vi "UNITEST MAIN v2.0.vi"() -> ()   [LabVIEW 2025]
uses:
  support/Message Queue/LAB-IQ Message Queue.lvlib
  support/Message Queue/Enqueue Message (Single).vi
  support/User Event - Stop/LAB-IQ User Event - Stop.lvlib
  <vilib>/Utility/error.llb/Error Cluster From Error Code.vi
  <vilib>/ErrorRing/Error Ring.xnode
  controls/LAB-IQ UI Data.ctl
  02c5850b-52e8-4ed5-91f8-6f0ad62f4994.vi
  HEAVE vi's/Heave Write enum.ctl
  d081153b-36ca-4bc4-8478-749476f82ba4.vi
  1223eb78-e4c4-4b69-bf80-185c82055158.vi
  e5651a45-6a49-4a3f-b503-ff1eaf449b4a.vi
  SWAY vi's/Sway Write enum.ctl
  1202965f-721d-4349-8d61-5de826f379ef.vi
  <vilib>/platform/TimedLoop/XDataNode/XDataNode.xnode
  <vilib>/Platform/TimedLoop/XDataNode/nitl_modes.ctl
  <vilib>/Platform/TimedLoop/XDataNode/XDNodeRunTimeDep.lvlib
  <vilib>/Platform/TimedLoop/XDataNode/wakeup.ctl
  <vilib>/Platform/TimedLoop/XDataNode/timing_clust.ctl
  HEAVE vi's/Heave Right enum.ctl
  SWAY vi's/Sway Right enum.ctl
  Traction Loop/Traction Write enum.ctl
  48f5795f-33f4-4366-aaa7-704d1097ecc1.vi
  Traction Loop/Traction Read enum.ctl
  0f9b3d6c-7caf-4790-9f98-5fac89a3677b.vi
  Acquostics Loops/Write Main Enum.ctl
  Acquostics Loops/Read Main Enum.ctl
  <vilib>/Utility/file.llb/Read Delimited Spreadsheet (string).vi
  <vilib>/Utility/file.llb/Write Delimited Spreadsheet (string).vi
  v05/LOAD CELL CODE/New Logic/Load cell Enum.ctl
  Traction Loop/Traction Receipe Enum.ctl
panel:
  in  "Ramp":bool
  out "Load Cell Communication Slide":u8(slide)=1 min=1 max=10 step=1 scale=0.0..10.0
  in  "Uplink Traction":refnum<vi>
  in  "Traction":bool
  in  "Scratch":bool
  in  "LRM CAM":bool
  in  "Sway LRM":bool
  in  "Rotary Horizontal":bool
  in  "Rotary Vertical":bool
  out "Acoustic Graphs":cluster{"number: 0 to 1":dbl, dbl, dbl}(graph)
  out "SET entrainment Velocity":dbl
  out "Test Array Size":i32
  in  "SRR INDEX [ STRIBECK]":i32
  out "Stribeck Size":i32
  out "SET SRR":dbl
  out "Enum - READ":T1
  out "ELAPSED TIMER":dbl
  out "BALL SET RPM":dbl
  out "DISC SET RPM":dbl
  out "SET LOAD":dbl
  in  "TEMPERATURE READ":dbl=40.0
  out "SET TEMPERATURE":dbl
  out "Traction Size":i32
  out "DISC SPEED (rpm)":dbl=100.0 min=0.1 max=3000.0 step=0.1 format="%.1f"
  out "BALL SPEED (rpm)":dbl=100.0 min=0.1 max=3000.0 step=0.1 format="%.1f"
  in  "BALL WEAR TRACK":dbl=7.9
  in  "DISC WEARTRACK":dbl=24.0
  in  "SRR INDEX [ TRACTION]":i32
  in  "Start Index Type":i32
  in  "Enum - Menu":T1
  out "Ball (mm/sec)":dbl
  out "Disc (mm/sec)":dbl
  in  "Traction Receipe Update Details":bool
  in  "HomeTraction":bool
  in  "Demo Mode Display":enum32{"Page 1", "Page 2"}(tab)
  in  "Traction Message":string="Recommended motion directions \nfor traction module.\n\nBall:  Counterclockwise\nDisc: Clockwise"
  in  "Traction Step Update Details":bool
  in  "Main Tab sequence for selection":T2(tab)
  out "ExceedDiscSpeed  Cinstant Speed":string
  out "ExceedBallSpeed Constant":string
  in  "TEST SELECTION (MTM) 2":enum32{"Ball Speed", "Disc Speed"}(radio)
  in  "SPEED SELECTION : MTM 2":enum32{"Speed in Rpm", "Speed in m/sec"}(radio)=enum."Speed in m/sec"
  in  "MTM Test Selection 2":enum32{"Time", "Cycle"}(radio)
  in  "Enter the Speed (m/sec):":dbl=0.5 min=3e-06 max=2500.0 step=0.001 format="%.6f"
  in  "Enter the Speed (m/sec):":dbl=0.5 min=3e-06 max=3000.0 step=0.001 format="%.6f"
  in  "Enter the Speed (RPM):":dbl=100.0 min=0.1 max=3000.0 step=0.1 format="%.1f"
  out "Lower Spped":string
  out "Upper":string
  in  "Enter the Speed (RPM):":dbl=1.0 min=0.1 max=2500.0 step=0.1 format="%.1f"
  out "ExceedBallSpeed step":string
  out "ExceedDiscSpeed":string
  out "Disc Speed Indicator":bool
  out "ExceedBallSpeed":string
  out "BallSpeed Exceed Indication":bool
  in  "Apply":bool
  in  "SPEED SELECTION : MTM":enum32{"Speed in Rpm", "Speed in m/sec"}(radio)=enum."Speed in m/sec"
  in  "TEST SELECTION (MTM)":enum32{"Ball Speed", "Disc Speed"}(radio)
  in  "MTM Test Selection":enum32{"Time", "Cycle"}(radio)
  in  "File Path Tab":enum32{"Page 1", "Page 2"}(tab)
  in  "File Path String":string="File Path Location : C:-->LAB-IQ 150 --> User Defined\n                                       Protocol-->File.txt"
  in  "Save":bool
  in  "Import":bool
  in  "File Path :":path
  in  "Step Sequence Indication Tab":enum32{"Page 1", "Page 2"}(tab)
  in  "Step Sequence Indication":string="Minimum 2 Steps required to perform the Speed Sequence"
  in  "Calculate Step":bool
  in  "StepTable":string[][](table)
  in  "Ramp Tab":enum32{"Page 1"}(tab)
  out "e.v/ssr":enum32{"E.V", "SSR"}(tab)
  in  "Enter Fixed SRR":dbl=1.0 min=-1.0 max=1.0 step=0.001 format="%.3f"
  in  "Enter the Final E.Velocity (m/s)":dbl=1.0 min=0.001 max=10.0 step=0.001 format="%.3f"
  in  "Enter initial E.Velocity (m/s)":dbl=2.0 min=0.001 max=10.0 step=0.001 format="%.3f"
  in  "Enter Fixed E.Velocity":dbl=1.0 min=0.001 max=2.0 step=0.001 format="%.3f"
  in  "Enter Final SRR":dbl=1.0 min=-1.0 max=1.0 step=0.001 format="%.2f"
  in  "Enter initial SRR":dbl=1.0 min=-1.0 max=1.0 step=0.001 format="%.2f"
  in  "Ball WTD":dbl=17.32 min=17.32 max=17.32 step=0.001 format="%.2f"
  in  "E.Velocity":bool caption="SRR"
  in  "Enter the Final Velocity (m/s)":dbl=1.0 min=0.001 max=2.0 step=0.001 format="%.3f"
  in  "Enter initial Velocity (m/s)":dbl=2.0 min=0.001 max=2.0 step=0.001 format="%.3f"
  out "Ramp Up   Disc":bool caption="Ramp Down"
  out "Initial DiscSpeed (RPM)":dbl=100.0 min=0.1 max=3000.0 step=0.1 format="%.1f"
  out "Final Speed (RPM)":dbl=1.0 min=0.1 max=3000.0 step=0.1 format="%.1f"
  out "Final Speed (RPM)":dbl=1.0 min=0.1 max=3000.0 step=0.1 format="%.1f"
  out "Initial Speed (RPM)":dbl=100.0 min=0.1 max=3000.0 step=0.1 format="%.1f"
  in  "Enter the Final Velocity (m/s)":dbl=1.0 min=0.001 max=2.0 step=0.001 format="%.3f"
  in  "Enter initial Velocity (m/s)":dbl=2.0 min=0.001 max=2.0 step=0.001 format="%.3f"
  out "Ramp Up":bool caption="Ramp Down"
  in  "Disc Motion Direction:":u16(ring) items=["Clockwise", "Counter Clockwise"]
  in  "Ball Motion Direction :":u16(ring) items=["Clockwise", "Counter Clockwise"]
  in  "Motion Mode:":u16(ring) items=["Uniform Rotation", "Speed Step", "Speed Ramp", "Speed Recipe"]
  in  "Wear Track Diameter (mm) 3":dbl=16.0 caption="Wear Track Diameter (mm):" min=1.0 max=20.0 step=0.01 format="%.2f"
  in  "Set WTD 2":bool
  in  "SRR Sweep Range (%)":string caption="Speed (mm/s)"
  out "Traction Receipe":i32(listbox)=-1
  in  "Total Execution Time":dbl
  in  "Total Steps":dbl
  in  "Duration / Step (s)":dbl=6.0
  in  "STRIBECK Fixed SRR List (%)":string="5,10,20,40,60,80,100"
  in  "Duration / Step (s)":dbl=6.0
  in  "SRR Sweep Range (%)":string
  in  "Speed (mm/s)":dbl=1000.0
  in  "Temperature Stages (°C)":string="40,100,140"
  in  "Load (N)":string="25"
  in  "Lubricant Name":string
  in  "Profile File Name":string
  out "error out":errorcluster
  in  "DEPTH TRIP   ENABLE":bool
  in  "DEPTH TRIP VALUE":dbl
  in  "LOAD TRIP  ENABLE":bool
  in  "LOAD TRIP VALUE":dbl
  in  "CYCLIC COF TRIP  ENABLE":bool
  in  "CYCLIC FF TRIP  ENABLE":bool
  in  "FF TRIP  ENABLE":bool
  in  "COF TRIP  ENABLE":bool
  in  "CYCLIC CoF TRIP VALUE":dbl
  in  "CYCLIC FF TRIP VALUE":dbl
  in  "FF TRIP VALUE":dbl
  in  "COF TRIP VALUE":dbl
  in  "Checkbox 2":bool
  in  "Checkbox":bool=TRUE
  out "Scratch Start Recording":bool
  in  "SwaySpeed Set":bool
  in  "Update":bool
  in  "Analysis Home":bool
  in  "Installation/Replacement completed":bool
  in  "Loahead":bool
  out "Test Trip":bool
  out "Hymidity":bool
  in  "Humidity Disable trip":bool=TRUE
  in  "CoF Trip  2":dbl=540.0 min=100.0 max=540.0 step=1.0
  in  "File Path :  2":path
  out "Wear Track Diameter":dbl
  in  "Stribeck table":bool
  in  "seq":bool=TRUE
  out "Drive Error":string
  out "Scratch Start Test":bool
  in  "HomeScratch":bool
  in  "TEST SELECTION":enum32{"Time", "Cycle"}(radio)
  out "Spare 15":u8
  out "Spare 14":u8
  out "Spare 13":u8
  out "Spare 12":u8
  out "Spare 11":u8
  out "Spare 10":u8
  out "Spare 9":u8
  out "Spare 8":u8
  out "Start Test Temp":bool
  in  "AppLoadSeq scratch":bool
  in  "PID Delay (sec)":dbl=1.0 format="%#_6p"
  out "Spare 15":u8
  out "Spare 14":u8
  out "Spare 13":u8
  out "Spare 12":u8
  out "Spare 11":u8
  out "Spare 10":u8
  out "Spare 9":u8
  out "Spare 8":u8
  out "Load Cell Temp":bool
  in  "Stop Scratch":bool
  in  "Enter Fixed SRR 2":dbl min=0.0 max=0.0 format="%.3f"
  in  "E.Velocity 2":bool=TRUE caption="SRR"
  in  "Tab Control 3":T3(tab)
  in  "PID":T4={"min_deadband_floor"=50000000.0, "min_finetune_floor"=10.0, "dynamic_spindle_noise_scalar"=100.0, "filter_alpha"=0.05, "Vertical load (N)"=0.0, "Pulse delta"=0.0, "Fine Tune Zone"=10.0, "Max_pos_limit"=50000000.0, "Min_pos_limit"=0.0, "i_limit"=10.0, "Max Step Linit"=10.0, "Init Step"=10.0, "pct_scale"=100.0, "Deadband"=0.1, "Kd"=0.0, "Ki"=0.0, "Kp"=1.0, "Current Position"=0.0, "Set Load"=0.0, "Current Load"=0.0, "gFF Rot 7"={0.0, 0.0, 0.0}, "Bypass Load"=FALSE, "Enter ByPass Load"=0.0, "apply load"=FALSE} {"Vertical load (N)" format="%#.3f"}
  in  "Load Cell Link":T5={"model"="", "SN"=0, "Sensor IP"="192.168.1.100", "Port"=8080, "Acq Delay (ms)"=10.0, "Burst Delay (ms)"=10.0, "Save Dwell"=0.015, "FORCE (N)"=[], "TORQUE (N-m)"=[], "ft_data"=[1.0, 1.0, 1.0, 1.0, 1.0, 1.0], "running_flag"=FALSE, "ClearAll"=FALSE, "ZeroAll"=FALSE} {"Save Dwell" min=0.0 max=5.0 step=0.001 format="%.3f"}
  out "Downlink traction":T6 {"TRACTION POSE 1" format="%#.6f"; "TRACTION POSE 2" format="%#.6f"; "Missed Packets" format="%#.6f"}
  in  "Uplink Traction 2":T7={"Sequence ID"=0, "Mode Command"=2, "Distance"=10000.0, "SPEED"=10000.0, "Reserved "=0.0, "SPARE 1"=0, "SPARE 2"=0, "SPARE  3"=0, "SPARE  4"=0, "SPARE  5"=0, "SPARE 6"=0, "SPARE 7"=0, "SPARE 8"=0, "SPARE 9"=0, "SPARE 10"=0, "SPARE 11"=0, "SPARE 12"=0, "SPARE 13"=0, "SPARE 14"=0, "SPARE 15"=0, "SPARE 16"=0, "SPARE 17"=0}
  out "DOWNLINK SWAY":T8 {"SWAY POSE" format="%#.6f"; "Rotary POSE" format="%#.6f"; "Missed Packets" format="%#.6f"}
  in  "UPLINK SWAY":T9={"Sequence ID"=0, "Mode Command"=2, "Distance"=10000.0, "SPEED"=10000.0, "Reserved"=0.0, "SPARE1"=0, "SPARE 2"=0, "SPARE  3"=0, "SPARE  4"=0, "SPARE  5"=0, "SPARE 6"=0, "SPARE 7"=0, "SPARE 8"=0, "SPARE 9"=0, "SPARE 10"=0, "SPARE 11"=0, "SPARE 12"=0, "SPARE 13"=0, "SPARE 14"=0, "SPARE 15"=0, "SPARE 16"=0, "SPARE 17"=0}
  out "DOWNLINK HEAVE":T10 {"HEAVE POSE" format="%#.6f"; "SURGE POSE" format="%#.6f"; "Missed Packets" format="%#.6f"}
  in  "UPLINK HEAVE":T11={"Sequence ID"=0, "Mode Command"=2, "Distance"=10000.0, "SPEED"=10000.0, "Reserved"=0.0, "SPARE 1"=0, "SPARE 2"=0, "SPARE 3"=0, "SPARE 4"=0, "SPARE 5"=0, "SPARE 6"=0, "SPARE 7"=0, "SPARE 8"=0, "SPARE 9"=0, "SPARE 10"=0, "SPARE 11"=0, "SPARE 12"=0, "SPARE 13"=0, "SPARE 14"=0, "SPARE 15"=0, "SPARE 16"=0, "SPARE 17"=0}
  out "error out 2":errorcluster
  in  "error in (no error)":errorcluster
  out "Downlink Packet":T12
  in  "Uplink Packet":T13
  in  "Manual Write TRACTION":bool
  out "TRACTION WRITE":string
  out "Read TRACTION Temp":bool
  out "error out Read TRACTION":errorcluster
  out "error out Write  TRACTION":errorcluster
  out "TRACTION READ":string
  in  "Manual Write SWAY":bool
  out "SWAY WRITE":string
  out "Read SWAY Temp":bool
  out "error out Read SWAY":errorcluster
  out "error out Write  SWAY":errorcluster
  out "SWAY READ":string
  out "HEAVE ENABLE":bool
  in  "Manual Write Heave & Surge":bool
  out "Heave and Surge Write":string
  out "Read Heave Temp":bool
  out "error out Read":errorcluster
  out "error out Write":errorcluster
  out "Heave and Surge Read":string
  out "DAQ Status":u32
  out "Isolated Gain":u32
  out "Current Filter Id":u32
  out "rx command count":u32
  out "Last Config Rejected":u32
  out "data out":string
  in  "Manual Write Acquostic":bool
  in  "Sway Loop Delay":dbl
  in  "Sway PID Speed":dbl=1.0 format="%.4f"
  in  "Sway Jog Speed":dbl=1.0 format="%.4f"
  in  "Heave Loop Delay":dbl
  in  "Heave PID Speed":dbl=15.0
  in  "Surge Jog Speed":dbl=1.0 format="%.4f"
  in  "Heave Jog Speed":dbl=15.0
  in  "Sway PPR":dbl=6400.0
  in  "Surge PPR":dbl=6400.0
  in  "Heave PPR":dbl=6400.0
  in  "Sway Pitch":dbl=2.0
  in  "Surge Pitch":dbl=3.0
  in  "Heave Pitch":dbl=4.0
  out "Sway Pulses/mm":dbl=320.0
  out "Surge Pulses/mm":dbl=1600.0
  out "Heave Pulses/mm":dbl=1600.0
  out "Zmm":dbl=1600.0
  in  "Heave distance":dbl=340.0
  in  "RotHomeSurgeOffsetCounts":dbl=311465.0
  in  "RotHomeSwayOffsetCounts":dbl=14656.0
  in  "TracHomeSwayOffsetCounts 20MM":dbl=1432.0
  in  "TracHomeSurgeOffsetCounts 20MM":dbl=505100.0
  in  "LRMHomeSwayOffsetCounts":dbl=26880.0
  in  "LRMHomeSurgeOffsetCounts":dbl=307197.0
  in  "Heave Counts:":dbl=100.0 min=0.0 max=100000000.0 step=1.0
  in  "Distance (mm):":dbl=100.0 min=0.0 max=1500.0 step=0.001 format="%.5f"
  in  "Distance (mm): 2":dbl=100.0 caption="Distance (mm):" min=0.0 max=1500.0 step=0.0001 format="%.3f"
  in  "Surge Counts:":dbl=100.0 min=0.0 max=100000000.0 step=1.0 format="%.1f"
  in  "Distance (mm): 3":dbl=100.0 caption="Distance (mm):" min=0.0 max=1500.0 step=0.001 format="%.5f"
  in  "Sway Counts:":dbl=100.0 min=0.0 max=100000000.0 step=1.0 format="%.2f"
  in  "Enter Distance":bool caption="Enter Counts"
  in  "SAVE  2":bool
  in  "DataSavingLoopDelay(ms)":dbl=15.0
  in  "Surge distance (mm)":dbl=370.0
  in  "Sway distance (mm)":dbl=245.0
  in  "Filter%":dbl=80.0 min=50.0 max=100.0 step=0.1 format="%.1f"
  in  "Apply Filter (Load)":bool=TRUE
  in  "Filter% 2":dbl=50.0 min=50.0 max=100.0 step=0.1 format="%.1f"
  in  "Apply Filter (FF)":bool
  in  "Acoustic Emission:":dbl=1.0 min=0.0001 max=200.0 step=0.0001 format="%.4f"
  in  "TracHomeSwayOffsetCounts 10MM":dbl=1432.0
  in  "TracHomeSurgeOffsetCounts 10MM":dbl=505100.0
  in  "Filter ON/OFF":bool=TRUE
  in  "Re-initilaize":bool
  in  "SAMPLES":dbl=100.0
  in  "JOG TRIP LOAD VALUE (N)":dbl
  in  "GUI":T14(tab)
  in  "Platform Settings":bool caption="Password"
  in  "Configure":bool caption="Password"
  in  "Home":bool caption="Password"
  in  "EXIT":bool
  in  "Analysis":bool caption="Password"
  in  "service 2":bool caption="Password"
  in  "MainPage":T15(tab)=enum."HOME"
  in  "Select Load Head":bool
  in  "Notes :":string
  in  "FILE":string
  in  "Sample ID :":string
  in  "Operator ID :":string
  in  "Operator Name :":string
  in  "Auto":bool caption="Power Status"
  in  "Disable Axis Jog Soft Limits m":bool
  out "Sway and Surge COM Status":bool=TRUE caption="Load COM Status"
  out "Heave COM Status":bool=TRUE caption="Load COM Status"
  in  "Enable Platform":bool
  in  "Surge Forward Main":bool
  in  "Surge Backward Main":bool
  in  "Sway Right Main":bool
  in  "Sway Left Main":bool
  in  "Heave Down Main":bool
  in  "Heave Up main":bool
  in  "mm":dbl=0.001 caption="Jog" min=0.001 max=100.0 step=0.01 format="%#.3f"
  in  "Surface Analysis":bool
  in  "Imaging":bool
  in  "Image Analysis":bool
  in  "Post Analysis":bool
  in  "SSP 0.75":bool
  in  "SSP 0.5":bool
  in  "SSP 0.3":bool
  in  "Warning":enum32{"Page 2"}(tab)
  in  "gui GIF":enum32{"Check", "Deca", "kilo", "Micro"}(tab)
  out "Communication is established":bool=TRUE caption="Load COM Status"
  in  "Reference Sample":u16(ring) items=["None", "Brass", "Aluminium", "Mild Steel"]
  in  "com 3":bool
  out "com":bool
  out "DecaForce COM Status":bool caption="Load COM Status"
  in  "Loading Mode":u16(ring) items=["Constant", "Ramp", "Steps", "Indentation"]
  in  "Enter the CoF Trip":dbl=1.0
  in  "Enter the Friction Force Trip":dbl=520.0 min=500.0 max=500.0 step=1.0 format="%#.1f"
  in  "Enter the Normal load Trip":dbl=520.0 min=500.0 max=500.0 step=0.001 format="%.3f"
  in  "KiloForce":bool
  in  "DecaForce":bool
  in  "MicroForce":bool
  in  "LHBack":bool
  in  "LHNext":bool
  in  "Load Selection":T16(tab)
  in  "Enter the Load  (N)":dbl=2.0 caption="Enter the Load (N)" min=2.0 max=200.0 step=0.1 format="%#.4f"
  in  "Enter the Final Load (N)":dbl=1.0 min=0.0 max=500.0 step=1.0 format="%#.0f"
  in  "Enter the Loading Rate (N/min)":dbl=60.0 min=1.0 max=200.0 step=0.1 format="%.2f"
  out "Warning 2":bool
  in  "Stribeck Table  For loading":string[][](table)
  in  "Clear 3":bool
  out "Message":string="Load Entered is out of range!!!"
  in  "Save 3":bool
  in  "Import 3":bool
  in  "Indentation":string[][](table)=[["Detection", "5", "2"], ["Unload", "0", "5"], ["Load", "10", "2"], ["Unload", "0", "5"], ["Detection", "5", "2"], ["Unload", "0", "5"]]
  in  "Multipoint":bool caption="Singlepoint"
  in  "AppLoad 4":bool
  in  "zNL":bool
  out "NL disp":dbl caption="Normal Load ( N )" min=-2000.0 max=2000.0 step=0.0001 format="%.1f"
  in  "Traction":bool
  in  "Surge Forward MM":bool
  in  "Surge Backward MM":bool
  in  "M3 Image":enum32{"Page 1", "Page 2"}(tab)
  in  "String 39":string="Jog heave to bring the upper sample closer to the lower sample within 1mm."
  in  "Sway Left MM":bool
  in  "Sway Right MM":bool
  in  "Disable Axis Jog Soft Limits":bool
  in  "mm":dbl=0.001 caption="Jog" min=0.001 max=5.0 step=0.0001 format="%#.3f"
  in  "Heave Down MM":bool
  in  "Heave Up MM":bool
  in  "Wear Track Diameter (mm)":dbl=30.0 caption="Wear Track Diameter (mm):" min=1.0 max=30.0 step=1.0 format="%.2f"
  in  "Set WTD":bool
  in  "HomeScratch":bool
  in  "HomeRot":bool
  in  "PlaceModule":bool
  in  "Motion Mode:":u16(ring) items=["Uniform Rotation", "Angular Oscillation", "Stribeck ", "Steps"]
  in  "LR Sway":bool
  in  "Rot Hor":bool
  in  "Rot Ver":bool
  in  "Scratch":bool
  in  "LR Cam":bool
  in  "MMBack":bool
  in  "MMNext":bool
  in  "Rotary Module Selection":T17(tab)
  in  "SPEED SELECTION :":enum32{"Speed in RPM", "Speed in m/sec"}(radio)=enum."Speed in m/sec"
  in  "Enter the Speed(mm/sec)":dbl=0.1 min=0.0001 max=1000.0 step=0.1 format="%#.4f"
  in  "Enter the Speed (RPM)":dbl=45.0 min=1.0 max=3000.0 step=1.0
  in  "Enter the Frequency (Hz)":dbl=1.0 min=0.1 max=10.0 step=0.1 format="%.1f"
  in  "Enter the Angle (Deg)":dbl=45.0 min=5.0 max=300.0 step=1.0
  in  "Angular Oscillation Set":bool
  in  "Rotary Tab":enum32{"Page 1", "Page 2"}(tab)
  out "e.v/ssr 2":enum32{"E.V", "SSR"}(tab)
  in  "Enter the Final E.Velocity (m/s) 2":dbl=1.0 min=0.001 max=4.0 step=0.001 format="%.3f"
  in  "Enter initial E.Velocity (m/s) 2":dbl=2.0 min=0.001 max=4.0 step=0.001 format="%.3f"
  in  "Enter Fixed E.Velocity 2":dbl=1.0 min=0.001 max=2.0 step=0.001 format="%.3f"
  in  "Enter Final SRR 2":dbl=1.0 min=0.001 max=1.0 step=0.001 format="%.2f"
  in  "Enter initial SRR 2":dbl=1.0 min=0.001 max=1.0 step=0.001 format="%.2f"
  out "Final Speed (RPM) 3":dbl=1.0 min=0.1 max=3000.0 step=0.1 format="%.1f"
  out "Initial Speed (RPM) 2":dbl=100.0 min=0.1 max=3000.0 step=0.1 format="%.1f"
  in  "Enter the Final Velocity (m/s) 3":dbl=1.0 min=0.001 max=2.0 step=0.001 format="%.3f"
  in  "Enter initial Velocity (m/s)  3":dbl=2.0 min=0.001 max=2.0 step=0.001 format="%.3f"
  out "Ramp Up 2":bool caption="Ramp Down"
  in  "Import 2":bool
  in  "Save 2":bool
  in  "SPEED SELECTION : rotary":enum32{"Speed in Rpm", "Speed in m/sec"}(radio)=enum."Speed in m/sec"
  in  "calculate rotary":bool
  in  "String 45":string="File Path Location : C:-->LAB-IQ 150 --> User Defined\n                                       Protocol-->File.txt"
  in  "Step Speed":enum32{"Step Speed", "Step (load-Speed)"}(tab)
  in  "StepTable For Speed":string[][](table)
  in  "StepTable For Load-Speed":string[][](table)=[["", "", ""], ["", "", ""], ["", "", ""], ["", "", ""]]
  in  "StepTable For Speed 3":string[][](table)=[["", "", ""], ["", "", ""], ["", "", ""], ["", "", ""]]
  in  "Motion Direction:  3":u16(ring)=1 items=["Clockwise", "Counter Clockwise"]
  in  "Enter Scratch length (mm):":dbl=1.0 min=1.0 max=50.0 step=0.0001 format="%.4f"
  in  "Enter Scratch Speed (mm/s):":dbl=1.0 min=0.003 max=10.0 step=0.0031 format="%.5f"
  in  "Scartch Offset":dbl=1.0 caption="Scratch Offset: (mm)" min=0.1 max=5.0 step=0.1 format="%.1f"
  in  "Motion type:":u16(ring) items=["Unidirection", "Bidirection"]
  in  "Scratch Mode":u16(ring) items=["Scratch", "Pre-Post Scan", "Multi Scratch"]
  in  "Rotary Speed Exced":string="Motor Speed Out of Range"
  in  "No of Scratch":dbl=1.0 min=1.0 max=50.0 step=0.0001
  out "Humidity  Status  3":bool caption="Communication Status"
  out "Low Temp  Status  2":bool=TRUE caption="Communication Status"
  out "TK4 status 2":bool=TRUE caption="Communication Status"
  in  "Acuostic M":string="Before selecting Acoustic make sure the sensor output pin is connected to A4."
  in  "Stage Temperature":dbl[](array[numeric])=[150.0, 230.0, 300.0, 350.0, 400.0, 450.0, 500.0]
  in  "Sample Temperature":dbl[](array[numeric])=[100.0, 150.0, 200.0, 250.0, 300.0, 350.0, 400.0]
  in  "Humidity (Amb)":bool
  in  "Clear List":bool
  out "Sensors Picked":string
  in  "Add to list":bool
  in  "Wear":bool
  in  "Vibration":bool
  in  "Humidity (Chamber)":bool
  in  "Temperature (Chamber)":bool
  in  "ECR":bool
  in  "Temperature (Amb)":bool
  in  "Microphone":bool
  in  "Acoustic Emission 3":bool
  in  "SNext":bool
  in  "APBack":bool
  in  "Enter the Temperature (°C):":dbl
  in  "Enter the Stage \nTemperature (°C):":dbl=20.0 min=20.0 max=150.0 step=1.0 format="%#.0f"
  in  "Enter the Humidity (%Rh):":dbl=30.0 min=30.0 max=85.0 step=1.0
  in  "Low Temp":bool
  in  "High Temp":bool
  in  "Humidity":bool
  in  "Gains":enum32{"20dB", "40dB", "60dB"}(radio)=enum."60dB"
  in  "Main Screen Tab":T18(tab)
  out "NL Trip 2":dbl=600.0
  out "Load Reset Graph":bool
  out "NL Display 4":dbl caption="Normal Load ( N )" min=-2000.0 max=2000.0 step=0.0001 format="%.1f"
  out "Load Disable Trip":bool=TRUE
  out "Main Chart 3":cluster{dbl, "NL disp":dbl, dbl}(graph)
  in  "Aqucostic Reset Graph":bool
  in  "Depth Reset Graph":bool
  out "Weart Deapth":bool
  in  "Depth Trip 2":bool=TRUE
  out "Depth Trip":dbl=600.0
  in  "ClrLog":bool
  out "Trip Log":string
  in  "Start Test":bool
  out "Test status":bool caption="Test Status"
  out "AR Led":bool caption="AR"
  out "Data":bool=TRUE
  out "Health":bool=TRUE
  out "Sway COM Status":bool=TRUE caption="Load COM Status"
  out "Heave COM Status":bool=TRUE caption="Load COM Status"
  in  "BACK":bool
  out "Ambient \nTemperature":dbl min=0.0 max=5000.0 step=0.1 format="%.1f"
  out "Ambient\n Humidity":dbl min=0.0 max=5000.0 step=0.1 format="%.2f"
  out "NL disp 2":dbl caption="Normal Load ( N )" min=-2000.0 max=2000.0 step=0.0001 format="%.1f"
  out "Set Humidity":dbl caption="Set Humidity  (% Rh)" min=-2000.0 max=2000.0 step=1.0 format="%.1f"
  out "humidity disp":dbl caption="Humidity (% Rh)" min=-2000.0 max=2000.0 step=1.0 format="%.1f"
  in  "Humidity On":bool
  in  "zNL 2":bool
  in  "Load En":bool
  out "Freq (Hz)":dbl min=0.0 max=5000.0 step=0.1 format="%.4f"
  out "HumCOMStatus":bool caption="Communication Status"
  out "Load Communication":bool
  in  "Temp Tabs":enum32{"Low Temp", "High Temp"}(tab)=enum."High Temp"
  out "Controller  Status":bool
  out "ChamberTemp":dbl format="%#.1f"
  in  "SetTmp":dbl=-190.0 caption="Set Temperature (Deg C)" min=-190.0 max=100.0 step=1.0 format="%.1f"
  in  "Cooling":bool
  in  "Heater":bool
  out "TK4 status":bool caption="Controller  Status"
  out "ChamberTemp":dbl format="%#.1f"
  in  "SetTmp":dbl caption="Set Temperature (Deg C)" min=0.0 max=1000.0 step=1.0 format="%.1f"
  in  "Set Load (N)":dbl=100.0 min=0.01 max=1500.0 step=0.01 format="%.1f"
  in  "Time Tab":enum32{"cycles", "duration"}(tab)=enum."duration"
  out "Test Duration 4":dbl=600.0 caption="Test Duration\n(HH:MM:SS)" min=0.0083 max=180000.0 step=0.0001 format="%<%H:%M:%S>t"
  out "TEST CYCLE":dbl min=0.0 max=5000.0 step=0.01 format="%.2f"
  in  "TOTAL CYCLES":dbl min=0.0 max=5000.0 step=0.1 format="%.4f"
  out "Time ( HH:MM:SS ) 2":dbl min=0.0 max=144000.0 step=1.0 format="%<%H:%M:%S>t"
  in  "Test Duration":dbl=600.0 caption="Test Duration\n(HH:MM:SS)" min=0.0083 max=180000.0 step=0.0001 format="%<%H:%M:%S>t"
  in  "Main Speed Tab":enum32{"ROTARY", "TRACTION"}(tab)
  in  "SPEED TAB":enum32{"RPM", "m/sec"}(tab)
  out "Speed (RPM)":dbl min=0.0 max=5000.0 step=0.1 format="%.1f"
  out "Set Speed":dbl caption="Set Speed (RPM)" min=0.0 max=1500.0 step=0.1 format="%.1f"
  out "Speed (m/sec)":dbl min=0.0 max=5000.0 step=0.001 format="%.4f"
  out "Set Speed (m/sec)":dbl min=0.0 max=1500.0 step=0.001 format="%.4f"
  in  "MTM MOTOR DISPLAY":enum32{"MTM RPM", "MTM m/sec"}(tab)
  out "Disc Speed (RPM)":dbl min=0.0 max=1500.0 step=0.1 format="%.1f"
  out "Ball Speed (RPM)":dbl min=0.0 max=1500.0 step=0.1 format="%.1f"
  out "Disc Speed (m/sec)":dbl min=0.0 max=1500.0 step=0.1 format="%.1f"
  out "Ball Speed (m/sec)":dbl min=0.0 max=1500.0 step=0.1 format="%.1f"
  in  "Angle and Frequency":enum32{"angular", "lrm"}(tab)
  out "Angle (Deg)":dbl min=0.0 max=5000.0 step=0.01 format="%.2f"
  out "Stroke (mm)":dbl min=0.0 max=5000.0 step=0.01 format="%.2f"
  in  "STOP":bool
  out "Multi Scratch Pass":dbl min=0.0 max=5000.0 step=0.1
  in  "FF Tab":T19(tab)
  in  "COF Reset Graph":bool
  in  "COF Disable Trip":bool=TRUE
  out "COF TRIP":dbl=600.0
  out "Coefficient of Friction":dbl(graph)=0.13298760003255525
  in  "zFF":bool
  out "Friction Force (N)":dbl min=-2000.0 max=2000.0 step=0.0001 format="%.3f"
  in  "FF Reset Graph":bool
  in  "FF Disable Trip":bool=TRUE
  out "FF TRIP":dbl=600.0
  out "Friction Force (N) Graph":dbl(graph)=0.13298760003255525
  in  "CZ FF":bool
  out "Cyclic Friction Force (N)":dbl min=-2000.0 max=2000.0 step=0.0001 format="%.3f"
  out "Cyclic FF TRIP":dbl=600.0
  in  "Cyclic FF Disable Trip":bool=TRUE
  in  "Cyclic FF Reset Graph":bool
  out "Cyclic Friction Force (N) Graph":dbl(graph)=0.13298760003255525
  out "cyclic COF TRIP":dbl=600.0
  in  "cyclic COF Disable Trip":bool=TRUE
  in  "cyclic COF Reset Graph":bool
  out "Cyclic Coefficient of Friction":dbl(graph)=0.13298760003255525
  out "WearGp":dbl(graph)=0.13298760003255525
  out "Depth (µm)":dbl min=-200.0 max=200.0 step=0.1 format="%.1f"
  in  "Depthz":bool
  out "Weart":bool
  out "Acoustic Emission (mV)":dbl min=0.0 max=5000.0 step=0.1
  out "gACQUOS":dbl(graph)=0.13298760003255525
  in  "X-AXIS":u16(ring) items=["None", "Time ( Sec )", "Normal Load ( N )", "Frictional Force ( N )", "Coefficient of Friction", "Depth ( Microns )", "Speed ( RPM )", "Frequency ( Hz )", "Angle ( Degree )", "Cyclic Friction Force ( N )", "Cyclic Co efficient Friction ", "Stage temperature ( Degree celcius )", "Sample temperature ( Degree celcius )", "Stroke Length ( mm )", "Scratch Speed ( mm/sec )", "Amb Humidity ( % Rh ) ", "Amb Temperature (Deg C)", "Acoustic (mV)", "Mx (Nm)", "My (Nm)", "Mz (Nm)", "Humidity ( % Rh )", "Sliding Distance (mm)", "Wear Track Diameter (mm)", "Fx(N)", "Fy(N)", "MTM BallSpeed (RPM)", "MTM DiscSpeed (RPM)", "Entrainment Speed", "Slide Role", "Slip(%)", "Rotary Speed (m/sec)", "MTM Ball Speed (m/sec)", "MTM Disc Speed (m/sec)", "ECR (ohms)"]
  in  "Y-AXIS":u16(ring) items=["None", "Time ( Sec )", "Normal Load ( N )", "Frictional Force ( N )", "Coefficient of Friction", "Depth ( Microns )", "Speed ( RPM )", "Frequency ( Hz )", "Angle ( Degree )", "Cyclic Friction Force ( N )", "Cyclic Co efficient Friction ", "Stage temperature ( Degree celcius )", "Sample temperature ( Degree celcius )", "Stroke Length ( mm )", "Scratch Speed ( mm/sec )", "Amb Humidity ( % Rh ) ", "Amb Temperature (Deg C)", "Acoustic (mV)", "Mx (Nm)", "My (Nm)", "Mz (Nm)", "Humidity ( % Rh )", "Sliding Distance (mm)", "Wear Track Diameter (mm)", "Fx(N)", "Fy(N)", "MTM BallSpeed (RPM)", "MTM DiscSpeed (RPM)", "Entrainment Speed", "Slide Role", "Slip(%)", "Rotary Speed (m/sec)", "MTM Ball Speed (m/sec)", "MTM Disc Speed (m/sec)", "ECR (ohms)"]
  out "XY Graph":cluster{"Array 2":dbl[], "Array 2":dbl[]}[](graph) caption="XY Graph 20"
  out "VARIANCE":dbl=-0.0 format="%0.2f"
  out "SD":dbl=-0.0 format="%.3f"
  out "MEAN":dbl format="%.3f"
  out "VARIANCE":dbl=-0.0 format="%0.2f"
  out "SD":dbl=-0.0 format="%.3f"
  out "MEAN":dbl format="%.3f"
  out "VARIANCE":dbl=-0.0 format="%0.2f"
  out "SD":dbl=-0.0 format="%.3f"
  out "MEAN":dbl format="%.3f"
  out "VARIANCE":dbl=-0.0 format="%0.2f"
  out "SD":dbl=-0.0 format="%.3f"
  out "MEAN":dbl format="%.3f"
  in  "Analysis Home new":bool
  out "File 2 Discription":string="\r"
  out "File 1 Discription":string="\r"
  in  "OPEN 1":bool
  in  "OPEN 2":bool
  out "File Name 1":string
  out "File Name 2":string
  in  "Refresh 2":bool
  in  "OPEN 3":bool
  out "File Name 3":string
  out "File Name 4":string
  in  "OPEN 4":bool
  out "File 4 Discription":string="\r"
  out "File 3 Discription":string="\r"
  in  "File Format":u16(ring) items=["csv", "txt", "duf"]
  in  "Export":bool
  in  "Report":bool
  in  "Password":string
  in  "Home Service":bool
  in  "Advanced Setting":bool
  in  "About Tab":enum32{"Primary"}(tab)
  in  "ECR Port:":refnum<visa-resource-name>="COM10"
  in  "Ramp Port:":refnum<visa-resource-name>="COM10"
  in  "Temp Modbus:":refnum<visa-resource-name>="COM14"
  in  "Humidity Port:":refnum<visa-resource-name>="COM10"
  in  "Edit Gain Constants":bool
  in  "Save Gain Constants":bool
  in  "Service About":bool
  # "1. Test Identification & Global Setup"
  # "2. Step Configurations & Timing"
  # "Step 1 Configuration: TRACTION Step"
  # "%"
  # "NOTE: This operation needs to be done only when the machine is ON."
  # "Steps 2+ Configuration: STRIBECK Steps"
  # "Upper Drive (Ball)"
  # "Lower Drive (Disc)"
  # "Variable"
  # "Configuration"
  # "Limits for Heave Surge and Sway"
  # "Modules Offset Parameters"
  # "Counts-Distance Calculator"
  # "File Name :"
  # "Ensure the traction module is aligned\n horizontally with the stage before ENABLE."
  # "JOG MODE"
  # "Module Selection"
  # "Positioning Control"
  # "Connect the controller\ncable to M2"
  # "Environment"
  # "Sensors"
  # "Data Points"
  # "Data Points"
  # "Data Points"
  # "LAB-IQ 150 / UNITEST / WO2476 / UT150  v06 / AUGUST 2026"
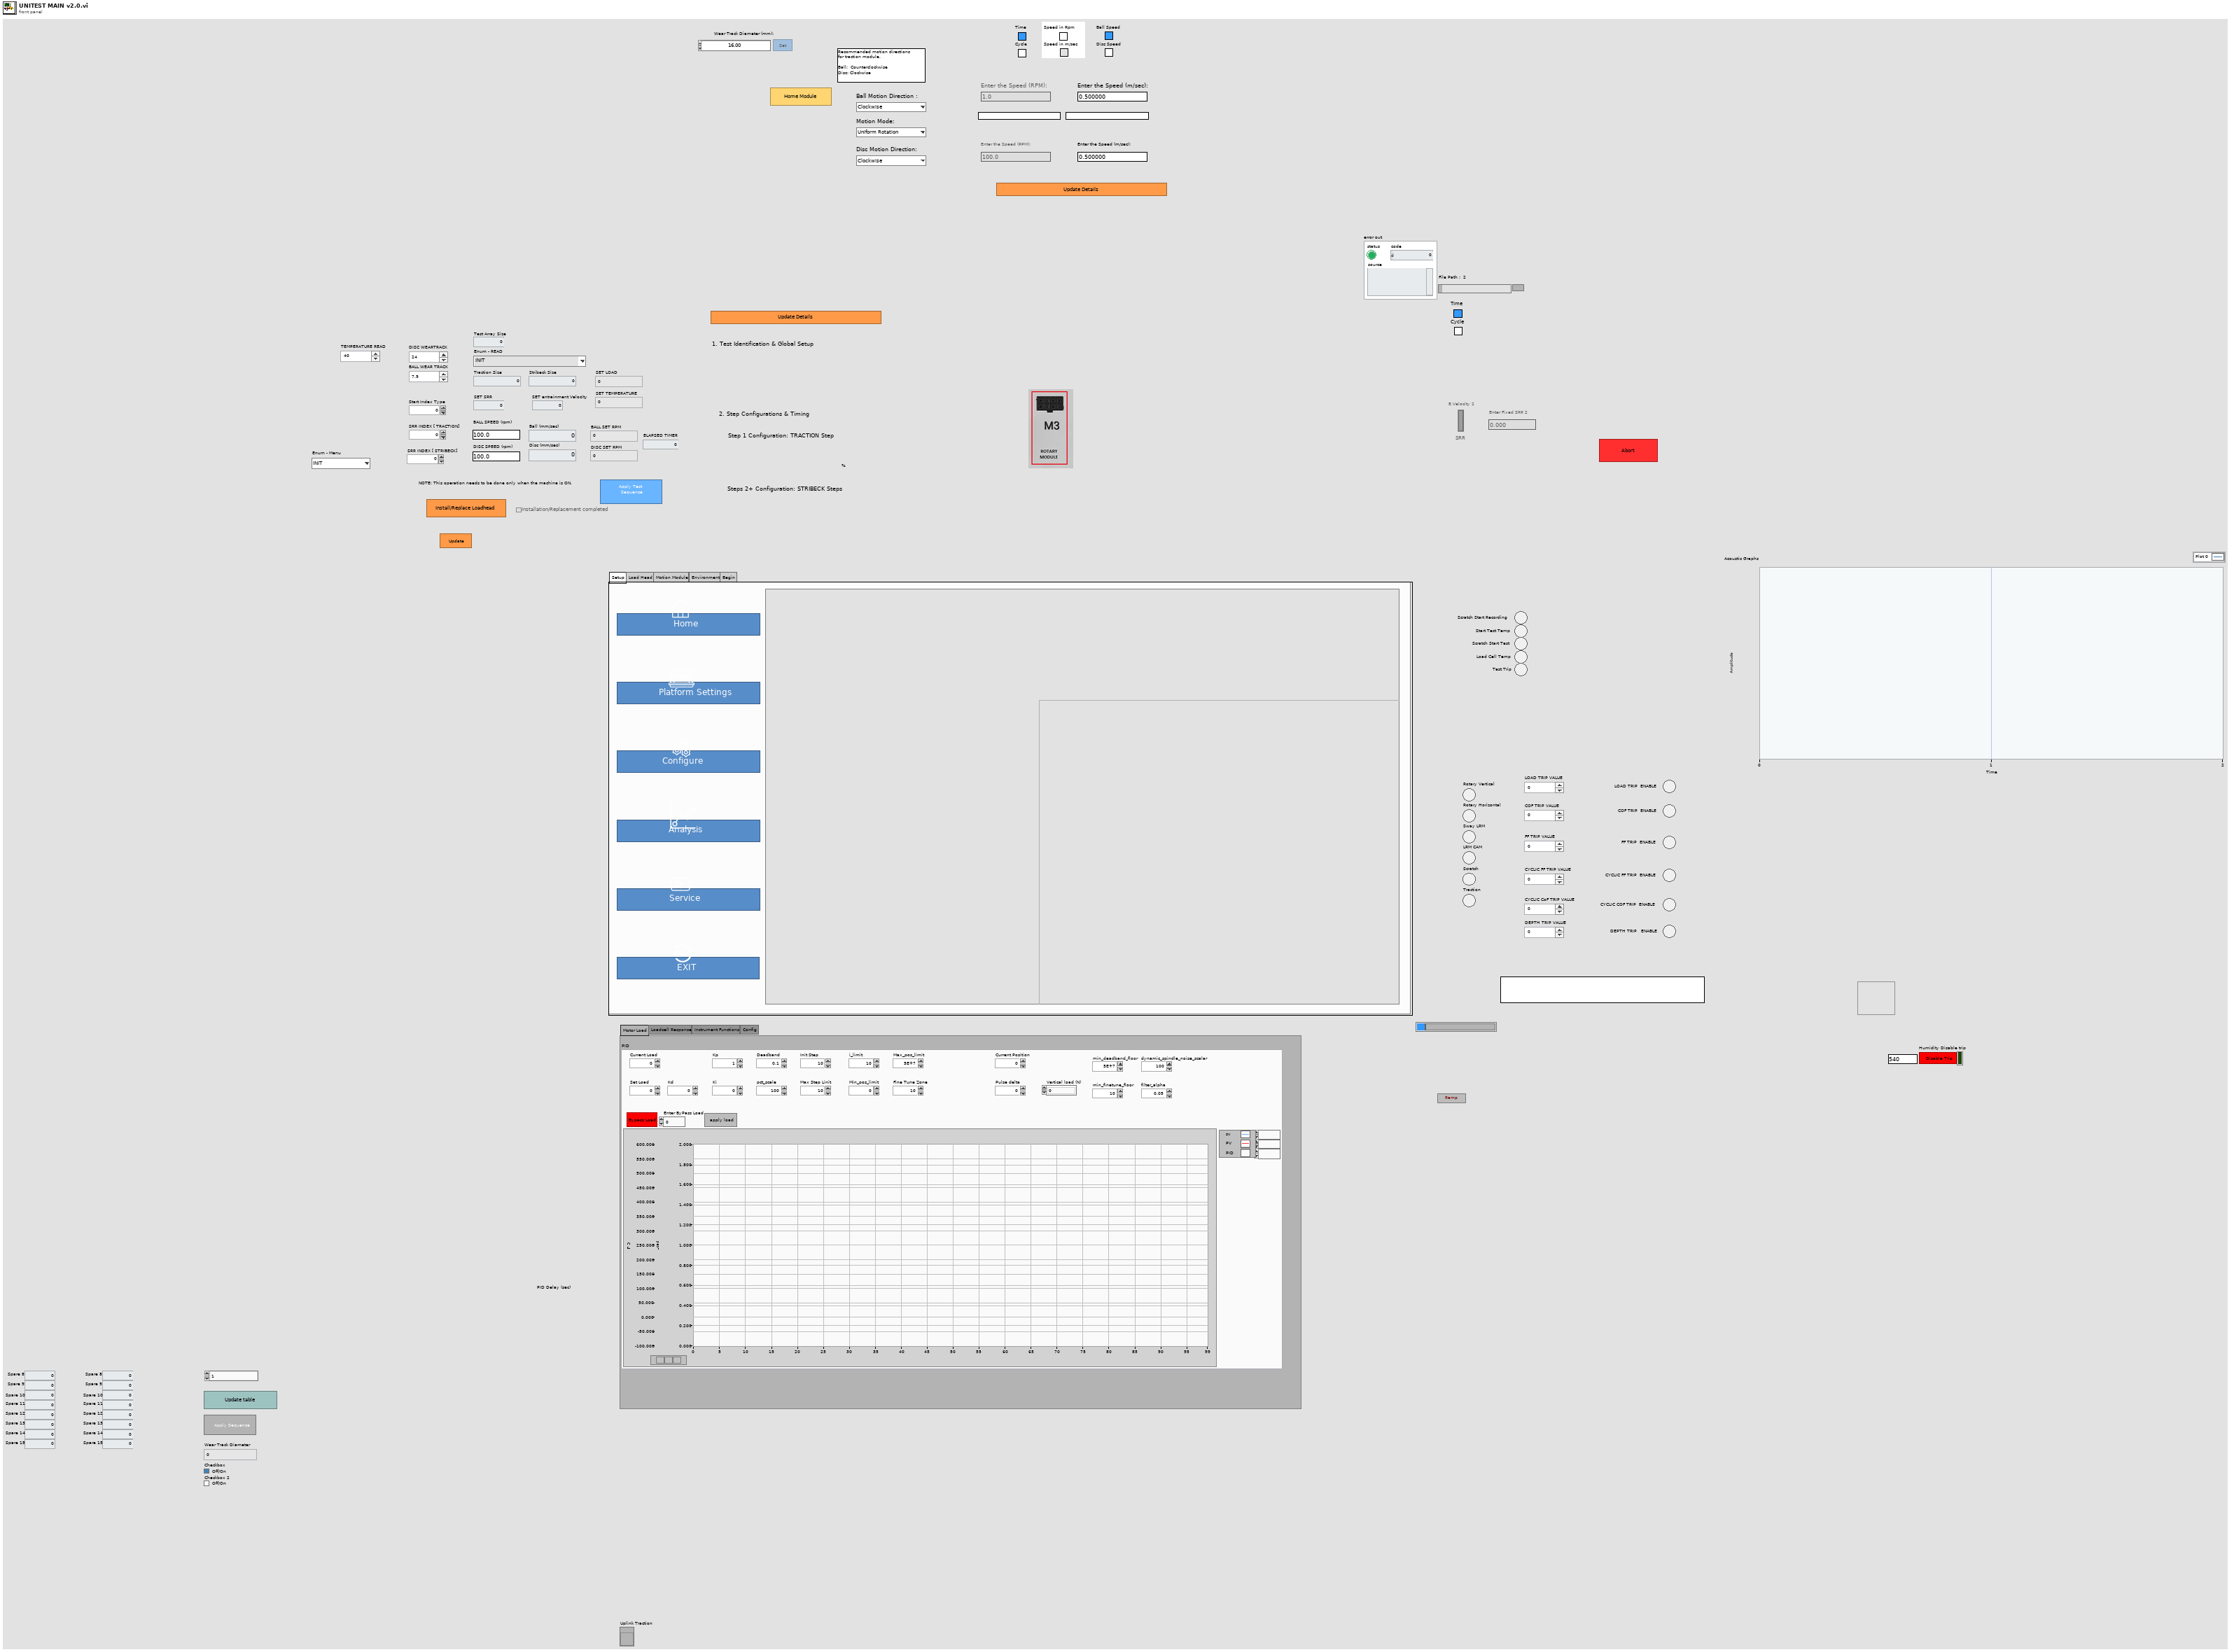
[diagram p1: front panel]
types:
  T1 = typedef "Traction Receipe Enum.ctl" = enum16{"INIT", "START", "TRACTION", "STRIBECK", "MAIN INDEX INCREMENT", "TEMPERATURE SET", "TEMPERATURE REACH", "CHURNING START", "CHURNING STOP", "LOAD", "LOAD REACHED", "SRR SET", "SRR WAIT", "SRR INCREMENT", "SPEED SET", "SPEED WAIT", "SPEED INCREMENT", "UNLOAD", "CLOSE"}
  T2 = enum32{"Uniform Rotary", "Speed Sequence", "SpeedRamp"}
  T3 = enum32{"Motor Load", "Loadcell Response", "Motor", "Depth_graph", "UIO Communicator", "Add to list parametrs", "Instrument Functions", "Config"}
  T4 = cluster{"min_deadband_floor":dbl, "min_finetune_floor":dbl, "dynamic_spindle_noise_scalar":dbl, "filter_alpha":dbl, "Vertical load (N)":dbl, "Pulse delta":dbl, "Fine Tune Zone":dbl, "Max_pos_limit":dbl, "Min_pos_limit":dbl, "i_limit":dbl, "Max Step Linit":dbl, "Init Step":dbl, "pct_scale":dbl, "Deadband":dbl, "Kd":dbl, "Ki":dbl, "Kp":dbl, "Current Position":dbl, "Set Load":dbl, "Current Load":dbl, "gFF Rot 7":cluster{dbl, dbl, dbl}, "Bypass Load":bool, "Enter ByPass Load":dbl, "apply load":bool}
  T5 = cluster{"model":string, "SN":i32, "Sensor IP":string, "Port":i32, "Acq Delay (ms)":dbl, "Burst Delay (ms)":dbl, "Save Dwell":dbl, "FORCE (N)":dbl[][], "TORQUE (N-m)":dbl[][], "ft_data":dbl[], "running_flag":bool, "ClearAll":bool, "ZeroAll":bool}
  T6 = cluster{"Ack ID":u16, "State":u8, "Homed":u8, "TRACTION POSE 1":sgl, "TRACTION POSE 2":sgl, "faultCode ":u16, "fwMajor ":u8, "fwMinor":u8, "Node Id":u8, "Spare 1":u8, "Spare 2":u8, "Spare 3":u8, "Spare 4":u8, "Spare 5":u8, "Spare 6":u8, "Spare 7":u8, "System UPTIME":sgl, "Missed Packets":sgl, "faultCode Traction 1":u16, "faultCode Traction 2":u16}
  T7 = cluster{"Sequence ID":u16, "Mode Command":u8, "Distance":sgl, "SPEED":sgl, "Reserved ":sgl, "SPARE 1":u8, "SPARE 2":u8, "SPARE  3":u8, "SPARE  4":u8, "SPARE  5":u8, "SPARE 6":u8, "SPARE 7":u8, "SPARE 8":u8, "SPARE 9":u8, "SPARE 10":u8, "SPARE 11":u8, "SPARE 12":u8, "SPARE 13":u8, "SPARE 14":u8, "SPARE 15":u8, "SPARE 16":u8, "SPARE 17":u8}
  T8 = cluster{"Ack ID ":u16, "State":u8, "Homed":u8, "SWAY POSE ":sgl, "Rotary POSE ":sgl, "faultCode":u16, "fwMajor":u8, "fwMinor":u8, "Node Id":u8, "Spare 1":u8, "Spare 2":u8, "Spare 3":u8, "Spare 4":u8, "Spare 5":u8, "Spare 6":u8, "Spare 7":u8, "System UPTIME ":sgl, "Missed Packets ":sgl, "faultCode Sway":u16, "faultCode Rotary":u16}
  T9 = cluster{"Sequence ID":u16, "Mode Command":u8, "Distance":sgl, "SPEED":sgl, "Reserved":sgl, "SPARE1":u8, "SPARE 2":u8, "SPARE  3":u8, "SPARE  4":u8, "SPARE  5":u8, "SPARE 6":u8, "SPARE 7":u8, "SPARE 8":u8, "SPARE 9":u8, "SPARE 10":u8, "SPARE 11":u8, "SPARE 12":u8, "SPARE 13":u8, "SPARE 14":u8, "SPARE 15":u8, "SPARE 16":u8, "SPARE 17":u8}
  T10 = cluster{"Ack ID":u16, "State":u8, "Homed":u8, "HEAVE POSE":sgl, "SURGE POSE":sgl, "faultCode":u16, "fwMajor":u8, "fwMinor":u8, "Node Id":u8, "Temp":u8, "Humidity":u8, "Spare 1":u8, "Spare 2":u8, "Spare 3":u8, "Spare 4":u8, "Spare 5":u8, "System UPTIME":sgl, "Missed Packets":sgl, "faultCode Heave":u16, "faultCode Surge Left":u16, "faultCode Surge Right":u16}
  T11 = cluster{"Sequence ID":u16, "Mode Command":u8, "Distance":sgl, "SPEED":sgl, "Reserved":sgl, "SPARE 1":u8, "SPARE 2":u8, "SPARE 3":u8, "SPARE 4":u8, "SPARE 5":u8, "SPARE 6":u8, "SPARE 7":u8, "SPARE 8":u8, "SPARE 9":u8, "SPARE 10":u8, "SPARE 11":u8, "SPARE 12":u8, "SPARE 13":u8, "SPARE 14":u8, "SPARE 15":u8, "SPARE 16":u8, "SPARE 17":u8}
  T12 = cluster{"Sequence ID":u32, "Timestamp":u32, "System Status":u32, "Peak Amplitude":sgl, "Amplitude dB_AE":sgl, "AE Ring-Down Counts":u32, "Signal Energy":sgl, "Spare 1":u32}
  T13 = cluster{"Sequence ID":u32, "Target Gain":u32, "Target Filter":u32, "Spare 1":u32, "Spare 2":u32, "Spare 3":u32, "Spare 4":u32, "Spare 5":u32}
  T14 = enum32{"Setup", "Load Head", "Motion Module", "Environment", "Begin"}
  T15 = enum32{"Details", "PlatformSetting", "Analysis", "HOME"}
  T16 = enum32{"Constant", "Ramp", "Step", "Indentation"}
  T17 = enum32{"Uniform Rotation", "Angular Oscillation", "Speed Ramp", "Speed Step"}
  T18 = enum32{"  Acquire  ", "Compare Files Rot", "About", "Service"}
  T19 = enum32{"Coefficient of Friction ", "Friction Force (N)", "Cyclic Friction Force (N)", "Cyclic Coefficient of Friction "}
  T20 = typedef "LAB-IQ UI Data.ctl" = cluster{"Main Home Screen":cluster{"GUI":refnum<vi>, "Platform Settings":refnum<vi>, "Configure":refnum<vi>, "Home":refnum<vi>, "EXIT":refnum<vi>, "service 2":refnum<vi>, "MainPage":refnum<vi>, "Analysis":refnum<vi>}, "Platform Settings":cluster{"mm/s  Surge":refnum<vi>, "Drive Error":refnum<vi>, "Disable Axis Jog Soft Limits":refnum<vi>, "mm/s  Sway":refnum<vi>, "Sway and Surge COM Status":refnum<vi>, "Heave COM Status":refnum<vi>, "Enable Platform":refnum<vi>, "Surge Forward Main":refnum<vi>, "Sway Right Main":refnum<vi>, "Sway Left Main":refnum<vi>, "Heave Down Main":refnum<vi>, "Heave Up main":refnum<vi>, "mm/s Heave":refnum<vi>, "mm/sec":refnum<vi>, "mm":refnum<vi>, "Surge Backward Main":refnum<vi>}, "Analysis Screen":cluster{"Analysis Home":refnum<vi>, "Surface Analysis":refnum<vi>, "Imaging":refnum<vi>, "Image Analysis":refnum<vi>, "Post Analysis":refnum<vi>}, "Config Screen":cluster{"Select Load Head":refnum<vi>, "Notes :":refnum<vi>, "FILE":refnum<vi>, "Sample ID :":refnum<vi>, "Operator ID :":refnum<vi>, "Operator Name :":refnum<vi>, "Auto":refnum<vi>}, "Motion Module":cluster{"zNL":refnum<vi>, "NL disp":refnum<vi>, "Rotary Tab":refnum<vi>, "Motion Direction:  3":refnum<vi>, "E.Velocity 2":refnum<vi>, "e.v/ssr 2":refnum<vi>, "Enter Fixed E.Velocity 2":refnum<vi>, "Enter Final SRR 2":refnum<vi>, "Enter initial SRR 2":refnum<vi>, "Enter Fixed SRR 2":refnum<vi>, "Enter the Final E.Velocity (m/s) 2":refnum<vi>, "Enter initial E.Velocity (m/s) 2":refnum<vi>, "Final Speed (RPM) 3":refnum<vi>, "Initial Speed (RPM) 2":refnum<vi>, "Enter the Final Velocity (m/s) 3":refnum<vi>, "Enter initial Velocity (m/s)  3":refnum<vi>, "Ramp Up 2":refnum<vi>, "TEST SELECTION":refnum<vi>, "SPEED SELECTION : ":refnum<vi>, "Angular Oscillation Set":refnum<vi>, "Traction":refnum<vi>, "Step Speed":refnum<vi>, "StepTable For Load-Speed":refnum<vi>, "StepTable For Speed":refnum<vi>, "Surge Forward MM":refnum<vi>, "Surge Backward MM":refnum<vi>, "M3 Image":refnum<vi>, "String 39":refnum<vi>, "Sway Left MM":refnum<vi>, "Sway Right MM":refnum<vi>, "Disable Axis Jog Soft Limits":refnum<vi>, "mm":refnum<vi>, "Heave Down MM":refnum<vi>, "Heave Up MM":refnum<vi>, "Wear Track Diameter (mm)":refnum<vi>, "Set WTD":refnum<vi>, "HomeScratch":refnum<vi>, "HomeRot":refnum<vi>, "PlaceModule":refnum<vi>, "Enter the Angle (Deg)":refnum<vi>, "Enter the Frequency (Hz)":refnum<vi>, "Motion Mode:":refnum<vi>, "LR Sway":refnum<vi>, "Rot Hor":refnum<vi>, "Scratch":refnum<vi>, "LR Cam":refnum<vi>, "MMBack":refnum<vi>, "MMNext":refnum<vi>, "Rot Ver":refnum<vi>, "Rotary Module Selection":refnum<vi>, "calculate rotary":refnum<vi>, "SPEED SELECTION : rotary":refnum<vi>, "Import 2":refnum<vi>, "Save 2":refnum<vi>, "File Path :  2":refnum<vi>, "String 45":refnum<vi>, "StepTable For Speed 3":refnum<vi>, "Enter the Speed(mm/sec)":refnum<vi>, "Enter the Speed(RPM)":refnum<vi>, "Enter Scratch Speed (mm/s):":refnum<vi>, "SwaySpeed Set":refnum<vi>, "Scartch Offset":refnum<vi>, "Motion type:":refnum<vi>, "HomeScratch 2":refnum<vi>, "Enter Scratch length (mm):":refnum<vi>, "Wear Track Diameter":refnum<vi>, "Rotary Speed Exced":refnum<vi>, "Scratch Mode":refnum<vi>, "No of Scratch":refnum<vi>}, "Environmental control":cluster{"Humidity  Status  3":refnum<vi>, "Low Temp  Status  2":refnum<vi>, "TK4 status 2":refnum<vi>, "Stage Temperature":refnum<vi>, "Sample Temperature":refnum<vi>, "Humidity (Amb)":refnum<vi>, "Clear List":refnum<vi>, "Add to list":refnum<vi>, "Wear":refnum<vi>, "Vibration":refnum<vi>, "Humidity (Chamber)":refnum<vi>, "Temperature (Chamber)":refnum<vi>, "ECR ":refnum<vi>, "Temperature (Amb)":refnum<vi>, "Microphone":refnum<vi>, "Acoustic Emission 3":refnum<vi>, "SNext":refnum<vi>, "APBack":refnum<vi>, "Enter the Temperature (°C):":refnum<vi>, "Enter the Stage \nTemperature (°C):":refnum<vi>, "Enter the Humidity (%Rh):":refnum<vi>, "Low Temp":refnum<vi>, "High Temp":refnum<vi>, "Humidity":refnum<vi>, "Sensors Picked":refnum<vi>}, "About Screen":cluster{"Password":refnum<vi>, "Home Service":refnum<vi>, "Advanced Setting":refnum<vi>, "About Tab":refnum<vi>, "ECR Port:":refnum<vi>, "Ramp Port:":refnum<vi>, "Installation/Replacement completed":refnum<vi>, "Loahead":refnum<vi>, "Heave and Surge COM Port:":refnum<vi>, "Sway COM Port:":refnum<vi>, "Temp Modbus:":refnum<vi>, "Humidity Port:":refnum<vi>, "Edit Gain Constants":refnum<vi>, "Save Gain Constants":refnum<vi>}, "Main Screen":cluster{"Main Screen Tab":refnum<vi>, "Angle and Frequency":refnum<vi>, "Stroke (mm)":refnum<vi>, "Angle (Deg)":refnum<vi>, "Main Speed Tab":refnum<vi>, "MTM MOTOR DISPLAY":refnum<vi>, "Disc Speed (m/sec)":refnum<vi>, "Ball Speed (m/sec)":refnum<vi>, "Disc Speed (RPM)":refnum<vi>, "Ball Speed (RPM)":refnum<vi>, "SPEED TAB":refnum<vi>, "Speed (m/sec)":refnum<vi>, "Set Speed (m/sec)":refnum<vi>, "Speed (RPM)":refnum<vi>, "Set Speed":refnum<vi>, "Time Tab":refnum<vi>, "Time ( HH:MM:SS ) 2":refnum<vi>, "Test Duration":refnum<vi>, "Test Duration 4":refnum<vi>, "TEST CYCLE":refnum<vi>, "TOTAL CYCLES":refnum<vi>, "Set Load (N)":refnum<vi>, "Temp Tabs":refnum<vi>, "Heater":refnum<vi>, "TK4 status":refnum<vi>, "ChamberTemp":refnum<vi>, "SetTmp":refnum<vi>, "Controller  Status":refnum<vi>, "ChamberTemp 2":refnum<vi>, "SetTmp 2":refnum<vi>, "Controller  Status 2":refnum<vi>, "ChamberTemp 3":refnum<vi>, "SetTmp 3":refnum<vi>, "Cooling":refnum<vi>, "Load Communication":refnum<vi>, "Ambient \nTemperature":refnum<vi>, "HumCOMStatus":refnum<vi>, "Ambient\n Humidity":refnum<vi>, "Freq (Hz)":refnum<vi>, "Load En":refnum<vi>, "NLt":refnum<vi>, "zNL 2":refnum<vi>, "Humidity On":refnum<vi>, "humidity disp":refnum<vi>, "Set Humidity":refnum<vi>, "NL disp 2":refnum<vi>, "Humidity On 2":refnum<vi>, "humidity disp 2":refnum<vi>, "Set Humidity 2":refnum<vi>, "NL disp 3":refnum<vi>, "AppLoadSeq scratch":refnum<vi>, "Stop Scratch":refnum<vi>, "ClrLog":refnum<vi>, "Trip Log":refnum<vi>, "STOP":refnum<vi>, "Start Test":refnum<vi>, "Test status":refnum<vi>, "AR Led":refnum<vi>, "Data":refnum<vi>, "Health":refnum<vi>, "Sway COM Status":refnum<vi>, "Heave COM Status":refnum<vi>, "Grp Tab":refnum<vi>, "Sub Graph":refnum<vi>, "SD (mm)":refnum<vi>, "Siliding distance Reset Graph":refnum<vi>, "SDGp":refnum<vi>, "Humidity Reset Graph":refnum<vi>, "HumrGp":refnum<vi>, "Acoustic Emission (mV)":refnum<vi>, "Aqucostic Reset Graph":refnum<vi>, "gACQUOS":refnum<vi>, "ECR RESET":refnum<vi>, "ECR":refnum<vi>, "Temperature Reset":refnum<vi>, "Acoustic Emission (mV) 2":refnum<vi>, "Aqucostic Reset Graph 2":refnum<vi>, "gACQUOS 2":refnum<vi>, "ECR RESET 2":refnum<vi>, "ECR 2":refnum<vi>, "Temperature Reset 2":refnum<vi>, "Temperature (deg c)":refnum<vi>, "Speed Reset Graph":refnum<vi>, "Speed Tab":refnum<vi>, "MTM DISC  SPEED":refnum<vi>, "MTM BALL SPEED":refnum<vi>, "speed mm/sec":refnum<vi>, "Hymidity":refnum<vi>, "Humidity Disable trip":refnum<vi>, "CoF Trip  2":refnum<vi>, "Depth Trip":refnum<vi>, "Weart Deapth":refnum<vi>, "Depth Reset Graph":refnum<vi>, "Weart":refnum<vi>, "Depthz":refnum<vi>, "Depth (µm)":refnum<vi>, "WearGp":refnum<vi>, "NL Trip 2":refnum<vi>, "Load pid":refnum<vi>, "Load Disable Trip":refnum<vi>, "Load Reset Graph":refnum<vi>, "NL Display 4":refnum<vi>, "Main Chart 3":refnum<vi>, "BACK":refnum<vi>, "Depth Trip 2":refnum<vi>, "COF TRIP ":refnum<vi>, "Friction Force (N)":refnum<vi>, "FF Reset Graph":refnum<vi>, "FF Disable Trip":refnum<vi>, "FF TRIP":refnum<vi>, "COF Disable Trip":refnum<vi>, "COF Reset Graph":refnum<vi>, "Start Test Temp":refnum<vi>, "zFF":refnum<vi>, "Friction Force (N) Graph":refnum<vi>, "Coefficient of Friction":refnum<vi>, "Scratch Start Test":refnum<vi>, "FF Tab":refnum<vi>, "Cyclic Friction Force (N)":refnum<vi>, "CZ FF":refnum<vi>, "Cyclic Friction Force (N) Graph":refnum<vi>, "Cyclic Coefficient of Friction":refnum<vi>, "Cyclic FF TRIP":refnum<vi>, "Cyclic FF Disable Trip":refnum<vi>, "cyclic COF Disable Trip":refnum<vi>, "cyclic COF TRIP":refnum<vi>, "cyclic COF Reset Graph":refnum<vi>, "Cyclic FF Reset Graph":refnum<vi>, "Test Trip":refnum<vi>, "Multi Scratch Pass":refnum<vi>, "Scratch Start Recording":refnum<vi>}, "Loading":cluster{"Indentation":refnum<vi>, "Reference Sample":refnum<vi>, "Load Cell Communication Slide":refnum<vi>, "com 3":refnum<vi>, "com":refnum<vi>, "DecaForce COM Status":refnum<vi>, "Update":refnum<vi>, "Clear 3":refnum<vi>, "seq":refnum<vi>, "Stribeck table":refnum<vi>, "Stribeck Table  For loading":refnum<vi>, "Loading Mode":refnum<vi>, "Enter the Final Load (N)":refnum<vi>, "Enter the CoF Trip":refnum<vi>, "Enter the Friction Force Trip":refnum<vi>, "Enter the Normal load Trip":refnum<vi>, "Enter the Load  (N)":refnum<vi>, "KiloForce":refnum<vi>, "DecaForce ":refnum<vi>, "MicroForce":refnum<vi>, "LHBack":refnum<vi>, "LHNext":refnum<vi>, "Enter the Loading Rate (N/min)":refnum<vi>, "Message":refnum<vi>, "Warning 2":refnum<vi>, "SSP 0.75":refnum<vi>, "SSP 0.5":refnum<vi>, "SSP 0.3":refnum<vi>, "Warning":refnum<vi>, "gui GIF":refnum<vi>, "Communication is established":refnum<vi>, "AppLoad 4":refnum<vi>, "Multipoint":refnum<vi>, "Load Selection":refnum<vi>}, "PID":cluster{"Ramp":refnum<vi>, "Vertical load (N)":refnum<vi>, "apply load":refnum<vi>, "apply load 2":refnum<vi>, "Enter ByPass Load":refnum<vi>, "Bypass Load":refnum<vi>, "gFF Rot":refnum<vi>}, "Config Parameters":cluster{"Tab Control 3":refnum<vi>, "Tab Control 19":refnum<vi>, "SAMPLES":refnum<vi>, "Re-initilaize":refnum<vi>, "Filter ON/OFF":refnum<vi>, "TracHomeSurgeOffsetCounts 10MM":refnum<vi>, "TracHomeSwayOffsetCounts 10MM":refnum<vi>, "Acoustic Emission:":refnum<vi>, "Apply Filter (FF)":refnum<vi>, "Filter% 2":refnum<vi>, "Apply Filter (Load)":refnum<vi>, "Filter% ":refnum<vi>, "Sway distance (mm)":refnum<vi>, "Surge distance (mm)":refnum<vi>, "DataSavingLoopDelay(ms)":refnum<vi>, "SAVE 2":refnum<vi>, "Enter Distance":refnum<vi>, "Sway Counts:":refnum<vi>, "Distance (mm): 3":refnum<vi>, "Surge Counts:":refnum<vi>, "Distance (mm): 2":refnum<vi>, "Distance (mm):":refnum<vi>, "Heave Counts:":refnum<vi>, "LRMHomeSurgeOffsetCounts":refnum<vi>, "LRMHomeSwayOffsetCounts":refnum<vi>, "TracHomeSurgeOffsetCounts 20MM":refnum<vi>, "TracHomeSwayOffsetCounts 20MM":refnum<vi>, "RotHomeSwayOffsetCounts":refnum<vi>, "RotHomeSurgeOffsetCounts":refnum<vi>, "Heave distance":refnum<vi>, "Zmm":refnum<vi>, "Heave Pulses/mm":refnum<vi>, "Surge Pulses/mm":refnum<vi>, "Sway Pulses/mm":refnum<vi>, "Heave Pitch":refnum<vi>, "Surge Pitch":refnum<vi>, "Sway Pitch":refnum<vi>, "Heave PPR":refnum<vi>, "Surge PPR":refnum<vi>, "Sway PPR":refnum<vi>, "Tab Control 5":refnum<vi>, "Tab Control 14":refnum<vi>, "Tab Control 26":refnum<vi>, "AE":refnum<vi>, "Heave Loop Delay":refnum<vi>, "Heave PID Speed":refnum<vi>, "Surge Jog Speed":refnum<vi>, "Heave Jog Speed":refnum<vi>, "Sway Loop Delay":refnum<vi>, "Sway PID Speed":refnum<vi>, "Sway Jog Speed":refnum<vi>, "DEPTH TRIP VALUE":refnum<vi>, "LOAD TRIP VALUE":refnum<vi>, "DEPTH TRIP   ENABLE":refnum<vi>, "LOAD TRIP  ENABLE":refnum<vi>, "CYCLIC FF TRIP VALUE":refnum<vi>, "FF TRIP VALUE":refnum<vi>, "CYCLIC CoF TRIP VALUE":refnum<vi>, "COF TRIP VALUE":refnum<vi>, "CYCLIC COF TRIP  ENABLE":refnum<vi>, "CYCLIC FF TRIP  ENABLE":refnum<vi>, "FF TRIP  ENABLE":refnum<vi>, "COF TRIP  ENABLE":refnum<vi>, "JOG TRIP LOAD VALUE (N)":refnum<vi>, "Rotary Vertical":refnum<vi>, "Traction":refnum<vi>, "Scratch":refnum<vi>, "LRM CAM":refnum<vi>, "Sway LRM":refnum<vi>, "Rotary Horizontal":refnum<vi>}, "Loading Com Port":cluster{"ClearAll":refnum<vi>, "Mz(Nm)":refnum<vi>, "My(Nm)":refnum<vi>, "Mx(Nm)":refnum<vi>, "Save Dwell":refnum<vi>, "Acq Delay (ms)":refnum<vi>, "Burst Delay (ms)":refnum<vi>, "model":refnum<vi>, "SN":refnum<vi>, "FFx(N)":refnum<vi>, "Sensor IP":refnum<vi>, "Port":refnum<vi>, "FFy(N)":refnum<vi>, "Load(N)":refnum<vi>, "delete Handle":refnum<vi>, "Create Handle":refnum<vi>, "ft_data":refnum<vi>, "ft_range":refnum<vi>, "ft_data 2":refnum<vi>, "stop 6":refnum<vi>, "running_flag":refnum<vi>, "ft_udp_handle":refnum<vi>, "get-data-return":refnum<vi>, "get-range-return":refnum<vi>, "zero-return":refnum<vi>, "filter-return":refnum<vi>, "initial-return":refnum<vi>, "deleteHandle-result":refnum<vi>, "Load Cell Temp":refnum<vi>, "Load Cell":refnum<vi>, "ZeroAll":refnum<vi>, "FORCE (N)":refnum<vi>, "TORQUE (N-m)":refnum<vi>, "Load Cell Link":refnum<vi>}, "Heave AND Surge":cluster{"SURGE POSE":refnum<vi>, "error out Read":refnum<vi>, "HEAVE POSE":refnum<vi>, "State":refnum<vi>, "Homed":refnum<vi>, "Sequence ID":refnum<vi>, "error out Write":refnum<vi>, "faultCode":refnum<vi>, "Ack ID":refnum<vi>, "SPEED":refnum<vi>, "Distance":refnum<vi>, "Mode Command":refnum<vi>, "Heave and Surge Read":refnum<vi>, "Read Heave Temp":refnum<vi>, "Spare 15":refnum<vi>, "Spare 14":refnum<vi>, "Spare 13":refnum<vi>, "Spare 12":refnum<vi>, "Spare 11":refnum<vi>, "Spare 10":refnum<vi>, "Spare 9":refnum<vi>, "Spare 8":refnum<vi>, "Spare 7":refnum<vi>, "Spare 4":refnum<vi>, "Spare 3":refnum<vi>, "Spare 2":refnum<vi>, "Humidity":refnum<vi>, "Temp":refnum<vi>, "Node Id":refnum<vi>, "Spare 1":refnum<vi>, "SPARE 4":refnum<vi>, "SPARE 3":refnum<vi>, "SPARE 2":refnum<vi>, "SPARE 1":refnum<vi>, "fwMajor":refnum<vi>, "fwMinor":refnum<vi>, "Manual Write":refnum<vi>, "Heave and Surge Write":refnum<vi>, "SPARE 5":refnum<vi>, "Reserved ":refnum<vi>, "SPARE 8":refnum<vi>, "SPARE 6":refnum<vi>, "SPARE 7":refnum<vi>, "SPARE 17":refnum<vi>, "SPARE 16":refnum<vi>, "SPARE 15":refnum<vi>, "SPARE 14":refnum<vi>, "SPARE 13":refnum<vi>, "SPARE 12":refnum<vi>, "SPARE 11":refnum<vi>, "SPARE 10":refnum<vi>, "SPARE 9":refnum<vi>, "System UPTIME":refnum<vi>, "Missed Packets":refnum<vi>, "faultCode Surge Right":refnum<vi>, "faultCode Surge Left":refnum<vi>, "faultCode Heave":refnum<vi>, "UPLINK HEAVE":refnum<vi>, "DOWNLINK HEAVE":refnum<vi>}, "New PID LOGIC":cluster{"Fine Tune Zone":refnum<vi>, "PID SDelay":refnum<vi>, "Max_pos_limit":refnum<vi>, "Min_pos_limit":refnum<vi>, "i_limit":refnum<vi>, "pct_scale":refnum<vi>, "Deadband":refnum<vi>, "Kd":refnum<vi>, "Ki":refnum<vi>, "Kp":refnum<vi>, "Current Position":refnum<vi>, "Set Load":refnum<vi>, "Current Load":refnum<vi>, "Pulse delta":refnum<vi>, "Init Step":refnum<vi>, "Max Step Linit":refnum<vi>, "min_deadband_floor":refnum<vi>, "dynamic_spindle_noise_scalar":refnum<vi>, "min_finetune_floor":refnum<vi>, "filter_alpha":refnum<vi>, "PID":refnum<vi>}, "SWAY ":cluster{"fwMajor":refnum<vi>, "Homed":refnum<vi>, "Rotary POSE":refnum<vi>, "State":refnum<vi>, "SWAY POSE":refnum<vi>, "Ack ID":refnum<vi>, "faultCode":refnum<vi>, "Node Id":refnum<vi>, "fwMinor":refnum<vi>, "Spare 6":refnum<vi>, "Spare 5":refnum<vi>, "Spare 4":refnum<vi>, "Spare 3":refnum<vi>, "Spare 2":refnum<vi>, "Spare 1":refnum<vi>, "Spare 7":refnum<vi>, "SPARE  5":refnum<vi>, "error out Write  SWAY ":refnum<vi>, "error out Read SWAY ":refnum<vi>, "Manual Write SWAY ":refnum<vi>, "SWAY WRITE":refnum<vi>, "SPARE  4":refnum<vi>, "SPARE  3":refnum<vi>, "SPARE 2":refnum<vi>, "SPARE 1":refnum<vi>, "Spare 15":refnum<vi>, "Spare 14":refnum<vi>, "Spare 13":refnum<vi>, "Spare 12":refnum<vi>, "Spare 11":refnum<vi>, "Spare 9":refnum<vi>, "Spare 8":refnum<vi>, "SPEED":refnum<vi>, "Distance":refnum<vi>, "Mode Command":refnum<vi>, "Sequence ID":refnum<vi>, "SWAY READ":refnum<vi>, "Spare 10":refnum<vi>, "Read SWAY Temp":refnum<vi>, "faultCode Sway ":refnum<vi>, "Missed Packets":refnum<vi>, "System UPTIME sway":refnum<vi>, "SPARE 6":refnum<vi>, "SPARE 7":refnum<vi>, "SPARE 9":refnum<vi>, "SPARE 11":refnum<vi>, "SPARE 10":refnum<vi>, "SPARE 8":refnum<vi>, "SPARE 13":refnum<vi>, "SPARE 12":refnum<vi>, "SPARE 17":refnum<vi>, "SPARE 16":refnum<vi>, "SPARE 15":refnum<vi>, "SPARE 14":refnum<vi>, "Reserved":refnum<vi>, "faultCode Rotary":refnum<vi>, "UPLINK SWAY":refnum<vi>, "DOWNLINK SWAY":refnum<vi>}, "Analysis Screen":cluster{"Analysis Home":refnum<vi>, "Refresh 2":refnum<vi>, "MEAN 4":refnum<vi>, "SD 4":refnum<vi>, "VARIANCE 4":refnum<vi>, "MEAN  3":refnum<vi>, "SD  3":refnum<vi>, "VARIANCE  3":refnum<vi>, "MEAN 2":refnum<vi>, "SD  2":refnum<vi>, "VARIANCE 2":refnum<vi>, "MEAN":refnum<vi>, "SD":refnum<vi>, "VARIANCE":refnum<vi>, "File 4 Discription":refnum<vi>, "OPEN 4":refnum<vi>, "File Name 4":refnum<vi>, "OPEN 3":refnum<vi>, "File 3 Discription":refnum<vi>, "File Name 3":refnum<vi>, "Y-AXIS":refnum<vi>, "X-AXIS":refnum<vi>, "XY Graph":refnum<vi>, "File Name 2":refnum<vi>, "File Name 1":refnum<vi>, "OPEN 2":refnum<vi>, "OPEN 1":refnum<vi>, "File 1 Discription ":refnum<vi>, "File 2 Discription":refnum<vi>, "Export":refnum<vi>, "File Format":refnum<vi>}, "Traction":cluster{"faultCode Traction 2":refnum<vi>, "faultCode Traction 1":refnum<vi>, "Missed Packets":refnum<vi>, "System UPTIME Traction":refnum<vi>, "SPARE 17":refnum<vi>, "SPARE 16":refnum<vi>, "SPARE 15":refnum<vi>, "SPARE 14":refnum<vi>, "SPARE 13":refnum<vi>, "SPARE 12":refnum<vi>, "SPARE 11":refnum<vi>, "SPARE 10":refnum<vi>, "SPARE 9":refnum<vi>, "SPARE 8":refnum<vi>, "SPARE 7":refnum<vi>, "SPARE 6":refnum<vi>, "Reserved":refnum<vi>, "SPARE  5":refnum<vi>, "Manual Write TRACTION":refnum<vi>, "TRACTION WRITE":refnum<vi>, "SPARE  4":refnum<vi>, "SPARE  3":refnum<vi>, "SPARE 2":refnum<vi>, "SPARE 1":refnum<vi>, "Spare 7":refnum<vi>, "Spare 6":refnum<vi>, "Spare 5":refnum<vi>, "Spare 4":refnum<vi>, "Spare 2":refnum<vi>, "Spare 1":refnum<vi>, "Node Id":refnum<vi>, "Read TRACTION Temp":refnum<vi>, "fwMinor":refnum<vi>, "fwMajor":refnum<vi>, "faultCode":refnum<vi>, "TRACTION POSE":refnum<vi>, "TRACTION POSE 2":refnum<vi>, "Homed":refnum<vi>, "State":refnum<vi>, "Ack ID":refnum<vi>, "SPEED":refnum<vi>, "Distance":refnum<vi>, "Mode Command":refnum<vi>, "Sequence ID":refnum<vi>, "error out Read TRACTION":refnum<vi>, "error out Write  TRACTION":refnum<vi>, "TRACTION READ":refnum<vi>, "Spare 3":refnum<vi>, "Downlink traction":refnum<vi>, "Uplink Traction":refnum<vi>}, "Traction reciepe":cluster{"SRR Sweep Range (%) Stribeck":refnum<vi>, "Traction Receipe":refnum<vi>, "Total Execution Time":refnum<vi>, "Total Steps":refnum<vi>, "Duration / Step (s)  Stribeck":refnum<vi>, "STRIBECK Fixed SRR List (%)":refnum<vi>, "Duration / Step (s) Traction":refnum<vi>, "SRR Sweep Range (%) traction":refnum<vi>, "Rolling Speed (mm/s)":refnum<vi>, "Temperature Stages (°C)":refnum<vi>, "Ball Load (N)":refnum<vi>, "Lubricant Name":refnum<vi>, "Profile File Name":refnum<vi>, "SET entrainment Velocity":refnum<vi>, "Test Array Size":refnum<vi>, "SRR INDEX [ STRIBECK]":refnum<vi>, "Stribeck Size":refnum<vi>, "SET SRR":refnum<vi>, "ELAPSED TIMER ":refnum<vi>, "BALL SET RPM":refnum<vi>, "DISC SET RPM":refnum<vi>, "SET LOAD":refnum<vi>, "TEMPERATURE READ":refnum<vi>, "SET TEMPERATURE":refnum<vi>, "Traction Size":refnum<vi>, "DISC SPEED (rpm)":refnum<vi>, "BALL SPEED (rpm)":refnum<vi>, "BALL WEAR TRACK":refnum<vi>, "DISC WEARTRACK":refnum<vi>, "SRR INDEX [ TRACTION]":refnum<vi>, "Start Index Type":refnum<vi>, "Enum - Menu":refnum<vi>, "Ball (mm/sec)":refnum<vi>, "Disc (mm/sec)":refnum<vi>}, "Traction Control":cluster{"HomeTraction":refnum<vi>, "Demo Mode Display":refnum<vi>, "Traction Message":refnum<vi>, "Traction Step Update Details":refnum<vi>, "Main Tab sequence for selection":refnum<vi>, "Ramp Tab":refnum<vi>, "e.v/ssr":refnum<vi>, "Enter Fixed E.Velocity":refnum<vi>, "Enter Final SRR":refnum<vi>, "Enter initial SRR":refnum<vi>, "Enter Fixed SRR":refnum<vi>, "Enter the Final E.Velocity (m/s)":refnum<vi>, "Enter initial E.Velocity (m/s)":refnum<vi>, "Ball WTD":refnum<vi>, "E.Velocity":refnum<vi>, "Enter the Final Velocity (m/s)":refnum<vi>, "Enter initial Velocity (m/s)":refnum<vi>, "Ramp Up   Disc":refnum<vi>, "Initial DiscSpeed (RPM)":refnum<vi>, "Final Speed (RPM) Ball":refnum<vi>, "Final Speed (RPM)":refnum<vi>, "Initial Speed (RPM) Ball":refnum<vi>, "Enter the Final Velocity (m/s) Ball":refnum<vi>, "Enter initial Velocity (m/s) Ball":refnum<vi>, "Ramp Up":refnum<vi>, "ExceedBallSpeed step":refnum<vi>, "ExceedDiscSpeed":refnum<vi>, "BallSpeed Exceed Indication":refnum<vi>, "Apply":refnum<vi>, "SPEED SELECTION : MTM":refnum<vi>, "SPEED SELECTION : MTM 2":refnum<vi>, "TEST SELECTION (MTM)":refnum<vi>, "MTM Test Selection":refnum<vi>, "File Path Tab":refnum<vi>, "File Path String":refnum<vi>, "Save":refnum<vi>, "Save  2":refnum<vi>, "Import ":refnum<vi>, "File Path :":refnum<vi>, "Step Sequence Indication Tab":refnum<vi>, "Step Sequence Indication":refnum<vi>, "Calculate Step":refnum<vi>, "StepTable":refnum<vi>, "ExceedDiscSpeed  Cinstant Speed":refnum<vi>, "ExceedBallSpeed Constant":refnum<vi>, "TEST SELECTION (MTM) 2":refnum<vi>, "SPEED SELECTION : MTM 3":refnum<vi>, "MTM Test Selection 2":refnum<vi>, "Enter the Speed (m/sec): ":refnum<vi>, "Enter the Speed (m/sec):  2":refnum<vi>, "Enter the Speed (RPM):":refnum<vi>, "Lower Spped ":refnum<vi>, "Upper":refnum<vi>, "Enter the Speed (RPM):Ball":refnum<vi>, "Disc Motion Direction: ":refnum<vi>, "Ball Motion Direction :":refnum<vi>, "Motion Mode: ":refnum<vi>, "Wear Track Diameter (mm) ":refnum<vi>, "Disc Speed Indicator":refnum<vi>, "ExceedBallSpeed":refnum<vi>}, "Acquostic":cluster{"Last Config Rejected ":refnum<vi>, "rx command count":refnum<vi>, "Current Filter Id":refnum<vi>, "Isolated Gain":refnum<vi>, "DAQ Status":refnum<vi>, "error out":refnum<vi>, "error in (no error)":refnum<vi>, "Uplink Packet":refnum<vi>, "data out":refnum<vi>, "Downlink Packet":refnum<vi>, "Gains":refnum<vi>, "Manual Write Acquostic":refnum<vi>, "Acoustic Graphs":refnum<vi>}}
  T21 = typedef "init queue out loop.ctl" = cluster{"UI Loop":refnum<queue>, "LOAD COM LOOP ":refnum<queue>, "SWAY MOTOR COM LOOP":refnum<queue>, "HEAVE MOTOR COM LOOP":refnum<queue>, "TEMPERATURE COM LOOP":refnum<queue>, "RAMP MOTOR COM LOOP":refnum<queue>, "ECR PORT":refnum<queue>, "HUMIDITY COM PORT":refnum<queue>, "PROGRAM LOOP":refnum<queue>, "MONITOR LOOP":refnum<queue>, "REPORT":refnum<queue>, "LOAD PID":refnum<queue>, "ACOUSTIC":refnum<queue>}
  T22 = typedef "XDNodeRunTimeDep.lvlib/timing_clust.ctl" = cluster{"Expected End [f-1]":u64, "Actual End [f-1]":u64, "Finished Late? [f-1]":bool, "Expected End [i-1]":u64, "Actual End [i-1]":u64, "Finished Late? [i-1]":bool, "Expected Start [i]":u64, "Actual Start [i]":u64, "Expected Start [f]":u64, "Actual Start [f]":u64, "Source Name":string, "Structure Name":string, "Period":i64, "Deadline":i64, "Offset":i64, "Start":i64, "Priority":i32, "Timeout":i32, "Mode":T23, "Wakeup Reason":T24, "Error":errorcluster, "Source Type":string, "Secondary Source Type":string, "Global End Time":u64, "Global Start Time":u64, "Frame Duration":u64, "Iteration Duration":u64, "Assigned CPU":i32, "I/O Scan Engine Mode":u32}
  T23 = typedef "XDNodeRunTimeDep.lvlib/nitl_modes.ctl" = enum32{"No Change", "Process missed periods, maintain original phase", "Discard missed periods, maintain original phase", "Process missed periods, ignore original phase", "Discard missed periods, ignore original phase"}
  T24 = typedef "XDNodeRunTimeDep.lvlib/wakeup.ctl" = enum32{"Normal", "Aborted", "Asynchronous wakeup", "Timing source error", "Timed loop error", "Timeout"}
  T25 = typedef "Traction Read enum.ctl" = enum16{"INIT", "READ", "CLOSE", "REINIT", ""}
  T26 = typedef "Traction Write enum.ctl" = enum16{"INIT", "WRITE", "CLOSE", "REINIT"}
  T27 = typedef "Read Main Enum.ctl" = enum16{"INIT", "READ", "RE-INIT", "CLOSE"}
  T28 = typedef "Write Main Enum.ctl" = enum16{"INIT", "WRITE", "RE-INIT", "CLOSE"}
  T29 = typedef "Heave Right enum.ctl" = enum16{"INIT", "READ", "CLOSE", "REINIT", ""}
  T30 = typedef "Heave Write enum.ctl" = enum16{"INIT", "WRITE", "CLOSE", "REINIT"}
  T31 = enum8{"Enabled", "Disabled", "Disabled and Grayed Out"}
  T32 = typedef "Load cell Enum.ctl" = enum16{"Init", "set UDP", "Read Info", "set Low Pass Filter", "Set Zero", "get data", "close", "REInit"}
  T33 = typedef "Sway Write enum.ctl" = enum16{"INIT", "WRITE", "CLOSE", "REINIT"}
  T34 = typedef "Sway Right enum.ctl" = enum16{"INIT", "READ", "CLOSE", "REINIT", ""}
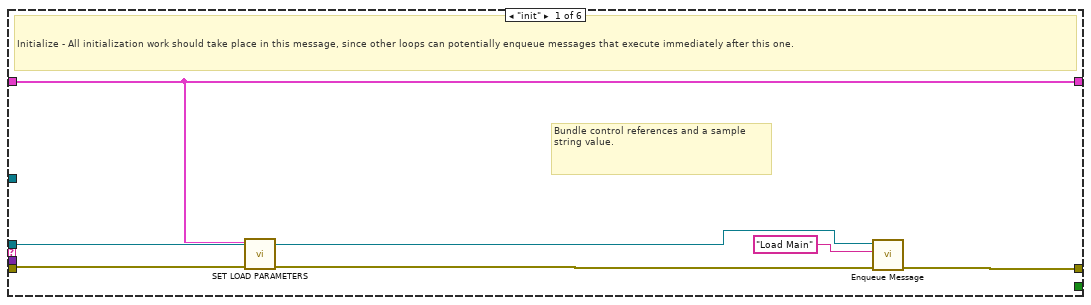
[diagram p2: hidden frame]
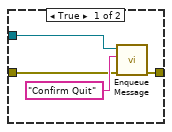
[diagram p3: hidden frame]
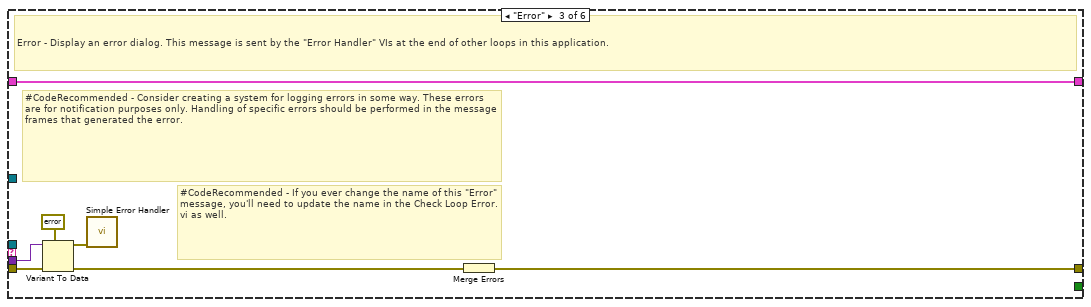
[diagram p4: hidden frame]
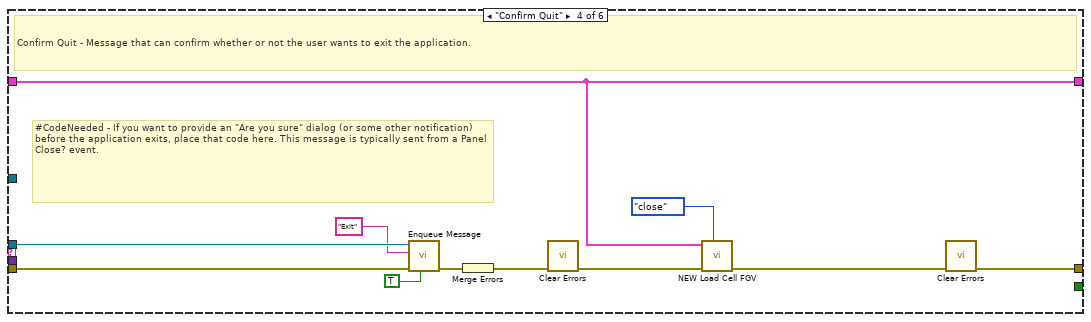
[diagram p5: hidden frame]
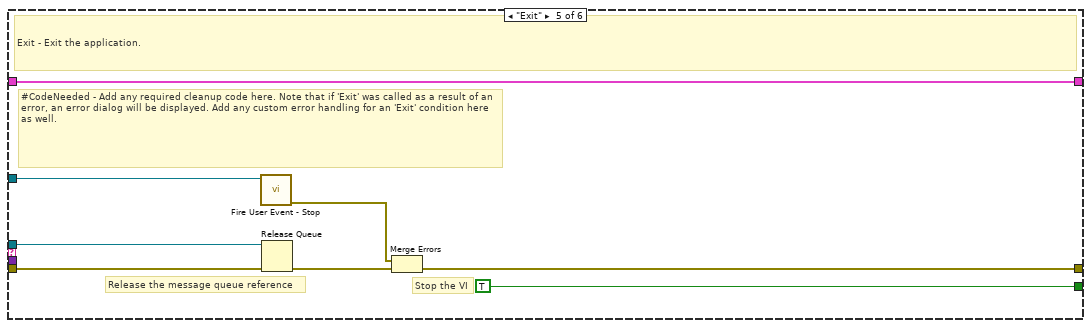
[diagram p6: hidden frame]
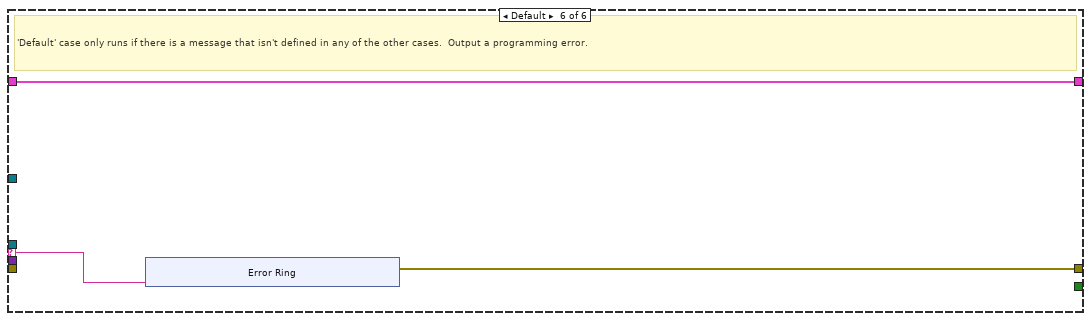
[diagram p7: hidden frame]
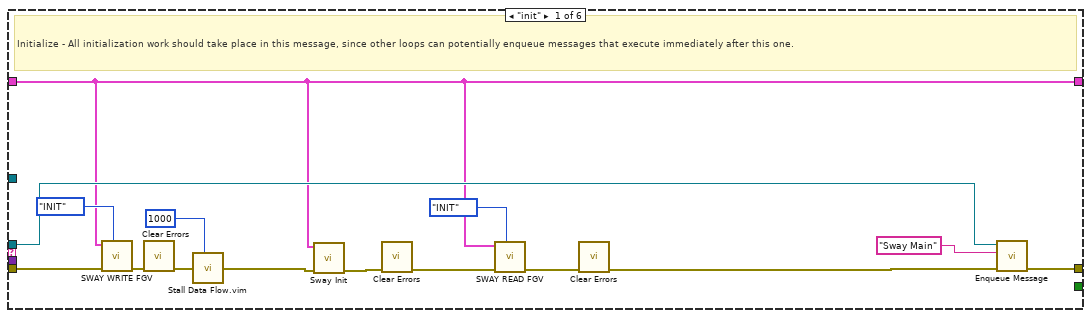
[diagram p8: hidden frame]
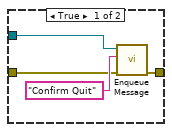
[diagram p11: hidden frame]
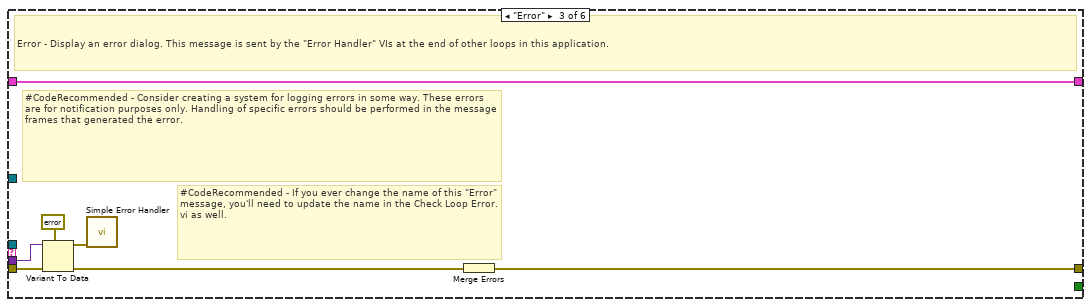
[diagram p12: hidden frame]
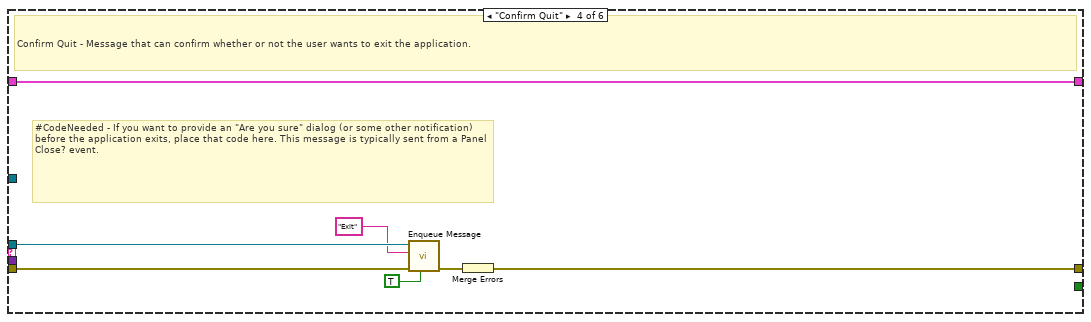
[diagram p13: hidden frame]
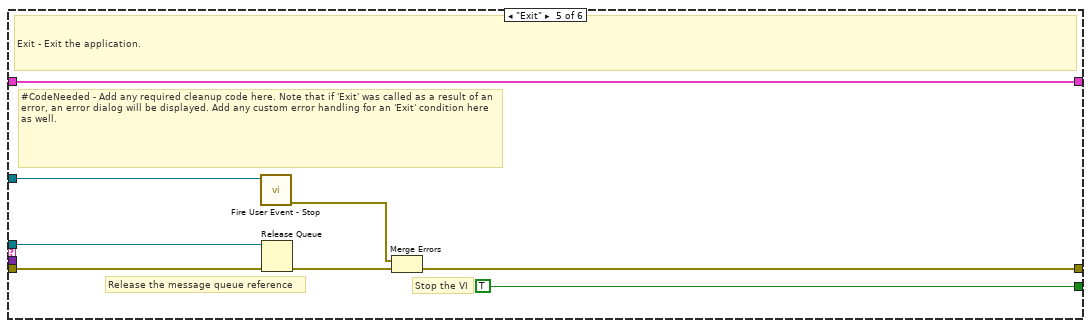
[diagram p14: hidden frame]
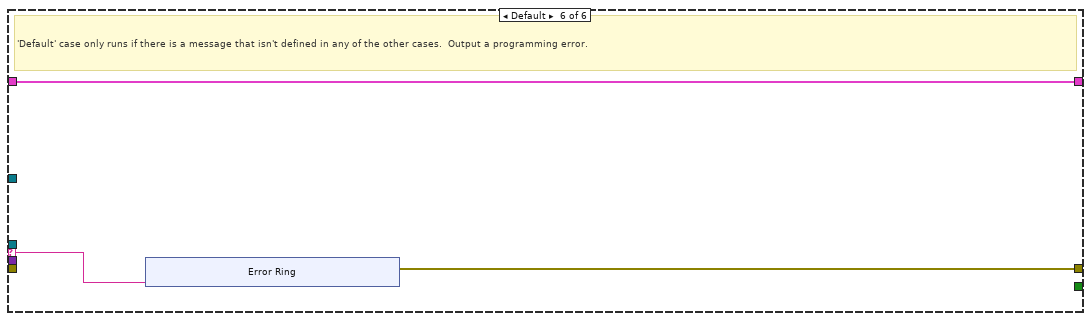
[diagram p15: hidden frame]
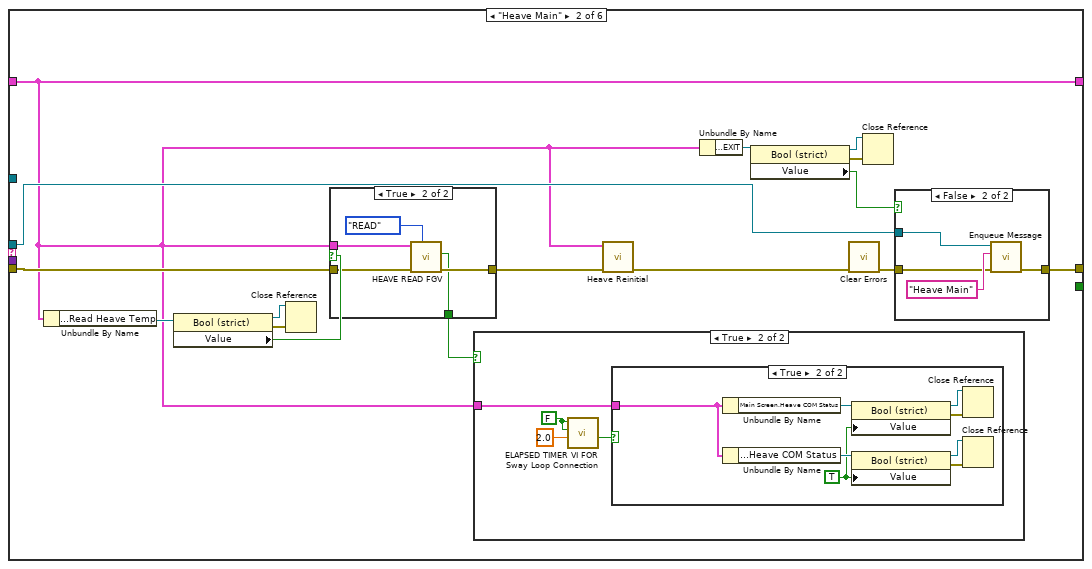
[diagram p16: hidden frame]
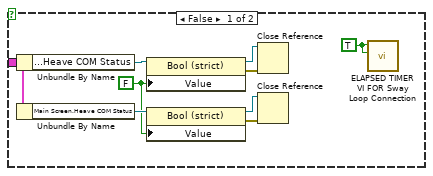
[diagram p17: hidden frame]
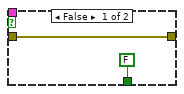
[diagram p19: hidden frame]
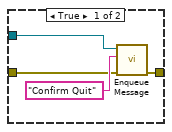
[diagram p20: hidden frame]
diagram:
  w17 = 0.0 ("prev_error_out")
  n1 = flat-sequence {
    tunnel: [w68] -> w55
    tunnel: T20 {"Main Home Screen"={"GUI"=refnum, "Platform Settings"=refnum, "Configure"=refnum, "Home"=refnum, "EXIT"=refnum, "service 2"=refnum, "MainPage"=refnum, "Analysis"=refnum}, "Platform Settings"={"mm/s  Surge"=refnum, "Drive Error"=refnum, "Disable Axis Jog Soft Limits"=refnum, "mm/s  Sway"=refnum, "Sway and Surge COM Status"=refnum, "Heave COM Status"=refnum, "Enable Platform"=refnum, "Surge Forward Main"=refnum, "Sway Right Main"=refnum, "Sway Left Main"=refnum, "Heave Down Main"=refnum, "Heave Up main"=refnum, "mm/s Heave"=refnum, "mm/sec"=refnum, "mm"=refnum, "Surge Backward Main"=refnum}, "Analysis Screen"={"Analysis Home"=refnum, "Surface Analysis"=refnum, "Imaging"=refnum, "Image Analysis"=refnum, "Post Analysis"=refnum}, "Config Screen"={"Select Load Head"=refnum, "Notes :"=refnum, "FILE"=refnum, "Sample ID :"=refnum, "Operator ID :"=refnum, "Operator Name :"=refnum, "Auto"=refnum}, "Motion Module"={"zNL"=refnum, "NL disp"=refnum, "Rotary Tab"=refnum, "Motion Direction:  3"=refnum, "E.Velocity 2"=refnum, "e.v/ssr 2"=refnum, "Enter Fixed E.Velocity 2"=refnum, "Enter Final SRR 2"=refnum, "Enter initial SRR 2"=refnum, "Enter Fixed SRR 2"=refnum, "Enter the Final E.Velocity (m/s) 2"=refnum, "Enter initial E.Velocity (m/s) 2"=refnum, "Final Speed (RPM) 3"=refnum, "Initial Speed (RPM) 2"=refnum, "Enter the Final Velocity (m/s) 3"=refnum, "Enter initial Velocity (m/s)  3"=refnum, "Ramp Up 2"=refnum, "TEST SELECTION"=refnum, "SPEED SELECTION : "=refnum, "Angular Oscillation Set"=refnum, "Traction"=refnum, "Step Speed"=refnum, "StepTable For Load-Speed"=refnum, "StepTable For Speed"=refnum, "Surge Forward MM"=refnum, "Surge Backward MM"=refnum, "M3 Image"=refnum, "String 39"=refnum, "Sway Left MM"=refnum, "Sway Right MM"=refnum, "Disable Axis Jog Soft Limits"=refnum, "mm"=refnum, "Heave Down MM"=refnum, "Heave Up MM"=refnum, "Wear Track Diameter (mm)"=refnum, "Set WTD"=refnum, "HomeScratch"=refnum, "HomeRot"=refnum, "PlaceModule"=refnum, "Enter the Angle (Deg)"=refnum, "Enter the Frequency (Hz)"=refnum, "Motion Mode:"=refnum, "LR Sway"=refnum, "Rot Hor"=refnum, "Scratch"=refnum, "LR Cam"=refnum, "MMBack"=refnum, "MMNext"=refnum, "Rot Ver"=refnum, "Rotary Module Selection"=refnum, "calculate rotary"=refnum, "SPEED SELECTION : rotary"=refnum, "Import 2"=refnum, "Save 2"=refnum, "File Path :  2"=refnum, "String 45"=refnum, "StepTable For Speed 3"=refnum, "Enter the Speed(mm/sec)"=refnum, "Enter the Speed(RPM)"=refnum, "Enter Scratch Speed (mm/s):"=refnum, "SwaySpeed Set"=refnum, "Scartch Offset"=refnum, "Motion type:"=refnum, "HomeScratch 2"=refnum, "Enter Scratch length (mm):"=refnum, "Wear Track Diameter"=refnum, "Rotary Speed Exced"=refnum, "Scratch Mode"=refnum, "No of Scratch"=refnum}, "Environmental control"={"Humidity  Status  3"=refnum, "Low Temp  Status  2"=refnum, "TK4 status 2"=refnum, "Stage Temperature"=refnum, "Sample Temperature"=refnum, "Humidity (Amb)"=refnum, "Clear List"=refnum, "Add to list"=refnum, "Wear"=refnum, "Vibration"=refnum, "Humidity (Chamber)"=refnum, "Temperature (Chamber)"=refnum, "ECR "=refnum, "Temperature (Amb)"=refnum, "Microphone"=refnum, "Acoustic Emission 3"=refnum, "SNext"=refnum, "APBack"=refnum, "Enter the Temperature (°C):"=refnum, "Enter the Stage \nTemperature (°C):"=refnum, "Enter the Humidity (%Rh):"=refnum, "Low Temp"=refnum, "High Temp"=refnum, "Humidity"=refnum, "Sensors Picked"=refnum}, "About Screen"={"Password"=refnum, "Home Service"=refnum, "Advanced Setting"=refnum, "About Tab"=refnum, "ECR Port:"=refnum, "Ramp Port:"=refnum, "Installation/Replacement completed"=refnum, "Loahead"=refnum, "Heave and Surge COM Port:"=refnum, "Sway COM Port:"=refnum, "Temp Modbus:"=refnum, "Humidity Port:"=refnum, "Edit Gain Constants"=refnum, "Save Gain Constants"=refnum}, "Main Screen"={"Main Screen Tab"=refnum, "Angle and Frequency"=refnum, "Stroke (mm)"=refnum, "Angle (Deg)"=refnum, "Main Speed Tab"=refnum, "MTM MOTOR DISPLAY"=refnum, "Disc Speed (m/sec)"=refnum, "Ball Speed (m/sec)"=refnum, "Disc Speed (RPM)"=refnum, "Ball Speed (RPM)"=refnum, "SPEED TAB"=refnum, "Speed (m/sec)"=refnum, "Set Speed (m/sec)"=refnum, "Speed (RPM)"=refnum, "Set Speed"=refnum, "Time Tab"=refnum, "Time ( HH:MM:SS ) 2"=refnum, "Test Duration"=refnum, "Test Duration 4"=refnum, "TEST CYCLE"=refnum, "TOTAL CYCLES"=refnum, "Set Load (N)"=refnum, "Temp Tabs"=refnum, "Heater"=refnum, "TK4 status"=refnum, "ChamberTemp"=refnum, "SetTmp"=refnum, "Controller  Status"=refnum, "ChamberTemp 2"=refnum, "SetTmp 2"=refnum, "Controller  Status 2"=refnum, "ChamberTemp 3"=refnum, "SetTmp 3"=refnum, "Cooling"=refnum, "Load Communication"=refnum, "Ambient \nTemperature"=refnum, "HumCOMStatus"=refnum, "Ambient\n Humidity"=refnum, "Freq (Hz)"=refnum, "Load En"=refnum, "NLt"=refnum, "zNL 2"=refnum, "Humidity On"=refnum, "humidity disp"=refnum, "Set Humidity"=refnum, "NL disp 2"=refnum, "Humidity On 2"=refnum, "humidity disp 2"=refnum, "Set Humidity 2"=refnum, "NL disp 3"=refnum, "AppLoadSeq scratch"=refnum, "Stop Scratch"=refnum, "ClrLog"=refnum, "Trip Log"=refnum, "STOP"=refnum, "Start Test"=refnum, "Test status"=refnum, "AR Led"=refnum, "Data"=refnum, "Health"=refnum, "Sway COM Status"=refnum, "Heave COM Status"=refnum, "Grp Tab"=refnum, "Sub Graph"=refnum, "SD (mm)"=refnum, "Siliding distance Reset Graph"=refnum, "SDGp"=refnum, "Humidity Reset Graph"=refnum, "HumrGp"=refnum, "Acoustic Emission (mV)"=refnum, "Aqucostic Reset Graph"=refnum, "gACQUOS"=refnum, "ECR RESET"=refnum, "ECR"=refnum, "Temperature Reset"=refnum, "Acoustic Emission (mV) 2"=refnum, "Aqucostic Reset Graph 2"=refnum, "gACQUOS 2"=refnum, "ECR RESET 2"=refnum, "ECR 2"=refnum, "Temperature Reset 2"=refnum, "Temperature (deg c)"=refnum, "Speed Reset Graph"=refnum, "Speed Tab"=refnum, "MTM DISC  SPEED"=refnum, "MTM BALL SPEED"=refnum, "speed mm/sec"=refnum, "Hymidity"=refnum, "Humidity Disable trip"=refnum, "CoF Trip  2"=refnum, "Depth Trip"=refnum, "Weart Deapth"=refnum, "Depth Reset Graph"=refnum, "Weart"=refnum, "Depthz"=refnum, "Depth (µm)"=refnum, "WearGp"=refnum, "NL Trip 2"=refnum, "Load pid"=refnum, "Load Disable Trip"=refnum, "Load Reset Graph"=refnum, "NL Display 4"=refnum, "Main Chart 3"=refnum, "BACK"=refnum, "Depth Trip 2"=refnum, "COF TRIP "=refnum, "Friction Force (N)"=refnum, "FF Reset Graph"=refnum, "FF Disable Trip"=refnum, "FF TRIP"=refnum, "COF Disable Trip"=refnum, "COF Reset Graph"=refnum, "Start Test Temp"=refnum, "zFF"=refnum, "Friction Force (N) Graph"=refnum, "Coefficient of Friction"=refnum, "Scratch Start Test"=refnum, "FF Tab"=refnum, "Cyclic Friction Force (N)"=refnum, "CZ FF"=refnum, "Cyclic Friction Force (N) Graph"=refnum, "Cyclic Coefficient of Friction"=refnum, "Cyclic FF TRIP"=refnum, "Cyclic FF Disable Trip"=refnum, "cyclic COF Disable Trip"=refnum, "cyclic COF TRIP"=refnum, "cyclic COF Reset Graph"=refnum, "Cyclic FF Reset Graph"=refnum, "Test Trip"=refnum, "Multi Scratch Pass"=refnum, "Scratch Start Recording"=refnum}, "Loading"={"Indentation"=refnum, "Reference Sample"=refnum, "Load Cell Communication Slide"=refnum, "com 3"=refnum, "com"=refnum, "DecaForce COM Status"=refnum, "Update"=refnum, "Clear 3"=refnum, "seq"=refnum, "Stribeck table"=refnum, "Stribeck Table  For loading"=refnum, "Loading Mode"=refnum, "Enter the Final Load (N)"=refnum, "Enter the CoF Trip"=refnum, "Enter the Friction Force Trip"=refnum, "Enter the Normal load Trip"=refnum, "Enter the Load  (N)"=refnum, "KiloForce"=refnum, "DecaForce "=refnum, "MicroForce"=refnum, "LHBack"=refnum, "LHNext"=refnum, "Enter the Loading Rate (N/min)"=refnum, "Message"=refnum, "Warning 2"=refnum, "SSP 0.75"=refnum, "SSP 0.5"=refnum, "SSP 0.3"=refnum, "Warning"=refnum, "gui GIF"=refnum, "Communication is established"=refnum, "AppLoad 4"=refnum, "Multipoint"=refnum, "Load Selection"=refnum}, "PID"={"Ramp"=refnum, "Vertical load (N)"=refnum, "apply load"=refnum, "apply load 2"=refnum, "Enter ByPass Load"=refnum, "Bypass Load"=refnum, "gFF Rot"=refnum}, "Config Parameters"={"Tab Control 3"=refnum, "Tab Control 19"=refnum, "SAMPLES"=refnum, "Re-initilaize"=refnum, "Filter ON/OFF"=refnum, "TracHomeSurgeOffsetCounts 10MM"=refnum, "TracHomeSwayOffsetCounts 10MM"=refnum, "Acoustic Emission:"=refnum, "Apply Filter (FF)"=refnum, "Filter% 2"=refnum, "Apply Filter (Load)"=refnum, "Filter% "=refnum, "Sway distance (mm)"=refnum, "Surge distance (mm)"=refnum, "DataSavingLoopDelay(ms)"=refnum, "SAVE 2"=refnum, "Enter Distance"=refnum, "Sway Counts:"=refnum, "Distance (mm): 3"=refnum, "Surge Counts:"=refnum, "Distance (mm): 2"=refnum, "Distance (mm):"=refnum, "Heave Counts:"=refnum, "LRMHomeSurgeOffsetCounts"=refnum, "LRMHomeSwayOffsetCounts"=refnum, "TracHomeSurgeOffsetCounts 20MM"=refnum, "TracHomeSwayOffsetCounts 20MM"=refnum, "RotHomeSwayOffsetCounts"=refnum, "RotHomeSurgeOffsetCounts"=refnum, "Heave distance"=refnum, "Zmm"=refnum, "Heave Pulses/mm"=refnum, "Surge Pulses/mm"=refnum, "Sway Pulses/mm"=refnum, "Heave Pitch"=refnum, "Surge Pitch"=refnum, "Sway Pitch"=refnum, "Heave PPR"=refnum, "Surge PPR"=refnum, "Sway PPR"=refnum, "Tab Control 5"=refnum, "Tab Control 14"=refnum, "Tab Control 26"=refnum, "AE"=refnum, "Heave Loop Delay"=refnum, "Heave PID Speed"=refnum, "Surge Jog Speed"=refnum, "Heave Jog Speed"=refnum, "Sway Loop Delay"=refnum, "Sway PID Speed"=refnum, "Sway Jog Speed"=refnum, "DEPTH TRIP VALUE"=refnum, "LOAD TRIP VALUE"=refnum, "DEPTH TRIP   ENABLE"=refnum, "LOAD TRIP  ENABLE"=refnum, "CYCLIC FF TRIP VALUE"=refnum, "FF TRIP VALUE"=refnum, "CYCLIC CoF TRIP VALUE"=refnum, "COF TRIP VALUE"=refnum, "CYCLIC COF TRIP  ENABLE"=refnum, "CYCLIC FF TRIP  ENABLE"=refnum, "FF TRIP  ENABLE"=refnum, "COF TRIP  ENABLE"=refnum, "JOG TRIP LOAD VALUE (N)"=refnum, "Rotary Vertical"=refnum, "Traction"=refnum, "Scratch"=refnum, "LRM CAM"=refnum, "Sway LRM"=refnum, "Rotary Horizontal"=refnum}, "Loading Com Port"={"ClearAll"=refnum, "Mz(Nm)"=refnum, "My(Nm)"=refnum, "Mx(Nm)"=refnum, "Save Dwell"=refnum, "Acq Delay (ms)"=refnum, "Burst Delay (ms)"=refnum, "model"=refnum, "SN"=refnum, "FFx(N)"=refnum, "Sensor IP"=refnum, "Port"=refnum, "FFy(N)"=refnum, "Load(N)"=refnum, "delete Handle"=refnum, "Create Handle"=refnum, "ft_data"=refnum, "ft_range"=refnum, "ft_data 2"=refnum, "stop 6"=refnum, "running_flag"=refnum, "ft_udp_handle"=refnum, "get-data-return"=refnum, "get-range-return"=refnum, "zero-return"=refnum, "filter-return"=refnum, "initial-return"=refnum, "deleteHandle-result"=refnum, "Load Cell Temp"=refnum, "Load Cell"=refnum, "ZeroAll"=refnum, "FORCE (N)"=refnum, "TORQUE (N-m)"=refnum, "Load Cell Link"=refnum}, "Heave AND Surge"={"SURGE POSE"=refnum, "error out Read"=refnum, "HEAVE POSE"=refnum, "State"=refnum, "Homed"=refnum, "Sequence ID"=refnum, "error out Write"=refnum, "faultCode"=refnum, "Ack ID"=refnum, "SPEED"=refnum, "Distance"=refnum, "Mode Command"=refnum, "Heave and Surge Read"=refnum, "Read Heave Temp"=refnum, "Spare 15"=refnum, "Spare 14"=refnum, "Spare 13"=refnum, "Spare 12"=refnum, "Spare 11"=refnum, "Spare 10"=refnum, "Spare 9"=refnum, "Spare 8"=refnum, "Spare 7"=refnum, "Spare 4"=refnum, "Spare 3"=refnum, "Spare 2"=refnum, "Humidity"=refnum, "Temp"=refnum, "Node Id"=refnum, "Spare 1"=refnum, "SPARE 4"=refnum, "SPARE 3"=refnum, "SPARE 2"=refnum, "SPARE 1"=refnum, "fwMajor"=refnum, "fwMinor"=refnum, "Manual Write"=refnum, "Heave and Surge Write"=refnum, "SPARE 5"=refnum, "Reserved "=refnum, "SPARE 8"=refnum, "SPARE 6"=refnum, "SPARE 7"=refnum, "SPARE 17"=refnum, "SPARE 16"=refnum, "SPARE 15"=refnum, "SPARE 14"=refnum, "SPARE 13"=refnum, "SPARE 12"=refnum, "SPARE 11"=refnum, "SPARE 10"=refnum, "SPARE 9"=refnum, "System UPTIME"=refnum, "Missed Packets"=refnum, "faultCode Surge Right"=refnum, "faultCode Surge Left"=refnum, "faultCode Heave"=refnum, "UPLINK HEAVE"=refnum, "DOWNLINK HEAVE"=refnum}, "New PID LOGIC"={"Fine Tune Zone"=refnum, "PID SDelay"=refnum, "Max_pos_limit"=refnum, "Min_pos_limit"=refnum, "i_limit"=refnum, "pct_scale"=refnum, "Deadband"=refnum, "Kd"=refnum, "Ki"=refnum, "Kp"=refnum, "Current Position"=refnum, "Set Load"=refnum, "Current Load"=refnum, "Pulse delta"=refnum, "Init Step"=refnum, "Max Step Linit"=refnum, "min_deadband_floor"=refnum, "dynamic_spindle_noise_scalar"=refnum, "min_finetune_floor"=refnum, "filter_alpha"=refnum, "PID"=refnum}, "SWAY "={"fwMajor"=refnum, "Homed"=refnum, "Rotary POSE"=refnum, "State"=refnum, "SWAY POSE"=refnum, "Ack ID"=refnum, "faultCode"=refnum, "Node Id"=refnum, "fwMinor"=refnum, "Spare 6"=refnum, "Spare 5"=refnum, "Spare 4"=refnum, "Spare 3"=refnum, "Spare 2"=refnum, "Spare 1"=refnum, "Spare 7"=refnum, "SPARE  5"=refnum, "error out Write  SWAY "=refnum, "error out Read SWAY "=refnum, "Manual Write SWAY "=refnum, "SWAY WRITE"=refnum, "SPARE  4"=refnum, "SPARE  3"=refnum, "SPARE 2"=refnum, "SPARE 1"=refnum, "Spare 15"=refnum, "Spare 14"=refnum, "Spare 13"=refnum, "Spare 12"=refnum, "Spare 11"=refnum, "Spare 9"=refnum, "Spare 8"=refnum, "SPEED"=refnum, "Distance"=refnum, "Mode Command"=refnum, "Sequence ID"=refnum, "SWAY READ"=refnum, "Spare 10"=refnum, "Read SWAY Temp"=refnum, "faultCode Sway "=refnum, "Missed Packets"=refnum, "System UPTIME sway"=refnum, "SPARE 6"=refnum, "SPARE 7"=refnum, "SPARE 9"=refnum, "SPARE 11"=refnum, "SPARE 10"=refnum, "SPARE 8"=refnum, "SPARE 13"=refnum, "SPARE 12"=refnum, "SPARE 17"=refnum, "SPARE 16"=refnum, "SPARE 15"=refnum, "SPARE 14"=refnum, "Reserved"=refnum, "faultCode Rotary"=refnum, "UPLINK SWAY"=refnum, "DOWNLINK SWAY"=refnum}, "Analysis Screen"={"Analysis Home"=refnum, "Refresh 2"=refnum, "MEAN 4"=refnum, "SD 4"=refnum, "VARIANCE 4"=refnum, "MEAN  3"=refnum, "SD  3"=refnum, "VARIANCE  3"=refnum, "MEAN 2"=refnum, "SD  2"=refnum, "VARIANCE 2"=refnum, "MEAN"=refnum, "SD"=refnum, "VARIANCE"=refnum, "File 4 Discription"=refnum, "OPEN 4"=refnum, "File Name 4"=refnum, "OPEN 3"=refnum, "File 3 Discription"=refnum, "File Name 3"=refnum, "Y-AXIS"=refnum, "X-AXIS"=refnum, "XY Graph"=refnum, "File Name 2"=refnum, "File Name 1"=refnum, "OPEN 2"=refnum, "OPEN 1"=refnum, "File 1 Discription "=refnum, "File 2 Discription"=refnum, "Export"=refnum, "File Format"=refnum}, "Traction"={"faultCode Traction 2"=refnum, "faultCode Traction 1"=refnum, "Missed Packets"=refnum, "System UPTIME Traction"=refnum, "SPARE 17"=refnum, "SPARE 16"=refnum, "SPARE 15"=refnum, "SPARE 14"=refnum, "SPARE 13"=refnum, "SPARE 12"=refnum, "SPARE 11"=refnum, "SPARE 10"=refnum, "SPARE 9"=refnum, "SPARE 8"=refnum, "SPARE 7"=refnum, "SPARE 6"=refnum, "Reserved"=refnum, "SPARE  5"=refnum, "Manual Write TRACTION"=refnum, "TRACTION WRITE"=refnum, "SPARE  4"=refnum, "SPARE  3"=refnum, "SPARE 2"=refnum, "SPARE 1"=refnum, "Spare 7"=refnum, "Spare 6"=refnum, "Spare 5"=refnum, "Spare 4"=refnum, "Spare 2"=refnum, "Spare 1"=refnum, "Node Id"=refnum, "Read TRACTION Temp"=refnum, "fwMinor"=refnum, "fwMajor"=refnum, "faultCode"=refnum, "TRACTION POSE"=refnum, "TRACTION POSE 2"=refnum, "Homed"=refnum, "State"=refnum, "Ack ID"=refnum, "SPEED"=refnum, "Distance"=refnum, "Mode Command"=refnum, "Sequence ID"=refnum, "error out Read TRACTION"=refnum, "error out Write  TRACTION"=refnum, "TRACTION READ"=refnum, "Spare 3"=refnum, "Downlink traction"=refnum, "Uplink Traction"=refnum}, "Traction reciepe"={"SRR Sweep Range (%) Stribeck"=refnum, "Traction Receipe"=refnum, "Total Execution Time"=refnum, "Total Steps"=refnum, "Duration / Step (s)  Stribeck"=refnum, "STRIBECK Fixed SRR List (%)"=refnum, "Duration / Step (s) Traction"=refnum, "SRR Sweep Range (%) traction"=refnum, "Rolling Speed (mm/s)"=refnum, "Temperature Stages (°C)"=refnum, "Ball Load (N)"=refnum, "Lubricant Name"=refnum, "Profile File Name"=refnum, "SET entrainment Velocity"=refnum, "Test Array Size"=refnum, "SRR INDEX [ STRIBECK]"=refnum, "Stribeck Size"=refnum, "SET SRR"=refnum, "ELAPSED TIMER "=refnum, "BALL SET RPM"=refnum, "DISC SET RPM"=refnum, "SET LOAD"=refnum, "TEMPERATURE READ"=refnum, "SET TEMPERATURE"=refnum, "Traction Size"=refnum, "DISC SPEED (rpm)"=refnum, "BALL SPEED (rpm)"=refnum, "BALL WEAR TRACK"=refnum, "DISC WEARTRACK"=refnum, "SRR INDEX [ TRACTION]"=refnum, "Start Index Type"=refnum, "Enum - Menu"=refnum, "Ball (mm/sec)"=refnum, "Disc (mm/sec)"=refnum}, "Traction Control"={"HomeTraction"=refnum, "Demo Mode Display"=refnum, "Traction Message"=refnum, "Traction Step Update Details"=refnum, "Main Tab sequence for selection"=refnum, "Ramp Tab"=refnum, "e.v/ssr"=refnum, "Enter Fixed E.Velocity"=refnum, "Enter Final SRR"=refnum, "Enter initial SRR"=refnum, "Enter Fixed SRR"=refnum, "Enter the Final E.Velocity (m/s)"=refnum, "Enter initial E.Velocity (m/s)"=refnum, "Ball WTD"=refnum, "E.Velocity"=refnum, "Enter the Final Velocity (m/s)"=refnum, "Enter initial Velocity (m/s)"=refnum, "Ramp Up   Disc"=refnum, "Initial DiscSpeed (RPM)"=refnum, "Final Speed (RPM) Ball"=refnum, "Final Speed (RPM)"=refnum, "Initial Speed (RPM) Ball"=refnum, "Enter the Final Velocity (m/s) Ball"=refnum, "Enter initial Velocity (m/s) Ball"=refnum, "Ramp Up"=refnum, "ExceedBallSpeed step"=refnum, "ExceedDiscSpeed"=refnum, "BallSpeed Exceed Indication"=refnum, "Apply"=refnum, "SPEED SELECTION : MTM"=refnum, "SPEED SELECTION : MTM 2"=refnum, "TEST SELECTION (MTM)"=refnum, "MTM Test Selection"=refnum, "File Path Tab"=refnum, "File Path String"=refnum, "Save"=refnum, "Save  2"=refnum, "Import "=refnum, "File Path :"=refnum, "Step Sequence Indication Tab"=refnum, "Step Sequence Indication"=refnum, "Calculate Step"=refnum, "StepTable"=refnum, "ExceedDiscSpeed  Cinstant Speed"=refnum, "ExceedBallSpeed Constant"=refnum, "TEST SELECTION (MTM) 2"=refnum, "SPEED SELECTION : MTM 3"=refnum, "MTM Test Selection 2"=refnum, "Enter the Speed (m/sec): "=refnum, "Enter the Speed (m/sec):  2"=refnum, "Enter the Speed (RPM):"=refnum, "Lower Spped "=refnum, "Upper"=refnum, "Enter the Speed (RPM):Ball"=refnum, "Disc Motion Direction: "=refnum, "Ball Motion Direction :"=refnum, "Motion Mode: "=refnum, "Wear Track Diameter (mm) "=refnum, "Disc Speed Indicator"=refnum, "ExceedBallSpeed"=refnum}, "Acquostic"={"Last Config Rejected "=refnum, "rx command count"=refnum, "Current Filter Id"=refnum, "Isolated Gain"=refnum, "DAQ Status"=refnum, "error out"=refnum, "error in (no error)"=refnum, "Uplink Packet"=refnum, "data out"=refnum, "Downlink Packet"=refnum, "Gains"=refnum, "Manual Write Acquostic"=refnum, "Acoustic Graphs"=refnum}} ("Data Cluster") -> [w67]
    tunnel: w55 -> [w90]
    tunnel: [w77] -> w54
    tunnel: w54 -> [w97]
    tunnel: [w91] -> w53
    tunnel: w53 -> [w106]
    tunnel: [w105] -> w52
    tunnel: w52 -> [w142]
    tunnel: [w141] -> w50
    tunnel: w50 -> [w213]
    tunnel: [w212] -> w49
    tunnel: w49 -> [w240]
    tunnel: [w239] -> w48
    tunnel: w48 -> [w254]
    tunnel: [w253] -> w47
    tunnel: w47 -> [w356]
    tunnel: [w355] -> w26
    tunnel: w26 -> [w364]
    tunnel: [w363] -> w25
    tunnel: w25 -> [w430]
    tunnel: [w429] -> w24
    tunnel: w24 -> [w447]
    tunnel: [w446] -> w23
    tunnel: w23 -> [w508]
    tunnel: [w507] -> w21
    tunnel: w21 -> [w531]
    tunnel: [w530] -> w20
    tunnel: w20 -> [w591]
    tunnel: [w590] -> w18
    tunnel: w18 -> [w624]
    tunnel: [w623] -> w15
    tunnel: w15 -> [w676]
    tunnel: [w675] -> w14
    tunnel: w14 -> [w712]
    tunnel: [w711] -> w13
    tunnel: w13 -> [w772]
    tunnel: [w771] -> w7
    tunnel: [w786] -> w5
    tunnel: w7 -> [w787]
    frame #0 {
      n2 = control-ref of="GUI"() -> (w76:refnum<vi>)
      n3 = control-ref of="MainPage"() -> (w70:refnum<vi>)
      n4 = control-ref of="Platform Settings"() -> (w75:refnum<vi>)
      n5 = control-ref of="Configure"() -> (w74:refnum<vi>)
      n6 = control-ref of="Home"() -> (w73:refnum<vi>)
      n7 = control-ref of="EXIT"() -> (w72:refnum<vi>)
      n8 = control-ref of="service 2"() -> (w71:refnum<vi>)
      n9 = control-ref of="Analysis"() -> (w69:refnum<vi>)
      n10 = Bundle By Name(cluster=w67, "Main Home Screen.GUI"=w76, "Main Home Screen.Platform Settings"=w75, "Main Home Screen.Configure"=w74, "Main Home Screen.Home"=w73, "Main Home Screen.EXIT"=w72, "Main Home Screen.service 2"=w71, "Main Home Screen.MainPage"=w70, "Main Home Screen.Analysis"=w69) -> (w68:T20)
    }
    frame #1 {
      n11 = control-ref of="Disable Axis Jog Soft Limits m"() -> (w88:refnum<vi>)
      n12 = control-ref of="Sway and Surge COM Status"() -> (w87:refnum<vi>)
      n13 = control-ref of="Heave COM Status"() -> (w86:refnum<vi>)
      n14 = control-ref of="Enable Platform"() -> (w85:refnum<vi>)
      n15 = control-ref of="Surge Forward Main"() -> (w84:refnum<vi>)
      n16 = control-ref of="Sway Right Main"() -> (w83:refnum<vi>)
      n17 = control-ref of="Sway Left Main"() -> (w82:refnum<vi>)
      n18 = control-ref of="Heave Down Main"() -> (w81:refnum<vi>)
      n19 = control-ref of="Heave Up main"() -> (w80:refnum<vi>)
      n20 = control-ref of="Surge Backward Main"() -> (w78:refnum<vi>)
      n21 = control-ref of="mm"() -> (w79:refnum<vi>)
      n22 = control-ref of="Drive Error"() -> (w89:refnum<vi>)
      n23 = Bundle By Name(cluster=w90, "Platform Settings.Drive Error"=w89, "Platform Settings.Disable Axis Jog Soft Limits"=w88, "Platform Settings.Sway and Surge COM Status"=w87, "Platform Settings.Heave COM Status"=w86, "Platform Settings.Enable Platform"=w85, "Platform Settings.Surge Forward Main"=w84, "Platform Settings.Sway Right Main"=w83, "Platform Settings.Sway Left Main"=w82, "Platform Settings.Heave Down Main"=w81, "Platform Settings.Heave Up main"=w80, "Platform Settings.mm"=w79, "Platform Settings.Surge Backward Main"=w78) -> (w77:T20)
    }
    frame #2 {
      n24 = control-ref of="Analysis Home"() -> (w96:refnum<vi>)
      n25 = control-ref of="Surface Analysis"() -> (w95:refnum<vi>)
      n26 = control-ref of="Imaging"() -> (w94:refnum<vi>)
      n27 = control-ref of="Image Analysis"() -> (w93:refnum<vi>)
      n28 = control-ref of="Post Analysis"() -> (w92:refnum<vi>)
      n29 = Bundle By Name(cluster=w97, "Analysis Screen.Analysis Home"=w96, "Analysis Screen.Surface Analysis"=w95, "Analysis Screen.Imaging"=w94, "Analysis Screen.Image Analysis"=w93, "Analysis Screen.Post Analysis"=w92) -> (w91:T20)
    }
    frame #3 {
      n30 = control-ref of="Select Load Head"() -> (w104:refnum<vi>)
      n31 = control-ref of="Auto"() -> (w98:refnum<vi>)
      n32 = control-ref of="Notes :"() -> (w103:refnum<vi>)
      n33 = control-ref of="FILE"() -> (w102:refnum<vi>)
      n34 = control-ref of="Sample ID :"() -> (w101:refnum<vi>)
      n35 = control-ref of="Operator ID :"() -> (w100:refnum<vi>)
      n36 = control-ref of="Operator Name :"() -> (w99:refnum<vi>)
      n37 = Bundle By Name(cluster=w106, "Config Screen.Select Load Head"=w104, "Config Screen.Notes :"=w103, "Config Screen.FILE"=w102, "Config Screen.Sample ID :"=w101, "Config Screen.Operator ID :"=w100, "Config Screen.Operator Name :"=w99, "Config Screen.Auto"=w98) -> (w105:T20)
    }
    frame #4 {
      n38 = control-ref of="Warning"() -> (w134:refnum<vi>)
      n39 = control-ref of="gui GIF"() -> (w133:refnum<vi>)
      n40 = control-ref of="Load Selection"() -> (w107:refnum<vi>)
      n41 = control-ref of="Warning 2"() -> (w138:refnum<vi>)
      n42 = control-ref of="SSP 0.75"() -> (w137:refnum<vi>)
      n43 = control-ref of="SSP 0.5"() -> (w136:refnum<vi>)
      n44 = control-ref of="SSP 0.3"() -> (w135:refnum<vi>)
      n45 = control-ref of="Communication is established"() -> (w132:refnum<vi>)
      n46 = control-ref of="AppLoad 4"() -> (w131:refnum<vi>)
      n47 = control-ref of="Multipoint"() -> (w130:refnum<vi>)
      n48 = control-ref of="com 3"() -> (w126:refnum<vi>)
      n49 = control-ref of="com"() -> (w125:refnum<vi>)
      n50 = control-ref of="DecaForce COM Status"() -> (w124:refnum<vi>)
      n51 = control-ref of="Update"() -> (w123:refnum<vi>)
      n52 = control-ref of="Clear 3"() -> (w122:refnum<vi>)
      n53 = control-ref of="seq"() -> (w121:refnum<vi>)
      n54 = control-ref of="Stribeck table"() -> (w120:refnum<vi>)
      n55 = control-ref of="KiloForce"() -> (w112:refnum<vi>)
      n56 = control-ref of="DecaForce"() -> (w111:refnum<vi>)
      n57 = control-ref of="MicroForce"() -> (w110:refnum<vi>)
      n58 = control-ref of="LHBack"() -> (w109:refnum<vi>)
      n59 = control-ref of="LHNext"() -> (w108:refnum<vi>)
      n60 = control-ref of="Enter the Loading Rate (N/min)"() -> (w140:refnum<vi>)
      n61 = control-ref of="Enter the Final Load (N)"() -> (w117:refnum<vi>)
      n62 = control-ref of="Enter the CoF Trip"() -> (w116:refnum<vi>)
      n63 = control-ref of="Enter the Friction Force Trip"() -> (w115:refnum<vi>)
      n64 = control-ref of="Enter the Normal load Trip"() -> (w114:refnum<vi>)
      n65 = control-ref of="Enter the Load  (N)"() -> (w113:refnum<vi>)
      n66 = control-ref of="Message"() -> (w139:refnum<vi>)
      n67 = control-ref of="Indentation"() -> (w129:refnum<vi>)
      n68 = control-ref of="Stribeck Table  For loading"() -> (w119:refnum<vi>)
      n69 = control-ref of="Reference Sample"() -> (w128:refnum<vi>)
      n70 = control-ref of="Load Cell Communication Slide"() -> (w127:refnum<vi>)
      n71 = control-ref of="Loading Mode"() -> (w118:refnum<vi>)
      n72 = Bundle By Name(cluster=w142, "Loading.Enter the Loading Rate (N/min)"=w140, "Loading.Message"=w139, "Loading.Warning 2"=w138, "Loading.SSP 0.75"=w137, "Loading.SSP 0.5"=w136, "Loading.SSP 0.3"=w135, "Loading.Warning"=w134, "Loading.gui GIF"=w133, "Loading.Communication is established"=w132, "Loading.AppLoad 4"=w131, "Loading.Multipoint"=w130, "Loading.Indentation"=w129, "Loading.Reference Sample"=w128, "Loading.Load Cell Communication Slide"=w127, "Loading.com 3"=w126, "Loading.com"=w125, "Loading.DecaForce COM Status"=w124, "Loading.Update"=w123, "Loading.Clear 3"=w122, "Loading.seq"=w121, "Loading.Stribeck table"=w120, "Loading.Stribeck Table  For loading"=w119, "Loading.Loading Mode"=w118, "Loading.Enter the Final Load (N)"=w117, "Loading.Enter the CoF Trip"=w116, "Loading.Enter the Friction Force Trip"=w115, "Loading.Enter the Normal load Trip"=w114, "Loading.Enter the Load  (N)"=w113, "Loading.KiloForce"=w112, "Loading.DecaForce"=w111, "Loading.MicroForce"=w110, "Loading.LHBack"=w109, "Loading.LHNext"=w108, "Loading.Load Selection"=w107) -> (w141:T20)
    }
    frame #5 {
      n73 = control-ref of="TEST SELECTION"() -> (w194:refnum<vi>)
      n74 = control-ref of="SPEED SELECTION :"() -> (w193:refnum<vi>)
      n75 = control-ref of="SPEED SELECTION : rotary"() -> (w160:refnum<vi>)
      n76 = control-ref of="Rotary Tab"() -> (w209:refnum<vi>)
      n77 = control-ref of="e.v/ssr 2"() -> (w206:refnum<vi>)
      n78 = control-ref of="Step Speed"() -> (w190:refnum<vi>)
      n79 = control-ref of="M3 Image"() -> (w185:refnum<vi>)
      n80 = control-ref of="Rotary Module Selection"() -> (w162:refnum<vi>)
      n81 = control-ref of="zNL"() -> (w211:refnum<vi>)
      n82 = control-ref of="E.Velocity 2"() -> (w207:refnum<vi>)
      n83 = control-ref of="Ramp Up 2"() -> (w195:refnum<vi>)
      n84 = control-ref of="Angular Oscillation Set"() -> (w192:refnum<vi>)
      n85 = control-ref of="Traction"() -> (w191:refnum<vi>)
      n86 = control-ref of="Surge Forward MM"() -> (w187:refnum<vi>)
      n87 = control-ref of="Surge Backward MM"() -> (w186:refnum<vi>)
      n88 = control-ref of="Sway Left MM"() -> (w183:refnum<vi>)
      n89 = control-ref of="Sway Right MM"() -> (w182:refnum<vi>)
      n90 = control-ref of="Disable Axis Jog Soft Limits"() -> (w181:refnum<vi>)
      n91 = control-ref of="Heave Down MM"() -> (w179:refnum<vi>)
      n92 = control-ref of="Heave Up MM"() -> (w178:refnum<vi>)
      n93 = control-ref of="Set WTD"() -> (w176:refnum<vi>)
      n94 = control-ref of="HomeScratch"() -> (w175:refnum<vi>)
      n95 = control-ref of="HomeRot"() -> (w174:refnum<vi>)
      n96 = control-ref of="PlaceModule"() -> (w173:refnum<vi>)
      n97 = control-ref of="LR Sway"() -> (w169:refnum<vi>)
      n98 = control-ref of="Rot Hor"() -> (w168:refnum<vi>)
      n99 = control-ref of="Scratch"() -> (w167:refnum<vi>)
      n100 = control-ref of="LR Cam"() -> (w166:refnum<vi>)
      n101 = control-ref of="MMBack"() -> (w165:refnum<vi>)
      n102 = control-ref of="MMNext"() -> (w164:refnum<vi>)
      n103 = control-ref of="Rot Ver"() -> (w163:refnum<vi>)
      n104 = control-ref of="calculate rotary"() -> (w161:refnum<vi>)
      n105 = control-ref of="Import 2"() -> (w159:refnum<vi>)
      n106 = control-ref of="Save 2"() -> (w158:refnum<vi>)
      n107 = control-ref of="SwaySpeed Set"() -> (w151:refnum<vi>)
      n108 = control-ref of="HomeScratch"() -> (w147:refnum<vi>)
      n109 = control-ref of="NL disp"() -> (w210:refnum<vi>)
      n110 = control-ref of="Enter Fixed E.Velocity 2"() -> (w205:refnum<vi>)
      n111 = control-ref of="Enter Final SRR 2"() -> (w204:refnum<vi>)
      n112 = control-ref of="Enter initial SRR 2"() -> (w203:refnum<vi>)
      n113 = control-ref of="Enter Fixed SRR 2"() -> (w202:refnum<vi>)
      n114 = control-ref of="Enter the Final E.Velocity (m/s) 2"() -> (w201:refnum<vi>)
      n115 = control-ref of="Enter initial E.Velocity (m/s) 2"() -> (w200:refnum<vi>)
      n116 = control-ref of="Final Speed (RPM) 3"() -> (w199:refnum<vi>)
      n117 = control-ref of="Initial Speed (RPM) 2"() -> (w198:refnum<vi>)
      n118 = control-ref of="Enter the Final Velocity (m/s) 3"() -> (w197:refnum<vi>)
      n119 = control-ref of="Enter initial Velocity (m/s)  3"() -> (w196:refnum<vi>)
      n120 = control-ref of="mm"() -> (w180:refnum<vi>)
      n121 = control-ref of="Wear Track Diameter (mm)"() -> (w177:refnum<vi>)
      n122 = control-ref of="Enter the Angle (Deg)"() -> (w172:refnum<vi>)
      n123 = control-ref of="Enter the Frequency (Hz)"() -> (w171:refnum<vi>)
      n124 = control-ref of="Enter the Speed(mm/sec)"() -> (w154:refnum<vi>)
      n125 = control-ref of="Enter the Speed (RPM)"() -> (w153:refnum<vi>)
      n126 = control-ref of="Enter Scratch Speed (mm/s):"() -> (w152:refnum<vi>)
      n127 = control-ref of="Scartch Offset"() -> (w150:refnum<vi>)
      n128 = control-ref of="Enter Scratch length (mm):"() -> (w146:refnum<vi>)
      n129 = control-ref of="Wear Track Diameter"() -> (w145:refnum<vi>)
      n130 = control-ref of="No of Scratch"() -> (w143:refnum<vi>)
      n131 = control-ref of="String 39"() -> (w184:refnum<vi>)
      n132 = control-ref of="String 45"() -> (w156:refnum<vi>)
      n133 = control-ref of="Rotary Speed Exced"() -> (w144:refnum<vi>)
      n134 = control-ref of="StepTable For Load-Speed"() -> (w189:refnum<vi>)
      n135 = control-ref of="StepTable For Speed"() -> (w188:refnum<vi>)
      n136 = control-ref of="StepTable For Speed 3"() -> (w155:refnum<vi>)
      n137 = control-ref of="Motion Direction:  3"() -> (w208:refnum<vi>)
      n138 = control-ref of="Motion Mode:"() -> (w170:refnum<vi>)
      n139 = control-ref of="Scratch Mode"() -> (w149:refnum<vi>)
      n140 = control-ref of="Motion type:"() -> (w148:refnum<vi>)
      n141 = control-ref of="File Path :  2"() -> (w157:refnum<vi>)
      n142 = Bundle By Name(cluster=w213, "Motion Module.zNL"=w211, "Motion Module.NL disp"=w210, "Motion Module.Rotary Tab"=w209, "Motion Module.Motion Direction:  3"=w208, "Motion Module.E.Velocity 2"=w207, "Motion Module.e.v/ssr 2"=w206, "Motion Module.Enter Fixed E.Velocity 2"=w205, "Motion Module.Enter Final SRR 2"=w204, "Motion Module.Enter initial SRR 2"=w203, "Motion Module.Enter Fixed SRR 2"=w202, "Motion Module.Enter the Final E.Velocity (m/s) 2"=w201, "Motion Module.Enter initial E.Velocity (m/s) 2"=w200, "Motion Module.Final Speed (RPM) 3"=w199, "Motion Module.Initial Speed (RPM) 2"=w198, "Motion Module.Enter the Final Velocity (m/s) 3"=w197, "Motion Module.Enter initial Velocity (m/s)  3"=w196, "Motion Module.Ramp Up 2"=w195, "Motion Module.TEST SELECTION"=w194, "Motion Module.SPEED SELECTION :"=w193, "Motion Module.Angular Oscillation Set"=w192, "Motion Module.Traction"=w191, "Motion Module.Step Speed"=w190, "Motion Module.StepTable For Load-Speed"=w189, "Motion Module.StepTable For Speed"=w188, "Motion Module.Surge Forward MM"=w187, "Motion Module.Surge Backward MM"=w186, "Motion Module.M3 Image"=w185, "Motion Module.String 39"=w184, "Motion Module.Sway Left MM"=w183, "Motion Module.Sway Right MM"=w182, "Motion Module.Disable Axis Jog Soft Limits"=w181, "Motion Module.mm"=w180, "Motion Module.Heave Down MM"=w179, "Motion Module.Heave Up MM"=w178, "Motion Module.Wear Track Diameter (mm)"=w177, "Motion Module.Set WTD"=w176, "Motion Module.HomeScratch"=w175, "Motion Module.HomeRot"=w174, "Motion Module.PlaceModule"=w173, "Motion Module.Enter the Angle (Deg)"=w172, "Motion Module.Enter the Frequency (Hz)"=w171, "Motion Module.Motion Mode:"=w170, "Motion Module.LR Sway"=w169, "Motion Module.Rot Hor"=w168, "Motion Module.Scratch"=w167, "Motion Module.LR Cam"=w166, "Motion Module.MMBack"=w165, "Motion Module.MMNext"=w164, "Motion Module.Rot Ver"=w163, "Motion Module.Rotary Module Selection"=w162, "Motion Module.calculate rotary"=w161, "Motion Module.SPEED SELECTION : rotary"=w160, "Motion Module.Import 2"=w159, "Motion Module.Save 2"=w158, "Motion Module.File Path :  2"=w157, "Motion Module.String 45"=w156, "Motion Module.StepTable For Speed 3"=w155, "Motion Module.Enter the Speed(mm/sec)"=w154, "Motion Module.Enter the Speed(RPM)"=w153, "Motion Module.Enter Scratch Speed (mm/s):"=w152, "Motion Module.SwaySpeed Set"=w151, "Motion Module.Scartch Offset"=w150, "Motion Module.Scratch Mode"=w149, "Motion Module.Motion type:"=w148, "Motion Module.HomeScratch 2"=w147, "Motion Module.Enter Scratch length (mm):"=w146, "Motion Module.Wear Track Diameter"=w145, "Motion Module.Rotary Speed Exced"=w144, "Motion Module.No of Scratch"=w143) -> (w212:T20)
    }
    frame #6 {
      n143 = control-ref of="Add to list"() -> (w231:refnum<vi>)
      n144 = control-ref of="Wear"() -> (w230:refnum<vi>)
      n145 = control-ref of="Vibration"() -> (w229:refnum<vi>)
      n146 = control-ref of="Humidity (Chamber)"() -> (w228:refnum<vi>)
      n147 = control-ref of="Temperature (Chamber)"() -> (w227:refnum<vi>)
      n148 = control-ref of="ECR"() -> (w226:refnum<vi>)
      n149 = control-ref of="Temperature (Amb)"() -> (w225:refnum<vi>)
      n150 = control-ref of="Microphone"() -> (w224:refnum<vi>)
      n151 = control-ref of="Acoustic Emission 3"() -> (w223:refnum<vi>)
      n152 = control-ref of="SNext"() -> (w222:refnum<vi>)
      n153 = control-ref of="APBack"() -> (w221:refnum<vi>)
      n154 = control-ref of="Low Temp"() -> (w217:refnum<vi>)
      n155 = control-ref of="High Temp"() -> (w216:refnum<vi>)
      n156 = control-ref of="Humidity"() -> (w215:refnum<vi>)
      n157 = control-ref of="Humidity  Status  3"() -> (w238:refnum<vi>)
      n158 = control-ref of="Low Temp  Status  2"() -> (w237:refnum<vi>)
      n159 = control-ref of="TK4 status 2"() -> (w236:refnum<vi>)
      n160 = control-ref of="Humidity (Amb)"() -> (w233:refnum<vi>)
      n161 = control-ref of="Clear List"() -> (w232:refnum<vi>)
      n162 = control-ref of="Enter the Temperature (°C):"() -> (w220:refnum<vi>)
      n163 = control-ref of="Enter the Stage \nTemperature (°C):"() -> (w219:refnum<vi>)
      n164 = control-ref of="Enter the Humidity (%Rh):"() -> (w218:refnum<vi>)
      n165 = control-ref of="Sensors Picked"() -> (w214:refnum<vi>)
      n166 = control-ref of="Stage Temperature"() -> (w235:refnum<vi>)
      n167 = control-ref of="Sample Temperature"() -> (w234:refnum<vi>)
      n168 = Bundle By Name(cluster=w240, "Environmental control.Humidity  Status  3"=w238, "Environmental control.Low Temp  Status  2"=w237, "Environmental control.TK4 status 2"=w236, "Environmental control.Stage Temperature"=w235, "Environmental control.Sample Temperature"=w234, "Environmental control.Humidity (Amb)"=w233, "Environmental control.Clear List"=w232, "Environmental control.Add to list"=w231, "Environmental control.Wear"=w230, "Environmental control.Vibration"=w229, "Environmental control.Humidity (Chamber)"=w228, "Environmental control.Temperature (Chamber)"=w227, "Environmental control.ECR"=w226, "Environmental control.Temperature (Amb)"=w225, "Environmental control.Microphone"=w224, "Environmental control.Acoustic Emission 3"=w223, "Environmental control.SNext"=w222, "Environmental control.APBack"=w221, "Environmental control.Enter the Temperature (°C):"=w220, "Environmental control.Enter the Stage \nTemperature (°C):"=w219, "Environmental control.Enter the Humidity (%Rh):"=w218, "Environmental control.Low Temp"=w217, "Environmental control.High Temp"=w216, "Environmental control.Humidity"=w215, "Environmental control.Sensors Picked"=w214) -> (w239:T20)
    }
    frame #7 {
      n169 = control-ref of="ECR Port:"() -> (w248:refnum<vi>)
      n170 = control-ref of="Ramp Port:"() -> (w247:refnum<vi>)
      n171 = control-ref of="Temp Modbus:"() -> (w244:refnum<vi>)
      n172 = control-ref of="Humidity Port:"() -> (w243:refnum<vi>)
      n173 = control-ref of="About Tab"() -> (w249:refnum<vi>)
      n174 = control-ref of="Home Service"() -> (w251:refnum<vi>)
      n175 = control-ref of="Advanced Setting"() -> (w250:refnum<vi>)
      n176 = control-ref of="Installation/Replacement completed"() -> (w246:refnum<vi>)
      n177 = control-ref of="Loahead"() -> (w245:refnum<vi>)
      n178 = control-ref of="Edit Gain Constants"() -> (w242:refnum<vi>)
      n179 = control-ref of="Save Gain Constants"() -> (w241:refnum<vi>)
      n180 = control-ref of="Password"() -> (w252:refnum<vi>)
      n181 = Bundle By Name(cluster=w254, "About Screen.Password"=w252, "About Screen.Home Service"=w251, "About Screen.Advanced Setting"=w250, "About Screen.About Tab"=w249, "About Screen.ECR Port:"=w248, "About Screen.Ramp Port:"=w247, "About Screen.Installation/Replacement completed"=w246, "About Screen.Loahead"=w245, "About Screen.Temp Modbus:"=w244, "About Screen.Humidity Port:"=w243, "About Screen.Edit Gain Constants"=w242, "About Screen.Save Gain Constants"=w241) -> (w253:T20)
    }
    frame #8 {
      n182 = control-ref of="Cyclic Friction Force (N) Graph"() -> (w265:refnum<vi>)
      n183 = control-ref of="Cyclic Coefficient of Friction"() -> (w264:refnum<vi>)
      n184 = control-ref of="gACQUOS"() -> (w298:refnum<vi>)
      n185 = control-ref of="WearGp"() -> (w288:refnum<vi>)
      n186 = control-ref of="Main Chart 3"() -> (w283:refnum<vi>)
      n187 = control-ref of="Friction Force (N) Graph"() -> (w271:refnum<vi>)
      n188 = control-ref of="Coefficient of Friction"() -> (w270:refnum<vi>)
      n189 = control-ref of="Main Screen Tab"() -> (w354:refnum<vi>)
      n190 = control-ref of="Angle and Frequency"() -> (w353:refnum<vi>)
      n191 = control-ref of="Main Speed Tab"() -> (w350:refnum<vi>)
      n192 = control-ref of="MTM MOTOR DISPLAY"() -> (w349:refnum<vi>)
      n193 = control-ref of="SPEED TAB"() -> (w344:refnum<vi>)
      n194 = control-ref of="Time Tab"() -> (w339:refnum<vi>)
      n195 = control-ref of="Temp Tabs"() -> (w332:refnum<vi>)
      n196 = control-ref of="FF Tab"() -> (w268:refnum<vi>)
      n197 = control-ref of="CZ FF"() -> (w266:refnum<vi>)
      n198 = control-ref of="Cyclic FF Disable Trip"() -> (w262:refnum<vi>)
      n199 = control-ref of="cyclic COF Disable Trip"() -> (w261:refnum<vi>)
      n200 = control-ref of="cyclic COF Reset Graph"() -> (w259:refnum<vi>)
      n201 = control-ref of="Cyclic FF Reset Graph"() -> (w258:refnum<vi>)
      n202 = control-ref of="Test Trip"() -> (w257:refnum<vi>)
      n203 = control-ref of="Scratch Start Test"() -> (w269:refnum<vi>)
      n204 = control-ref of="Scratch Start Recording"() -> (w255:refnum<vi>)
      n205 = control-ref of="Heater"() -> (w331:refnum<vi>)
      n206 = control-ref of="TK4 status"() -> (w330:refnum<vi>)
      n207 = control-ref of="Controller  Status"() -> (w327:refnum<vi>)
      n208 = control-ref of="Cooling"() -> (w324:refnum<vi>)
      n209 = control-ref of="Load Communication"() -> (w323:refnum<vi>)
      n210 = control-ref of="HumCOMStatus"() -> (w321:refnum<vi>)
      n211 = control-ref of="Load En"() -> (w318:refnum<vi>)
      n212 = control-ref of="zNL 2"() -> (w317:refnum<vi>)
      n213 = control-ref of="Humidity On"() -> (w316:refnum<vi>)
      n214 = control-ref of="AppLoadSeq scratch"() -> (w312:refnum<vi>)
      n215 = control-ref of="Stop Scratch"() -> (w311:refnum<vi>)
      n216 = control-ref of="ClrLog"() -> (w310:refnum<vi>)
      n217 = control-ref of="STOP"() -> (w308:refnum<vi>)
      n218 = control-ref of="Start Test"() -> (w307:refnum<vi>)
      n219 = control-ref of="Test status"() -> (w306:refnum<vi>)
      n220 = control-ref of="AR Led"() -> (w305:refnum<vi>)
      n221 = control-ref of="Data"() -> (w304:refnum<vi>)
      n222 = control-ref of="Health"() -> (w303:refnum<vi>)
      n223 = control-ref of="Sway COM Status"() -> (w302:refnum<vi>)
      n224 = control-ref of="Heave COM Status"() -> (w301:refnum<vi>)
      n225 = control-ref of="Aqucostic Reset Graph"() -> (w299:refnum<vi>)
      n226 = control-ref of="Hymidity"() -> (w297:refnum<vi>)
      n227 = control-ref of="Humidity Disable trip"() -> (w296:refnum<vi>)
      n228 = control-ref of="Weart Deapth"() -> (w293:refnum<vi>)
      n229 = control-ref of="Depth Reset Graph"() -> (w292:refnum<vi>)
      n230 = control-ref of="Weart"() -> (w291:refnum<vi>)
      n231 = control-ref of="Depthz"() -> (w290:refnum<vi>)
      n232 = control-ref of="Load Disable Trip"() -> (w286:refnum<vi>)
      n233 = control-ref of="Load Reset Graph"() -> (w285:refnum<vi>)
      n234 = control-ref of="BACK"() -> (w282:refnum<vi>)
      n235 = control-ref of="zFF"() -> (w272:refnum<vi>)
      n236 = control-ref of="FF Reset Graph"() -> (w278:refnum<vi>)
      n237 = control-ref of="FF Disable Trip"() -> (w277:refnum<vi>)
      n238 = control-ref of="COF Disable Trip"() -> (w275:refnum<vi>)
      n239 = control-ref of="COF Reset Graph"() -> (w274:refnum<vi>)
      n240 = control-ref of="Start Test Temp"() -> (w273:refnum<vi>)
      n241 = control-ref of="Depth Trip 2"() -> (w281:refnum<vi>)
      n242 = control-ref of="Multi Scratch Pass"() -> (w256:refnum<vi>)
      n243 = control-ref of="Cyclic Friction Force (N)"() -> (w267:refnum<vi>)
      n244 = control-ref of="Cyclic FF TRIP"() -> (w263:refnum<vi>)
      n245 = control-ref of="cyclic COF TRIP"() -> (w260:refnum<vi>)
      n246 = control-ref of="Stroke (mm)"() -> (w352:refnum<vi>)
      n247 = control-ref of="Angle (Deg)"() -> (w351:refnum<vi>)
      n248 = control-ref of="Disc Speed (m/sec)"() -> (w348:refnum<vi>)
      n249 = control-ref of="Ball Speed (m/sec)"() -> (w347:refnum<vi>)
      n250 = control-ref of="Disc Speed (RPM)"() -> (w346:refnum<vi>)
      n251 = control-ref of="Ball Speed (RPM)"() -> (w345:refnum<vi>)
      n252 = control-ref of="Speed (m/sec)"() -> (w343:refnum<vi>)
      n253 = control-ref of="Set Speed (m/sec)"() -> (w342:refnum<vi>)
      n254 = control-ref of="Speed (RPM)"() -> (w341:refnum<vi>)
      n255 = control-ref of="Set Speed"() -> (w340:refnum<vi>)
      n256 = control-ref of="Time ( HH:MM:SS ) 2"() -> (w338:refnum<vi>)
      n257 = control-ref of="Test Duration"() -> (w337:refnum<vi>)
      n258 = control-ref of="Test Duration 4"() -> (w336:refnum<vi>)
      n259 = control-ref of="TEST CYCLE"() -> (w335:refnum<vi>)
      n260 = control-ref of="TOTAL CYCLES"() -> (w334:refnum<vi>)
      n261 = control-ref of="Set Load (N)"() -> (w333:refnum<vi>)
      n262 = control-ref of="ChamberTemp"() -> (w329:refnum<vi>)
      n263 = control-ref of="SetTmp"() -> (w328:refnum<vi>)
      n264 = control-ref of="ChamberTemp"() -> (w326:refnum<vi>)
      n265 = control-ref of="SetTmp"() -> (w325:refnum<vi>)
      n266 = control-ref of="Ambient \nTemperature"() -> (w322:refnum<vi>)
      n267 = control-ref of="Ambient\n Humidity"() -> (w320:refnum<vi>)
      n268 = control-ref of="Freq (Hz)"() -> (w319:refnum<vi>)
      n269 = control-ref of="humidity disp"() -> (w315:refnum<vi>)
      n270 = control-ref of="Set Humidity"() -> (w314:refnum<vi>)
      n271 = control-ref of="NL disp 2"() -> (w313:refnum<vi>)
      n272 = control-ref of="Acoustic Emission (mV)"() -> (w300:refnum<vi>)
      n273 = control-ref of="CoF Trip  2"() -> (w295:refnum<vi>)
      n274 = control-ref of="Depth Trip"() -> (w294:refnum<vi>)
      n275 = control-ref of="Depth (µm)"() -> (w289:refnum<vi>)
      n276 = control-ref of="NL Trip 2"() -> (w287:refnum<vi>)
      n277 = control-ref of="NL Display 4"() -> (w284:refnum<vi>)
      n278 = control-ref of="COF TRIP"() -> (w280:refnum<vi>)
      n279 = control-ref of="Friction Force (N)"() -> (w279:refnum<vi>)
      n280 = control-ref of="FF TRIP"() -> (w276:refnum<vi>)
      n281 = control-ref of="Trip Log"() -> (w309:refnum<vi>)
      n282 = Bundle By Name(cluster=w356, "Main Screen.Test Trip"=w257, "Main Screen.Main Screen Tab"=w354, "Main Screen.Angle and Frequency"=w353, "Main Screen.Stroke (mm)"=w352, "Main Screen.Angle (Deg)"=w351, "Main Screen.Main Speed Tab"=w350, "Main Screen.MTM MOTOR DISPLAY"=w349, "Main Screen.Disc Speed (m/sec)"=w348, "Main Screen.Ball Speed (m/sec)"=w347, "Main Screen.Disc Speed (RPM)"=w346, "Main Screen.Ball Speed (RPM)"=w345, "Main Screen.SPEED TAB"=w344, "Main Screen.Speed (m/sec)"=w343, "Main Screen.Set Speed (m/sec)"=w342, "Main Screen.Speed (RPM)"=w341, "Main Screen.Set Speed"=w340, "Main Screen.Time Tab"=w339, "Main Screen.Time ( HH:MM:SS ) 2"=w338, "Main Screen.Test Duration"=w337, "Main Screen.Test Duration 4"=w336, "Main Screen.TEST CYCLE"=w335, "Main Screen.TOTAL CYCLES"=w334, "Main Screen.Set Load (N)"=w333, "Main Screen.Temp Tabs"=w332, "Main Screen.Heater"=w331, "Main Screen.TK4 status"=w330, "Main Screen.ChamberTemp"=w329, "Main Screen.SetTmp"=w328, "Main Screen.Controller  Status"=w327, "Main Screen.ChamberTemp 2"=w326, "Main Screen.SetTmp 2"=w325, "Main Screen.Cooling"=w324, "Main Screen.Load Communication"=w323, "Main Screen.Ambient \nTemperature"=w322, "Main Screen.HumCOMStatus"=w321, "Main Screen.Ambient\n Humidity"=w320, "Main Screen.Freq (Hz)"=w319, "Main Screen.Load En"=w318, "Main Screen.zNL 2"=w317, "Main Screen.Humidity On"=w316, "Main Screen.humidity disp"=w315, "Main Screen.Set Humidity"=w314, "Main Screen.NL disp 2"=w313, "Main Screen.AppLoadSeq scratch"=w312, "Main Screen.Stop Scratch"=w311, "Main Screen.ClrLog"=w310, "Main Screen.Trip Log"=w309, "Main Screen.STOP"=w308, "Main Screen.Start Test"=w307, "Main Screen.Test status"=w306, "Main Screen.AR Led"=w305, "Main Screen.Data"=w304, "Main Screen.Health"=w303, "Main Screen.Sway COM Status"=w302, "Main Screen.Heave COM Status"=w301, "Main Screen.Acoustic Emission (mV)"=w300, "Main Screen.Aqucostic Reset Graph"=w299, "Main Screen.gACQUOS"=w298, "Main Screen.Hymidity"=w297, "Main Screen.Humidity Disable trip"=w296, "Main Screen.CoF Trip  2"=w295, "Main Screen.Depth Trip"=w294, "Main Screen.Weart Deapth"=w293, "Main Screen.Depth Reset Graph"=w292, "Main Screen.Weart"=w291, "Main Screen.Depthz"=w290, "Main Screen.Depth (µm)"=w289, "Main Screen.WearGp"=w288, "Main Screen.NL Trip 2"=w287, "Main Screen.Load Disable Trip"=w286, "Main Screen.Load Reset Graph"=w285, "Main Screen.NL Display 4"=w284, "Main Screen.Main Chart 3"=w283, "Main Screen.BACK"=w282, "Main Screen.Depth Trip 2"=w281, "Main Screen.COF TRIP"=w280, "Main Screen.Friction Force (N)"=w279, "Main Screen.FF Reset Graph"=w278, "Main Screen.FF Disable Trip"=w277, "Main Screen.FF TRIP"=w276, "Main Screen.COF Disable Trip"=w275, "Main Screen.COF Reset Graph"=w274, "Main Screen.FF Tab"=w268, "Main Screen.Start Test Temp"=w273, "Main Screen.zFF"=w272, "Main Screen.Friction Force (N) Graph"=w271, "Main Screen.Coefficient of Friction"=w270, "Main Screen.Scratch Start Test"=w269, "Main Screen.Cyclic Friction Force (N)"=w267, "Main Screen.CZ FF"=w266, "Main Screen.Cyclic Friction Force (N) Graph"=w265, "Main Screen.Cyclic Coefficient of Friction"=w264, "Main Screen.Cyclic FF TRIP"=w263, "Main Screen.Cyclic FF Disable Trip"=w262, "Main Screen.cyclic COF Disable Trip"=w261, "Main Screen.cyclic COF TRIP"=w260, "Main Screen.cyclic COF Reset Graph"=w259, "Main Screen.Cyclic FF Reset Graph"=w258, "Main Screen.Multi Scratch Pass"=w256, "Main Screen.Scratch Start Recording"=w255) -> (w355:T20)
    }
    frame #9 {
      n283 = control-ref of="gFF Rot 7"() -> (w357:refnum<vi>)
      n284 = control-ref of="Ramp"() -> (w362:refnum<vi>)
      n285 = control-ref of="apply load"() -> (w360:refnum<vi>)
      n286 = control-ref of="Bypass Load"() -> (w358:refnum<vi>)
      n287 = control-ref of="Vertical load (N)"() -> (w361:refnum<vi>)
      n288 = control-ref of="Enter ByPass Load"() -> (w359:refnum<vi>)
      n289 = Bundle By Name(cluster=w364, "PID.Ramp"=w362, "PID.Vertical load (N)"=w361, "PID.apply load"=w360, "PID.Enter ByPass Load"=w359, "PID.Bypass Load"=w358, "PID.gFF Rot"=w357) -> (w363:T20)
    }
    frame #10 {
      n290 = control-ref of="DEPTH TRIP   ENABLE"() -> (w381:refnum<vi>)
      n291 = control-ref of="LOAD TRIP  ENABLE"() -> (w380:refnum<vi>)
      n292 = control-ref of="CYCLIC COF TRIP  ENABLE"() -> (w375:refnum<vi>)
      n293 = control-ref of="CYCLIC FF TRIP  ENABLE"() -> (w374:refnum<vi>)
      n294 = control-ref of="FF TRIP  ENABLE"() -> (w373:refnum<vi>)
      n295 = control-ref of="COF TRIP  ENABLE"() -> (w372:refnum<vi>)
      n296 = control-ref of="Rotary Vertical"() -> (w370:refnum<vi>)
      n297 = control-ref of="Traction"() -> (w369:refnum<vi>)
      n298 = control-ref of="Scratch"() -> (w368:refnum<vi>)
      n299 = control-ref of="LRM CAM"() -> (w367:refnum<vi>)
      n300 = control-ref of="Sway LRM"() -> (w366:refnum<vi>)
      n301 = control-ref of="Rotary Horizontal"() -> (w365:refnum<vi>)
      n302 = control-ref of="Re-initilaize"() -> (w427:refnum<vi>)
      n303 = control-ref of="Filter ON/OFF"() -> (w426:refnum<vi>)
      n304 = control-ref of="Apply Filter (FF)"() -> (w422:refnum<vi>)
      n305 = control-ref of="Apply Filter (Load)"() -> (w420:refnum<vi>)
      n306 = control-ref of="SAVE  2"() -> (w415:refnum<vi>)
      n307 = control-ref of="Enter Distance"() -> (w414:refnum<vi>)
      n308 = control-ref of="Heave Loop Delay"() -> (w390:refnum<vi>)
      n309 = control-ref of="Heave PID Speed"() -> (w389:refnum<vi>)
      n310 = control-ref of="Surge Jog Speed"() -> (w388:refnum<vi>)
      n311 = control-ref of="Heave Jog Speed"() -> (w387:refnum<vi>)
      n312 = control-ref of="Sway Loop Delay"() -> (w386:refnum<vi>)
      n313 = control-ref of="Sway PID Speed"() -> (w385:refnum<vi>)
      n314 = control-ref of="Sway Jog Speed"() -> (w384:refnum<vi>)
      n315 = control-ref of="DEPTH TRIP VALUE"() -> (w383:refnum<vi>)
      n316 = control-ref of="LOAD TRIP VALUE"() -> (w382:refnum<vi>)
      n317 = control-ref of="CYCLIC FF TRIP VALUE"() -> (w379:refnum<vi>)
      n318 = control-ref of="FF TRIP VALUE"() -> (w378:refnum<vi>)
      n319 = control-ref of="CYCLIC CoF TRIP VALUE"() -> (w377:refnum<vi>)
      n320 = control-ref of="COF TRIP VALUE"() -> (w376:refnum<vi>)
      n321 = control-ref of="JOG TRIP LOAD VALUE (N)"() -> (w371:refnum<vi>)
      n322 = control-ref of="SAMPLES"() -> (w428:refnum<vi>)
      n323 = control-ref of="TracHomeSurgeOffsetCounts 10MM"() -> (w425:refnum<vi>)
      n324 = control-ref of="TracHomeSwayOffsetCounts 10MM"() -> (w424:refnum<vi>)
      n325 = control-ref of="Acoustic Emission:"() -> (w423:refnum<vi>)
      n326 = control-ref of="Filter% 2"() -> (w421:refnum<vi>)
      n327 = control-ref of="Filter%"() -> (w419:refnum<vi>)
      n328 = control-ref of="Sway distance (mm)"() -> (w418:refnum<vi>)
      n329 = control-ref of="Surge distance (mm)"() -> (w417:refnum<vi>)
      n330 = control-ref of="DataSavingLoopDelay(ms)"() -> (w416:refnum<vi>)
      n331 = control-ref of="Sway Counts:"() -> (w413:refnum<vi>)
      n332 = control-ref of="Distance (mm): 3"() -> (w412:refnum<vi>)
      n333 = control-ref of="Surge Counts:"() -> (w411:refnum<vi>)
      n334 = control-ref of="Distance (mm): 2"() -> (w410:refnum<vi>)
      n335 = control-ref of="Distance (mm):"() -> (w409:refnum<vi>)
      n336 = control-ref of="Heave Counts:"() -> (w408:refnum<vi>)
      n337 = control-ref of="LRMHomeSurgeOffsetCounts"() -> (w407:refnum<vi>)
      n338 = control-ref of="LRMHomeSwayOffsetCounts"() -> (w406:refnum<vi>)
      n339 = control-ref of="TracHomeSurgeOffsetCounts 20MM"() -> (w405:refnum<vi>)
      n340 = control-ref of="TracHomeSwayOffsetCounts 20MM"() -> (w404:refnum<vi>)
      n341 = control-ref of="RotHomeSwayOffsetCounts"() -> (w403:refnum<vi>)
      n342 = control-ref of="RotHomeSurgeOffsetCounts"() -> (w402:refnum<vi>)
      n343 = control-ref of="Heave distance"() -> (w401:refnum<vi>)
      n344 = control-ref of="Zmm"() -> (w400:refnum<vi>)
      n345 = control-ref of="Heave Pulses/mm"() -> (w399:refnum<vi>)
      n346 = control-ref of="Surge Pulses/mm"() -> (w398:refnum<vi>)
      n347 = control-ref of="Sway Pulses/mm"() -> (w397:refnum<vi>)
      n348 = control-ref of="Heave Pitch"() -> (w396:refnum<vi>)
      n349 = control-ref of="Surge Pitch"() -> (w395:refnum<vi>)
      n350 = control-ref of="Sway Pitch"() -> (w394:refnum<vi>)
      n351 = control-ref of="Heave PPR"() -> (w393:refnum<vi>)
      n352 = control-ref of="Surge PPR"() -> (w392:refnum<vi>)
      n353 = control-ref of="Sway PPR"() -> (w391:refnum<vi>)
      n354 = Bundle By Name(cluster=w430, "Config Parameters.SAMPLES"=w428, "Config Parameters.Re-initilaize"=w427, "Config Parameters.Filter ON/OFF"=w426, "Config Parameters.TracHomeSurgeOffsetCounts 10MM"=w425, "Config Parameters.TracHomeSwayOffsetCounts 10MM"=w424, "Config Parameters.Acoustic Emission:"=w423, "Config Parameters.Apply Filter (FF)"=w422, "Config Parameters.Filter% 2"=w421, "Config Parameters.Apply Filter (Load)"=w420, "Config Parameters.Filter%"=w419, "Config Parameters.Sway distance (mm)"=w418, "Config Parameters.Surge distance (mm)"=w417, "Config Parameters.DataSavingLoopDelay(ms)"=w416, "Config Parameters.SAVE 2"=w415, "Config Parameters.Enter Distance"=w414, "Config Parameters.Sway Counts:"=w413, "Config Parameters.Distance (mm): 3"=w412, "Config Parameters.Surge Counts:"=w411, "Config Parameters.Distance (mm): 2"=w410, "Config Parameters.Distance (mm):"=w409, "Config Parameters.Heave Counts:"=w408, "Config Parameters.LRMHomeSurgeOffsetCounts"=w407, "Config Parameters.LRMHomeSwayOffsetCounts"=w406, "Config Parameters.TracHomeSurgeOffsetCounts 20MM"=w405, "Config Parameters.TracHomeSwayOffsetCounts 20MM"=w404, "Config Parameters.RotHomeSwayOffsetCounts"=w403, "Config Parameters.RotHomeSurgeOffsetCounts"=w402, "Config Parameters.Heave distance"=w401, "Config Parameters.Zmm"=w400, "Config Parameters.Heave Pulses/mm"=w399, "Config Parameters.Surge Pulses/mm"=w398, "Config Parameters.Sway Pulses/mm"=w397, "Config Parameters.Heave Pitch"=w396, "Config Parameters.Surge Pitch"=w395, "Config Parameters.Sway Pitch"=w394, "Config Parameters.Heave PPR"=w393, "Config Parameters.Surge PPR"=w392, "Config Parameters.Sway PPR"=w391, "Config Parameters.Heave Loop Delay"=w390, "Config Parameters.Heave PID Speed"=w389, "Config Parameters.Surge Jog Speed"=w388, "Config Parameters.Heave Jog Speed"=w387, "Config Parameters.Sway Loop Delay"=w386, "Config Parameters.Sway PID Speed"=w385, "Config Parameters.Sway Jog Speed"=w384, "Config Parameters.DEPTH TRIP VALUE"=w383, "Config Parameters.LOAD TRIP VALUE"=w382, "Config Parameters.DEPTH TRIP   ENABLE"=w381, "Config Parameters.LOAD TRIP  ENABLE"=w380, "Config Parameters.CYCLIC FF TRIP VALUE"=w379, "Config Parameters.FF TRIP VALUE"=w378, "Config Parameters.CYCLIC CoF TRIP VALUE"=w377, "Config Parameters.COF TRIP VALUE"=w376, "Config Parameters.CYCLIC COF TRIP  ENABLE"=w375, "Config Parameters.CYCLIC FF TRIP  ENABLE"=w374, "Config Parameters.FF TRIP  ENABLE"=w373, "Config Parameters.COF TRIP  ENABLE"=w372, "Config Parameters.JOG TRIP LOAD VALUE (N)"=w371, "Config Parameters.Rotary Vertical"=w370, "Config Parameters.Traction"=w369, "Config Parameters.Scratch"=w368, "Config Parameters.LRM CAM"=w367, "Config Parameters.Sway LRM"=w366, "Config Parameters.Rotary Horizontal"=w365) -> (w429:T20)
    }
    frame #11 {
      n355 = control-ref of="FORCE (N)"() -> (w433:refnum<vi>)
      n356 = control-ref of="TORQUE (N-m)"() -> (w432:refnum<vi>)
      n357 = control-ref of="ClearAll"() -> (w445:refnum<vi>)
      n358 = control-ref of="ZeroAll"() -> (w443:refnum<vi>)
      n359 = control-ref of="running_flag"() -> (w435:refnum<vi>)
      n360 = control-ref of="Load Cell Temp"() -> (w434:refnum<vi>)
      n361 = control-ref of="Save Dwell"() -> (w444:refnum<vi>)
      n362 = control-ref of="Acq Delay (ms)"() -> (w442:refnum<vi>)
      n363 = control-ref of="Burst Delay (ms)"() -> (w441:refnum<vi>)
      n364 = control-ref of="SN"() -> (w439:refnum<vi>)
      n365 = control-ref of="Port"() -> (w437:refnum<vi>)
      n366 = control-ref of="Load Cell Link"() -> (w431:refnum<vi>)
      n367 = control-ref of="model"() -> (w440:refnum<vi>)
      n368 = control-ref of="Sensor IP"() -> (w438:refnum<vi>)
      n369 = control-ref of="ft_data"() -> (w436:refnum<vi>)
      n370 = Bundle By Name(cluster=w447, "Loading Com Port.ClearAll"=w445, "Loading Com Port.Save Dwell"=w444, "Loading Com Port.ZeroAll"=w443, "Loading Com Port.Acq Delay (ms)"=w442, "Loading Com Port.Burst Delay (ms)"=w441, "Loading Com Port.model"=w440, "Loading Com Port.SN"=w439, "Loading Com Port.Sensor IP"=w438, "Loading Com Port.Port"=w437, "Loading Com Port.ft_data"=w436, "Loading Com Port.running_flag"=w435, "Loading Com Port.Load Cell Temp"=w434, "Loading Com Port.FORCE (N)"=w433, "Loading Com Port.TORQUE (N-m)"=w432, "Loading Com Port.Load Cell Link"=w431) -> (w446:T20)
    }
    frame #12 {
      n371 = control-ref of="Read Heave Temp"() -> (w493:refnum<vi>)
      n372 = control-ref of="Manual Write Heave & Surge"() -> (w470:refnum<vi>)
      n373 = control-ref of="error out Read"() -> (w505:refnum<vi>)
      n374 = control-ref of="error out Write"() -> (w500:refnum<vi>)
      n375 = control-ref of="UPLINK HEAVE"() -> (w449:refnum<vi>)
      n376 = control-ref of="DOWNLINK HEAVE"() -> (w448:refnum<vi>)
      n377 = control-ref of="SURGE POSE"() -> (w506:refnum<vi>)
      n378 = control-ref of="HEAVE POSE"() -> (w504:refnum<vi>)
      n379 = control-ref of="State"() -> (w503:refnum<vi>)
      n380 = control-ref of="Homed"() -> (w502:refnum<vi>)
      n381 = control-ref of="Sequence ID"() -> (w501:refnum<vi>)
      n382 = control-ref of="faultCode"() -> (w499:refnum<vi>)
      n383 = control-ref of="Ack ID"() -> (w498:refnum<vi>)
      n384 = control-ref of="SPEED"() -> (w497:refnum<vi>)
      n385 = control-ref of="Distance"() -> (w496:refnum<vi>)
      n386 = control-ref of="Mode Command"() -> (w495:refnum<vi>)
      n387 = control-ref of="SPARE 2"() -> (w492:refnum<vi>)
      n388 = control-ref of="SPARE 1"() -> (w491:refnum<vi>)
      n389 = control-ref of="Spare 15"() -> (w490:refnum<vi>)
      n390 = control-ref of="Spare 14"() -> (w489:refnum<vi>)
      n391 = control-ref of="Spare 13"() -> (w488:refnum<vi>)
      n392 = control-ref of="Spare 12"() -> (w487:refnum<vi>)
      n393 = control-ref of="Spare 11"() -> (w486:refnum<vi>)
      n394 = control-ref of="Spare 10"() -> (w485:refnum<vi>)
      n395 = control-ref of="Spare 9"() -> (w484:refnum<vi>)
      n396 = control-ref of="Spare 8"() -> (w483:refnum<vi>)
      n397 = control-ref of="Spare 5"() -> (w482:refnum<vi>)
      n398 = control-ref of="Spare 4"() -> (w481:refnum<vi>)
      n399 = control-ref of="Spare 3"() -> (w480:refnum<vi>)
      n400 = control-ref of="Spare 2"() -> (w479:refnum<vi>)
      n401 = control-ref of="Spare 1"() -> (w478:refnum<vi>)
      n402 = control-ref of="Humidity"() -> (w477:refnum<vi>)
      n403 = control-ref of="Temp"() -> (w476:refnum<vi>)
      n404 = control-ref of="Node Id"() -> (w475:refnum<vi>)
      n405 = control-ref of="SPARE 3"() -> (w474:refnum<vi>)
      n406 = control-ref of="SPARE 4"() -> (w473:refnum<vi>)
      n407 = control-ref of="fwMajor"() -> (w472:refnum<vi>)
      n408 = control-ref of="fwMinor"() -> (w471:refnum<vi>)
      n409 = control-ref of="SPARE 5"() -> (w468:refnum<vi>)
      n410 = control-ref of="Reserved"() -> (w467:refnum<vi>)
      n411 = control-ref of="SPARE 8"() -> (w466:refnum<vi>)
      n412 = control-ref of="SPARE 6"() -> (w465:refnum<vi>)
      n413 = control-ref of="SPARE 7"() -> (w464:refnum<vi>)
      n414 = control-ref of="SPARE 17"() -> (w463:refnum<vi>)
      n415 = control-ref of="SPARE 16"() -> (w462:refnum<vi>)
      n416 = control-ref of="SPARE 15"() -> (w461:refnum<vi>)
      n417 = control-ref of="SPARE 14"() -> (w460:refnum<vi>)
      n418 = control-ref of="SPARE 13"() -> (w459:refnum<vi>)
      n419 = control-ref of="SPARE 12"() -> (w458:refnum<vi>)
      n420 = control-ref of="SPARE 11"() -> (w457:refnum<vi>)
      n421 = control-ref of="SPARE 10"() -> (w456:refnum<vi>)
      n422 = control-ref of="SPARE 9"() -> (w455:refnum<vi>)
      n423 = control-ref of="System UPTIME"() -> (w454:refnum<vi>)
      n424 = control-ref of="Missed Packets"() -> (w453:refnum<vi>)
      n425 = control-ref of="faultCode Surge Right"() -> (w452:refnum<vi>)
      n426 = control-ref of="faultCode Surge Left"() -> (w451:refnum<vi>)
      n427 = control-ref of="faultCode Heave"() -> (w450:refnum<vi>)
      n428 = control-ref of="Heave and Surge Read"() -> (w494:refnum<vi>)
      n429 = control-ref of="Heave and Surge Write"() -> (w469:refnum<vi>)
      n430 = Bundle By Name(cluster=w508, "Heave AND Surge.SURGE POSE"=w506, "Heave AND Surge.error out Read"=w505, "Heave AND Surge.HEAVE POSE"=w504, "Heave AND Surge.State"=w503, "Heave AND Surge.Homed"=w502, "Heave AND Surge.Sequence ID"=w501, "Heave AND Surge.error out Write"=w500, "Heave AND Surge.faultCode"=w499, "Heave AND Surge.Ack ID"=w498, "Heave AND Surge.SPEED"=w497, "Heave AND Surge.Distance"=w496, "Heave AND Surge.Mode Command"=w495, "Heave AND Surge.Heave and Surge Read"=w494, "Heave AND Surge.Read Heave Temp"=w493, "Heave AND Surge.SPARE 2"=w492, "Heave AND Surge.SPARE 1"=w491, "Heave AND Surge.Spare 15"=w490, "Heave AND Surge.Spare 14"=w489, "Heave AND Surge.Spare 13"=w488, "Heave AND Surge.Spare 12"=w487, "Heave AND Surge.Spare 11"=w486, "Heave AND Surge.Spare 10"=w485, "Heave AND Surge.Spare 9"=w484, "Heave AND Surge.Spare 8"=w483, "Heave AND Surge.Spare 7"=w482, "Heave AND Surge.Spare 4"=w481, "Heave AND Surge.Spare 3"=w480, "Heave AND Surge.Spare 4"=w479, "Heave AND Surge.Spare 3"=w478, "Heave AND Surge.Spare 2"=w477, "Heave AND Surge.Spare 1"=w476, "Heave AND Surge.Node Id"=w475, "Heave AND Surge.SPARE 3"=w474, "Heave AND Surge.SPARE 4"=w473, "Heave AND Surge.fwMajor"=w472, "Heave AND Surge.fwMinor"=w471, "Heave AND Surge.Manual Write"=w470, "Heave AND Surge.Heave and Surge Write"=w469, "Heave AND Surge.SPARE 5"=w468, "Heave AND Surge.Reserved"=w467, "Heave AND Surge.SPARE 8"=w466, "Heave AND Surge.SPARE 6"=w465, "Heave AND Surge.SPARE 7"=w464, "Heave AND Surge.SPARE 17"=w463, "Heave AND Surge.SPARE 16"=w462, "Heave AND Surge.SPARE 15"=w461, "Heave AND Surge.SPARE 14"=w460, "Heave AND Surge.SPARE 13"=w459, "Heave AND Surge.SPARE 12"=w458, "Heave AND Surge.SPARE 11"=w457, "Heave AND Surge.SPARE 10"=w456, "Heave AND Surge.SPARE 9"=w455, "Heave AND Surge.System UPTIME"=w454, "Heave AND Surge.Missed Packets"=w453, "Heave AND Surge.faultCode Surge Right"=w452, "Heave AND Surge.faultCode Surge Left"=w451, "Heave AND Surge.faultCode Heave"=w450, "Heave AND Surge.UPLINK HEAVE"=w449, "Heave AND Surge.DOWNLINK HEAVE"=w448) -> (w507:T20)
    }
    frame #13 {
      n431 = control-ref of="PID"() -> (w509:refnum<vi>)
      n432 = control-ref of="Fine Tune Zone"() -> (w529:refnum<vi>)
      n433 = control-ref of="PID Delay (sec)"() -> (w528:refnum<vi>)
      n434 = control-ref of="Max_pos_limit"() -> (w527:refnum<vi>)
      n435 = control-ref of="Min_pos_limit"() -> (w526:refnum<vi>)
      n436 = control-ref of="i_limit"() -> (w525:refnum<vi>)
      n437 = control-ref of="pct_scale"() -> (w516:refnum<vi>)
      n438 = control-ref of="Deadband"() -> (w524:refnum<vi>)
      n439 = control-ref of="Kd"() -> (w523:refnum<vi>)
      n440 = control-ref of="Ki"() -> (w522:refnum<vi>)
      n441 = control-ref of="Kp"() -> (w521:refnum<vi>)
      n442 = control-ref of="Current Position"() -> (w520:refnum<vi>)
      n443 = control-ref of="Set Load"() -> (w519:refnum<vi>)
      n444 = control-ref of="Current Load"() -> (w518:refnum<vi>)
      n445 = control-ref of="Pulse delta"() -> (w517:refnum<vi>)
      n446 = control-ref of="Init Step"() -> (w515:refnum<vi>)
      n447 = control-ref of="Max Step Linit"() -> (w514:refnum<vi>)
      n448 = control-ref of="min_deadband_floor"() -> (w513:refnum<vi>)
      n449 = control-ref of="dynamic_spindle_noise_scalar"() -> (w512:refnum<vi>)
      n450 = control-ref of="min_finetune_floor"() -> (w511:refnum<vi>)
      n451 = control-ref of="filter_alpha"() -> (w510:refnum<vi>)
      n452 = Bundle By Name(cluster=w531, "New PID LOGIC.Fine Tune Zone"=w529, "New PID LOGIC.PID SDelay"=w528, "New PID LOGIC.Max_pos_limit"=w527, "New PID LOGIC.Min_pos_limit"=w526, "New PID LOGIC.i_limit"=w525, "New PID LOGIC.pct_scale"=w516, "New PID LOGIC.Deadband"=w524, "New PID LOGIC.Kd"=w523, "New PID LOGIC.Ki"=w522, "New PID LOGIC.Kp"=w521, "New PID LOGIC.Current Position"=w520, "New PID LOGIC.Set Load"=w519, "New PID LOGIC.Current Load"=w518, "New PID LOGIC.Pulse delta"=w517, "New PID LOGIC.Init Step"=w515, "New PID LOGIC.Max Step Linit"=w514, "New PID LOGIC.min_deadband_floor"=w513, "New PID LOGIC.dynamic_spindle_noise_scalar"=w512, "New PID LOGIC.min_finetune_floor"=w511, "New PID LOGIC.filter_alpha"=w510, "New PID LOGIC.PID"=w509) -> (w530:T20)
    }
    frame #14 {
      n453 = control-ref of="Manual Write SWAY"() -> (w570:refnum<vi>)
      n454 = control-ref of="Read SWAY Temp"() -> (w551:refnum<vi>)
      n455 = control-ref of="error out Write  SWAY"() -> (w572:refnum<vi>)
      n456 = control-ref of="error out Read SWAY"() -> (w571:refnum<vi>)
      n457 = control-ref of="faultCode Rotary"() -> (w534:refnum<vi>)
      n458 = control-ref of="UPLINK SWAY"() -> (w533:refnum<vi>)
      n459 = control-ref of="DOWNLINK SWAY"() -> (w532:refnum<vi>)
      n460 = control-ref of="fwMajor"() -> (w589:refnum<vi>)
      n461 = control-ref of="Homed"() -> (w588:refnum<vi>)
      n462 = control-ref of="Rotary POSE"() -> (w587:refnum<vi>)
      n463 = control-ref of="State"() -> (w586:refnum<vi>)
      n464 = control-ref of="SWAY POSE"() -> (w585:refnum<vi>)
      n465 = control-ref of="Ack ID"() -> (w584:refnum<vi>)
      n466 = control-ref of="faultCode"() -> (w583:refnum<vi>)
      n467 = control-ref of="Node Id"() -> (w582:refnum<vi>)
      n468 = control-ref of="fwMinor"() -> (w581:refnum<vi>)
      n469 = control-ref of="Spare 6"() -> (w580:refnum<vi>)
      n470 = control-ref of="Spare 5"() -> (w579:refnum<vi>)
      n471 = control-ref of="Spare 4"() -> (w578:refnum<vi>)
      n472 = control-ref of="Spare 3"() -> (w577:refnum<vi>)
      n473 = control-ref of="Spare 2"() -> (w576:refnum<vi>)
      n474 = control-ref of="Spare 1"() -> (w575:refnum<vi>)
      n475 = control-ref of="Spare 7"() -> (w574:refnum<vi>)
      n476 = control-ref of="SPARE  5"() -> (w573:refnum<vi>)
      n477 = control-ref of="SPARE  4"() -> (w568:refnum<vi>)
      n478 = control-ref of="SPARE  3"() -> (w567:refnum<vi>)
      n479 = control-ref of="SPARE 2"() -> (w566:refnum<vi>)
      n480 = control-ref of="SPARE1"() -> (w565:refnum<vi>)
      n481 = control-ref of="Spare 15"() -> (w564:refnum<vi>)
      n482 = control-ref of="Spare 14"() -> (w563:refnum<vi>)
      n483 = control-ref of="Spare 13"() -> (w562:refnum<vi>)
      n484 = control-ref of="Spare 12"() -> (w561:refnum<vi>)
      n485 = control-ref of="Spare 11"() -> (w560:refnum<vi>)
      n486 = control-ref of="Spare 9"() -> (w559:refnum<vi>)
      n487 = control-ref of="Spare 8"() -> (w558:refnum<vi>)
      n488 = control-ref of="SPEED"() -> (w557:refnum<vi>)
      n489 = control-ref of="Distance"() -> (w556:refnum<vi>)
      n490 = control-ref of="Mode Command"() -> (w555:refnum<vi>)
      n491 = control-ref of="Sequence ID"() -> (w554:refnum<vi>)
      n492 = control-ref of="Spare 10"() -> (w552:refnum<vi>)
      n493 = control-ref of="faultCode Sway"() -> (w550:refnum<vi>)
      n494 = control-ref of="Missed Packets"() -> (w549:refnum<vi>)
      n495 = control-ref of="System UPTIME"() -> (w548:refnum<vi>)
      n496 = control-ref of="SPARE 6"() -> (w547:refnum<vi>)
      n497 = control-ref of="SPARE 7"() -> (w546:refnum<vi>)
      n498 = control-ref of="SPARE 9"() -> (w545:refnum<vi>)
      n499 = control-ref of="SPARE 11"() -> (w544:refnum<vi>)
      n500 = control-ref of="SPARE 10"() -> (w543:refnum<vi>)
      n501 = control-ref of="SPARE 8"() -> (w542:refnum<vi>)
      n502 = control-ref of="SPARE 13"() -> (w541:refnum<vi>)
      n503 = control-ref of="SPARE 12"() -> (w540:refnum<vi>)
      n504 = control-ref of="SPARE 17"() -> (w539:refnum<vi>)
      n505 = control-ref of="SPARE 16"() -> (w538:refnum<vi>)
      n506 = control-ref of="SPARE 15"() -> (w537:refnum<vi>)
      n507 = control-ref of="SPARE 14"() -> (w536:refnum<vi>)
      n508 = control-ref of="Reserved"() -> (w535:refnum<vi>)
      n509 = control-ref of="SWAY WRITE"() -> (w569:refnum<vi>)
      n510 = control-ref of="SWAY READ"() -> (w553:refnum<vi>)
      n511 = Bundle By Name(cluster=w591, "SWAY.fwMajor"=w589, "SWAY.Homed"=w588, "SWAY.Rotary POSE"=w587, "SWAY.State"=w586, "SWAY.SWAY POSE"=w585, "SWAY.Ack ID"=w584, "SWAY.faultCode"=w583, "SWAY.Node Id"=w582, "SWAY.fwMinor"=w581, "SWAY.Spare 6"=w580, "SWAY.Spare 5"=w579, "SWAY.Spare 4"=w578, "SWAY.Spare 3"=w577, "SWAY.Spare 2"=w576, "SWAY.Spare 1"=w575, "SWAY.Spare 7"=w574, "SWAY.SPARE  5"=w573, "SWAY.error out Write  SWAY"=w572, "SWAY.error out Read SWAY"=w571, "SWAY.Manual Write SWAY"=w570, "SWAY.SWAY WRITE"=w569, "SWAY.SPARE  4"=w568, "SWAY.SPARE  3"=w567, "SWAY.SPARE 2"=w566, "SWAY.SPARE 1"=w565, "SWAY.Spare 15"=w564, "SWAY.Spare 14"=w563, "SWAY.Spare 13"=w562, "SWAY.Spare 12"=w561, "SWAY.Spare 11"=w560, "SWAY.Spare 9"=w559, "SWAY.Spare 8"=w558, "SWAY.SPEED"=w557, "SWAY.Distance"=w556, "SWAY.Mode Command"=w555, "SWAY.Sequence ID"=w554, "SWAY.SWAY READ"=w553, "SWAY.Spare 10"=w552, "SWAY.Read SWAY Temp"=w551, "SWAY.faultCode Sway"=w550, "SWAY.Missed Packets"=w549, "SWAY.System UPTIME sway"=w548, "SWAY.SPARE 6"=w547, "SWAY.SPARE 7"=w546, "SWAY.SPARE 9"=w545, "SWAY.SPARE 11"=w544, "SWAY.SPARE 10"=w543, "SWAY.SPARE 8"=w542, "SWAY.SPARE 13"=w541, "SWAY.SPARE 12"=w540, "SWAY.SPARE 17"=w539, "SWAY.SPARE 16"=w538, "SWAY.SPARE 15"=w537, "SWAY.SPARE 14"=w536, "SWAY.Reserved"=w535, "SWAY.faultCode Rotary"=w534, "SWAY.UPLINK SWAY"=w533, "SWAY.DOWNLINK SWAY"=w532) -> (w590:T20)
    }
    frame #15 {
      n512 = control-ref of="Analysis Home new"() -> (w622:refnum<vi>)
      n513 = control-ref of="Refresh 2"() -> (w621:refnum<vi>)
      n514 = control-ref of="OPEN 4"() -> (w607:refnum<vi>)
      n515 = control-ref of="OPEN 3"() -> (w605:refnum<vi>)
      n516 = control-ref of="XY Graph"() -> (w600:refnum<vi>)
      n517 = control-ref of="OPEN 2"() -> (w597:refnum<vi>)
      n518 = control-ref of="OPEN 1"() -> (w596:refnum<vi>)
      n519 = control-ref of="Export"() -> (w593:refnum<vi>)
      n520 = control-ref of="MEAN"() -> (w620:refnum<vi>)
      n521 = control-ref of="SD"() -> (w619:refnum<vi>)
      n522 = control-ref of="VARIANCE"() -> (w618:refnum<vi>)
      n523 = control-ref of="MEAN"() -> (w617:refnum<vi>)
      n524 = control-ref of="SD"() -> (w616:refnum<vi>)
      n525 = control-ref of="VARIANCE"() -> (w615:refnum<vi>)
      n526 = control-ref of="MEAN"() -> (w614:refnum<vi>)
      n527 = control-ref of="SD"() -> (w613:refnum<vi>)
      n528 = control-ref of="VARIANCE"() -> (w612:refnum<vi>)
      n529 = control-ref of="MEAN"() -> (w611:refnum<vi>)
      n530 = control-ref of="SD"() -> (w610:refnum<vi>)
      n531 = control-ref of="VARIANCE"() -> (w609:refnum<vi>)
      n532 = control-ref of="File 4 Discription"() -> (w608:refnum<vi>)
      n533 = control-ref of="File Name 4"() -> (w606:refnum<vi>)
      n534 = control-ref of="File 3 Discription"() -> (w604:refnum<vi>)
      n535 = control-ref of="File Name 3"() -> (w603:refnum<vi>)
      n536 = control-ref of="File Name 2"() -> (w599:refnum<vi>)
      n537 = control-ref of="File Name 1"() -> (w598:refnum<vi>)
      n538 = control-ref of="File 1 Discription"() -> (w595:refnum<vi>)
      n539 = control-ref of="File 2 Discription"() -> (w594:refnum<vi>)
      n540 = control-ref of="Y-AXIS"() -> (w602:refnum<vi>)
      n541 = control-ref of="X-AXIS"() -> (w601:refnum<vi>)
      n542 = control-ref of="File Format"() -> (w592:refnum<vi>)
      n543 = Bundle By Name(cluster=w624, "Analysis Screen.Analysis Home"=w622, "Analysis Screen.Refresh 2"=w621, "Analysis Screen.MEAN 4"=w620, "Analysis Screen.SD 4"=w619, "Analysis Screen.VARIANCE 4"=w618, "Analysis Screen.MEAN  3"=w617, "Analysis Screen.SD  3"=w616, "Analysis Screen.VARIANCE  3"=w615, "Analysis Screen.MEAN 2"=w614, "Analysis Screen.SD  2"=w613, "Analysis Screen.VARIANCE 2"=w612, "Analysis Screen.MEAN"=w611, "Analysis Screen.SD"=w610, "Analysis Screen.VARIANCE"=w609, "Analysis Screen.File 4 Discription"=w608, "Analysis Screen.OPEN 4"=w607, "Analysis Screen.File Name 4"=w606, "Analysis Screen.OPEN 3"=w605, "Analysis Screen.File 3 Discription"=w604, "Analysis Screen.File Name 3"=w603, "Analysis Screen.Y-AXIS"=w602, "Analysis Screen.X-AXIS"=w601, "Analysis Screen.XY Graph"=w600, "Analysis Screen.File Name 2"=w599, "Analysis Screen.File Name 1"=w598, "Analysis Screen.OPEN 2"=w597, "Analysis Screen.OPEN 1"=w596, "Analysis Screen.File 1 Discription"=w595, "Analysis Screen.File 2 Discription"=w594, "Analysis Screen.Export"=w593, "Analysis Screen.File Format"=w592) -> (w623:T20)
    }
    frame #16 {
      n544 = control-ref of="Manual Write TRACTION"() -> (w656:refnum<vi>)
      n545 = control-ref of="Read TRACTION Temp"() -> (w643:refnum<vi>)
      n546 = control-ref of="error out Read TRACTION"() -> (w630:refnum<vi>)
      n547 = control-ref of="error out Write  TRACTION"() -> (w629:refnum<vi>)
      n548 = control-ref of="Downlink traction"() -> (w626:refnum<vi>)
      n549 = control-ref of="Uplink Traction 2"() -> (w625:refnum<vi>)
      n550 = control-ref of="Spare 3"() -> (w627:refnum<vi>)
      n551 = control-ref of="faultCode Traction 2"() -> (w674:refnum<vi>)
      n552 = control-ref of="faultCode Traction 1"() -> (w673:refnum<vi>)
      n553 = control-ref of="Missed Packets"() -> (w672:refnum<vi>)
      n554 = control-ref of="System UPTIME"() -> (w671:refnum<vi>)
      n555 = control-ref of="SPARE 17"() -> (w670:refnum<vi>)
      n556 = control-ref of="SPARE 16"() -> (w669:refnum<vi>)
      n557 = control-ref of="SPARE 15"() -> (w668:refnum<vi>)
      n558 = control-ref of="SPARE 14"() -> (w667:refnum<vi>)
      n559 = control-ref of="SPARE 13"() -> (w666:refnum<vi>)
      n560 = control-ref of="SPARE 12"() -> (w665:refnum<vi>)
      n561 = control-ref of="SPARE 11"() -> (w664:refnum<vi>)
      n562 = control-ref of="SPARE 10"() -> (w663:refnum<vi>)
      n563 = control-ref of="SPARE 9"() -> (w662:refnum<vi>)
      n564 = control-ref of="SPARE 8"() -> (w661:refnum<vi>)
      n565 = control-ref of="SPARE 7"() -> (w660:refnum<vi>)
      n566 = control-ref of="SPARE 6"() -> (w659:refnum<vi>)
      n567 = control-ref of="Reserved"() -> (w658:refnum<vi>)
      n568 = control-ref of="SPARE  5"() -> (w657:refnum<vi>)
      n569 = control-ref of="SPARE  4"() -> (w654:refnum<vi>)
      n570 = control-ref of="SPARE  3"() -> (w653:refnum<vi>)
      n571 = control-ref of="SPARE 2"() -> (w652:refnum<vi>)
      n572 = control-ref of="SPARE 1"() -> (w651:refnum<vi>)
      n573 = control-ref of="Spare 7"() -> (w650:refnum<vi>)
      n574 = control-ref of="Spare 6"() -> (w649:refnum<vi>)
      n575 = control-ref of="Spare 5"() -> (w648:refnum<vi>)
      n576 = control-ref of="Spare 4"() -> (w647:refnum<vi>)
      n577 = control-ref of="Spare 2"() -> (w646:refnum<vi>)
      n578 = control-ref of="Spare 1"() -> (w645:refnum<vi>)
      n579 = control-ref of="Node Id"() -> (w644:refnum<vi>)
      n580 = control-ref of="fwMinor"() -> (w642:refnum<vi>)
      n581 = control-ref of="fwMajor"() -> (w641:refnum<vi>)
      n582 = control-ref of="faultCode"() -> (w640:refnum<vi>)
      n583 = control-ref of="TRACTION POSE 2"() -> (w639:refnum<vi>)
      n584 = control-ref of="TRACTION POSE 1"() -> (w638:refnum<vi>)
      n585 = control-ref of="Homed"() -> (w637:refnum<vi>)
      n586 = control-ref of="State"() -> (w636:refnum<vi>)
      n587 = control-ref of="Ack ID"() -> (w635:refnum<vi>)
      n588 = control-ref of="SPEED"() -> (w634:refnum<vi>)
      n589 = control-ref of="Distance"() -> (w633:refnum<vi>)
      n590 = control-ref of="Mode Command"() -> (w632:refnum<vi>)
      n591 = control-ref of="Sequence ID"() -> (w631:refnum<vi>)
      n592 = control-ref of="TRACTION WRITE"() -> (w655:refnum<vi>)
      n593 = control-ref of="TRACTION READ"() -> (w628:refnum<vi>)
      n594 = Bundle By Name(cluster=w676, "Traction.faultCode Traction 2"=w674, "Traction.faultCode Traction 1"=w673, "Traction.Missed Packets"=w672, "Traction.System UPTIME Traction"=w671, "Traction.SPARE 17"=w670, "Traction.SPARE 16"=w669, "Traction.SPARE 15"=w668, "Traction.SPARE 14"=w667, "Traction.SPARE 13"=w666, "Traction.SPARE 12"=w665, "Traction.SPARE 11"=w664, "Traction.SPARE 10"=w663, "Traction.SPARE 9"=w662, "Traction.SPARE 8"=w661, "Traction.SPARE 7"=w660, "Traction.SPARE 6"=w659, "Traction.Reserved"=w658, "Traction.SPARE  5"=w657, "Traction.Manual Write TRACTION"=w656, "Traction.TRACTION WRITE"=w655, "Traction.SPARE  4"=w654, "Traction.SPARE  3"=w653, "Traction.SPARE 2"=w652, "Traction.SPARE 1"=w651, "Traction.Spare 7"=w650, "Traction.Spare 6"=w649, "Traction.Spare 5"=w648, "Traction.Spare 4"=w647, "Traction.Spare 2"=w646, "Traction.Spare 1"=w645, "Traction.Node Id"=w644, "Traction.Read TRACTION Temp"=w643, "Traction.fwMinor"=w642, "Traction.fwMajor"=w641, "Traction.faultCode"=w640, "Traction.TRACTION POSE"=w639, "Traction.TRACTION POSE 2"=w638, "Traction.Homed"=w637, "Traction.State"=w636, "Traction.Ack ID"=w635, "Traction.SPEED"=w634, "Traction.Distance"=w633, "Traction.Mode Command"=w632, "Traction.Sequence ID"=w631, "Traction.error out Read TRACTION"=w630, "Traction.error out Write  TRACTION"=w629, "Traction.TRACTION READ"=w628, "Traction.Spare 3"=w627, "Traction.Downlink traction"=w626, "Traction.Uplink Traction"=w625) -> (w675:T20)
    }
    frame #17 {
      n595 = control-ref of="Traction Receipe"() -> (w698:refnum<vi>)
      n596 = control-ref of="Total Execution Time"() -> (w709:refnum<vi>)
      n597 = control-ref of="Total Steps"() -> (w708:refnum<vi>)
      n598 = control-ref of="Duration / Step (s)"() -> (w707:refnum<vi>)
      n599 = control-ref of="Duration / Step (s)"() -> (w705:refnum<vi>)
      n600 = control-ref of="Speed (mm/s)"() -> (w703:refnum<vi>)
      n601 = control-ref of="SET entrainment Velocity"() -> (w697:refnum<vi>)
      n602 = control-ref of="Test Array Size"() -> (w696:refnum<vi>)
      n603 = control-ref of="SRR INDEX [ STRIBECK]"() -> (w695:refnum<vi>)
      n604 = control-ref of="Stribeck Size"() -> (w694:refnum<vi>)
      n605 = control-ref of="SET SRR"() -> (w693:refnum<vi>)
      n606 = control-ref of="ELAPSED TIMER"() -> (w692:refnum<vi>)
      n607 = control-ref of="BALL SET RPM"() -> (w691:refnum<vi>)
      n608 = control-ref of="DISC SET RPM"() -> (w690:refnum<vi>)
      n609 = control-ref of="SET LOAD"() -> (w689:refnum<vi>)
      n610 = control-ref of="TEMPERATURE READ"() -> (w688:refnum<vi>)
      n611 = control-ref of="SET TEMPERATURE"() -> (w687:refnum<vi>)
      n612 = control-ref of="Traction Size"() -> (w686:refnum<vi>)
      n613 = control-ref of="DISC SPEED (rpm)"() -> (w685:refnum<vi>)
      n614 = control-ref of="BALL SPEED (rpm)"() -> (w684:refnum<vi>)
      n615 = control-ref of="BALL WEAR TRACK"() -> (w683:refnum<vi>)
      n616 = control-ref of="DISC WEARTRACK"() -> (w682:refnum<vi>)
      n617 = control-ref of="SRR INDEX [ TRACTION]"() -> (w681:refnum<vi>)
      n618 = control-ref of="Start Index Type"() -> (w680:refnum<vi>)
      n619 = control-ref of="Ball (mm/sec)"() -> (w678:refnum<vi>)
      n620 = control-ref of="Disc (mm/sec)"() -> (w677:refnum<vi>)
      n621 = control-ref of="SRR Sweep Range (%)"() -> (w710:refnum<vi>)
      n622 = control-ref of="STRIBECK Fixed SRR List (%)"() -> (w706:refnum<vi>)
      n623 = control-ref of="SRR Sweep Range (%)"() -> (w704:refnum<vi>)
      n624 = control-ref of="Temperature Stages (°C)"() -> (w702:refnum<vi>)
      n625 = control-ref of="Load (N)"() -> (w701:refnum<vi>)
      n626 = control-ref of="Lubricant Name"() -> (w700:refnum<vi>)
      n627 = control-ref of="Profile File Name"() -> (w699:refnum<vi>)
      n628 = control-ref of="Enum - Menu"() -> (w679:refnum<vi>)
      n629 = Bundle By Name(cluster=w712, "Traction reciepe.SRR Sweep Range (%) Stribeck"=w710, "Traction reciepe.Traction Receipe"=w698, "Traction reciepe.Total Execution Time"=w709, "Traction reciepe.Total Steps"=w708, "Traction reciepe.Duration / Step (s)  Stribeck"=w707, "Traction reciepe.STRIBECK Fixed SRR List (%)"=w706, "Traction reciepe.Duration / Step (s) Traction"=w705, "Traction reciepe.SRR Sweep Range (%) traction"=w704, "Traction reciepe.Rolling Speed (mm/s)"=w703, "Traction reciepe.Temperature Stages (°C)"=w702, "Traction reciepe.Ball Load (N)"=w701, "Traction reciepe.Lubricant Name"=w700, "Traction reciepe.Profile File Name"=w699, "Traction reciepe.SET entrainment Velocity"=w697, "Traction reciepe.Test Array Size"=w696, "Traction reciepe.SRR INDEX [ STRIBECK]"=w695, "Traction reciepe.Stribeck Size"=w694, "Traction reciepe.SET SRR"=w693, "Traction reciepe.ELAPSED TIMER"=w692, "Traction reciepe.BALL SET RPM"=w691, "Traction reciepe.DISC SET RPM"=w690, "Traction reciepe.SET LOAD"=w689, "Traction reciepe.TEMPERATURE READ"=w688, "Traction reciepe.SET TEMPERATURE"=w687, "Traction reciepe.Traction Size"=w686, "Traction reciepe.DISC SPEED (rpm)"=w685, "Traction reciepe.BALL SPEED (rpm)"=w684, "Traction reciepe.BALL WEAR TRACK"=w683, "Traction reciepe.DISC WEARTRACK"=w682, "Traction reciepe.SRR INDEX [ TRACTION]"=w681, "Traction reciepe.Start Index Type"=w680, "Traction reciepe.Enum - Menu"=w679, "Traction reciepe.Ball (mm/sec)"=w678, "Traction reciepe.Disc (mm/sec)"=w677) -> (w711:T20)
    }
    frame #18 {
      n630 = control-ref of="SPEED SELECTION : MTM"() -> (w741:refnum<vi>)
      n631 = control-ref of="TEST SELECTION (MTM)"() -> (w740:refnum<vi>)
      n632 = control-ref of="MTM Test Selection"() -> (w739:refnum<vi>)
      n633 = control-ref of="TEST SELECTION (MTM) 2"() -> (w727:refnum<vi>)
      n634 = control-ref of="SPEED SELECTION : MTM 2"() -> (w726:refnum<vi>)
      n635 = control-ref of="MTM Test Selection 2"() -> (w725:refnum<vi>)
      n636 = control-ref of="Demo Mode Display"() -> (w769:refnum<vi>)
      n637 = control-ref of="Main Tab sequence for selection"() -> (w766:refnum<vi>)
      n638 = control-ref of="Ramp Tab"() -> (w765:refnum<vi>)
      n639 = control-ref of="e.v/ssr"() -> (w764:refnum<vi>)
      n640 = control-ref of="File Path Tab"() -> (w738:refnum<vi>)
      n641 = control-ref of="Step Sequence Indication Tab"() -> (w733:refnum<vi>)
      n642 = control-ref of="Disc Speed Indicator"() -> (w714:refnum<vi>)
      n643 = control-ref of="HomeTraction"() -> (w770:refnum<vi>)
      n644 = control-ref of="Traction Step Update Details"() -> (w767:refnum<vi>)
      n645 = control-ref of="E.Velocity"() -> (w756:refnum<vi>)
      n646 = control-ref of="Ramp Up   Disc"() -> (w753:refnum<vi>)
      n647 = control-ref of="Ramp Up"() -> (w746:refnum<vi>)
      n648 = control-ref of="BallSpeed Exceed Indication"() -> (w743:refnum<vi>)
      n649 = control-ref of="Apply"() -> (w742:refnum<vi>)
      n650 = control-ref of="Save"() -> (w736:refnum<vi>)
      n651 = control-ref of="Import"() -> (w735:refnum<vi>)
      n652 = control-ref of="Calculate Step"() -> (w731:refnum<vi>)
      n653 = control-ref of="Enter Fixed E.Velocity"() -> (w763:refnum<vi>)
      n654 = control-ref of="Enter Final SRR"() -> (w762:refnum<vi>)
      n655 = control-ref of="Enter initial SRR"() -> (w761:refnum<vi>)
      n656 = control-ref of="Enter Fixed SRR"() -> (w760:refnum<vi>)
      n657 = control-ref of="Enter the Final E.Velocity (m/s)"() -> (w759:refnum<vi>)
      n658 = control-ref of="Enter initial E.Velocity (m/s)"() -> (w758:refnum<vi>)
      n659 = control-ref of="Ball WTD"() -> (w757:refnum<vi>)
      n660 = control-ref of="Enter the Final Velocity (m/s)"() -> (w755:refnum<vi>)
      n661 = control-ref of="Enter initial Velocity (m/s)"() -> (w754:refnum<vi>)
      n662 = control-ref of="Initial DiscSpeed (RPM)"() -> (w752:refnum<vi>)
      n663 = control-ref of="Final Speed (RPM)"() -> (w751:refnum<vi>)
      n664 = control-ref of="Final Speed (RPM) Ball"() -> (w750:refnum<vi>)
      n665 = control-ref of="Initial Speed (RPM) Ball"() -> (w749:refnum<vi>)
      n666 = control-ref of="Enter the Final Velocity (m/s) Ball"() -> (w748:refnum<vi>)
      n667 = control-ref of="Enter initial Velocity (m/s) Ball"() -> (w747:refnum<vi>)
      n668 = control-ref of="Enter the Speed (m/sec):"() -> (w724:refnum<vi>)
      n669 = control-ref of="Enter the Speed (m/sec):"() -> (w723:refnum<vi>)
      n670 = control-ref of="Enter the Speed (RPM):"() -> (w722:refnum<vi>)
      n671 = control-ref of="Enter the Speed (RPM):Ball"() -> (w719:refnum<vi>)
      n672 = control-ref of="Wear Track Diameter (mm)"() -> (w715:refnum<vi>)
      n673 = control-ref of="ExceedBallSpeed"() -> (w713:refnum<vi>)
      n674 = control-ref of="Traction Message"() -> (w768:refnum<vi>)
      n675 = control-ref of="ExceedBallSpeed step"() -> (w745:refnum<vi>)
      n676 = control-ref of="ExceedDiscSpeed"() -> (w744:refnum<vi>)
      n677 = control-ref of="File Path String"() -> (w737:refnum<vi>)
      n678 = control-ref of="Step Sequence Indication"() -> (w732:refnum<vi>)
      n679 = control-ref of="ExceedDiscSpeed  Cinstant Speed"() -> (w729:refnum<vi>)
      n680 = control-ref of="ExceedBallSpeed Constant"() -> (w728:refnum<vi>)
      n681 = control-ref of="Lower Spped"() -> (w721:refnum<vi>)
      n682 = control-ref of="Upper"() -> (w720:refnum<vi>)
      n683 = control-ref of="StepTable"() -> (w730:refnum<vi>)
      n684 = control-ref of="Disc Motion Direction:"() -> (w718:refnum<vi>)
      n685 = control-ref of="Ball Motion Direction :"() -> (w717:refnum<vi>)
      n686 = control-ref of="Motion Mode:"() -> (w716:refnum<vi>)
      n687 = control-ref of="File Path :"() -> (w734:refnum<vi>)
      n688 = Bundle By Name(cluster=w772, "Traction Control.HomeTraction"=w770, "Traction Control.Demo Mode Display"=w769, "Traction Control.Traction Message"=w768, "Traction Control.Traction Step Update Details"=w767, "Traction Control.Main Tab sequence for selection"=w766, "Traction Control.Ramp Tab"=w765, "Traction Control.e.v/ssr"=w764, "Traction Control.Enter Fixed E.Velocity"=w763, "Traction Control.Enter Final SRR"=w762, "Traction Control.Enter initial SRR"=w761, "Traction Control.Enter Fixed SRR"=w760, "Traction Control.Enter the Final E.Velocity (m/s)"=w759, "Traction Control.Enter initial E.Velocity (m/s)"=w758, "Traction Control.Ball WTD"=w757, "Traction Control.E.Velocity"=w756, "Traction Control.Enter the Final Velocity (m/s)"=w755, "Traction Control.Enter initial Velocity (m/s)"=w754, "Traction Control.Ramp Up   Disc"=w753, "Traction Control.Initial DiscSpeed (RPM)"=w752, "Traction Control.Final Speed (RPM) Ball"=w751, "Traction Control.Final Speed (RPM)"=w750, "Traction Control.Initial Speed (RPM) Ball"=w749, "Traction Control.Enter the Final Velocity (m/s) Ball"=w748, "Traction Control.Enter initial Velocity (m/s) Ball"=w747, "Traction Control.Ramp Up"=w746, "Traction Control.ExceedBallSpeed step"=w745, "Traction Control.ExceedDiscSpeed"=w744, "Traction Control.BallSpeed Exceed Indication"=w743, "Traction Control.Apply"=w742, "Traction Control.SPEED SELECTION : MTM"=w741, "Traction Control.TEST SELECTION (MTM)"=w740, "Traction Control.MTM Test Selection"=w739, "Traction Control.File Path Tab"=w738, "Traction Control.File Path String"=w737, "Traction Control.Save"=w736, "Traction Control.Import"=w735, "Traction Control.File Path :"=w734, "Traction Control.Step Sequence Indication Tab"=w733, "Traction Control.Step Sequence Indication"=w732, "Traction Control.Calculate Step"=w731, "Traction Control.StepTable"=w730, "Traction Control.ExceedDiscSpeed  Cinstant Speed"=w729, "Traction Control.ExceedBallSpeed Constant"=w728, "Traction Control.TEST SELECTION (MTM) 2"=w727, "Traction Control.SPEED SELECTION : MTM 3"=w726, "Traction Control.MTM Test Selection 2"=w725, "Traction Control.Enter the Speed (m/sec):"=w724, "Traction Control.Enter the Speed (m/sec):  2"=w723, "Traction Control.Enter the Speed (RPM):"=w722, "Traction Control.Lower Spped"=w721, "Traction Control.Upper"=w720, "Traction Control.Enter the Speed (RPM):Ball"=w719, "Traction Control.Disc Motion Direction:"=w718, "Traction Control.Ball Motion Direction :"=w717, "Traction Control.Motion Mode:"=w716, "Traction Control.Wear Track Diameter (mm)"=w715, "Traction Control.Disc Speed Indicator"=w714, "Traction Control.ExceedBallSpeed"=w713) -> (w771:T20)
    }
    frame #19 {
      n689 = control-ref of="Gains"() -> (w775:refnum<vi>)
      n690 = control-ref of="Acoustic Graphs"() -> (w773:refnum<vi>)
      n691 = control-ref of="Manual Write Acquostic"() -> (w774:refnum<vi>)
      n692 = control-ref of="error out 2"() -> (w780:refnum<vi>)
      n693 = control-ref of="error in (no error)"() -> (w779:refnum<vi>)
      n694 = control-ref of="Downlink Packet"() -> (w778:refnum<vi>)
      n695 = control-ref of="Uplink Packet"() -> (w777:refnum<vi>)
      n696 = control-ref of="Last Config Rejected"() -> (w785:refnum<vi>)
      n697 = control-ref of="rx command count"() -> (w784:refnum<vi>)
      n698 = control-ref of="Current Filter Id"() -> (w783:refnum<vi>)
      n699 = control-ref of="Isolated Gain"() -> (w782:refnum<vi>)
      n700 = control-ref of="DAQ Status"() -> (w781:refnum<vi>)
      n701 = control-ref of="data out"() -> (w776:refnum<vi>)
      n702 = Bundle By Name(cluster=w787, "Acquostic.Last Config Rejected"=w785, "Acquostic.rx command count"=w784, "Acquostic.Current Filter Id"=w783, "Acquostic.Isolated Gain"=w782, "Acquostic.DAQ Status"=w781, "Acquostic.error out"=w780, "Acquostic.error in (no error)"=w779, "Acquostic.Downlink Packet"=w778, "Acquostic.Uplink Packet"=w777, "Acquostic.data out"=w776, "Acquostic.Acoustic Graphs"=w773, "Acquostic.Gains"=w775, "Acquostic.Manual Write Acquostic"=w774) -> (w786:T20)
    }
  }
  n703 = call <userlib>:"Fit VI window to Largest Dec.vi"() -> ("error out"=w43:errorcluster, "dup VI Ref"=w40:refnum<vi>)  [unwired: 6 in]
  n704 = invoke on="Invoke Node" class="VI" method="FP.Run-Time Position.Maximized"(reference=w40, error in=w43) -> (error out=w42:errorcluster)  [unwired: 2 in, 3 out]
  n705 = call <vilib>:"Clear Errors.vi"("error in (no error)"=w42) -> ("error out"=w41:errorcluster)  [unwired: 5 in, 1 out]
  n706 = control-ref of="This VI"() -> (w46:refnum<vi>)
  n707 = invoke on="Invoke Node" class="VI" method="Default Vals.Reinit All"(reference=w46, error in=w41) -> (reference out=w44:refnum<vi>, error out=w45:errorcluster)  [unwired: 1 in, 1 out]
  n708 = Close Reference(reference=w44, error in (no error)=w45) -> (error out=w39:errorcluster)
  n709 = call "Create User Event - Stop.vi"("error in (no error)"=w39) -> ("error out"=w2:errorcluster, "User Event - Stop"=w6:refnum<user-event>)  [unwired: 9 in]
  n710 = call "main screen queue out Unitest.vi"("error in (no error)"=w2) -> ("error out"=w66:errorcluster, "output Queue"=w4:T21)  [unwired: 9 in]
  n711 = Unbundle By Name(w4) -> ("RAMP MOTOR COM LOOP"=w32:refnum<queue>)
  n712 = Unbundle By Name(w4) -> ("TEMPERATURE COM LOOP"=w34:refnum<queue>)
  n713 = Unbundle By Name(w4) -> ("ECR PORT"=w31:refnum<queue>)
  n714 = Unbundle By Name(w4) -> ("SWAY MOTOR COM LOOP"=w36:refnum<queue>)
  n715 = Unbundle By Name(w4) -> ("UI Loop"=w64:refnum<queue>)
  n716 = Unbundle By Name(w4) -> ("LOAD COM LOOP"=w37:refnum<queue>)
  n717 = Unbundle By Name(w4) -> ("HEAVE MOTOR COM LOOP"=w22:refnum<queue>)
  n718 = Unbundle By Name(w4) -> ("HUMIDITY COM PORT"=w30:refnum<queue>)
  n719 = Unbundle By Name(w4) -> ("PROGRAM LOOP"=w29:refnum<queue>)
  n720 = Unbundle By Name(w4) -> ("MONITOR LOOP"=w28:refnum<queue>)
  n721 = Unbundle By Name(w4) -> ("LOAD PID"=w27:refnum<queue>)
  n722 = register-events(w6) -> (reference out=w58:refnum<event-registration>, error out=w56:errorcluster)  [unwired: 2 in]
  n723 = Unbundle By Name(w4) -> ("ACOUSTIC"=w3:refnum<queue>)
  n724 = Merge Errors(w56, w66) -> (w57:errorcluster)
  n725 = disable-structure shown="Enabled" {
    disable-tunnel: w32 -> [w792 _]
    disable-tunnel: [w791 w899] -> w16
    disable-tunnel: w6 -> [w790 _]
    disable-tunnel: w5 -> [w789 _]
    disable-tunnel: w2 -> [w788 w899]
    frame Disabled {
      n726 = node-c288() -> (w794:T22)  [unwired: 4 in]
      n727 = timed-loop {
        shift-right: [w796] -> _
        shift-left: w789 -> [w815]
        tunnel: [w809] -> w791
        tunnel: w792 -> [w807]
        tunnel: w788 -> [w806]
        tunnel: w790 -> [w805]
        timing: w794 -> [_]
        timing-out: [_] -> w793
        stop <- w814 stop-if-true
        # "Ramp Motor  Handling Loop"
        n728 = node-c288() -> ()  [unwired: 1 in, 1 out]
        n729 = call "Dequeue Message.vi"("error in (no error)"=w806, "Message Queue"=w807) -> ("error out"=w813:errorcluster, "Message Data"=w811:variant, "Message"=w812:string, "dup Message Queue"=w810:refnum<queue>)  [unwired: 6 in]
        n730 = case "Message Cases" shown="\"Ramp Main\"" w812 {
          selector: w812 -> [_ _ _ _ _ w887]
          tunnel: w810 -> [w831 w847 _ w874 w886 _]
          tunnel: w813 -> [w833 w845 w871 w878 w880 _]
          tunnel: [w834 w848 w865 w876 w882 w888] -> w808
          tunnel: w815 -> [w822 w836 w870 w877 w885 w889]
          tunnel: [w822 w836 w870 w877 w885 w889] -> w796
          tunnel: [_ _ _ _ TRUE _] -> w814
          tunnel: w811 -> [_ _ w869 _ _ _]
          tunnel: w805 -> [_ _ _ _ w879 _]
          frame "init" {
            # "Initialize - All initialization work should take place in this message, since other loops can potentially enqueue messages that execute immediately after this one."
            n731 = call "TRACTION WRITE FGV.vi"("Enum - Menu"=Traction_Write_enum."INIT", "error in (no error)"=w833, "main ref"=w822) -> ("error out"=w830:errorcluster)  [unwired: 8 in]
            n732 = call <vilib>:"Clear Errors.vi"("error in (no error)"=w830) -> ("error out"=w828:errorcluster)  [unwired: 5 in, 1 out]
            n733 = call "Stall Data Flow.vim"("value in"=w828, "milliseconds to wait"=u32 1000) -> ("value out"=w827:errorcluster)  [unwired: 1 out]
            n734 = call "Traction  Init.vi"("error in (no error)"=w827, "main ref"=w822) -> ("error out"=w825:errorcluster)  [unwired: 9 in]
            n735 = call <vilib>:"Clear Errors.vi"("error in (no error)"=w825) -> ("error out"=w824:errorcluster)  [unwired: 5 in, 1 out]
            n736 = call "TRACTION READ FGV.vi"("Enum - Menu"=Traction_Read_enum."INIT", "error in (no error)"=w824, "main ref"=w822) -> ("error out"=w823:errorcluster)  [unwired: 7 in, 1 out]
            n737 = call <vilib>:"Clear Errors.vi"("error in (no error)"=w823) -> ("error out"=w821:errorcluster)  [unwired: 5 in, 1 out]
            n738 = call-poly "Enqueue Message.vi"("error in (no error)"=w821, "Message"="Ramp Main", "Message Queue"=w831) -> ("error out"=w834:errorcluster)  [unwired: 7 in, 1 out]
          }
          frame "Ramp Main" {
            n739 = Unbundle By Name(w836) -> ("Traction.Read TRACTION Temp"=w841:refnum<vi>)
            n740 = property on="Property Node" class="Bool (strict)"(reference=w841) -> (reference out=w839:refnum<vi>, error out=w840:errorcluster, "Value"=w837:bool)  [unwired: 1 in]
            n741 = Close Reference(reference=w839, error in (no error)=w840) -> ()  [unwired: 1 out]
            n742 = case shown="True" w837 {
              tunnel: w845 -> [w849 w856]
              tunnel: [w849 w853] -> w838
              tunnel: w836 -> [_ w854]
              tunnel: w836 -> [_ w852]
              frame False {
              }
              frame True {
                n743 = call "TRACTION READ FGV.vi"("Enum - Menu"=Traction_Read_enum."READ", "error in (no error)"=w856, "main ref"=w854) -> ("error out"=w855:errorcluster, "ERROR TEMP"=w851:bool)  [unwired: 7 in]
                n744 = call "Traction Reinitize.vi"("error in (no error)"=w855, "Checkbox"=w851, "Data Cluster"=w852) -> ("error out"=w853:errorcluster)  [unwired: 8 in]
              }
            }
            n745 = Unbundle By Name(w836) -> ("Main Home Screen.EXIT"=w846:refnum<vi>)
            n746 = call <vilib>:"Clear Errors.vi"("error in (no error)"=w838) -> ("error out"=w835:errorcluster)  [unwired: 5 in, 1 out]
            n747 = property on="Property Node" class="Bool (strict)"(reference=w846) -> (reference out=w843:refnum<vi>, error out=w844:errorcluster, "Value"=w842:bool)  [unwired: 1 in]
            n748 = case shown="False" w842 {
              tunnel: [w859 w863] -> w848
              tunnel: w847 -> [w858 w862]
              tunnel: w835 -> [w857 w861]
              frame True {
                n749 = call-poly "Enqueue Message.vi"("error in (no error)"=w857, "Message"="Confirm Quit", "Message Queue"=w858) -> ("error out"=w859:errorcluster)  [unwired: 7 in, 1 out]
              }
              frame False {
                n750 = call-poly "Enqueue Message.vi"("error in (no error)"=w861, "Message"="Ramp Main", "Message Queue"=w862) -> ("error out"=w863:errorcluster)  [unwired: 7 in, 1 out]
              }
            }
            n751 = Close Reference(reference=w843, error in (no error)=w844) -> ()  [unwired: 1 out]
          }
          frame "Error" {
            # "#CodeRecommended - If you ever change the name of this \"Error\" message, you'll need to update the name in the Check Loop Error.vi as well."
            # "#CodeRecommended - Consider creating a system for logging errors in some way. These errors are for notification purposes only. Handling of specific errors should be performed in the message frames that generated the error."
            # "Error - Display an error dialog. This message is sent by the \"Error Handler\" VIs at the end of other loops in this application."
            n752 = Variant To Data(error in=w871, type=errorcluster {"status"=FALSE, "code"=0, "source"=""} ("error constant"), Variant=w869) -> (data=w867:errorcluster, error out=w866:errorcluster)
            n753 = call <vilib>:"Simple Error Handler.vi"("error in (no error)"=w867) -> ()  [unwired: 4 in, 5 out]
            n754 = Merge Errors(w866) -> (w865:errorcluster)
          }
          frame "Confirm Quit" {
            # "#CodeNeeded - If you want to provide an \"Are you sure\" dialog (or some other notification) before the application exits, place that code here. This message is typically sent from a Panel Close? event."
            # "Confirm Quit - Message that can confirm whether or not the user wants to exit the application."
            n755 = call-poly "Enqueue Message.vi"("Priority Message? (F)"=TRUE, "error in (no error)"=w878, "Message"="Exit", "Message Queue"=w874) -> ("error out"=w875:errorcluster)  [unwired: 6 in, 1 out]
            n756 = Merge Errors(w875) -> (w876:errorcluster)
          }
          frame "Exit" {
            # "Stop the VI"
            # "Release the message queue reference"
            # "#CodeNeeded - Add any required cleanup code here. Note that if 'Exit' was called as a result of an error, an error dialog will be displayed. Add any custom error handling for an 'Exit' condition here as well."
            # "Exit - Exit the application."
            n757 = call "Fire User Event - Stop.vi"("User Event - Stop"=w879) -> ("error out"=w881:errorcluster)  [unwired: 10 in]
            n758 = Release Queue(queue=w886, error in (no error)=w880) -> (error out=w883:errorcluster)  [unwired: 1 in, 2 out]
            n759 = Merge Errors(w881, w883) -> (w882:errorcluster)
          }
          frame Default {
            # "'Default' case only runs if there is a message that isn't defined in any of the other cases.  Output a programming error."
            n760 = xnode ("Error Ring")("parameter 0"=w887) -> ("error out"=w888:errorcluster)
          }
        }
        n761 = call "LAB-IQ Error Handler - Message Handling Loop.vi"("error in (no error)"=w808, "Message Queue"=w810) -> ("dup error in"=w809:errorcluster)  [unwired: 8 in, 1 out]
        n762 = Unbundle By Name(w796) -> ("Motion Module.Traction"=w804:refnum<vi>)
        n763 = property on="Property Node" class="Bool (strict)"(reference=w804) -> (reference out=w802:refnum<vi>, error out=w803:errorcluster, "Value"=w801:bool)  [unwired: 1 in]
        n764 = Close Reference(reference=w802, error in (no error)=w803) -> ()  [unwired: 1 out]
        n765 = Equal?(x=w801, y=TRUE) -> (x = y?=w799:bool)
        n766 = Select(t=i64 10 ("Period"), s=w799, f=i64 1000) -> (s? t:f=w795:i64)
        n767 = node-c288(w795) -> ()  [unwired: 1 in, 1 out]
      }
      n768 = node-c288(w793) -> ()  [unwired: 1 out]
    }
    frame Enabled {
      # "E"
      # "ENABLE WHEN RUNNING IN TRACTION TEST CONDITION"
    }
  }
  n769 = while {
    shift-right: [w901] -> _
    shift-left: w5 -> [w912]
    tunnel: [w906] -> w1
    tunnel: w3 -> [w904]
    tunnel: w2 -> [w903]
    tunnel: w6 -> [w902]
    stop <- w911 stop-if-true
    # "Acqoustic  Handling Loop"
    n770 = call "Dequeue Message.vi"("error in (no error)"=w903, "Message Queue"=w904) -> ("error out"=w910:errorcluster, "Message Data"=w908:variant, "Message"=w909:string, "dup Message Queue"=w907:refnum<queue>)  [unwired: 6 in]
    n771 = case "Message Cases" shown="\"Acoustic Main\"" w909 {
      selector: w909 -> [_ _ _ _ _ w997]
      tunnel: w907 -> [w924 w945 _ w982 w995 _]
      tunnel: w910 -> [w918 w936 w978 w986 w989 _]
      tunnel: [w926 w946 w972 w984 w991 w998] -> w905
      tunnel: w912 -> [w915 w931 w977 w985 w994 w999]
      tunnel: [w915 w931 w977 w985 w994 w999] -> w901
      tunnel: [_ _ _ _ TRUE _] -> w911
      tunnel: w908 -> [_ _ w976 _ _ _]
      tunnel: w902 -> [_ _ _ _ w988 _]
      tunnel: [i64 1000 ("Period") w927 i64 1000 ("Period") i64 1000 ("Period") i64 1000 ("Period") i64 1000 ("Period")] -> w900
      frame "init" {
        (unwired) dbl[] [] ("0UTPUT")
        # "Initialize - All initialization work should take place in this message, since other loops can potentially enqueue messages that execute immediately after this one."
        n772 = call "Acq Write Loop.vi"("Enum - Menu"=Write_Main_Enum."INIT", "error in (no error)"=w918, "main ref"=w915) -> ("error out"=w923:errorcluster)  [unwired: 8 in]
        n773 = call <vilib>:"Clear Errors.vi"("error in (no error)"=w923) -> ("error out"=w922:errorcluster)  [unwired: 5 in, 1 out]
        n774 = call "Stall Data Flow.vim"("value in"=w922, "milliseconds to wait"=u32 1000) -> ("value out"=w921:errorcluster)  [unwired: 1 out]
        n775 = call "Acq Read Loop.vi"("Enum - Menu"=Read_Main_Enum."INIT", "error in (no error)"=w921, "main ref"=w915) -> ("error out"=w919:errorcluster)  [unwired: 7 in, 1 out]
        n776 = call <vilib>:"Clear Errors.vi"("error in (no error)"=w919) -> ("error out"=w917:errorcluster)  [unwired: 5 in, 1 out]
        n777 = call-poly "Enqueue Message.vi"("error in (no error)"=w917, "Message"="Acoustic Main", "Message Queue"=w924) -> ("error out"=w926:errorcluster)  [unwired: 7 in, 1 out]
      }
      frame "Acoustic Main" {
        (unwired) TRUE
        n778 = Unbundle By Name(w931) -> ("Environmental control.Acoustic Emission 3"=w940:refnum<vi>)
        n779 = Unbundle By Name(w931) -> ("Main Screen.Start Test Temp"=w932:refnum<vi>)
        n780 = property class="Bool (strict)"(reference=w932) -> (reference out=w930:refnum<vi>, error out=w933:errorcluster, "Value"=w928:bool)  [unwired: 1 in]
        n781 = property on="Property Node" class="Bool (strict)"(reference=w940) -> (reference out=w938:refnum<vi>, error out=w939:errorcluster, "Value"=w937:bool)  [unwired: 1 in]
        n782 = Close Reference(reference=w930, error in (no error)=w933) -> ()  [unwired: 1 out]
        n783 = Close Reference(reference=w938, error in (no error)=w939) -> ()  [unwired: 1 out]
        n784 = And(x=w937, y=w928) -> (x .and. y?=w929:bool)
        n785 = case shown="True" w929 {
          tunnel: w936 -> [w948 w957]
          tunnel: w931 -> [_ w952]
          tunnel: [w948 w950] -> w935
          tunnel: [i64 1000 ("Period") i64 2 ("Period")] -> w927
          frame False {
          }
          frame True {
            n786 = call "Acq Read Loop.vi"("Enum - Menu"=Read_Main_Enum."READ", "error in (no error)"=w957, "main ref"=w952) -> ("error out"=w955:errorcluster, "ERROR TEMP"=w954:bool)  [unwired: 7 in]
            n787 = call <vilib>:"Clear Errors.vi"("error in (no error)"=w955) -> ("error out"=w951:errorcluster)  [unwired: 5 in, 1 out]
            n788 = disable-structure shown="Disabled" {
              disable-tunnel: w954 -> [w961 _]
              disable-tunnel: [w960 w962] -> w953
              disable-tunnel: w952 -> [w959 _]
              disable-tunnel: w951 -> [w958 w962]
              frame Disabled {
                n789 = call "Acoustic Reinitize.vi"("error in (no error)"=w958, "Checkbox"=w961, "Data Cluster"=w959) -> ("error out"=w960:errorcluster)  [unwired: 8 in]
              }
              frame Enabled {
              }
            }
            n790 = call <vilib>:"Clear Errors.vi"("error in (no error)"=w953) -> ("error out"=w950:errorcluster)  [unwired: 5 in, 1 out]
          }
        }
        n791 = Unbundle By Name(w931) -> ("Main Home Screen.EXIT"=w944:refnum<vi>)
        n792 = property on="Property Node" class="Bool (strict)"(reference=w944) -> (reference out=w942:refnum<vi>, error out=w943:errorcluster, "Value"=w941:bool)  [unwired: 1 in]
        n793 = call <vilib>:"Clear Errors.vi"("error in (no error)"=w935) -> ("error out"=w934:errorcluster)  [unwired: 5 in, 1 out]
        n794 = Close Reference(reference=w942, error in (no error)=w943) -> ()  [unwired: 1 out]
        n795 = case shown="False" w941 {
          tunnel: [w965 w969] -> w946
          tunnel: w945 -> [w964 w968]
          tunnel: w934 -> [w963 w967]
          frame True {
            n796 = call-poly "Enqueue Message.vi"("error in (no error)"=w963, "Message"="Confirm Quit", "Message Queue"=w964) -> ("error out"=w965:errorcluster)  [unwired: 7 in, 1 out]
          }
          frame False {
            n797 = call-poly "Enqueue Message.vi"("error in (no error)"=w967, "Message"="Acoustic Main", "Message Queue"=w968) -> ("error out"=w969:errorcluster)  [unwired: 7 in, 1 out]
          }
        }
      }
      frame "Error" {
        (unwired) dbl[] [] ("0UTPUT")
        # "#CodeRecommended - If you ever change the name of this \"Error\" message, you'll need to update the name in the Check Loop Error.vi as well."
        # "#CodeRecommended - Consider creating a system for logging errors in some way. These errors are for notification purposes only. Handling of specific errors should be performed in the message frames that generated the error."
        # "Error - Display an error dialog. This message is sent by the \"Error Handler\" VIs at the end of other loops in this application."
        n798 = Variant To Data(error in=w978, type=errorcluster {"status"=FALSE, "code"=0, "source"=""} ("error constant"), Variant=w976) -> (data=w974:errorcluster, error out=w973:errorcluster)
        n799 = call <vilib>:"Simple Error Handler.vi"("error in (no error)"=w974) -> ()  [unwired: 4 in, 5 out]
        n800 = Merge Errors(w973) -> (w972:errorcluster)
      }
      frame "Confirm Quit" {
        (unwired) dbl[] [] ("0UTPUT")
        # "#CodeNeeded - If you want to provide an \"Are you sure\" dialog (or some other notification) before the application exits, place that code here. This message is typically sent from a Panel Close? event."
        # "Confirm Quit - Message that can confirm whether or not the user wants to exit the application."
        n801 = call-poly "Enqueue Message.vi"("Priority Message? (F)"=TRUE, "error in (no error)"=w986, "Message"="Exit", "Message Queue"=w982) -> ("error out"=w983:errorcluster)  [unwired: 6 in, 1 out]
        n802 = Merge Errors(w983) -> (w984:errorcluster)
      }
      frame "Exit" {
        (unwired) dbl[] [] ("0UTPUT")
        # "Stop the VI"
        # "Release the message queue reference"
        # "#CodeNeeded - Add any required cleanup code here. Note that if 'Exit' was called as a result of an error, an error dialog will be displayed. Add any custom error handling for an 'Exit' condition here as well."
        # "Exit - Exit the application."
        n803 = call "Fire User Event - Stop.vi"("User Event - Stop"=w988) -> ("error out"=w990:errorcluster)  [unwired: 10 in]
        n804 = Release Queue(queue=w995, error in (no error)=w989) -> (error out=w992:errorcluster)  [unwired: 1 in, 2 out]
        n805 = Merge Errors(w990, w992) -> (w991:errorcluster)
      }
      frame Default {
        # "'Default' case only runs if there is a message that isn't defined in any of the other cases.  Output a programming error."
        n806 = xnode ("Error Ring")("parameter 0"=w997) -> ("error out"=w998:errorcluster)
      }
    }
    n807 = call "LAB-IQ Error Handler - Message Handling Loop.vi"("error in (no error)"=w905, "Message Queue"=w907) -> ("dup error in"=w906:errorcluster)  [unwired: 8 in, 1 out]
    n808 = Wait (ms)(milliseconds to wait=w900) -> ()  [unwired: 1 out]
  }
  n809 = while {
    tunnel: w64 -> [w1014]
    shift-right: [w1012] -> w61
    shift-left: w58 -> [w1013]
    tunnel: [w1008] -> w59
    stop <- w1010 stop-if-true
    # "Event Handling Loop"
    n810 = event shown="[68] \"Refresh 2\": Value Change" {
      selector: w1013 -> [_ _ _ _ _ _ _ _ _ _ _ _ _ _ _ _ _ _ _ _ _ _ _ _ _ _ _ _ _ _ _ _ _ _ _ _ _ _ _ _ _ _ _ _ _ _ _ _ _ _ _ _ _ _ _ _ _ _ _ _ _ _ _ _ _ _ _ _ _ _ _ _ _ _ _ _ _ _ _ _ _]
      dyn-events: [_ _ _ _ _ _ _ _ _ _ _ _ _ _ _ _ _ _ _ _ _ _ _ _ _ _ _ _ _ _ _ _ _ _ _ _ _ _ _ _ _ _ _ _ _ _ _ _ _ _ _ _ _ _ _ _ _ _ _ _ _ _ _ _ _ _ _ _ _ _ _ _ _ _ _ _ _ _ _ _ _] -> w1012
      timeout: 100 -> [_ _ _ _ _ _ _ _ _ _ _ _ _ _ _ _ _ _ _ _ _ _ _ _ _ _ _ _ _ _ _ _ _ _ _ _ _ _ _ _ _ _ _ _ _ _ _ _ _ _ _ _ _ _ _ _ _ _ _ _ _ _ _ _ _ _ _ _ _ _ _ _ _ _ _ _ _ _ _ _ _]
      tunnel: [_ _ _ _ _ _ _ _ _ _ _ _ _ _ _ _ _ _ _ _ _ _ _ _ _ _ _ _ _ _ _ _ _ _ _ _ _ _ _ _ _ _ _ _ _ _ _ _ _ _ _ _ _ _ _ _ _ _ _ _ _ _ _ _ _ _ _ _ _ _ _ _ _ _ _ _ _ _ _ _ TRUE ("Discard?")] -> w1010
      tunnel: w1014 -> [w1019 w1025 w1028 w1033 w1038 w1043 w1048 w1053 w1058 w1063 w1068 w1073 w1078 w1083 w1088 w1093 w1098 w1103 w1108 w1113 w1118 w1123 w1128 w1133 w1138 w1143 w1148 w1153 w1158 w1163 w1168 w1173 w1178 w1183 w1188 w1193 w1198 w1203 w1208 w1213 w1218 w1223 w1228 w1233 w1238 w1243 w1248 w1253 w1258 w1263 w1268 w1273 w1278 w1283 w1288 w1293 w1298 w1303 w1308 w1313 w1318 w1323 w1328 w1333 w1338 w1343 w1348 w1353 w1358 w1363 w1368 w1373 w1378 w1383 w1388 w1393 w1398 w1403 w1406 w1411 w1413]
      tunnel: [w1018 w1024 w1026 w1031 w1036 w1041 w1046 w1051 w1056 w1061 w1066 w1071 w1076 w1081 w1086 w1091 w1096 w1101 w1106 w1111 w1116 w1121 w1126 w1131 w1136 w1141 w1146 w1151 w1156 w1161 w1166 w1171 w1176 w1181 w1186 w1191 w1196 w1201 w1206 w1211 w1216 w1221 w1226 w1231 w1236 w1241 w1246 w1251 w1256 w1261 w1266 w1271 w1276 w1281 w1286 w1291 w1296 w1301 w1306 w1311 w1316 w1321 w1326 w1331 w1336 w1341 w1346 w1351 w1356 w1361 w1366 w1371 w1376 w1381 w1386 w1391 w1396 w1401 _ w1410 _] -> w1011
      tunnel: [w1017 w1023 w1027 w1032 w1037 w1042 w1047 w1052 w1057 w1062 w1067 w1072 w1077 w1082 w1087 w1092 w1097 w1102 w1107 w1112 w1117 w1122 w1127 w1132 w1137 w1142 w1147 w1152 w1157 w1162 w1167 w1172 w1177 w1182 w1187 w1192 w1197 w1202 w1207 w1212 w1217 w1222 w1227 w1232 w1237 w1242 w1247 w1252 w1257 w1262 w1267 w1272 w1277 w1282 w1287 w1292 w1297 w1302 w1307 w1312 w1317 w1322 w1327 w1332 w1337 w1342 w1347 w1352 w1357 w1362 w1367 w1372 w1377 w1382 w1387 w1392 w1397 w1402 w1406 w1409 w1413] -> w1009
      event Panel Close? {
        n811 = event-data() -> ()  [unwired: 1 in, 1 out]
        n812 = call-poly "Enqueue Message.vi"("Priority Message? (F)"=TRUE, "Message"="Confirm Quit", "Message Queue"=w1019) -> ("error out"=w1018:errorcluster, "dup Message Queue"=w1017:refnum<queue>)  [unwired: 7 in]
        n813 = event-data ("Event Filter Node")("Discard?"=TRUE) -> ()  [unwired: 1 in, 1 out]
      }
      event Timeout {
        n814 = event-data() -> ()  [unwired: 1 in, 1 out]
        n815 = call-poly "Enqueue Message.vi"("Priority Message? (F)"=TRUE, "Message"="Timeout", "Message Queue"=w1025) -> ("error out"=w1024:errorcluster, "dup Message Queue"=w1023:refnum<queue>)  [unwired: 7 in]
      }
      event "SAVE  2": Value Change {
        n816 = event-data() -> ()  [unwired: 1 in, 1 out]
        n817 = call-poly "Enqueue Message.vi"("Priority Message? (F)"=TRUE, "Message"="Service Save", "Message Queue"=w1028) -> ("error out"=w1026:errorcluster, "dup Message Queue"=w1027:refnum<queue>)  [unwired: 7 in]
      }
      event "Home": Value Change {
        n818 = event-data() -> ()  [unwired: 1 in, 1 out]
        n819 = call-poly "Enqueue Message.vi"("Priority Message? (F)"=TRUE, "Message"="HOME", "Message Queue"=w1033) -> ("error out"=w1031:errorcluster, "dup Message Queue"=w1032:refnum<queue>)  [unwired: 7 in]
      }
      event "Platform Settings": Value Change {
        n820 = event-data() -> ()  [unwired: 1 in, 1 out]
        n821 = call-poly "Enqueue Message.vi"("Priority Message? (F)"=TRUE, "Message"="Platform Setting", "Message Queue"=w1038) -> ("error out"=w1036:errorcluster, "dup Message Queue"=w1037:refnum<queue>)  [unwired: 7 in]
      }
      event "Configure": Value Change {
        n822 = event-data() -> ()  [unwired: 1 in, 1 out]
        n823 = call-poly "Enqueue Message.vi"("Priority Message? (F)"=TRUE, "Message"="Configure", "Message Queue"=w1043) -> ("error out"=w1041:errorcluster, "dup Message Queue"=w1042:refnum<queue>)  [unwired: 7 in]
      }
      event "Analysis": Value Change {
        n824 = event-data() -> ()  [unwired: 1 in, 1 out]
        n825 = call-poly "Enqueue Message.vi"("Priority Message? (F)"=TRUE, "Message"="Analysis", "Message Queue"=w1048) -> ("error out"=w1046:errorcluster, "dup Message Queue"=w1047:refnum<queue>)  [unwired: 7 in]
      }
      event "service 2": Value Change {
        n826 = event-data() -> ()  [unwired: 1 in, 1 out]
        n827 = call-poly "Enqueue Message.vi"("Priority Message? (F)"=TRUE, "Message"="service 2", "Message Queue"=w1053) -> ("error out"=w1051:errorcluster, "dup Message Queue"=w1052:refnum<queue>)  [unwired: 7 in]
      }
      event "Auto": Value Change {
        n828 = event-data() -> ()  [unwired: 1 in, 1 out]
        n829 = call-poly "Enqueue Message.vi"("Priority Message? (F)"=TRUE, "Message"="Auto", "Message Queue"=w1058) -> ("error out"=w1056:errorcluster, "dup Message Queue"=w1057:refnum<queue>)  [unwired: 7 in]
      }
      event "Select Load Head": Value Change {
        n830 = event-data() -> ()  [unwired: 1 in, 1 out]
        n831 = call-poly "Enqueue Message.vi"("Priority Message? (F)"=TRUE, "Message"="Select Load Head", "Message Queue"=w1063) -> ("error out"=w1061:errorcluster, "dup Message Queue"=w1062:refnum<queue>)  [unwired: 7 in]
      }
      event "com 3": Value Change {
        n832 = event-data() -> ()  [unwired: 1 in, 1 out]
        n833 = call-poly "Enqueue Message.vi"("Priority Message? (F)"=TRUE, "Message"="com 3", "Message Queue"=w1068) -> ("error out"=w1066:errorcluster, "dup Message Queue"=w1067:refnum<queue>)  [unwired: 7 in]
      }
      event "Loading Mode": Value Change {
        n834 = event-data() -> ()  [unwired: 1 in, 1 out]
        n835 = call-poly "Enqueue Message.vi"("Priority Message? (F)"=TRUE, "Message"="Loading Mode", "Message Queue"=w1073) -> ("error out"=w1071:errorcluster, "dup Message Queue"=w1072:refnum<queue>)  [unwired: 7 in]
      }
      event "SSP 0.3": Value Change {
        n836 = event-data() -> ()  [unwired: 1 in, 1 out]
        n837 = call-poly "Enqueue Message.vi"("Priority Message? (F)"=TRUE, "Message"="SSP 0.3", "Message Queue"=w1078) -> ("error out"=w1076:errorcluster, "dup Message Queue"=w1077:refnum<queue>)  [unwired: 7 in]
      }
      event "SSP 0.5": Value Change {
        n838 = event-data() -> ()  [unwired: 1 in, 1 out]
        n839 = call-poly "Enqueue Message.vi"("Priority Message? (F)"=TRUE, "Message"="SSP 0.5", "Message Queue"=w1083) -> ("error out"=w1081:errorcluster, "dup Message Queue"=w1082:refnum<queue>)  [unwired: 7 in]
      }
      event "SSP 0.75": Value Change {
        n840 = event-data() -> ()  [unwired: 1 in, 1 out]
        n841 = call-poly "Enqueue Message.vi"("Priority Message? (F)"=TRUE, "Message"="SSP 0.75", "Message Queue"=w1088) -> ("error out"=w1086:errorcluster, "dup Message Queue"=w1087:refnum<queue>)  [unwired: 7 in]
      }
      event "LHBack": Value Change {
        n842 = event-data() -> ()  [unwired: 1 in, 1 out]
        n843 = call-poly "Enqueue Message.vi"("Priority Message? (F)"=TRUE, "Message"="LHBack", "Message Queue"=w1093) -> ("error out"=w1091:errorcluster, "dup Message Queue"=w1092:refnum<queue>)  [unwired: 7 in]
      }
      event "LHNext": Value Change {
        n844 = event-data() -> ()  [unwired: 1 in, 1 out]
        n845 = call-poly "Enqueue Message.vi"("Priority Message? (F)"=TRUE, "Message"="LHNext", "Message Queue"=w1098) -> ("error out"=w1096:errorcluster, "dup Message Queue"=w1097:refnum<queue>)  [unwired: 7 in]
      }
      event "Rot Ver": Value Change {
        n846 = event-data() -> ()  [unwired: 1 in, 1 out]
        n847 = call-poly "Enqueue Message.vi"("Priority Message? (F)"=TRUE, "Message"="Rot Ver", "Message Queue"=w1103) -> ("error out"=w1101:errorcluster, "dup Message Queue"=w1102:refnum<queue>)  [unwired: 7 in]
      }
      event "Traction": Value Change {
        n848 = event-data() -> ()  [unwired: 1 in, 1 out]
        n849 = call-poly "Enqueue Message.vi"("Priority Message? (F)"=TRUE, "Message"="Traction", "Message Queue"=w1108) -> ("error out"=w1106:errorcluster, "dup Message Queue"=w1107:refnum<queue>)  [unwired: 7 in]
      }
      event "Scratch": Value Change {
        n850 = event-data() -> ()  [unwired: 1 in, 1 out]
        n851 = call-poly "Enqueue Message.vi"("Priority Message? (F)"=TRUE, "Message"="Scratch", "Message Queue"=w1113) -> ("error out"=w1111:errorcluster, "dup Message Queue"=w1112:refnum<queue>)  [unwired: 7 in]
      }
      event "Motion Mode:": Value Change {
        n852 = event-data() -> ()  [unwired: 1 in, 1 out]
        n853 = call-poly "Enqueue Message.vi"("Priority Message? (F)"=TRUE, "Message"="Motion Mode:", "Message Queue"=w1118) -> ("error out"=w1116:errorcluster, "dup Message Queue"=w1117:refnum<queue>)  [unwired: 7 in]
      }
      event "MMBack": Value Change {
        n854 = event-data() -> ()  [unwired: 1 in, 1 out]
        n855 = call-poly "Enqueue Message.vi"("Priority Message? (F)"=TRUE, "Message"="MMBack", "Message Queue"=w1123) -> ("error out"=w1121:errorcluster, "dup Message Queue"=w1122:refnum<queue>)  [unwired: 7 in]
      }
      event "MMNext": Value Change {
        n856 = event-data() -> ()  [unwired: 1 in, 1 out]
        n857 = call-poly "Enqueue Message.vi"("Priority Message? (F)"=TRUE, "Message"="MMNext", "Message Queue"=w1128) -> ("error out"=w1126:errorcluster, "dup Message Queue"=w1127:refnum<queue>)  [unwired: 7 in]
      }
      event "APBack": Value Change {
        n858 = event-data() -> ()  [unwired: 1 in, 1 out]
        n859 = call-poly "Enqueue Message.vi"("Priority Message? (F)"=TRUE, "Message"="APBack", "Message Queue"=w1133) -> ("error out"=w1131:errorcluster, "dup Message Queue"=w1132:refnum<queue>)  [unwired: 7 in]
      }
      event "SNext": Value Change {
        n860 = event-data() -> ()  [unwired: 1 in, 1 out]
        n861 = call-poly "Enqueue Message.vi"("Priority Message? (F)"=TRUE, "Message"="SNext", "Message Queue"=w1138) -> ("error out"=w1136:errorcluster, "dup Message Queue"=w1137:refnum<queue>)  [unwired: 7 in]
      }
      event "Load Cell Link.ZeroAll": Value Change {
        n862 = event-data() -> ()  [unwired: 1 in, 1 out]
        n863 = call-poly "Enqueue Message.vi"("Priority Message? (F)"=TRUE, "Message"="ZeroAll", "Message Queue"=w1143) -> ("error out"=w1141:errorcluster, "dup Message Queue"=w1142:refnum<queue>)  [unwired: 7 in]
      }
      event "Enable Platform": Value Change {
        n864 = event-data() -> ()  [unwired: 1 in, 1 out]
        n865 = call-poly "Enqueue Message.vi"("Priority Message? (F)"=TRUE, "Message"="Enable Platform", "Message Queue"=w1148) -> ("error out"=w1146:errorcluster, "dup Message Queue"=w1147:refnum<queue>)  [unwired: 7 in]
      }
      event "Heave Up main": Value Change {
        n866 = event-data() -> ()  [unwired: 1 in, 1 out]
        n867 = call-poly "Enqueue Message.vi"("Priority Message? (F)"=TRUE, "Message"="Heave Up main", "Message Queue"=w1153) -> ("error out"=w1151:errorcluster, "dup Message Queue"=w1152:refnum<queue>)  [unwired: 7 in]
      }
      event "Heave Up MM": Value Change {
        n868 = event-data() -> ()  [unwired: 1 in, 1 out]
        n869 = call-poly "Enqueue Message.vi"("Priority Message? (F)"=TRUE, "Message"="Heave Up MM", "Message Queue"=w1158) -> ("error out"=w1156:errorcluster, "dup Message Queue"=w1157:refnum<queue>)  [unwired: 7 in]
      }
      event "Heave Down Main": Value Change {
        n870 = event-data() -> ()  [unwired: 1 in, 1 out]
        n871 = call-poly "Enqueue Message.vi"("Priority Message? (F)"=TRUE, "Message"="Heave Down Main", "Message Queue"=w1163) -> ("error out"=w1161:errorcluster, "dup Message Queue"=w1162:refnum<queue>)  [unwired: 7 in]
      }
      event "Heave Down MM": Value Change {
        n872 = event-data() -> ()  [unwired: 1 in, 1 out]
        n873 = call-poly "Enqueue Message.vi"("Priority Message? (F)"=TRUE, "Message"="Heave Down MM", "Message Queue"=w1168) -> ("error out"=w1166:errorcluster, "dup Message Queue"=w1167:refnum<queue>)  [unwired: 7 in]
      }
      event "Manual Write Heave & Surge": Value Change {
        n874 = event-data() -> ()  [unwired: 1 in, 1 out]
        n875 = call-poly "Enqueue Message.vi"("Priority Message? (F)"=TRUE, "Message"="Manual Write Heave & Surge", "Message Queue"=w1173) -> ("error out"=w1171:errorcluster, "dup Message Queue"=w1172:refnum<queue>)  [unwired: 7 in]
      }
      event "Manual Write SWAY": Value Change {
        n876 = event-data() -> ()  [unwired: 1 in, 1 out]
        n877 = call-poly "Enqueue Message.vi"("Priority Message? (F)"=TRUE, "Message"="Manual Write SWAY", "Message Queue"=w1178) -> ("error out"=w1176:errorcluster, "dup Message Queue"=w1177:refnum<queue>)  [unwired: 7 in]
      }
      event "Surge Backward Main": Value Change {
        n878 = event-data() -> ()  [unwired: 1 in, 1 out]
        n879 = call-poly "Enqueue Message.vi"("Priority Message? (F)"=TRUE, "Message"="Surge Backward Main", "Message Queue"=w1183) -> ("error out"=w1181:errorcluster, "dup Message Queue"=w1182:refnum<queue>)  [unwired: 7 in]
      }
      event "Surge Backward MM": Value Change {
        n880 = event-data() -> ()  [unwired: 1 in, 1 out]
        n881 = call-poly "Enqueue Message.vi"("Priority Message? (F)"=TRUE, "Message"="Surge Backward MM", "Message Queue"=w1188) -> ("error out"=w1186:errorcluster, "dup Message Queue"=w1187:refnum<queue>)  [unwired: 7 in]
      }
      event "Surge Forward Main": Value Change {
        n882 = event-data() -> ()  [unwired: 1 in, 1 out]
        n883 = call-poly "Enqueue Message.vi"("Priority Message? (F)"=TRUE, "Message"="Surge Forward Main", "Message Queue"=w1193) -> ("error out"=w1191:errorcluster, "dup Message Queue"=w1192:refnum<queue>)  [unwired: 7 in]
      }
      event "Surge Forward MM": Value Change {
        n884 = event-data() -> ()  [unwired: 1 in, 1 out]
        n885 = call-poly "Enqueue Message.vi"("Priority Message? (F)"=TRUE, "Message"="Surge Forward MM", "Message Queue"=w1198) -> ("error out"=w1196:errorcluster, "dup Message Queue"=w1197:refnum<queue>)  [unwired: 7 in]
      }
      event "Sway Left Main": Value Change {
        n886 = event-data() -> ()  [unwired: 1 in, 1 out]
        n887 = call-poly "Enqueue Message.vi"("Priority Message? (F)"=TRUE, "Message"="Sway Left Main", "Message Queue"=w1203) -> ("error out"=w1201:errorcluster, "dup Message Queue"=w1202:refnum<queue>)  [unwired: 7 in]
      }
      event "Sway Left MM": Value Change {
        n888 = event-data() -> ()  [unwired: 1 in, 1 out]
        n889 = call-poly "Enqueue Message.vi"("Priority Message? (F)"=TRUE, "Message"="Sway Left MM", "Message Queue"=w1208) -> ("error out"=w1206:errorcluster, "dup Message Queue"=w1207:refnum<queue>)  [unwired: 7 in]
      }
      event "Sway Right MM": Value Change {
        n890 = event-data() -> ()  [unwired: 1 in, 1 out]
        n891 = call-poly "Enqueue Message.vi"("Priority Message? (F)"=TRUE, "Message"="Sway Right MM", "Message Queue"=w1213) -> ("error out"=w1211:errorcluster, "dup Message Queue"=w1212:refnum<queue>)  [unwired: 7 in]
      }
      event "Sway Right Main": Value Change {
        n892 = event-data() -> ()  [unwired: 1 in, 1 out]
        n893 = call-poly "Enqueue Message.vi"("Priority Message? (F)"=TRUE, "Message"="Sway Right Main", "Message Queue"=w1218) -> ("error out"=w1216:errorcluster, "dup Message Queue"=w1217:refnum<queue>)  [unwired: 7 in]
      }
      event "Load En": Value Change {
        n894 = event-data() -> ()  [unwired: 1 in, 1 out]
        n895 = call-poly "Enqueue Message.vi"("Priority Message? (F)"=TRUE, "Message"="Load En", "Message Queue"=w1223) -> ("error out"=w1221:errorcluster, "dup Message Queue"=w1222:refnum<queue>)  [unwired: 7 in]
      }
      event "PID.apply load": Value Change {
        n896 = event-data() -> ()  [unwired: 1 in, 1 out]
        n897 = call-poly "Enqueue Message.vi"("Priority Message? (F)"=TRUE, "Message"="apply load", "Message Queue"=w1228) -> ("error out"=w1226:errorcluster, "dup Message Queue"=w1227:refnum<queue>)  [unwired: 7 in]
      }
      event "BACK": Value Change {
        n898 = event-data() -> ()  [unwired: 1 in, 1 out]
        n899 = call-poly "Enqueue Message.vi"("Priority Message? (F)"=TRUE, "Message"="BACK", "Message Queue"=w1233) -> ("error out"=w1231:errorcluster, "dup Message Queue"=w1232:refnum<queue>)  [unwired: 7 in]
      }
      event "Start Test": Value Change {
        n900 = event-data() -> ()  [unwired: 1 in, 1 out]
        n901 = call-poly "Enqueue Message.vi"("Priority Message? (F)"=TRUE, "Message"="Start Test", "Message Queue"=w1238) -> ("error out"=w1236:errorcluster, "dup Message Queue"=w1237:refnum<queue>)  [unwired: 7 in]
      }
      event "STOP": Value Change {
        n902 = event-data() -> ()  [unwired: 1 in, 1 out]
        n903 = call-poly "Enqueue Message.vi"("Priority Message? (F)"=TRUE, "Message"="STOP", "Message Queue"=w1243) -> ("error out"=w1241:errorcluster, "dup Message Queue"=w1242:refnum<queue>)  [unwired: 7 in]
      }
      event "PlaceModule": Value Change {
        n904 = event-data() -> ()  [unwired: 1 in, 1 out]
        n905 = call-poly "Enqueue Message.vi"("Priority Message? (F)"=TRUE, "Message"="PlaceModule", "Message Queue"=w1248) -> ("error out"=w1246:errorcluster, "dup Message Queue"=w1247:refnum<queue>)  [unwired: 7 in]
      }
      event "HomeRot", "HomeScratch", "HomeScratch": Value Change {
        n906 = event-data() -> ()  [unwired: 1 in, 1 out]
        n907 = call-poly "Enqueue Message.vi"("Priority Message? (F)"=TRUE, "Message"="Stage Homing", "Message Queue"=w1253) -> ("error out"=w1251:errorcluster, "dup Message Queue"=w1252:refnum<queue>)  [unwired: 7 in]
      }
      event "Clear 3": Value Change {
        n908 = event-data() -> ()  [unwired: 1 in, 1 out]
        n909 = call-poly "Enqueue Message.vi"("Priority Message? (F)"=TRUE, "Message"="Clear 3", "Message Queue"=w1258) -> ("error out"=w1256:errorcluster, "dup Message Queue"=w1257:refnum<queue>)  [unwired: 7 in]
      }
      event "Set WTD": Value Change {
        n910 = event-data() -> ()  [unwired: 1 in, 1 out]
        n911 = call-poly "Enqueue Message.vi"("Priority Message? (F)"=TRUE, "Message"="Set WTD", "Message Queue"=w1263) -> ("error out"=w1261:errorcluster, "dup Message Queue"=w1262:refnum<queue>)  [unwired: 7 in]
      }
      event "Import 2": Value Change {
        n912 = event-data() -> ()  [unwired: 1 in, 1 out]
        n913 = call-poly "Enqueue Message.vi"("Priority Message? (F)"=TRUE, "Message"="Import 2", "Message Queue"=w1268) -> ("error out"=w1266:errorcluster, "dup Message Queue"=w1267:refnum<queue>)  [unwired: 7 in]
      }
      event "Import 3": Value Change {
        n914 = event-data() -> ()  [unwired: 1 in, 1 out]
        n915 = call-poly "Enqueue Message.vi"("Priority Message? (F)"=TRUE, "Message"="Import 3", "Message Queue"=w1273) -> ("error out"=w1271:errorcluster, "dup Message Queue"=w1272:refnum<queue>)  [unwired: 7 in]
      }
      event "Save 2": Value Change {
        n916 = event-data() -> ()  [unwired: 1 in, 1 out]
        n917 = call-poly "Enqueue Message.vi"("Priority Message? (F)"=TRUE, "Message"="Save 2", "Message Queue"=w1278) -> ("error out"=w1276:errorcluster, "dup Message Queue"=w1277:refnum<queue>)  [unwired: 7 in]
      }
      event "Save 3": Value Change {
        n918 = event-data() -> ()  [unwired: 1 in, 1 out]
        n919 = call-poly "Enqueue Message.vi"("Priority Message? (F)"=TRUE, "Message"="Save 3", "Message Queue"=w1283) -> ("error out"=w1281:errorcluster, "dup Message Queue"=w1282:refnum<queue>)  [unwired: 7 in]
      }
      event "calculate rotary": Value Change {
        n920 = event-data() -> ()  [unwired: 1 in, 1 out]
        n921 = call-poly "Enqueue Message.vi"("Priority Message? (F)"=TRUE, "Message"="Calculate Rotary", "Message Queue"=w1288) -> ("error out"=w1286:errorcluster, "dup Message Queue"=w1287:refnum<queue>)  [unwired: 7 in]
      }
      event "Clear List": Value Change {
        n922 = event-data() -> ()  [unwired: 1 in, 1 out]
        n923 = call-poly "Enqueue Message.vi"("Priority Message? (F)"=TRUE, "Message"="Clear List", "Message Queue"=w1293) -> ("error out"=w1291:errorcluster, "dup Message Queue"=w1292:refnum<queue>)  [unwired: 7 in]
      }
      event "Add to list": Value Change {
        n924 = event-data() -> ()  [unwired: 1 in, 1 out]
        n925 = call-poly "Enqueue Message.vi"("Priority Message? (F)"=TRUE, "Message"="Add to list", "Message Queue"=w1298) -> ("error out"=w1296:errorcluster, "dup Message Queue"=w1297:refnum<queue>)  [unwired: 7 in]
      }
      event "ClrLog": Value Change {
        n926 = event-data() -> ()  [unwired: 1 in, 1 out]
        n927 = call-poly "Enqueue Message.vi"("Priority Message? (F)"=TRUE, "Message"="ClrLog", "Message Queue"=w1303) -> ("error out"=w1301:errorcluster, "dup Message Queue"=w1302:refnum<queue>)  [unwired: 7 in]
      }
      event "Disable Axis Jog Soft Limits m": Value Change {
        n928 = event-data() -> ()  [unwired: 1 in, 1 out]
        n929 = call-poly "Enqueue Message.vi"("Priority Message? (F)"=TRUE, "Message"="Disable Axis Jog Soft Limits", "Message Queue"=w1308) -> ("error out"=w1306:errorcluster, "dup Message Queue"=w1307:refnum<queue>)  [unwired: 7 in]
      }
      event "Home Service": Value Change {
        n930 = event-data() -> ()  [unwired: 1 in, 1 out]
        n931 = call-poly "Enqueue Message.vi"("Priority Message? (F)"=TRUE, "Message"="Home Service", "Message Queue"=w1313) -> ("error out"=w1311:errorcluster, "dup Message Queue"=w1312:refnum<queue>)  [unwired: 7 in]
      }
      event "Edit Gain Constants": Value Change {
        n932 = event-data() -> ()  [unwired: 1 in, 1 out]
        n933 = call-poly "Enqueue Message.vi"("Priority Message? (F)"=TRUE, "Message"="Edit Gain Constants", "Message Queue"=w1318) -> ("error out"=w1316:errorcluster, "dup Message Queue"=w1317:refnum<queue>)  [unwired: 7 in]
      }
      event "Advanced Setting": Value Change {
        n934 = event-data() -> ()  [unwired: 1 in, 1 out]
        n935 = call-poly "Enqueue Message.vi"("Priority Message? (F)"=TRUE, "Message"="Advanced Setting", "Message Queue"=w1323) -> ("error out"=w1321:errorcluster, "dup Message Queue"=w1322:refnum<queue>)  [unwired: 7 in]
      }
      event "Password": Value Change {
        n936 = event-data() -> ()  [unwired: 1 in, 1 out]
        n937 = call-poly "Enqueue Message.vi"("Priority Message? (F)"=TRUE, "Message"="Password", "Message Queue"=w1328) -> ("error out"=w1326:errorcluster, "dup Message Queue"=w1327:refnum<queue>)  [unwired: 7 in]
      }
      event "Service About": Value Change {
        n938 = event-data() -> ()  [unwired: 1 in, 1 out]
        n939 = call-poly "Enqueue Message.vi"("Priority Message? (F)"=TRUE, "Message"="Service About", "Message Queue"=w1333) -> ("error out"=w1331:errorcluster, "dup Message Queue"=w1332:refnum<queue>)  [unwired: 7 in]
      }
      event "OPEN 1": Value Change {
        n940 = event-data() -> ()  [unwired: 1 in, 1 out]
        n941 = call-poly "Enqueue Message.vi"("Priority Message? (F)"=TRUE, "Message"="OPEN 1", "Message Queue"=w1338) -> ("error out"=w1336:errorcluster, "dup Message Queue"=w1337:refnum<queue>)  [unwired: 7 in]
      }
      event "OPEN 2": Value Change {
        n942 = event-data() -> ()  [unwired: 1 in, 1 out]
        n943 = call-poly "Enqueue Message.vi"("Priority Message? (F)"=TRUE, "Message"="OPEN 2", "Message Queue"=w1343) -> ("error out"=w1341:errorcluster, "dup Message Queue"=w1342:refnum<queue>)  [unwired: 7 in]
      }
      event "OPEN 3": Value Change {
        n944 = event-data() -> ()  [unwired: 1 in, 1 out]
        n945 = call-poly "Enqueue Message.vi"("Priority Message? (F)"=TRUE, "Message"="OPEN 3", "Message Queue"=w1348) -> ("error out"=w1346:errorcluster, "dup Message Queue"=w1347:refnum<queue>)  [unwired: 7 in]
      }
      event "OPEN 4": Value Change {
        n946 = event-data() -> ()  [unwired: 1 in, 1 out]
        n947 = call-poly "Enqueue Message.vi"("Priority Message? (F)"=TRUE, "Message"="OPEN 4", "Message Queue"=w1353) -> ("error out"=w1351:errorcluster, "dup Message Queue"=w1352:refnum<queue>)  [unwired: 7 in]
      }
      event "Refresh 2": Value Change {
        n948 = event-data() -> ()  [unwired: 1 in, 1 out]
        n949 = call-poly "Enqueue Message.vi"("Priority Message? (F)"=TRUE, "Message"="Refresh 2", "Message Queue"=w1358) -> ("error out"=w1356:errorcluster, "dup Message Queue"=w1357:refnum<queue>)  [unwired: 7 in]
      }
      event "Analysis Home new": Value Change {
        n950 = event-data() -> ()  [unwired: 1 in, 1 out]
        n951 = call-poly "Enqueue Message.vi"("Priority Message? (F)"=TRUE, "Message"="Analysis Home", "Message Queue"=w1363) -> ("error out"=w1361:errorcluster, "dup Message Queue"=w1362:refnum<queue>)  [unwired: 7 in]
      }
      event "Post Analysis": Value Change {
        n952 = event-data() -> ()  [unwired: 1 in, 1 out]
        n953 = call-poly "Enqueue Message.vi"("Priority Message? (F)"=TRUE, "Message"="Post Analysis", "Message Queue"=w1368) -> ("error out"=w1366:errorcluster, "dup Message Queue"=w1367:refnum<queue>)  [unwired: 7 in]
      }
      event "Scratch Mode": Value Change {
        n954 = event-data() -> ()  [unwired: 1 in, 1 out]
        n955 = call-poly "Enqueue Message.vi"("Priority Message? (F)"=TRUE, "Message"="Scratch Mode", "Message Queue"=w1373) -> ("error out"=w1371:errorcluster, "dup Message Queue"=w1372:refnum<queue>)  [unwired: 7 in]
      }
      event "Export": Value Change {
        n956 = event-data() -> ()  [unwired: 1 in, 1 out]
        n957 = call-poly "Enqueue Message.vi"("Priority Message? (F)"=TRUE, "Message"="Export", "Message Queue"=w1378) -> ("error out"=w1376:errorcluster, "dup Message Queue"=w1377:refnum<queue>)  [unwired: 7 in]
      }
      event "Traction Receipe Update Details": Value Change {
        n958 = event-data() -> ()  [unwired: 1 in, 1 out]
        n959 = call-poly "Enqueue Message.vi"("Priority Message? (F)"=TRUE, "Message"="Traction Receipe Update Details", "Message Queue"=w1383) -> ("error out"=w1381:errorcluster, "dup Message Queue"=w1382:refnum<queue>)  [unwired: 7 in]
      }
      event "Manual Write TRACTION": Value Change {
        n960 = event-data() -> ()  [unwired: 1 in, 1 out]
        n961 = call-poly "Enqueue Message.vi"("Priority Message? (F)"=TRUE, "Message"="Manual Write TRACTION", "Message Queue"=w1388) -> ("error out"=w1386:errorcluster, "dup Message Queue"=w1387:refnum<queue>)  [unwired: 7 in]
      }
      event "Manual Write Acquostic": Value Change {
        n962 = event-data() -> ()  [unwired: 1 in, 1 out]
        n963 = call-poly "Enqueue Message.vi"("Priority Message? (F)"=TRUE, "Message"="Manual Write ACQUOSTIC", "Message Queue"=w1393) -> ("error out"=w1391:errorcluster, "dup Message Queue"=w1392:refnum<queue>)  [unwired: 7 in]
      }
      event "Report": Value Change {
        n964 = event-data() -> ()  [unwired: 1 in, 1 out]
        n965 = call-poly "Enqueue Message.vi"("Priority Message? (F)"=TRUE, "Message"="Report", "Message Queue"=w1398) -> ("error out"=w1396:errorcluster, "dup Message Queue"=w1397:refnum<queue>)  [unwired: 7 in]
      }
      event "Acoustic Emission 3": Value Change {
        n966 = event-data() -> ()  [unwired: 1 in, 1 out]
        n967 = call-poly "Enqueue Message.vi"("Priority Message? (F)"=TRUE, "Message"="Acoustic Emission 3", "Message Queue"=w1403) -> ("error out"=w1401:errorcluster, "dup Message Queue"=w1402:refnum<queue>)  [unwired: 7 in]
      }
      event Application Instance Close {
        # "#CodeRecommended - When a project closes, all VIs within that project are aborted and leave memory. However, any code placed in this event frame is guaranteed to run to completion, so add any cleanup code that absolutely must happen here."
        n968 = event-data() -> ()  [unwired: 1 in, 1 out]
      }
      event "EXIT": Value Change {
        n969 = event-data() -> ()  [unwired: 1 in, 1 out]
        n970 = call-poly "Enqueue Message.vi"("Priority Message? (F)"=TRUE, "Message"="Exit", "Message Queue"=w1411) -> ("error out"=w1410:errorcluster, "dup Message Queue"=w1409:refnum<queue>)  [unwired: 7 in]
      }
      event User Event {
        # "The Message Handling Loop processed an \"Exit\" message, which fired this event to stop the Event Handling Loop."
        n971 = event-data() -> ()  [unwired: 1 in, 1 out]
      }
    }
    n972 = call "LAB-IQ Error Handler - Event Handling Loop.vi"("error in (no error)"=w1011, "Message Queue"=w1009) -> ("dup error in"=w1008:errorcluster)  [unwired: 8 in, 1 out]
  }
  n973 = disable-structure "Diagram Disable Structure" shown="Enabled" {
    disable-tunnel: w30 -> [w1418 _]
    disable-tunnel: w5 -> [w1417 _]
    disable-tunnel: w6 -> [w1416 _]
    disable-tunnel: w2 -> [w1415 _]
    disable-tunnel: [w1414 _] -> w11
    frame Disabled {
      n974 = while {
        shift-right: [w1429] -> _
        shift-left: w1417 -> [w1430]
        tunnel: [w1423] -> w1414
        tunnel: w1418 -> [w1421]
        tunnel: w1415 -> [w1420]
        tunnel: w1416 -> [w1419]
        stop <- w1428 stop-if-true
        # "Humidity  Handling Loop"
        n975 = call "Dequeue Message.vi"("error in (no error)"=w1420, "Message Queue"=w1421) -> ("error out"=w1427:errorcluster, "Message Data"=w1425:variant, "Message"=w1426:string, "dup Message Queue"=w1424:refnum<queue>)  [unwired: 6 in]
        n976 = case "Message Cases" shown="\"Humidity Main\"" w1426 {
          selector: w1426 -> [_ _ _ _ _ w1474]
          tunnel: w1424 -> [w1431 w1442 _ w1461 w1473 _]
          tunnel: w1427 -> [w1434 w1439 w1458 w1465 w1467 _]
          tunnel: [w1435 w1443 w1452 w1463 w1469 w1475] -> w1422
          tunnel: w1430 -> [w1433 w1441 w1457 w1464 w1472 w1476]
          tunnel: [w1433 w1441 w1457 w1464 w1472 w1476] -> w1429
          tunnel: [_ _ _ _ TRUE _] -> w1428
          tunnel: w1425 -> [_ _ w1456 _ _ _]
          tunnel: w1419 -> [_ _ _ _ w1466 _]
          frame "init" {
            # "Initialize - All initialization work should take place in this message, since other loops can potentially enqueue messages that execute immediately after this one."
            n977 = call-poly "Enqueue Message.vi"("error in (no error)"=w1434, "Message"="Humidity Main", "Message Queue"=w1431) -> ("error out"=w1435:errorcluster)  [unwired: 7 in, 1 out]
          }
          frame "Humidity Main" {
            n978 = Unbundle By Name(w1441) -> ("Main Home Screen.EXIT"=w1440:refnum<vi>)
            n979 = property on="Property Node" class="Bool (strict)"(reference=w1440) -> (reference out=w1437:refnum<vi>, error out=w1438:errorcluster, "Value"=w1436:bool)  [unwired: 1 in]
            n980 = case shown="False" w1436 {
              tunnel: [w1446 w1450] -> w1443
              tunnel: w1442 -> [w1445 w1449]
              tunnel: w1439 -> [w1444 w1448]
              frame True {
                n981 = call-poly "Enqueue Message.vi"("error in (no error)"=w1444, "Message"="Confirm Quit", "Message Queue"=w1445) -> ("error out"=w1446:errorcluster)  [unwired: 7 in, 1 out]
              }
              frame False {
                n982 = call-poly "Enqueue Message.vi"("error in (no error)"=w1448, "Message"="Humidity Main", "Message Queue"=w1449) -> ("error out"=w1450:errorcluster)  [unwired: 7 in, 1 out]
              }
            }
            n983 = Close Reference(reference=w1437, error in (no error)=w1438) -> ()  [unwired: 1 out]
          }
          frame "Error" {
            # "#CodeRecommended - If you ever change the name of this \"Error\" message, you'll need to update the name in the Check Loop Error.vi as well."
            # "#CodeRecommended - Consider creating a system for logging errors in some way. These errors are for notification purposes only. Handling of specific errors should be performed in the message frames that generated the error."
            # "Error - Display an error dialog. This message is sent by the \"Error Handler\" VIs at the end of other loops in this application."
            n984 = Variant To Data(error in=w1458, type=errorcluster {"status"=FALSE, "code"=0, "source"=""} ("error constant"), Variant=w1456) -> (data=w1454:errorcluster, error out=w1453:errorcluster)
            n985 = call <vilib>:"Simple Error Handler.vi"("error in (no error)"=w1454) -> ()  [unwired: 4 in, 5 out]
            n986 = Merge Errors(w1453) -> (w1452:errorcluster)
          }
          frame "Confirm Quit" {
            # "#CodeNeeded - If you want to provide an \"Are you sure\" dialog (or some other notification) before the application exits, place that code here. This message is typically sent from a Panel Close? event."
            # "Confirm Quit - Message that can confirm whether or not the user wants to exit the application."
            n987 = call-poly "Enqueue Message.vi"("Priority Message? (F)"=TRUE, "error in (no error)"=w1465, "Message"="Exit", "Message Queue"=w1461) -> ("error out"=w1462:errorcluster)  [unwired: 6 in, 1 out]
            n988 = Merge Errors(w1462) -> (w1463:errorcluster)
          }
          frame "Exit" {
            # "Stop the VI"
            # "Release the message queue reference"
            # "#CodeNeeded - Add any required cleanup code here. Note that if 'Exit' was called as a result of an error, an error dialog will be displayed. Add any custom error handling for an 'Exit' condition here as well."
            # "Exit - Exit the application."
            n989 = call "Fire User Event - Stop.vi"("User Event - Stop"=w1466) -> ("error out"=w1468:errorcluster)  [unwired: 10 in]
            n990 = Release Queue(queue=w1473, error in (no error)=w1467) -> (error out=w1470:errorcluster)  [unwired: 1 in, 2 out]
            n991 = Merge Errors(w1468, w1470) -> (w1469:errorcluster)
          }
          frame Default {
            # "'Default' case only runs if there is a message that isn't defined in any of the other cases.  Output a programming error."
            n992 = xnode ("Error Ring")("parameter 0"=w1474) -> ("error out"=w1475:errorcluster)
          }
        }
        n993 = call "LAB-IQ Error Handler - Message Handling Loop.vi"("error in (no error)"=w1422, "Message Queue"=w1424) -> ("dup error in"=w1423:errorcluster)  [unwired: 8 in, 1 out]
      }
    }
    frame Enabled {
    }
  }
  n994 = disable-structure "Diagram Disable Structure" shown="Disabled" {
    disable-tunnel: w31 -> [w1488 _]
    disable-tunnel: w5 -> [w1487 _]
    disable-tunnel: w6 -> [w1486 _]
    disable-tunnel: w2 -> [w1485 w1554]
    disable-tunnel: [w1484 w1554] -> w12
    frame Disabled {
      n995 = while {
        shift-right: [w1499] -> _
        shift-left: w1487 -> [w1500]
        tunnel: [w1493] -> w1484
        tunnel: w1488 -> [w1491]
        tunnel: w1485 -> [w1490]
        tunnel: w1486 -> [w1489]
        stop <- w1498 stop-if-true
        # "ECR  Handling Loop"
        n996 = call "Dequeue Message.vi"("error in (no error)"=w1490, "Message Queue"=w1491) -> ("error out"=w1497:errorcluster, "Message Data"=w1495:variant, "Message"=w1496:string, "dup Message Queue"=w1494:refnum<queue>)  [unwired: 6 in]
        n997 = case "Message Cases" shown="\"ECR Main\"" w1496 {
          selector: w1496 -> [_ _ _ _ _ w1544]
          tunnel: w1494 -> [w1501 w1512 _ w1531 w1543 _]
          tunnel: w1497 -> [w1504 w1509 w1528 w1535 w1537 _]
          tunnel: [w1505 w1513 w1522 w1533 w1539 w1545] -> w1492
          tunnel: w1500 -> [w1503 w1511 w1527 w1534 w1542 w1546]
          tunnel: [w1503 w1511 w1527 w1534 w1542 w1546] -> w1499
          tunnel: [_ _ _ _ TRUE _] -> w1498
          tunnel: w1495 -> [_ _ w1526 _ _ _]
          tunnel: w1489 -> [_ _ _ _ w1536 _]
          frame "init" {
            # "Initialize - All initialization work should take place in this message, since other loops can potentially enqueue messages that execute immediately after this one."
            n998 = call-poly "Enqueue Message.vi"("error in (no error)"=w1504, "Message"="ECR Main", "Message Queue"=w1501) -> ("error out"=w1505:errorcluster)  [unwired: 7 in, 1 out]
          }
          frame "ECR Main" {
            n999 = Unbundle By Name(w1511) -> ("Main Home Screen.EXIT"=w1510:refnum<vi>)
            n1000 = property on="Property Node" class="Bool (strict)"(reference=w1510) -> (reference out=w1507:refnum<vi>, error out=w1508:errorcluster, "Value"=w1506:bool)  [unwired: 1 in]
            n1001 = case shown="False" w1506 {
              tunnel: [w1516 w1520] -> w1513
              tunnel: w1512 -> [w1515 w1519]
              tunnel: w1509 -> [w1514 w1518]
              frame True {
                n1002 = call-poly "Enqueue Message.vi"("error in (no error)"=w1514, "Message"="Confirm Quit", "Message Queue"=w1515) -> ("error out"=w1516:errorcluster)  [unwired: 7 in, 1 out]
              }
              frame False {
                n1003 = call-poly "Enqueue Message.vi"("error in (no error)"=w1518, "Message"="ECR Main", "Message Queue"=w1519) -> ("error out"=w1520:errorcluster)  [unwired: 7 in, 1 out]
              }
            }
            n1004 = Close Reference(reference=w1507, error in (no error)=w1508) -> ()  [unwired: 1 out]
          }
          frame "Error" {
            # "#CodeRecommended - If you ever change the name of this \"Error\" message, you'll need to update the name in the Check Loop Error.vi as well."
            # "#CodeRecommended - Consider creating a system for logging errors in some way. These errors are for notification purposes only. Handling of specific errors should be performed in the message frames that generated the error."
            # "Error - Display an error dialog. This message is sent by the \"Error Handler\" VIs at the end of other loops in this application."
            n1005 = Variant To Data(error in=w1528, type=errorcluster {"status"=FALSE, "code"=0, "source"=""} ("error constant"), Variant=w1526) -> (data=w1524:errorcluster, error out=w1523:errorcluster)
            n1006 = call <vilib>:"Simple Error Handler.vi"("error in (no error)"=w1524) -> ()  [unwired: 4 in, 5 out]
            n1007 = Merge Errors(w1523) -> (w1522:errorcluster)
          }
          frame "Confirm Quit" {
            # "#CodeNeeded - If you want to provide an \"Are you sure\" dialog (or some other notification) before the application exits, place that code here. This message is typically sent from a Panel Close? event."
            # "Confirm Quit - Message that can confirm whether or not the user wants to exit the application."
            n1008 = call-poly "Enqueue Message.vi"("Priority Message? (F)"=TRUE, "error in (no error)"=w1535, "Message"="Exit", "Message Queue"=w1531) -> ("error out"=w1532:errorcluster)  [unwired: 6 in, 1 out]
            n1009 = Merge Errors(w1532) -> (w1533:errorcluster)
          }
          frame "Exit" {
            # "Stop the VI"
            # "Release the message queue reference"
            # "#CodeNeeded - Add any required cleanup code here. Note that if 'Exit' was called as a result of an error, an error dialog will be displayed. Add any custom error handling for an 'Exit' condition here as well."
            # "Exit - Exit the application."
            n1010 = call "Fire User Event - Stop.vi"("User Event - Stop"=w1536) -> ("error out"=w1538:errorcluster)  [unwired: 10 in]
            n1011 = Release Queue(queue=w1543, error in (no error)=w1537) -> (error out=w1540:errorcluster)  [unwired: 1 in, 2 out]
            n1012 = Merge Errors(w1538, w1540) -> (w1539:errorcluster)
          }
          frame Default {
            # "'Default' case only runs if there is a message that isn't defined in any of the other cases.  Output a programming error."
            n1013 = xnode ("Error Ring")("parameter 0"=w1544) -> ("error out"=w1545:errorcluster)
          }
        }
        n1014 = call "LAB-IQ Error Handler - Message Handling Loop.vi"("error in (no error)"=w1492, "Message Queue"=w1494) -> ("dup error in"=w1493:errorcluster)  [unwired: 8 in, 1 out]
      }
    }
    frame Enabled {
    }
  }
  n1015 = while "Timed Loop" {
    shift-right: [w1573] -> _
    shift-left: w5 -> [w1574]
    tunnel: [w1567] -> w8
    tunnel: w27 -> [w1565]
    tunnel: w2 -> [w1564]
    tunnel: w6 -> [w1563]
    shift-right: [w1561] -> _
    shift-left: w17 -> [w1562]
    shift-right: [w1559] -> _
    shift-left: w17 -> [w1560]
    shift-right: [w1557] -> _
    shift-left: w17 -> [w1558]
    shift-right: [w1556] -> _
    shift-left: w17 -> [w1555]
    stop <- w1572 stop-if-true
    # "Load Pid  Handling Loop"
    n1016 = call "Dequeue Message.vi"("error in (no error)"=w1564, "Message Queue"=w1565) -> ("error out"=w1571:errorcluster, "Message Data"=w1569:variant, "Message"=w1570:string, "dup Message Queue"=w1568:refnum<queue>)  [unwired: 6 in]
    n1017 = case "Message Cases" shown="\"Load Pid Main\"" w1570 {
      selector: w1570 -> [_ _ _ _ _ w1681]
      tunnel: w1568 -> [w1579 w1609 _ w1660 w1676 _]
      tunnel: w1571 -> [w1582 w1607 w1653 w1664 w1670 _]
      tunnel: [w1583 w1610 w1647 w1662 w1672 w1682] -> w1566
      tunnel: w1574 -> [w1581 w1596 w1652 w1663 w1675 w1683]
      tunnel: [w1581 w1596 w1652 w1663 w1675 w1683] -> w1573
      tunnel: [_ _ _ _ TRUE _] -> w1572
      tunnel: w1569 -> [_ _ w1651 _ _ _]
      tunnel: w1563 -> [_ _ _ _ w1669 _]
      tunnel: w1562 -> [w1577 w1592 w1646 w1657 w1668 w1679]
      tunnel: [w1577 w1591 w1646 w1657 w1668 w1679] -> w1561
      tunnel: w1560 -> [w1578 w1590 w1645 w1656 w1667 w1680]
      tunnel: [w1578 w1589 w1645 w1656 w1667 w1680] -> w1559
      tunnel: w1558 -> [w1576 w1588 w1644 w1655 w1666 w1678]
      tunnel: [w1576 w1587 w1644 w1655 w1666 w1678] -> w1557
      tunnel: w1555 -> [_ w1586 _ _ _ _]
      tunnel: [w1575 w1585 w1643 w1654 w1665 w1677] -> w1556
      tunnel: w1555 -> [w1575 _ w1643 w1654 w1665 w1677]
      frame "init" {
        # "Initialize - All initialization work should take place in this message, since other loops can potentially enqueue messages that execute immediately after this one."
        n1018 = call-poly "Enqueue Message.vi"("error in (no error)"=w1582, "Message"="Load Pid Main", "Message Queue"=w1579) -> ("error out"=w1583:errorcluster)  [unwired: 7 in, 1 out]
      }
      frame "Load Pid Main" {
        n1019 = Unbundle By Name(w1596) -> ("Main Screen.Load En"=w1602:refnum<vi>)
        n1020 = Unbundle By Name(w1596) -> ("PID.apply load"=w1597:refnum<vi>)
        n1021 = property on="Property Node" class="Bool (strict)"(reference=w1602) -> (reference out=w1600:refnum<vi>, error out=w1601:errorcluster, "Value"=w1595:bool)  [unwired: 1 in]
        n1022 = property on="Property Node" class="Bool (strict)"(reference=w1597) -> (reference out=w1599:refnum<vi>, error out=w1598:errorcluster, "Value"=w1594:bool)  [unwired: 1 in]
        n1023 = Close Reference(reference=w1600, error in (no error)=w1601) -> ()  [unwired: 1 out]
        n1024 = Close Reference(reference=w1599, error in (no error)=w1598) -> ()  [unwired: 1 out]
        n1025 = Or(x=w1595, y=w1594) -> (x .or. y?=w1593:bool)
        n1026 = case shown="True" w1593 {
          tunnel: w1607 -> [w1617 w1630]
          tunnel: [w1617 w1629] -> w1603
          tunnel: w1596 -> [_ w1628]
          tunnel: w1592 -> [w1616 w1627]
          tunnel: [w1616 w1626] -> w1591
          tunnel: w1590 -> [w1615 w1625]
          tunnel: [w1615 w1624] -> w1589
          tunnel: w1588 -> [w1612 w1621]
          tunnel: [w1612 w1620] -> w1587
          tunnel: w1586 -> [w1611 w1619]
          tunnel: [w1611 w1618] -> w1585
          frame False {
            n1027 = local write "Checkbox 2"(TRUE ("Checkbox 2")) -> ()
            n1028 = local write "Checkbox"(TRUE ("Checkbox")) -> ()
          }
          frame True {
            n1029 = case shown="True" "Checkbox 2" {
              selector: "Checkbox 2" -> [_ w1633]
              tunnel: [FALSE ("Checkbox") "Checkbox"] -> w1623
              frame False {
              }
              frame True {
                n1030 = Not(x=w1633) -> (.not. x?=w1632:bool)
                n1031 = local write "Checkbox 2"(w1632) -> ()
              }
            }
            n1032 = call "NEW LOAD CELL PID.vi"("filtered_load_in"=w1621, "filtered_deriv_in"=w1619, "integral_out"=w1625, "error in (no error)"=w1630, "prev_error_out"=w1627, "Checkbox"=w1623, "main ref"=w1628) -> ("error out"=w1629:errorcluster, "prev_error_out"=w1626:dbl, "integral_out"=w1624:dbl, "filtered_load_out"=w1620:dbl, "filtered_deriv_out"=w1618:dbl)
          }
        }
        n1033 = Unbundle By Name(w1596) -> ("Main Home Screen.EXIT"=w1608:refnum<vi>)
        n1034 = property on="Property Node" class="Bool (strict)"(reference=w1608) -> (reference out=w1605:refnum<vi>, error out=w1606:errorcluster, "Value"=w1604:bool)  [unwired: 1 in]
        n1035 = case shown="False" w1604 {
          tunnel: [w1637 w1641] -> w1610
          tunnel: w1609 -> [w1636 w1640]
          tunnel: w1603 -> [w1635 w1639]
          frame True {
            n1036 = call-poly "Enqueue Message.vi"("error in (no error)"=w1635, "Message"="Confirm Quit", "Message Queue"=w1636) -> ("error out"=w1637:errorcluster)  [unwired: 7 in, 1 out]
          }
          frame False {
            n1037 = call-poly "Enqueue Message.vi"("error in (no error)"=w1639, "Message"="Load Pid Main", "Message Queue"=w1640) -> ("error out"=w1641:errorcluster)  [unwired: 7 in, 1 out]
          }
        }
        n1038 = Close Reference(reference=w1605, error in (no error)=w1606) -> ()  [unwired: 1 out]
        n1039 = Wait (ms)(milliseconds to wait=u32 30) -> ()  [unwired: 1 out]
      }
      frame "Error" {
        # "#CodeRecommended - If you ever change the name of this \"Error\" message, you'll need to update the name in the Check Loop Error.vi as well."
        # "#CodeRecommended - Consider creating a system for logging errors in some way. These errors are for notification purposes only. Handling of specific errors should be performed in the message frames that generated the error."
        # "Error - Display an error dialog. This message is sent by the \"Error Handler\" VIs at the end of other loops in this application."
        n1040 = Variant To Data(error in=w1653, type=errorcluster {"status"=FALSE, "code"=0, "source"=""} ("error constant"), Variant=w1651) -> (data=w1649:errorcluster, error out=w1648:errorcluster)
        n1041 = call <vilib>:"Simple Error Handler.vi"("error in (no error)"=w1649) -> ()  [unwired: 4 in, 5 out]
        n1042 = Merge Errors(w1648) -> (w1647:errorcluster)
      }
      frame "Confirm Quit" {
        # "#CodeNeeded - If you want to provide an \"Are you sure\" dialog (or some other notification) before the application exits, place that code here. This message is typically sent from a Panel Close? event."
        # "Confirm Quit - Message that can confirm whether or not the user wants to exit the application."
        n1043 = call-poly "Enqueue Message.vi"("Priority Message? (F)"=TRUE, "error in (no error)"=w1664, "Message"="Exit", "Message Queue"=w1660) -> ("error out"=w1661:errorcluster)  [unwired: 6 in, 1 out]
        n1044 = Merge Errors(w1661) -> (w1662:errorcluster)
      }
      frame "Exit" {
        # "Stop the VI"
        # "Release the message queue reference"
        # "#CodeNeeded - Add any required cleanup code here. Note that if 'Exit' was called as a result of an error, an error dialog will be displayed. Add any custom error handling for an 'Exit' condition here as well."
        # "Exit - Exit the application."
        n1045 = call "Fire User Event - Stop.vi"("User Event - Stop"=w1669) -> ("error out"=w1671:errorcluster)  [unwired: 10 in]
        n1046 = Release Queue(queue=w1676, error in (no error)=w1670) -> (error out=w1673:errorcluster)  [unwired: 1 in, 2 out]
        n1047 = Merge Errors(w1671, w1673) -> (w1672:errorcluster)
      }
      frame Default {
        # "'Default' case only runs if there is a message that isn't defined in any of the other cases.  Output a programming error."
        n1048 = xnode ("Error Ring")("parameter 0"=w1681) -> ("error out"=w1682:errorcluster)
      }
    }
    n1049 = call "LAB-IQ Error Handler - Message Handling Loop.vi"("error in (no error)"=w1566, "Message Queue"=w1568) -> ("dup error in"=w1567:errorcluster)  [unwired: 8 in, 1 out]
  }
  n1050 = disable-structure "Diagram Disable Structure" shown="Disabled" {
    disable-tunnel: w34 -> [w1695 _]
    disable-tunnel: w5 -> [w1694 _]
    disable-tunnel: w6 -> [w1693 _]
    disable-tunnel: w2 -> [w1692 w1761]
    disable-tunnel: [w1691 w1761] -> w19
    frame Disabled {
      n1051 = while {
        shift-right: [w1706] -> _
        shift-left: w1694 -> [w1707]
        tunnel: [w1700] -> w1691
        tunnel: w1695 -> [w1698]
        tunnel: w1692 -> [w1697]
        tunnel: w1693 -> [w1696]
        stop <- w1705 stop-if-true
        # "Temperature  Handling Loop"
        n1052 = call "Dequeue Message.vi"("error in (no error)"=w1697, "Message Queue"=w1698) -> ("error out"=w1704:errorcluster, "Message Data"=w1702:variant, "Message"=w1703:string, "dup Message Queue"=w1701:refnum<queue>)  [unwired: 6 in]
        n1053 = case "Message Cases" shown="\"Temperature Main\"" w1703 {
          selector: w1703 -> [_ _ _ _ _ w1751]
          tunnel: w1701 -> [w1708 w1719 _ w1738 w1750 _]
          tunnel: w1704 -> [w1711 w1716 w1735 w1742 w1744 _]
          tunnel: [w1712 w1720 w1729 w1740 w1746 w1752] -> w1699
          tunnel: w1707 -> [w1710 w1718 w1734 w1741 w1749 w1753]
          tunnel: [w1710 w1718 w1734 w1741 w1749 w1753] -> w1706
          tunnel: [_ _ _ _ TRUE _] -> w1705
          tunnel: w1702 -> [_ _ w1733 _ _ _]
          tunnel: w1696 -> [_ _ _ _ w1743 _]
          frame "init" {
            # "Initialize - All initialization work should take place in this message, since other loops can potentially enqueue messages that execute immediately after this one."
            n1054 = call-poly "Enqueue Message.vi"("error in (no error)"=w1711, "Message"="Temperature Main", "Message Queue"=w1708) -> ("error out"=w1712:errorcluster)  [unwired: 7 in, 1 out]
          }
          frame "Temperature Main" {
            n1055 = Unbundle By Name(w1718) -> ("Main Home Screen.EXIT"=w1717:refnum<vi>)
            n1056 = property on="Property Node" class="Bool (strict)"(reference=w1717) -> (reference out=w1714:refnum<vi>, error out=w1715:errorcluster, "Value"=w1713:bool)  [unwired: 1 in]
            n1057 = case shown="False" w1713 {
              tunnel: [w1723 w1727] -> w1720
              tunnel: w1719 -> [w1722 w1726]
              tunnel: w1716 -> [w1721 w1725]
              frame True {
                n1058 = call-poly "Enqueue Message.vi"("error in (no error)"=w1721, "Message"="Confirm Quit", "Message Queue"=w1722) -> ("error out"=w1723:errorcluster)  [unwired: 7 in, 1 out]
              }
              frame False {
                n1059 = call-poly "Enqueue Message.vi"("error in (no error)"=w1725, "Message"="Temperature Main", "Message Queue"=w1726) -> ("error out"=w1727:errorcluster)  [unwired: 7 in, 1 out]
              }
            }
            n1060 = Close Reference(reference=w1714, error in (no error)=w1715) -> ()  [unwired: 1 out]
          }
          frame "Error" {
            # "#CodeRecommended - If you ever change the name of this \"Error\" message, you'll need to update the name in the Check Loop Error.vi as well."
            # "#CodeRecommended - Consider creating a system for logging errors in some way. These errors are for notification purposes only. Handling of specific errors should be performed in the message frames that generated the error."
            # "Error - Display an error dialog. This message is sent by the \"Error Handler\" VIs at the end of other loops in this application."
            n1061 = Variant To Data(error in=w1735, type=errorcluster {"status"=FALSE, "code"=0, "source"=""} ("error constant"), Variant=w1733) -> (data=w1731:errorcluster, error out=w1730:errorcluster)
            n1062 = call <vilib>:"Simple Error Handler.vi"("error in (no error)"=w1731) -> ()  [unwired: 4 in, 5 out]
            n1063 = Merge Errors(w1730) -> (w1729:errorcluster)
          }
          frame "Confirm Quit" {
            # "#CodeNeeded - If you want to provide an \"Are you sure\" dialog (or some other notification) before the application exits, place that code here. This message is typically sent from a Panel Close? event."
            # "Confirm Quit - Message that can confirm whether or not the user wants to exit the application."
            n1064 = call-poly "Enqueue Message.vi"("Priority Message? (F)"=TRUE, "error in (no error)"=w1742, "Message"="Exit", "Message Queue"=w1738) -> ("error out"=w1739:errorcluster)  [unwired: 6 in, 1 out]
            n1065 = Merge Errors(w1739) -> (w1740:errorcluster)
          }
          frame "Exit" {
            # "Stop the VI"
            # "Release the message queue reference"
            # "#CodeNeeded - Add any required cleanup code here. Note that if 'Exit' was called as a result of an error, an error dialog will be displayed. Add any custom error handling for an 'Exit' condition here as well."
            # "Exit - Exit the application."
            n1066 = call "Fire User Event - Stop.vi"("User Event - Stop"=w1743) -> ("error out"=w1745:errorcluster)  [unwired: 10 in]
            n1067 = Release Queue(queue=w1750, error in (no error)=w1744) -> (error out=w1747:errorcluster)  [unwired: 1 in, 2 out]
            n1068 = Merge Errors(w1745, w1747) -> (w1746:errorcluster)
          }
          frame Default {
            # "'Default' case only runs if there is a message that isn't defined in any of the other cases.  Output a programming error."
            n1069 = xnode ("Error Ring")("parameter 0"=w1751) -> ("error out"=w1752:errorcluster)
          }
        }
        n1070 = call "LAB-IQ Error Handler - Message Handling Loop.vi"("error in (no error)"=w1699, "Message Queue"=w1701) -> ("dup error in"=w1700:errorcluster)  [unwired: 8 in, 1 out]
      }
    }
    frame Enabled {
    }
  }
  n1071 = while "Timed Loop" {
    shift-right: [w1773] -> _
    shift-left: w5 -> [w1774]
    tunnel: [w1767] -> w33
    tunnel: w22 -> [w1765]
    tunnel: w2 -> [w1764]
    tunnel: w6 -> [w1763]
    stop <- w1772 stop-if-true
    # "Heave Motor  Handling Loop"
    n1072 = call "Dequeue Message.vi"("error in (no error)"=w1764, "Message Queue"=w1765) -> ("error out"=w1771:errorcluster, "Message Data"=w1769:variant, "Message"=w1770:string, "dup Message Queue"=w1768:refnum<queue>)  [unwired: 6 in]
    n1073 = case "Message Cases" shown="\"init\"" w1770 {
      selector: w1770 -> [_ _ _ _ _ w1867]
      tunnel: w1768 -> [w1787 w1803 _ w1855 w1866 _]
      tunnel: w1771 -> [w1784 w1801 w1847 w1858 w1860 _]
      tunnel: [w1785 w1804 w1841 w1848 w1862 w1868] -> w1766
      tunnel: w1774 -> [w1776 w1789 w1846 w1851 w1865 w1869]
      tunnel: [w1776 w1789 w1846 w1851 w1865 w1869] -> w1773
      tunnel: [_ _ _ _ TRUE _] -> w1772
      tunnel: w1769 -> [_ _ w1845 _ _ _]
      tunnel: w1763 -> [_ _ _ _ w1859 _]
      frame "init" {
        # "Initialize - All initialization work should take place in this message, since other loops can potentially enqueue messages that execute immediately after this one."
        n1074 = call "HEAVE WRITE FGV.vi"("Enum - Menu"=Heave_Write_enum."INIT", "error in (no error)"=w1784, "main ref"=w1776) -> ("error out"=w1783:errorcluster)  [unwired: 8 in]
        n1075 = call <vilib>:"Clear Errors.vi"("error in (no error)"=w1783) -> ("error out"=w1778:errorcluster)  [unwired: 5 in, 1 out]
        n1076 = call "Stall Data Flow.vim"("value in"=w1778, "milliseconds to wait"=u32 1000) -> ("value out"=w1781:errorcluster)  [unwired: 1 out]
        n1077 = call "Heave Init.vi"("error in (no error)"=w1781, "main ref"=w1776) -> ("error out"=w1779:errorcluster)  [unwired: 9 in]
        n1078 = call "HEAVE READ FGV.vi"("Enum - Menu"=Heave_Right_enum."INIT", "error in (no error)"=w1779, "main ref"=w1776) -> ("error out"=w1777:errorcluster)  [unwired: 6 in, 2 out]
        n1079 = call <vilib>:"Clear Errors.vi"("error in (no error)"=w1777) -> ("error out"=w1786:errorcluster)  [unwired: 5 in, 1 out]
        n1080 = call-poly "Enqueue Message.vi"("error in (no error)"=w1786, "Message"="Heave Main", "Message Queue"=w1787) -> ("error out"=w1785:errorcluster)  [unwired: 7 in, 1 out]
      }
      frame "Heave Main" {
        n1081 = Unbundle By Name(w1789) -> ("Heave AND Surge.Read Heave Temp"=w1797:refnum<vi>)
        n1082 = property on="Property Node" class="Bool (strict)"(reference=w1797) -> (reference out=w1795:refnum<vi>, error out=w1796:errorcluster, "Value"=w1794:bool)  [unwired: 1 in]
        n1083 = Close Reference(reference=w1795, error in (no error)=w1796) -> ()  [unwired: 1 out]
        n1084 = case shown="True" w1794 {
          tunnel: w1801 -> [w1827 w1832]
          tunnel: [w1827 w1831] -> w1792
          tunnel: w1789 -> [_ w1830]
          tunnel: [FALSE ("x < y?") w1829] -> w1790
          frame False {
          }
          frame True {
            n1085 = call "HEAVE READ FGV.vi"("Enum - Menu"=Heave_Right_enum."READ", "error in (no error)"=w1832, "main ref"=w1830) -> ("error out"=w1831:errorcluster, "x < y?"=w1829:bool)  [unwired: 6 in, 1 out]
          }
        }
        n1086 = case shown="True" w1790 {
          tunnel: w1789 -> [w1807 w1814]
          frame False {
            w1805 = TRUE ("PAUSE")
            w1806 = FALSE ("Value")
            n1087 = Unbundle By Name(w1807) -> ("Platform Settings.Heave COM Status"=w1813:refnum<vi>)
            n1088 = Unbundle By Name(w1807) -> ("Main Screen.Heave COM Status"=w1808:refnum<vi>)
            n1089 = property on="Property Node" class="Bool (strict)"(reference=w1813, "Value"=w1806) -> (reference out=w1811:refnum<vi>, error out=w1812:errorcluster)  [unwired: 1 in]
            n1090 = property on="Property Node" class="Bool (strict)"(reference=w1808, "Value"=w1806) -> (reference out=w1810:refnum<vi>, error out=w1809:errorcluster)  [unwired: 1 in]
            n1091 = Close Reference(reference=w1811, error in (no error)=w1812) -> ()  [unwired: 1 out]
            n1092 = Close Reference(reference=w1810, error in (no error)=w1809) -> ()  [unwired: 1 out]
            n1093 = call "ELAPSED TIMER VI FOR Sway Loop Connection.vi"("RESET"=w1805, "PAUSE"=w1805) -> ()  [unwired: 7 in, 3 out]
          }
          frame True {
            w1817 = FALSE ("PAUSE")
            n1094 = call "ELAPSED TIMER VI FOR Sway Loop Connection.vi"("TARGET"=2.0, "RESET"=w1817, "PAUSE"=w1817) -> ("ELAPSED INDICATION"=w1815:bool)  [unwired: 6 in, 2 out]
            n1095 = case shown="True" w1815 {
              tunnel: w1814 -> [_ w1818]
              frame False {
              }
              frame True {
                w1819 = TRUE ("Value")
                n1096 = Unbundle By Name(w1818) -> ("Main Screen.Heave COM Status"=w1820:refnum<vi>)
                n1097 = Unbundle By Name(w1818) -> ("Platform Settings.Heave COM Status"=w1825:refnum<vi>)
                n1098 = property on="Property Node" class="Bool (strict)"(reference=w1820, "Value"=w1819) -> (reference out=w1822:refnum<vi>, error out=w1821:errorcluster)  [unwired: 1 in]
                n1099 = property on="Property Node" class="Bool (strict)"(reference=w1825, "Value"=w1819) -> (reference out=w1823:refnum<vi>, error out=w1824:errorcluster)  [unwired: 1 in]
                n1100 = Close Reference(reference=w1822, error in (no error)=w1821) -> ()  [unwired: 1 out]
                n1101 = Close Reference(reference=w1823, error in (no error)=w1824) -> ()  [unwired: 1 out]
              }
            }
          }
        }
        n1102 = call "Heave Reinitial.vi"("error in (no error)"=w1792, "Data Cluster"=w1789) -> ("error out"=w1791:errorcluster)  [unwired: 9 in]
        n1103 = Unbundle By Name(w1789) -> ("Main Home Screen.EXIT"=w1802:refnum<vi>)
        n1104 = property on="Property Node" class="Bool (strict)"(reference=w1802) -> (reference out=w1799:refnum<vi>, error out=w1800:errorcluster, "Value"=w1798:bool)  [unwired: 1 in]
        n1105 = call <vilib>:"Clear Errors.vi"("error in (no error)"=w1791) -> ("error out"=w1793:errorcluster)  [unwired: 5 in, 1 out]
        n1106 = Close Reference(reference=w1799, error in (no error)=w1800) -> ()  [unwired: 1 out]
        n1107 = case shown="False" w1798 {
          tunnel: [w1835 w1839] -> w1804
          tunnel: w1803 -> [w1834 w1838]
          tunnel: w1793 -> [w1833 w1837]
          frame True {
            n1108 = call-poly "Enqueue Message.vi"("error in (no error)"=w1833, "Message"="Confirm Quit", "Message Queue"=w1834) -> ("error out"=w1835:errorcluster)  [unwired: 7 in, 1 out]
          }
          frame False {
            n1109 = call-poly "Enqueue Message.vi"("error in (no error)"=w1837, "Message"="Heave Main", "Message Queue"=w1838) -> ("error out"=w1839:errorcluster)  [unwired: 7 in, 1 out]
          }
        }
      }
      frame "Error" {
        # "#CodeRecommended - If you ever change the name of this \"Error\" message, you'll need to update the name in the Check Loop Error.vi as well."
        # "#CodeRecommended - Consider creating a system for logging errors in some way. These errors are for notification purposes only. Handling of specific errors should be performed in the message frames that generated the error."
        # "Error - Display an error dialog. This message is sent by the \"Error Handler\" VIs at the end of other loops in this application."
        n1110 = Variant To Data(error in=w1847, type=errorcluster {"status"=FALSE, "code"=0, "source"=""} ("error constant"), Variant=w1845) -> (data=w1843:errorcluster, error out=w1842:errorcluster)
        n1111 = call <vilib>:"Simple Error Handler.vi"("error in (no error)"=w1843) -> ()  [unwired: 4 in, 5 out]
        n1112 = Merge Errors(w1842) -> (w1841:errorcluster)
      }
      frame "Confirm Quit" {
        # "#CodeNeeded - If you want to provide an \"Are you sure\" dialog (or some other notification) before the application exits, place that code here. This message is typically sent from a Panel Close? event."
        # "Confirm Quit - Message that can confirm whether or not the user wants to exit the application."
        n1113 = call-poly "Enqueue Message.vi"("Priority Message? (F)"=TRUE, "error in (no error)"=w1858, "Message"="Exit", "Message Queue"=w1855) -> ("error out"=w1856:errorcluster)  [unwired: 6 in, 1 out]
        n1114 = Merge Errors(w1856) -> (w1857:errorcluster)
        n1115 = call <vilib>:"Clear Errors.vi"("error in (no error)"=w1857) -> ("error out"=w1849:errorcluster)  [unwired: 5 in, 1 out]
        n1116 = call "HEAVE WRITE FGV.vi"("Enum - Menu"=Heave_Write_enum."CLOSE", "error in (no error)"=w1849, "main ref"=w1851) -> ("error out"=w1852:errorcluster)  [unwired: 8 in]
        n1117 = call <vilib>:"Clear Errors.vi"("error in (no error)"=w1852) -> ("error out"=w1848:errorcluster)  [unwired: 5 in, 1 out]
      }
      frame "Exit" {
        # "Stop the VI"
        # "Release the message queue reference"
        # "#CodeNeeded - Add any required cleanup code here. Note that if 'Exit' was called as a result of an error, an error dialog will be displayed. Add any custom error handling for an 'Exit' condition here as well."
        # "Exit - Exit the application."
        n1118 = call "Fire User Event - Stop.vi"("User Event - Stop"=w1859) -> ("error out"=w1861:errorcluster)  [unwired: 10 in]
        n1119 = Release Queue(queue=w1866, error in (no error)=w1860) -> (error out=w1863:errorcluster)  [unwired: 1 in, 2 out]
        n1120 = Merge Errors(w1861, w1863) -> (w1862:errorcluster)
      }
      frame Default {
        # "'Default' case only runs if there is a message that isn't defined in any of the other cases.  Output a programming error."
        n1121 = xnode ("Error Ring")("parameter 0"=w1867) -> ("error out"=w1868:errorcluster)
      }
    }
    n1122 = call "LAB-IQ Error Handler - Message Handling Loop.vi"("error in (no error)"=w1766, "Message Queue"=w1768) -> ("dup error in"=w1767:errorcluster)  [unwired: 8 in, 1 out]
    n1123 = Wait (ms)(milliseconds to wait=u32 5) -> ()  [unwired: 1 out]
  }
  n1124 = while {
    tunnel: w64 -> [w1880]
    shift-right: [w1887] -> _
    shift-left: w5 -> [w1888]
    tunnel: w6 -> [w1885]
    tunnel: w57 -> [w1884]
    tunnel: [w1878] -> w65
    stop <- w1886 stop-if-true
    # "Message Handling Loop"
    n1125 = call "Dequeue Message.vi"("error in (no error)"=w1884, "Message Queue"=w1880) -> ("error out"=w1883:errorcluster, "Message Data"=w1881:variant, "Message"=w1882:string, "dup Message Queue"=w1879:refnum<queue>)  [unwired: 6 in]
    n1126 = case "Message Cases" shown="\"ZeroAll\"" w1882 {
      selector: w1882 -> [_ _ _ _ _ _ _ _ _ _ _ _ _ _ _ _ _ _ _ _ _ _ _ _ _ _ _ _ _ _ _ _ _ _ _ _ _ _ _ _ _ _ _ _ _ _ _ _ _ _ _ _ _ _ _ _ _ _ _ _ _ _ _ _ _ _ _ _ _ _ _ _ _ _ _ _ _ _ _ _ _ _ w3311]
      tunnel: w1879 -> [_ w1933 _ _ _ _ _ _ _ _ _ _ _ _ _ _ _ _ _ _ _ _ _ _ _ _ _ _ _ _ _ _ _ _ _ _ _ _ _ _ _ _ _ _ _ _ _ _ _ _ _ _ _ _ _ _ _ _ _ _ _ _ _ _ _ _ _ _ _ _ _ _ _ _ _ _ _ _ _ _ w3299 w3310 _]
      tunnel: w1883 -> [w1889 w1935 w1937 w1947 w1968 w1985 w2002 w2019 w2040 w2053 w2058 w2063 w2075 w2080 w2145 w2171 w2197 w2232 w2248 w2300 w2304 w2307 w2310 w2317 w2393 w2405 w2422 w2434 w2460 w2471 w2482 w2493 w2504 w2515 w2526 w2537 w2549 w2560 w2571 w2582 w2591 w2602 w2612 w2623 w2630 w2660 w2701 w2707 w2739 w2747 w2750 w2758 w2770 w2779 w2799 w2819 w2834 w2848 w2858 w2868 w2870 w2885 w2898 w2915 w2932 w2968 w2976 w3035 w3059 w3069 w3110 w3153 w3196 w3232 w3239 w3258 w3264 w3272 w3288 w3295 w3302 w3303 _]
      tunnel: [w1891 w1906 w1939 w1948 w1963 w1980 w1997 w2014 w2035 w2045 w2056 w2061 w2073 w2084 w2141 w2167 w2193 w2233 w2249 w2264 w2303 w2306 w2309 w2316 w2387 w2404 w2423 w2446 w2462 w2473 w2484 w2495 w2506 w2517 w2528 w2539 w2550 w2561 w2572 w2583 w2593 w2603 w2613 w2624 w2629 w2659 w2680 w2712 w2720 w2746 w2749 w2757 w2764 w2774 w2794 w2812 w2831 w2847 w2858 w2868 w2876 w2884 w2897 w2914 w2931 w2967 w2975 w3035 w3059 w3066 w3107 w3150 w3193 w3233 w3239 w3252 w3262 w3271 w3286 w3289 w3301 w3306 w3312] -> w1877
      tunnel: w1888 -> [w1890 w1893 w1938 w1946 w1954 w1971 w1988 w2005 w2023 w2043 w2055 w2060 w2068 w2079 w2143 w2169 w2195 w2220 w2235 w2251 w2302 w2305 w2308 w2311 w2386 w2403 w2416 w2430 w2458 w2469 w2480 w2491 w2502 w2513 w2524 w2535 w2547 w2558 w2569 w2580 w2590 w2601 w2611 w2622 w2628 w2658 w2679 w2705 w2718 w2745 w2748 w2752 w2763 w2772 w2792 w2814 w2832 w2846 w2850 w2860 w2869 w2883 w2887 w2900 w2918 w2934 w2970 w3027 w3050 w3062 w3103 w3146 w3189 w3231 w3234 w3251 w3261 w3266 w3285 w3294 w3296 w3309 w3313]
      tunnel: [w1890 w1893 w1938 w1946 w1954 w1971 w1988 w2005 w2023 w2043 w2055 w2060 w2068 w2079 w2143 w2169 w2195 w2220 w2235 w2251 w2302 w2305 w2308 w2311 w2386 w2403 w2416 w2430 w2458 w2469 w2480 w2491 w2502 w2513 w2524 w2535 w2547 w2558 w2569 w2580 w2590 w2601 w2611 w2622 w2628 w2658 w2679 w2705 w2718 w2745 w2748 w2752 w2763 w2772 w2792 w2814 w2832 w2846 w2850 w2860 w2869 w2883 w2887 w2900 w2918 w2934 w2970 w3027 w3050 w3062 w3103 w3146 w3189 w3231 w3234 w3251 w3261 w3266 w3285 w3294 w3296 w3309 w3313] -> w1887
      tunnel: [_ _ _ _ _ _ _ _ _ _ _ _ _ _ _ _ _ _ _ _ _ _ _ _ _ _ _ _ _ _ _ _ _ _ _ _ _ _ _ _ _ _ _ _ _ _ _ _ _ _ _ _ _ _ _ _ _ _ _ _ _ _ _ _ _ _ _ _ _ _ _ _ _ _ _ _ _ _ _ _ _ TRUE _] -> w1886
      tunnel: w1881 -> [_ _ _ _ _ _ _ _ _ _ _ _ _ _ _ _ _ _ _ _ _ _ _ _ _ _ _ _ _ _ _ _ _ _ _ _ _ _ _ _ _ _ _ _ _ _ _ _ _ _ _ _ _ _ _ _ _ _ _ _ _ _ _ _ _ _ _ _ _ _ _ _ _ _ _ _ _ _ _ w3293 _ _ _]
      tunnel: w1885 -> [_ _ _ _ _ _ _ _ _ _ _ _ _ _ _ _ _ _ _ _ _ _ _ _ _ _ _ _ _ _ _ _ _ _ _ _ _ _ _ _ _ _ _ _ _ _ _ _ _ _ _ _ _ _ _ _ _ _ _ _ _ _ _ _ _ _ _ _ _ _ _ _ _ _ _ _ _ _ _ _ _ w3305 _]
      frame "Timeout" {
        n1127 = call "Time Out Loop.vi"("error in (no error)"=w1889, "Data Cluster"=w1890) -> ("error out"=w1891:errorcluster)  [unwired: 9 in]
        n1128 = call "Trip Log and Trip Monitor.vi"("error in (no error)"=w1889, "main ref"=w1890) -> ()  [unwired: 9 in, 1 out]
      }
      frame "init" {
        (unwired) FALSE ("Value")
        # "Initialize - All initialization work should take place in this message, since other loops can potentially enqueue messages that execute immediately after this one."
        n1129 = Unbundle By Name(w1893) -> ("Loading.Warning"=w1896:refnum<vi>)
        n1130 = property class="TabCtl (strict)"(reference=w1896, "Visible"=FALSE) -> (reference out=w1894:refnum<vi>, error out=w1895:errorcluster)  [unwired: 1 in]
        n1131 = call-poly "Enqueue Message.vi"("error in (no error)"=w1935, "Message"="Init Other Loop", "Message Queue"=w1933) -> ("error out"=w1936:errorcluster)  [unwired: 7 in, 1 out]
        n1132 = Close Reference(reference=w1894, error in (no error)=w1895) -> ()  [unwired: 1 out]
        n1133 = Unbundle By Name(w1893) -> ("Loading.SSP 0.3"=w1925:refnum<vi>)
        n1134 = Unbundle By Name(w1893) -> ("Loading.SSP 0.5"=w1922:refnum<vi>)
        n1135 = Unbundle By Name(w1893) -> ("Loading.SSP 0.75"=w1917:refnum<vi>)
        n1136 = Unbundle By Name(w1893) -> ("Loading.Communication is established"=w1912:refnum<vi>)
        n1137 = Unbundle By Name(w1893) -> ("Motion Module.Set WTD"=w1905:refnum<vi>)
        n1138 = call "Read Config Unitest.vi"("error in (no error)"=w1936, "main ref"=w1893) -> ("error out"=w1931:errorcluster)  [unwired: 9 in]
        n1139 = Unbundle By Name(w1893) -> ("Motion Module.Wear Track Diameter"=w1899:refnum<vi>)
        n1140 = Unbundle By Name(w1893) -> ("PID.Ramp"=w1909:refnum<vi>)
        n1141 = call "Encrypt file path creation.vi"("error in (no error)"=w1931) -> ("error out"=w1930:errorcluster, "File Path"=w1929:path)  [unwired: 9 in]
        n1142 = property on="Property Node" class="Bool (strict)"(reference=w1922, "Visible"=FALSE) -> (reference out=w1920:refnum<vi>, error out=w1921:errorcluster)  [unwired: 1 in]
        n1143 = property on="Property Node" class="Bool (strict)"(reference=w1925, "Visible"=FALSE) -> (reference out=w1927:refnum<vi>, error out=w1926:errorcluster)  [unwired: 1 in]
        n1144 = property on="Property Node" class="Bool (strict)"(reference=w1917, "Visible"=FALSE) -> (reference out=w1919:refnum<vi>, error out=w1918:errorcluster)  [unwired: 1 in]
        n1145 = property on="Property Node" class="Bool (strict)"(reference=w1909, "Value"=FALSE) -> (reference out=w1911:refnum<vi>, error out=w1910:errorcluster)  [unwired: 1 in]
        n1146 = property on="Property Node" class="DigNum (strict)"(reference=w1899, "Value"=0.0) -> (reference out=w1898:refnum<vi>, error out=w1900:errorcluster)  [unwired: 1 in]
        n1147 = property on="Property Node" class="Bool (strict)"(reference=w1905, "Visible"=FALSE, "DisabledEnum"=T31."Disabled and Grayed Out" ("Disabled")) -> (reference out=w1902:refnum<vi>, error out=w1904:errorcluster)  [unwired: 1 in]
        n1148 = property on="Property Node" class="Bool (strict)"(reference=w1912, "Visible"=FALSE ("Value")) -> (reference out=w1914:refnum<vi>, error out=w1913:errorcluster)  [unwired: 1 in]
        n1149 = call "DATA ENCRYPT STRING FILE WRITE.vi"("file path (dialog if empty)"=w1929, "error in (no error)"=w1930, "User Action"="System Booted", "main ref"=w1893) -> ("error out"=w1932:errorcluster)  [unwired: 5 in, 1 out]
        n1150 = Close Reference(reference=w1920, error in (no error)=w1921) -> ()  [unwired: 1 out]
        n1151 = Close Reference(reference=w1927, error in (no error)=w1926) -> ()  [unwired: 1 out]
        n1152 = Close Reference(reference=w1919, error in (no error)=w1918) -> ()  [unwired: 1 out]
        n1153 = Close Reference(reference=w1911, error in (no error)=w1910) -> ()  [unwired: 1 out]
        n1154 = Close Reference(reference=w1898, error in (no error)=w1900) -> ()  [unwired: 1 out]
        n1155 = Close Reference(reference=w1902, error in (no error)=w1904) -> ()  [unwired: 1 out]
        n1156 = Close Reference(reference=w1914, error in (no error)=w1913) -> ()  [unwired: 1 out]
        n1157 = call "Reinitial Parameter After Test.vi"("error in (no error)"=w1932, "main ref"=w1893) -> ("error out"=w1906:errorcluster)  [unwired: 9 in]
        n1158 = local write "HEAVE ENABLE"(FALSE ("HEAVE ENABLE")) -> ()
      }
      frame "Init Other Loop" {
        n1159 = disable-structure shown="Disabled" {
          disable-tunnel: [w1942 w1943] -> w1939
          disable-tunnel: w1938 -> [w1941 _]
          disable-tunnel: w1937 -> [w1940 w1943]
          frame Disabled {
            n1160 = call "SET LOAD PARAMETERS.vi"("error in (no error)"=w1940, "main ref"=w1941) -> ("error out"=w1942:errorcluster)  [unwired: 9 in]
          }
          frame Enabled {
          }
        }
      }
      frame "Service Save" {
        n1161 = call "Write Config Unitest.vi"("error in (no error)"=w1947, "main ref"=w1946) -> ("error out"=w1952:errorcluster)  [unwired: 9 in]
        n1162 = call "Stall Data Flow.vim"("value in"=w1952, "milliseconds to wait"=u32 2000) -> ("value out"=w1951:errorcluster)  [unwired: 1 out]
        n1163 = call "Read Config Unitest.vi"("error in (no error)"=w1951, "main ref"=w1946) -> ("error out"=w1949:errorcluster)  [unwired: 9 in]
        n1164 = local write "SAVE  2"(FALSE ("SAVE  2")) -> ()
        n1165 = call "DATA ENCRYPT STRING FILE WRITE.vi"("error in (no error)"=w1949, "User Action"="Service Parameter Saved", "main ref"=w1946) -> ("error out"=w1948:errorcluster)  [unwired: 6 in, 1 out]
      }
      frame "HOME" {
        n1166 = call "DATA ENCRYPT STRING FILE WRITE.vi"("error in (no error)"=w1968, "User Action"="User Pressed Home", "main ref"=w1954) -> ("error out"=w1964:errorcluster)  [unwired: 6 in, 1 out]
        n1167 = Unbundle By Name(w1954) -> ("Main Home Screen.MainPage"=w1959:refnum<vi>)
        n1168 = Unbundle By Name(w1954) -> ("Main Home Screen.Home"=w1967:refnum<vi>)
        n1169 = Unbundle By Name(w1954) -> ("Main Home Screen.GUI"=w1957:refnum<vi>)
        n1170 = property on="Property Node" class="Bool (strict)"(reference=w1967, error in=w1964, "Value"=FALSE) -> (reference out=w1965:refnum<vi>, error out=w1966:errorcluster)
        n1171 = property on="Property Node" class="TabCtl (strict)"(reference=w1959, "Value"=T15."HOME") -> (reference out=w1961:refnum<vi>, error out=w1960:errorcluster)  [unwired: 1 in]
        n1172 = property on="Property Node" class="TabCtl (strict)"(reference=w1957, "Value"=T14."Setup") -> (reference out=w1955:refnum<vi>, error out=w1956:errorcluster)  [unwired: 1 in]
        n1173 = Close Reference(reference=w1965, error in (no error)=w1966) -> (error out=w1963:errorcluster)
        n1174 = Close Reference(reference=w1961, error in (no error)=w1960) -> ()  [unwired: 1 out]
        n1175 = Close Reference(reference=w1955, error in (no error)=w1956) -> ()  [unwired: 1 out]
      }
      frame "Platform Setting" {
        n1176 = call "DATA ENCRYPT STRING FILE WRITE.vi"("error in (no error)"=w1985, "User Action"="User Pressed Platform Setting", "main ref"=w1971) -> ("error out"=w1981:errorcluster)  [unwired: 6 in, 1 out]
        n1177 = Unbundle By Name(w1971) -> ("Main Home Screen.Platform Settings"=w1984:refnum<vi>)
        n1178 = Unbundle By Name(w1971) -> ("Main Home Screen.MainPage"=w1976:refnum<vi>)
        n1179 = Unbundle By Name(w1971) -> ("Main Home Screen.GUI"=w1974:refnum<vi>)
        n1180 = property on="Property Node" class="TabCtl (strict)"(reference=w1976, "Value"=T15."PlatformSetting") -> (reference out=w1978:refnum<vi>, error out=w1977:errorcluster)  [unwired: 1 in]
        n1181 = property on="Property Node" class="TabCtl (strict)"(reference=w1974, "Value"=T14."Setup") -> (reference out=w1972:refnum<vi>, error out=w1973:errorcluster)  [unwired: 1 in]
        n1182 = property on="Property Node" class="Bool (strict)"(reference=w1984, error in=w1981, "Value"=FALSE) -> (reference out=w1982:refnum<vi>, error out=w1983:errorcluster)
        n1183 = Close Reference(reference=w1978, error in (no error)=w1977) -> ()  [unwired: 1 out]
        n1184 = Close Reference(reference=w1972, error in (no error)=w1973) -> ()  [unwired: 1 out]
        n1185 = Close Reference(reference=w1982, error in (no error)=w1983) -> (error out=w1980:errorcluster)
      }
      frame "Configure" {
        n1186 = call "DATA ENCRYPT STRING FILE WRITE.vi"("error in (no error)"=w2002, "User Action"="User Pressed Configure", "main ref"=w1988) -> ("error out"=w1998:errorcluster)  [unwired: 6 in, 1 out]
        n1187 = Unbundle By Name(w1988) -> ("Main Home Screen.Configure"=w2001:refnum<vi>)
        n1188 = Unbundle By Name(w1988) -> ("Main Home Screen.MainPage"=w1993:refnum<vi>)
        n1189 = Unbundle By Name(w1988) -> ("Main Home Screen.GUI"=w1991:refnum<vi>)
        n1190 = property on="Property Node" class="Bool (strict)"(reference=w2001, error in=w1998, "Value"=FALSE) -> (reference out=w1999:refnum<vi>, error out=w2000:errorcluster)
        n1191 = property on="Property Node" class="TabCtl (strict)"(reference=w1993, "Value"=T15."Details") -> (reference out=w1995:refnum<vi>, error out=w1994:errorcluster)  [unwired: 1 in]
        n1192 = property on="Property Node" class="TabCtl (strict)"(reference=w1991, "Value"=T14."Setup") -> (reference out=w1989:refnum<vi>, error out=w1990:errorcluster)  [unwired: 1 in]
        n1193 = Close Reference(reference=w1999, error in (no error)=w2000) -> (error out=w1997:errorcluster)
        n1194 = Close Reference(reference=w1995, error in (no error)=w1994) -> ()  [unwired: 1 out]
        n1195 = Close Reference(reference=w1989, error in (no error)=w1990) -> ()  [unwired: 1 out]
      }
      frame "Analysis" {
        n1196 = call "DATA ENCRYPT STRING FILE WRITE.vi"("error in (no error)"=w2019, "User Action"="User Pressed Analysis", "main ref"=w2005) -> ("error out"=w2015:errorcluster)  [unwired: 6 in, 1 out]
        n1197 = Unbundle By Name(w2005) -> ("Main Home Screen.MainPage"=w2010:refnum<vi>)
        n1198 = Unbundle By Name(w2005) -> ("Main Home Screen.Analysis"=w2018:refnum<vi>)
        n1199 = Unbundle By Name(w2005) -> ("Main Home Screen.GUI"=w2008:refnum<vi>)
        n1200 = property on="Property Node" class="Bool (strict)"(reference=w2018, error in=w2015, "Value"=FALSE) -> (reference out=w2016:refnum<vi>, error out=w2017:errorcluster)
        n1201 = property on="Property Node" class="TabCtl (strict)"(reference=w2010, "Value"=T15."Analysis") -> (reference out=w2012:refnum<vi>, error out=w2011:errorcluster)  [unwired: 1 in]
        n1202 = property on="Property Node" class="TabCtl (strict)"(reference=w2008, "Value"=T14."Setup") -> (reference out=w2006:refnum<vi>, error out=w2007:errorcluster)  [unwired: 1 in]
        n1203 = Close Reference(reference=w2016, error in (no error)=w2017) -> (error out=w2014:errorcluster)
        n1204 = Close Reference(reference=w2012, error in (no error)=w2011) -> ()  [unwired: 1 out]
        n1205 = Close Reference(reference=w2006, error in (no error)=w2007) -> ()  [unwired: 1 out]
      }
      frame "service 2" {
        n1206 = call "DATA ENCRYPT STRING FILE WRITE.vi"("error in (no error)"=w2040, "User Action"="User Pressed service", "main ref"=w2023) -> ("error out"=w2036:errorcluster)  [unwired: 6 in, 1 out]
        n1207 = Unbundle By Name(w2023) -> ("Main Screen.Main Screen Tab"=w2024:refnum<vi>)
        n1208 = Unbundle By Name(w2023) -> ("Main Home Screen.MainPage"=w2031:refnum<vi>)
        n1209 = Unbundle By Name(w2023) -> ("Main Home Screen.Analysis"=w2039:refnum<vi>)
        n1210 = Unbundle By Name(w2023) -> ("Main Home Screen.GUI"=w2029:refnum<vi>)
        n1211 = property on="Property Node" class="Bool (strict)"(reference=w2039, error in=w2036, "Value"=FALSE) -> (reference out=w2037:refnum<vi>, error out=w2038:errorcluster)
        n1212 = property on="Property Node" class="TabCtl (strict)"(reference=w2031, "Value"=T15."HOME") -> (reference out=w2033:refnum<vi>, error out=w2032:errorcluster)  [unwired: 1 in]
        n1213 = property on="Property Node" class="TabCtl (strict)"(reference=w2029, "Value"=T14."Begin") -> (reference out=w2027:refnum<vi>, error out=w2028:errorcluster)  [unwired: 1 in]
        n1214 = property on="Property Node" class="TabCtl (strict)"(reference=w2024, "Value"=T18."About") -> (reference out=w2021:refnum<vi>, error out=w2025:errorcluster)  [unwired: 1 in]
        n1215 = Close Reference(reference=w2037, error in (no error)=w2038) -> (error out=w2035:errorcluster)
        n1216 = Close Reference(reference=w2033, error in (no error)=w2032) -> ()  [unwired: 1 out]
        n1217 = Close Reference(reference=w2027, error in (no error)=w2028) -> ()  [unwired: 1 out]
        n1218 = Close Reference(reference=w2021, error in (no error)=w2025) -> ()  [unwired: 1 out]
      }
      frame "Auto" {
        n1219 = call "DATA ENCRYPT STRING FILE WRITE.vi"("error in (no error)"=w2053, "User Action"="User Pressed Auto File Name", "main ref"=w2043) -> ("error out"=w2050:errorcluster)  [unwired: 6 in, 1 out]
        n1220 = Get Date/Time In Seconds() -> (seconds since 1Jan1904=w2051:timestamp)
        n1221 = Format Into String(format string="%<%I_%M_%S_%p_%d_%B_%Y>T", error in=w2050, w2051) -> (resulting string=w2044:string, error out=w2046:errorcluster)  [unwired: 1 in]
        n1222 = local write "Auto"(FALSE ("Auto")) -> ()
        n1223 = Unbundle By Name(w2043) -> ("Config Screen.FILE"=w2049:refnum<vi>)
        n1224 = property on="Property Node" class="Str"(reference=w2049, error in=w2046, "Value"=w2044) -> (reference out=w2047:refnum<vi>, error out=w2048:errorcluster)
        n1225 = Close Reference(reference=w2047, error in (no error)=w2048) -> (error out=w2045:errorcluster)
      }
      frame "Select Load Head" {
        n1226 = call "Reinitial Parameter.vi"("error in (no error)"=w2058, "Data Cluster"=w2055) -> ("error out"=w2057:errorcluster)  [unwired: 9 in]
        n1227 = call "FILE NAME RECHECK.vi"("error in (no error)"=w2057, "main ref"=w2055) -> ("error out"=w2056:errorcluster)  [unwired: 9 in]
      }
      frame "com 3" {
        n1228 = call "DATA ENCRYPT STRING FILE WRITE.vi"("error in (no error)"=w2063, "User Action"="User Pressed Check Load Communication", "main ref"=w2060) -> ("error out"=w2062:errorcluster)  [unwired: 6 in, 1 out]
        n1229 = call "SET LOAD PARAMETERS.vi"("error in (no error)"=w2062, "main ref"=w2060) -> ("error out"=w2061:errorcluster)  [unwired: 9 in]
        n1230 = local write "com 3"(FALSE ("com 3")) -> ()
      }
      frame "ZeroAll" {
        n1231 = call "DATA ENCRYPT STRING FILE WRITE.vi"("error in (no error)"=w2075, "User Action"="User Pressed Zero All", "main ref"=w2068) -> ("error out"=w2074:errorcluster)  [unwired: 6 in, 1 out]
        n1232 = call "NEW Load Cell FGV.vi"("Enum - Menu"=Load_cell_Enum."Set Zero", "error in (no error)"=w2074, "main ref"=w2068) -> ("error out"=w2073:errorcluster)  [unwired: 7 in, 1 out]
        n1233 = Unbundle By Name(w2068) -> ("Loading Com Port.Load Cell Link"=w2071:refnum<vi>)
        n1234 = Bundle By Name(cluster=T5 {"model"="", "SN"=0, "Sensor IP"="", "Port"=0, "Acq Delay (ms)"=0.0, "Burst Delay (ms)"=0.0, "Save Dwell"=0.0, "FORCE (N)"=[], "TORQUE (N-m)"=[], "ft_data"=[], "running_flag"=FALSE, "ClearAll"=FALSE, "ZeroAll"=FALSE} ("Value"), "ZeroAll"=FALSE) -> (w2066:T5)
        n1235 = property on="Property Node" class="Clust (strict)"(reference=w2071, "Value"=w2066) -> (reference out=w2069:refnum<vi>, error out=w2070:errorcluster)  [unwired: 1 in]
        n1236 = Close Reference(reference=w2069, error in (no error)=w2070) -> ()  [unwired: 1 out]
      }
      frame "Loading Mode" {
        n1237 = Unbundle By Name(w2079) -> ("Loading.Loading Mode"=w2081:refnum<vi>)
        n1238 = property on="Property Node" class="Ring (strict)"(reference=w2081, error in=w2080) -> (reference out=w2083:refnum<vi>, error out=w2082:errorcluster, "Value"=w2077:u16)
        n1239 = Close Reference(reference=w2083, error in (no error)=w2082) -> (error out=w2078:errorcluster)
        n1240 = case shown="1" w2077 {
          tunnel: [w2098 w2115 w2127 w2139] -> w2084
          tunnel: w2079 -> [w2085 w2101 w2119 w2131]
          tunnel: w2078 -> [w2099 w2114 w2126 w2138]
          frame 0, Default {
            n1241 = Unbundle By Name(w2085) -> ("Loading.Enter the Loading Rate (N/min)"=w2092:refnum<vi>)
            n1242 = Unbundle By Name(w2085) -> ("Loading.Load Selection"=w2095:refnum<vi>)
            n1243 = Unbundle By Name(w2085) -> ("Loading.Enter the Final Load (N)"=w2087:refnum<vi>)
            n1244 = property on="Property Node" class="TabCtl (strict)"(reference=w2095, "Value"=T16."Constant") -> (reference out=w2097:refnum<vi>, error out=w2096:errorcluster)  [unwired: 1 in]
            n1245 = property on="Property Node" class="DigNum (strict)"(reference=w2092, "DisabledEnum"=T31."Disabled and Grayed Out" ("Disabled")) -> (reference out=w2091:refnum<vi>, error out=w2093:errorcluster)  [unwired: 1 in]
            n1246 = property on="Property Node" class="DigNum (strict)"(reference=w2087, "DisabledEnum"=T31."Disabled and Grayed Out" ("Disabled")) -> (reference out=w2088:refnum<vi>, error out=w2086:errorcluster)  [unwired: 1 in]
            n1247 = call "DATA ENCRYPT STRING FILE WRITE.vi"("error in (no error)"=w2099, "User Action"="User selected Constant Mode", "main ref"=w2085) -> ("error out"=w2098:errorcluster)  [unwired: 6 in, 1 out]
            n1248 = Close Reference(reference=w2097, error in (no error)=w2096) -> ()  [unwired: 1 out]
            n1249 = Close Reference(reference=w2091, error in (no error)=w2093) -> ()  [unwired: 1 out]
            n1250 = Close Reference(reference=w2088, error in (no error)=w2086) -> ()  [unwired: 1 out]
          }
          frame 1 {
            n1251 = Unbundle By Name(w2101) -> ("Loading.Enter the Loading Rate (N/min)"=w2112:refnum<vi>)
            n1252 = Unbundle By Name(w2101) -> ("Loading.Enter the Final Load (N)"=w2107:refnum<vi>)
            n1253 = Unbundle By Name(w2101) -> ("Loading.Load Selection"=w2103:refnum<vi>)
            n1254 = property on="Property Node" class="TabCtl (strict)"(reference=w2103, "Value"=T16."Constant") -> (reference out=w2105:refnum<vi>, error out=w2104:errorcluster)  [unwired: 1 in]
            n1255 = property on="Property Node" class="DigNum (strict)"(reference=w2112, "DisabledEnum"=T31."Enabled" ("Disabled")) -> (reference out=w2111:refnum<vi>, error out=w2113:errorcluster)  [unwired: 1 in]
            n1256 = property on="Property Node" class="DigNum (strict)"(reference=w2107, "DisabledEnum"=T31."Enabled" ("Disabled")) -> (reference out=w2108:refnum<vi>, error out=w2106:errorcluster)  [unwired: 1 in]
            n1257 = call "DATA ENCRYPT STRING FILE WRITE.vi"("error in (no error)"=w2114, "User Action"="User selected Ramp Mode", "main ref"=w2101) -> ("error out"=w2115:errorcluster)  [unwired: 6 in, 1 out]
            n1258 = Close Reference(reference=w2105, error in (no error)=w2104) -> ()  [unwired: 1 out]
            n1259 = Close Reference(reference=w2111, error in (no error)=w2113) -> ()  [unwired: 1 out]
            n1260 = Close Reference(reference=w2108, error in (no error)=w2106) -> ()  [unwired: 1 out]
          }
          frame 2 {
            n1261 = Unbundle By Name(w2119) -> ("Loading.Load Selection"=w2123:refnum<vi>)
            n1262 = Unbundle By Name(w2119) -> ("Loading.Warning 2"=w2121:refnum<vi>)
            n1263 = property on="Property Node" class="TabCtl (strict)"(reference=w2123, "Value"=T16."Step") -> (reference out=w2125:refnum<vi>, error out=w2124:errorcluster)  [unwired: 1 in]
            n1264 = property on="Property Node" class="Bool (strict)"(reference=w2121, "Visible"=FALSE) -> (reference out=w2117:refnum<vi>, error out=w2120:errorcluster)  [unwired: 1 in]
            n1265 = call "DATA ENCRYPT STRING FILE WRITE.vi"("error in (no error)"=w2126, "User Action"="User selected Step Mode", "main ref"=w2119) -> ("error out"=w2127:errorcluster)  [unwired: 6 in, 1 out]
            n1266 = Close Reference(reference=w2125, error in (no error)=w2124) -> ()  [unwired: 1 out]
            n1267 = Close Reference(reference=w2117, error in (no error)=w2120) -> ()  [unwired: 1 out]
          }
          frame 3 {
            n1268 = Unbundle By Name(w2131) -> ("Loading.Load Selection"=w2135:refnum<vi>)
            n1269 = Unbundle By Name(w2131) -> ("Loading.Warning 2"=w2133:refnum<vi>)
            n1270 = property on="Property Node" class="TabCtl (strict)"(reference=w2135, "Value"=T16."Indentation") -> (reference out=w2137:refnum<vi>, error out=w2136:errorcluster)  [unwired: 1 in]
            n1271 = property on="Property Node" class="Bool (strict)"(reference=w2133, "Visible"=FALSE) -> (reference out=w2129:refnum<vi>, error out=w2132:errorcluster)  [unwired: 1 in]
            n1272 = call "DATA ENCRYPT STRING FILE WRITE.vi"("error in (no error)"=w2138, "User Action"="User selected Indentation Mode", "main ref"=w2131) -> ("error out"=w2139:errorcluster)  [unwired: 6 in, 1 out]
            n1273 = Close Reference(reference=w2137, error in (no error)=w2136) -> ()  [unwired: 1 out]
            n1274 = Close Reference(reference=w2129, error in (no error)=w2132) -> ()  [unwired: 1 out]
          }
        }
      }
      frame "SSP 0.3" {
        n1275 = Unbundle By Name(w2143) -> ("Loading.SSP 0.3"=w2146:refnum<vi>)
        n1276 = property on="Property Node" class="Bool (strict)"(reference=w2146, error in=w2145) -> (reference out=w2148:refnum<vi>, error out=w2147:errorcluster, "Value"=w2144:bool)
        n1277 = Close Reference(reference=w2148, error in (no error)=w2147) -> (error out=w2142:errorcluster)
        n1278 = case shown="True" w2144 {
          tunnel: w2143 -> [_ w2150]
          tunnel: w2142 -> [w2149 w2158]
          tunnel: [w2149 w2157] -> w2141
          frame False {
          }
          frame True {
            w2160 = FALSE ("Value")
            n1279 = Unbundle By Name(w2150) -> ("Loading.Enter the Load  (N)"=w2156:refnum<vi>)
            n1280 = Unbundle By Name(w2150) -> ("Loading.SSP 0.75"=w2161:refnum<vi>)
            n1281 = Unbundle By Name(w2150) -> ("Loading.SSP 0.5"=w2166:refnum<vi>)
            n1282 = property on="Property Node" class="Bool (strict)"(reference=w2161, "Value"=w2160) -> (reference out=w2163:refnum<vi>, error out=w2162:errorcluster)  [unwired: 1 in]
            n1283 = property on="Property Node" class="Bool (strict)"(reference=w2166, "Value"=w2160) -> (reference out=w2164:refnum<vi>, error out=w2165:errorcluster)  [unwired: 1 in]
            n1284 = property on="Property Node" class="DigNum (strict)"(reference=w2156, "Minimum"=2.0 ("Data Entry Limits:Minimum"), "Maximum"=50.0 ("Data Entry Limits:Maximum"), "Increment"=0.1 ("Data Entry Limits:Increment")) -> (reference out=w2154:refnum<vi>, error out=w2155:errorcluster)  [unwired: 1 in]
            n1285 = call "DATA ENCRYPT STRING FILE WRITE.vi"("error in (no error)"=w2158, "User Action"="User selected 0.3 SSP", "main ref"=w2150) -> ("error out"=w2157:errorcluster)  [unwired: 6 in, 1 out]
            n1286 = Close Reference(reference=w2163, error in (no error)=w2162) -> ()  [unwired: 1 out]
            n1287 = Close Reference(reference=w2164, error in (no error)=w2165) -> ()  [unwired: 1 out]
            n1288 = Close Reference(reference=w2154, error in (no error)=w2155) -> ()  [unwired: 1 out]
          }
        }
      }
      frame "SSP 0.5" {
        n1289 = Unbundle By Name(w2169) -> ("Loading.SSP 0.5"=w2172:refnum<vi>)
        n1290 = property on="Property Node" class="Bool (strict)"(reference=w2172, error in=w2171) -> (reference out=w2174:refnum<vi>, error out=w2173:errorcluster, "Value"=w2170:bool)
        n1291 = Close Reference(reference=w2174, error in (no error)=w2173) -> (error out=w2168:errorcluster)
        n1292 = case shown="True" w2170 {
          tunnel: w2169 -> [_ w2176]
          tunnel: w2168 -> [w2175 w2184]
          tunnel: [w2175 w2183] -> w2167
          frame False {
          }
          frame True {
            w2186 = FALSE ("Value")
            n1293 = Unbundle By Name(w2176) -> ("Loading.Enter the Load  (N)"=w2182:refnum<vi>)
            n1294 = Unbundle By Name(w2176) -> ("Loading.SSP 0.75"=w2192:refnum<vi>)
            n1295 = Unbundle By Name(w2176) -> ("Loading.SSP 0.3"=w2187:refnum<vi>)
            n1296 = property on="Property Node" class="Bool (strict)"(reference=w2187, "Value"=w2186) -> (reference out=w2189:refnum<vi>, error out=w2188:errorcluster)  [unwired: 1 in]
            n1297 = property on="Property Node" class="Bool (strict)"(reference=w2192, "Value"=w2186) -> (reference out=w2190:refnum<vi>, error out=w2191:errorcluster)  [unwired: 1 in]
            n1298 = property on="Property Node" class="DigNum (strict)"(reference=w2182, "Minimum"=2.0 ("Data Entry Limits:Minimum"), "Maximum"=200.0 ("Data Entry Limits:Maximum"), "Increment"=0.1 ("Data Entry Limits:Increment")) -> (reference out=w2180:refnum<vi>, error out=w2181:errorcluster)  [unwired: 1 in]
            n1299 = call "DATA ENCRYPT STRING FILE WRITE.vi"("error in (no error)"=w2184, "User Action"="User selected 0.5 SSP", "main ref"=w2176) -> ("error out"=w2183:errorcluster)  [unwired: 6 in, 1 out]
            n1300 = Close Reference(reference=w2189, error in (no error)=w2188) -> ()  [unwired: 1 out]
            n1301 = Close Reference(reference=w2190, error in (no error)=w2191) -> ()  [unwired: 1 out]
            n1302 = Close Reference(reference=w2180, error in (no error)=w2181) -> ()  [unwired: 1 out]
          }
        }
      }
      frame "SSP 0.75" {
        n1303 = Unbundle By Name(w2195) -> ("Loading.SSP 0.75"=w2198:refnum<vi>)
        n1304 = property on="Property Node" class="Bool (strict)"(reference=w2198, error in=w2197) -> (reference out=w2200:refnum<vi>, error out=w2199:errorcluster, "Value"=w2196:bool)
        n1305 = Close Reference(reference=w2200, error in (no error)=w2199) -> (error out=w2194:errorcluster)
        n1306 = case shown="True" w2196 {
          tunnel: w2195 -> [_ w2202]
          tunnel: w2194 -> [w2201 w2210]
          tunnel: [w2201 w2209] -> w2193
          frame False {
          }
          frame True {
            w2212 = FALSE ("Value")
            n1307 = Unbundle By Name(w2202) -> ("Loading.SSP 0.3"=w2213:refnum<vi>)
            n1308 = Unbundle By Name(w2202) -> ("Loading.SSP 0.5"=w2218:refnum<vi>)
            n1309 = Unbundle By Name(w2202) -> ("Loading.Enter the Load  (N)"=w2208:refnum<vi>)
            n1310 = property on="Property Node" class="Bool (strict)"(reference=w2213, "Value"=w2212) -> (reference out=w2215:refnum<vi>, error out=w2214:errorcluster)  [unwired: 1 in]
            n1311 = property on="Property Node" class="Bool (strict)"(reference=w2218, "Value"=w2212) -> (reference out=w2216:refnum<vi>, error out=w2217:errorcluster)  [unwired: 1 in]
            n1312 = property on="Property Node" class="DigNum (strict)"(reference=w2208, "Minimum"=200.0 ("Data Entry Limits:Minimum"), "Maximum"=500.0 ("Data Entry Limits:Maximum"), "Increment"=0.1 ("Data Entry Limits:Increment")) -> (reference out=w2206:refnum<vi>, error out=w2207:errorcluster)  [unwired: 1 in]
            n1313 = call "DATA ENCRYPT STRING FILE WRITE.vi"("error in (no error)"=w2210, "User Action"="User selected 0.75 SSP", "main ref"=w2202) -> ("error out"=w2209:errorcluster)  [unwired: 6 in, 1 out]
            n1314 = Close Reference(reference=w2215, error in (no error)=w2214) -> ()  [unwired: 1 out]
            n1315 = Close Reference(reference=w2216, error in (no error)=w2217) -> ()  [unwired: 1 out]
            n1316 = Close Reference(reference=w2206, error in (no error)=w2207) -> ()  [unwired: 1 out]
          }
        }
      }
      frame "LHBack" {
        # "Back to Configure"
        n1317 = Unbundle By Name(w2220) -> ("Main Home Screen.GUI"=w2229:refnum<vi>)
        n1318 = Unbundle By Name(w2220) -> ("Main Home Screen.MainPage"=w2225:refnum<vi>)
        n1319 = Unbundle By Name(w2220) -> ("Loading.LHBack"=w2223:refnum<vi>)
        n1320 = property on="Property Node" class="TabCtl (strict)"(reference=w2225, "Value"=T15."HOME") -> (reference out=w2227:refnum<vi>, error out=w2226:errorcluster)  [unwired: 1 in]
        n1321 = property on="Property Node" class="Bool (strict)"(reference=w2223, "Value"=FALSE) -> (reference out=w2221:refnum<vi>, error out=w2222:errorcluster)  [unwired: 1 in]
        n1322 = property on="Property Node" class="TabCtl (strict)"(reference=w2229, "Value"=T14."Setup") -> (reference out=w2231:refnum<vi>, error out=w2230:errorcluster)  [unwired: 1 in]
        n1323 = Close Reference(reference=w2227, error in (no error)=w2226) -> ()  [unwired: 1 out]
        n1324 = Close Reference(reference=w2221, error in (no error)=w2222) -> ()  [unwired: 1 out]
        n1325 = Close Reference(reference=w2231, error in (no error)=w2230) -> ()  [unwired: 1 out]
        n1326 = call "DATA ENCRYPT STRING FILE WRITE.vi"("error in (no error)"=w2232, "User Action"="User selected Back to Configure", "main ref"=w2220) -> ("error out"=w2233:errorcluster)  [unwired: 6 in, 1 out]
      }
      frame "MMBack" {
        # "Back to Configure"
        n1327 = Unbundle By Name(w2235) -> ("Motion Module.MMBack"=w2239:refnum<vi>)
        n1328 = Unbundle By Name(w2235) -> ("Main Home Screen.GUI"=w2245:refnum<vi>)
        n1329 = Unbundle By Name(w2235) -> ("Main Home Screen.MainPage"=w2241:refnum<vi>)
        n1330 = property on="Property Node" class="Bool (strict)"(reference=w2239, "Value"=FALSE) -> (reference out=w2237:refnum<vi>, error out=w2238:errorcluster)  [unwired: 1 in]
        n1331 = property on="Property Node" class="TabCtl (strict)"(reference=w2241, "Value"=T15."HOME") -> (reference out=w2243:refnum<vi>, error out=w2242:errorcluster)  [unwired: 1 in]
        n1332 = property on="Property Node" class="TabCtl (strict)"(reference=w2245, "Value"=T14."Load Head") -> (reference out=w2247:refnum<vi>, error out=w2246:errorcluster)  [unwired: 1 in]
        n1333 = Close Reference(reference=w2237, error in (no error)=w2238) -> ()  [unwired: 1 out]
        n1334 = Close Reference(reference=w2243, error in (no error)=w2242) -> ()  [unwired: 1 out]
        n1335 = Close Reference(reference=w2247, error in (no error)=w2246) -> ()  [unwired: 1 out]
        n1336 = call "DATA ENCRYPT STRING FILE WRITE.vi"("error in (no error)"=w2248, "User Action"="User selected Back to Load Selection", "main ref"=w2235) -> ("error out"=w2249:errorcluster)  [unwired: 6 in, 1 out]
      }
      frame "LHNext" {
        w2285 = FALSE ("Visible")
        n1337 = Unbundle By Name(w2251) -> ("Motion Module.HomeRot"=w2291:refnum<vi>)
        n1338 = Unbundle By Name(w2251) -> ("Motion Module.HomeScratch"=w2286:refnum<vi>)
        n1339 = Unbundle By Name(w2251) -> ("Motion Module.PlaceModule"=w2284:refnum<vi>)
        n1340 = Unbundle By Name(w2251) -> ("Motion Module.Motion Mode:"=w2277:refnum<vi>)
        n1341 = Unbundle By Name(w2251) -> ("Motion Module.Motion Direction:  3"=w2276:refnum<vi>)
        n1342 = Unbundle By Name(w2251) -> ("Motion Module.Wear Track Diameter (mm)"=w2270:refnum<vi>)
        n1343 = Unbundle By Name(w2251) -> ("Motion Module.Set WTD"=w2267:refnum<vi>)
        n1344 = Unbundle By Name(w2251) -> ("Motion Module.Rotary Module Selection"=w2261:refnum<vi>)
        n1345 = call "DATA ENCRYPT STRING FILE WRITE.vi"("error in (no error)"=w2300, "User Action"="User selected Select Module", "main ref"=w2251) -> ("error out"=w2264:errorcluster)  [unwired: 6 in, 1 out]
        n1346 = property on="Property Node" class="TabCtl (strict)"(reference=w2261, "Visible"=FALSE) -> (reference out=w2260:refnum<vi>, error out=w2262:errorcluster)  [unwired: 1 in]
        n1347 = property on="Property Node" class="Bool (strict)"(reference=w2291, error in=w2264, "Visible"=w2285) -> (reference out=w2289:refnum<vi>, error out=w2290:errorcluster)
        n1348 = property on="Property Node" class="Bool (strict)"(reference=w2286, error in=w2264, "Visible"=w2285) -> (reference out=w2288:refnum<vi>, error out=w2287:errorcluster)
        n1349 = property on="Property Node" class="Bool (strict)"(reference=w2284, error in=w2264, "Visible"=TRUE) -> (reference out=w2282:refnum<vi>, error out=w2283:errorcluster)
        n1350 = property on="Property Node" class="Ring (strict)"(reference=w2277, error in=w2264, "Visible"=FALSE) -> (reference out=w2279:refnum<vi>, error out=w2278:errorcluster)
        n1351 = property on="Property Node" class="Ring (strict)"(reference=w2276, error in=w2264, "Visible"=FALSE) -> (reference out=w2273:refnum<vi>, error out=w2275:errorcluster)
        n1352 = property on="Property Node" class="DigNum (strict)"(reference=w2270, "Visible"=FALSE) -> (reference out=w2269:refnum<vi>, error out=w2271:errorcluster)  [unwired: 1 in]
        n1353 = property on="Property Node" class="Bool (strict)"(reference=w2267, "Visible"=FALSE) -> (reference out=w2268:refnum<vi>, error out=w2266:errorcluster)  [unwired: 1 in]
        n1354 = Close Reference(reference=w2289, error in (no error)=w2290) -> ()  [unwired: 1 out]
        n1355 = Close Reference(reference=w2288, error in (no error)=w2287) -> ()  [unwired: 1 out]
        n1356 = Close Reference(reference=w2282, error in (no error)=w2283) -> ()  [unwired: 1 out]
        n1357 = Close Reference(reference=w2279, error in (no error)=w2278) -> ()  [unwired: 1 out]
        n1358 = Close Reference(reference=w2273, error in (no error)=w2275) -> ()  [unwired: 1 out]
        n1359 = Close Reference(reference=w2269, error in (no error)=w2271) -> ()  [unwired: 1 out]
        n1360 = Close Reference(reference=w2260, error in (no error)=w2262) -> ()  [unwired: 1 out]
        n1361 = Close Reference(reference=w2268, error in (no error)=w2266) -> ()  [unwired: 1 out]
        n1362 = Unbundle By Name(w2251) -> ("Motion Module.M3 Image"=w2259:refnum<vi>)
        n1363 = Unbundle By Name(w2251) -> ("Main Home Screen.GUI"=w2297:refnum<vi>)
        n1364 = Unbundle By Name(w2251) -> ("Main Home Screen.MainPage"=w2293:refnum<vi>)
        n1365 = Unbundle By Name(w2251) -> ("Loading.LHNext"=w2255:refnum<vi>)
        n1366 = property on="Property Node" class="TabCtl (strict)"(reference=w2259, "Value"=enum32{"Page 1", "Page 2"}."Page 2") -> (reference out=w2257:refnum<vi>, error out=w2258:errorcluster)  [unwired: 1 in]
        n1367 = property on="Property Node" class="TabCtl (strict)"(reference=w2293, "Value"=T15."HOME") -> (reference out=w2295:refnum<vi>, error out=w2294:errorcluster)  [unwired: 1 in]
        n1368 = property on="Property Node" class="TabCtl (strict)"(reference=w2297, "Value"=T14."Motion Module") -> (reference out=w2299:refnum<vi>, error out=w2298:errorcluster)  [unwired: 1 in]
        n1369 = property on="Property Node" class="Bool (strict)"(reference=w2255, "Value"=FALSE ("Visible")) -> (reference out=w2252:refnum<vi>, error out=w2254:errorcluster)  [unwired: 1 in]
        n1370 = Close Reference(reference=w2257, error in (no error)=w2258) -> ()  [unwired: 1 out]
        n1371 = Close Reference(reference=w2252, error in (no error)=w2254) -> ()  [unwired: 1 out]
        n1372 = Close Reference(reference=w2295, error in (no error)=w2294) -> ()  [unwired: 1 out]
        n1373 = Close Reference(reference=w2299, error in (no error)=w2298) -> ()  [unwired: 1 out]
      }
      frame "Rot Ver" {
        n1374 = call "Rotory Module Selection.vi"("error in (no error)"=w2304, "Data Cluster"=w2302) -> ("error out"=w2303:errorcluster)  [unwired: 9 in]
      }
      frame "Scratch" {
        n1375 = call "Scratch Module Selection.vi"("error in (no error)"=w2307, "Data Cluster"=w2305) -> ("error out"=w2306:errorcluster)  [unwired: 9 in]
      }
      frame "Traction" {
        n1376 = call "TractionModule Selection.vi"("error in (no error)"=w2310, "Data Cluster"=w2308) -> ("error out"=w2309:errorcluster)  [unwired: 9 in]
      }
      frame "Motion Mode:" {
        n1377 = Unbundle By Name(w2311) -> ("Motion Module.Motion Mode:"=w2313:refnum<vi>)
        n1378 = property on="Property Node" class="Ring (strict)"(reference=w2313) -> (reference out=w2315:refnum<vi>, error out=w2314:errorcluster, "Value"=w2312:u16)  [unwired: 1 in]
        n1379 = Close Reference(reference=w2315, error in (no error)=w2314) -> ()  [unwired: 1 out]
        n1380 = case shown="3" w2312 {
          tunnel: w2317 -> [w2334 w2351 w2368 w2385]
          tunnel: [w2333 w2350 w2367 w2384] -> w2316
          tunnel: w2311 -> [w2332 w2349 w2366 w2383]
          tunnel: w2311 -> [w2318 w2336 w2352 w2369]
          frame 0, Default {
            n1381 = Unbundle By Name(w2318) -> ("Motion Module.Rotary Module Selection"=w2328:refnum<vi>)
            n1382 = Unbundle By Name(w2318) -> ("Motion Module.Motion Direction:  3"=w2326:refnum<vi>)
            n1383 = Unbundle By Name(w2318) -> ("Main Screen.Angle (Deg)"=w2320:refnum<vi>)
            n1384 = property on="Property Node" class="TabCtl (strict)"(reference=w2328, "Value"=T17."Uniform Rotation") -> (reference out=w2330:refnum<vi>, error out=w2329:errorcluster)  [unwired: 1 in]
            n1385 = property on="Property Node" class="DigNum (strict)"(reference=w2320, "DisabledEnum"=T31."Disabled and Grayed Out" ("Disabled")) -> (reference out=w2322:refnum<vi>, error out=w2321:errorcluster)  [unwired: 1 in]
            n1386 = property on="Property Node" class="Ring (strict)"(reference=w2326, "Visible"=TRUE) -> (reference out=w2324:refnum<vi>, error out=w2325:errorcluster)  [unwired: 1 in]
            n1387 = Close Reference(reference=w2330, error in (no error)=w2329) -> ()  [unwired: 1 out]
            n1388 = Close Reference(reference=w2322, error in (no error)=w2321) -> ()  [unwired: 1 out]
            n1389 = Close Reference(reference=w2324, error in (no error)=w2325) -> ()  [unwired: 1 out]
            n1390 = call "DATA ENCRYPT STRING FILE WRITE.vi"("error in (no error)"=w2334, "User Action"="User Selected Uniform Rotation", "main ref"=w2332) -> ("error out"=w2333:errorcluster)  [unwired: 6 in, 1 out]
          }
          frame 1 {
            n1391 = Unbundle By Name(w2336) -> ("Motion Module.Rotary Module Selection"=w2345:refnum<vi>)
            n1392 = Unbundle By Name(w2336) -> ("Motion Module.Motion Direction:  3"=w2343:refnum<vi>)
            n1393 = Unbundle By Name(w2336) -> ("Main Screen.Angle (Deg)"=w2337:refnum<vi>)
            n1394 = property on="Property Node" class="TabCtl (strict)"(reference=w2345, "Value"=T17."Angular Oscillation") -> (reference out=w2347:refnum<vi>, error out=w2346:errorcluster)  [unwired: 1 in]
            n1395 = property on="Property Node" class="DigNum (strict)"(reference=w2337, "DisabledEnum"=T31."Enabled" ("Disabled")) -> (reference out=w2339:refnum<vi>, error out=w2338:errorcluster)  [unwired: 1 in]
            n1396 = property on="Property Node" class="Ring (strict)"(reference=w2343, "Visible"=FALSE) -> (reference out=w2341:refnum<vi>, error out=w2342:errorcluster)  [unwired: 1 in]
            n1397 = Close Reference(reference=w2347, error in (no error)=w2346) -> ()  [unwired: 1 out]
            n1398 = Close Reference(reference=w2341, error in (no error)=w2342) -> ()  [unwired: 1 out]
            n1399 = Close Reference(reference=w2339, error in (no error)=w2338) -> ()  [unwired: 1 out]
            n1400 = call "DATA ENCRYPT STRING FILE WRITE.vi"("error in (no error)"=w2351, "User Action"="User Selected Angular Oscillation", "main ref"=w2349) -> ("error out"=w2350:errorcluster)  [unwired: 6 in, 1 out]
          }
          frame 2 {
            n1401 = Unbundle By Name(w2352) -> ("Motion Module.Rotary Module Selection"=w2362:refnum<vi>)
            n1402 = Unbundle By Name(w2352) -> ("Motion Module.Motion Direction:  3"=w2360:refnum<vi>)
            n1403 = Unbundle By Name(w2352) -> ("Main Screen.Angle (Deg)"=w2354:refnum<vi>)
            n1404 = property on="Property Node" class="DigNum (strict)"(reference=w2354, "DisabledEnum"=T31."Disabled and Grayed Out" ("Disabled")) -> (reference out=w2356:refnum<vi>, error out=w2355:errorcluster)  [unwired: 1 in]
            n1405 = property on="Property Node" class="TabCtl (strict)"(reference=w2362, "Value"=T17."Speed Ramp") -> (reference out=w2364:refnum<vi>, error out=w2363:errorcluster)  [unwired: 1 in]
            n1406 = property on="Property Node" class="Ring (strict)"(reference=w2360, "Visible"=TRUE) -> (reference out=w2358:refnum<vi>, error out=w2359:errorcluster)  [unwired: 1 in]
            n1407 = Close Reference(reference=w2356, error in (no error)=w2355) -> ()  [unwired: 1 out]
            n1408 = Close Reference(reference=w2364, error in (no error)=w2363) -> ()  [unwired: 1 out]
            n1409 = Close Reference(reference=w2358, error in (no error)=w2359) -> ()  [unwired: 1 out]
            n1410 = call "DATA ENCRYPT STRING FILE WRITE.vi"("error in (no error)"=w2368, "User Action"="User Selected Ramp Mode", "main ref"=w2366) -> ("error out"=w2367:errorcluster)  [unwired: 6 in, 1 out]
          }
          frame 3 {
            n1411 = Unbundle By Name(w2369) -> ("Motion Module.Rotary Module Selection"=w2379:refnum<vi>)
            n1412 = Unbundle By Name(w2369) -> ("Motion Module.Motion Direction:  3"=w2377:refnum<vi>)
            n1413 = Unbundle By Name(w2369) -> ("Main Screen.Angle (Deg)"=w2371:refnum<vi>)
            n1414 = property on="Property Node" class="TabCtl (strict)"(reference=w2379, "Value"=T17."Speed Step") -> (reference out=w2381:refnum<vi>, error out=w2380:errorcluster)  [unwired: 1 in]
            n1415 = property on="Property Node" class="DigNum (strict)"(reference=w2371, "DisabledEnum"=T31."Disabled and Grayed Out" ("Disabled")) -> (reference out=w2373:refnum<vi>, error out=w2372:errorcluster)  [unwired: 1 in]
            n1416 = property on="Property Node" class="Ring (strict)"(reference=w2377, "Visible"=FALSE) -> (reference out=w2375:refnum<vi>, error out=w2376:errorcluster)  [unwired: 1 in]
            n1417 = Close Reference(reference=w2381, error in (no error)=w2380) -> ()  [unwired: 1 out]
            n1418 = Close Reference(reference=w2373, error in (no error)=w2372) -> ()  [unwired: 1 out]
            n1419 = Close Reference(reference=w2375, error in (no error)=w2376) -> ()  [unwired: 1 out]
            n1420 = call "DATA ENCRYPT STRING FILE WRITE.vi"("error in (no error)"=w2385, "User Action"="User Selected Step Mode", "main ref"=w2383) -> ("error out"=w2384:errorcluster)  [unwired: 6 in, 1 out]
          }
        }
      }
      frame "MMNext" {
        n1421 = Unbundle By Name(w2386) -> ("Motion Module.MMNext"=w2391:refnum<vi>)
        n1422 = Unbundle By Name(w2386) -> ("Motion Module.MMNext"=w2398:refnum<vi>)
        n1423 = Unbundle By Name(w2386) -> ("Main Home Screen.GUI"=w2400:refnum<vi>)
        n1424 = property on="Property Node" class="Bool (strict)"(reference=w2391, "Value"=FALSE ("Visible")) -> (reference out=w2388:refnum<vi>, error out=w2390:errorcluster)  [unwired: 1 in]
        n1425 = property on="Property Node" class="TabCtl (strict)"(reference=w2400, "Value"=T14."Environment") -> (reference out=w2402:refnum<vi>, error out=w2401:errorcluster)  [unwired: 1 in]
        n1426 = property on="Property Node" class="Bool (strict)"(reference=w2398, "Value"=FALSE) -> (reference out=w2396:refnum<vi>, error out=w2397:errorcluster)  [unwired: 1 in]
        n1427 = Close Reference(reference=w2388, error in (no error)=w2390) -> ()  [unwired: 1 out]
        n1428 = Close Reference(reference=w2396, error in (no error)=w2397) -> ()  [unwired: 1 out]
        n1429 = Close Reference(reference=w2402, error in (no error)=w2401) -> ()  [unwired: 1 out]
        n1430 = call "DATA ENCRYPT STRING FILE WRITE.vi"("error in (no error)"=w2393, "User Action"="User Selected SetUp Module", "main ref"=w2386) -> ("error out"=w2392:errorcluster)  [unwired: 6 in, 1 out]
        n1431 = call "Main Screen Tab Visible.vi"("error in (no error)"=w2392, "main ref"=w2386) -> ("error out"=w2387:errorcluster)  [unwired: 9 in]
      }
      frame "APBack" {
        n1432 = Unbundle By Name(w2403) -> ("Environmental control.APBack"=w2410:refnum<vi>)
        n1433 = Unbundle By Name(w2403) -> ("Main Home Screen.GUI"=w2412:refnum<vi>)
        n1434 = property on="Property Node" class="TabCtl (strict)"(reference=w2412, "Value"=T14."Motion Module") -> (reference out=w2414:refnum<vi>, error out=w2413:errorcluster)  [unwired: 1 in]
        n1435 = property on="Property Node" class="Bool (strict)"(reference=w2410, "Value"=FALSE) -> (reference out=w2408:refnum<vi>, error out=w2409:errorcluster)  [unwired: 1 in]
        n1436 = Close Reference(reference=w2408, error in (no error)=w2409) -> ()  [unwired: 1 out]
        n1437 = Close Reference(reference=w2414, error in (no error)=w2413) -> ()  [unwired: 1 out]
        n1438 = call "DATA ENCRYPT STRING FILE WRITE.vi"("error in (no error)"=w2405, "User Action"="User Selected Back to Module", "main ref"=w2403) -> ("error out"=w2404:errorcluster)  [unwired: 6 in, 1 out]
      }
      frame "SNext" {
        n1439 = Unbundle By Name(w2416) -> ("Environmental control.Acoustic Emission 3"=w2420:refnum<vi>)
        n1440 = property on="Property Node" class="Bool (strict)"(reference=w2420) -> (reference out=w2418:refnum<vi>, error out=w2419:errorcluster, "Value"=w2415:bool)  [unwired: 1 in]
        n1441 = Close Reference(reference=w2418, error in (no error)=w2419) -> ()  [unwired: 1 out]
        n1442 = case shown="True" w2415 {
          tunnel: w2422 -> [w2425 w2429]
          tunnel: [w2425 w2426] -> w2417
          tunnel: w2416 -> [_ w2427]
          frame False {
          }
          frame True {
            n1443 = call "Acq Gain Selection.vi"("error in (no error)"=w2429, "Data Cluster"=w2427) -> ("error out"=w2428:errorcluster)  [unwired: 9 in]
            n1444 = call <vilib>:"Clear Errors.vi"("error in (no error)"=w2428) -> ("error out"=w2426:errorcluster)  [unwired: 5 in, 1 out]
          }
        }
        n1445 = call "Init Before Main Screen.vi"("error in (no error)"=w2417, "Data Cluster"=w2416) -> ("error out"=w2421:errorcluster)  [unwired: 9 in]
        n1446 = call "DATA ENCRYPT STRING FILE WRITE.vi"("error in (no error)"=w2421, "User Action"="User Pressed Setup", "main ref"=w2416) -> ("error out"=w2423:errorcluster)  [unwired: 6 in, 1 out]
      }
      frame "Enable Platform" {
        n1447 = call "Reinitialise Load cell after Error.vi"("error in (no error)"=w2434, "main ref"=w2430) -> ("error out"=w2432:errorcluster)  [unwired: 9 in]
        n1448 = Unbundle By Name(w2430) -> ("Platform Settings.Enable Platform"=w2457:refnum<vi>)
        n1449 = Bundle By Name(cluster=T11 {"Sequence ID"=0, "Mode Command"=0, "Distance"=0.0, "SPEED"=0.0, "Reserved"=0.0, "SPARE 1"=0, "SPARE 2"=0, "SPARE 3"=0, "SPARE 4"=0, "SPARE 5"=0, "SPARE 6"=0, "SPARE 7"=0, "SPARE 8"=0, "SPARE 9"=0, "SPARE 10"=0, "SPARE 11"=0, "SPARE 12"=0, "SPARE 13"=0, "SPARE 14"=0, "SPARE 15"=0, "SPARE 16"=0, "SPARE 17"=0} ("Value"), "Mode Command"=u8 1, "Distance"=sgl 0.0, "SPEED"=sgl 0.0, "Sequence ID"=u16 0) -> (w2443:T11)
        n1450 = Unbundle By Name(w2430) -> ("Heave AND Surge.UPLINK HEAVE"=w2436:refnum<vi>)
        n1451 = property on="Property Node" class="Bool (strict)"(reference=w2457, "Value"=FALSE) -> (reference out=w2455:refnum<vi>, error out=w2456:errorcluster)  [unwired: 1 in]
        n1452 = property on="Property Node" class="Clust (strict)"(reference=w2436, error in=w2432, "Value"=w2443) -> (reference out=w2442:refnum<vi>, error out=w2441:errorcluster)
        n1453 = Close Reference(reference=w2455, error in (no error)=w2456) -> ()  [unwired: 1 out]
        n1454 = Close Reference(reference=w2442, error in (no error)=w2441) -> (error out=w2433:errorcluster)
        n1455 = call "DATA ENCRYPT STRING FILE WRITE.vi"("error in (no error)"=w2433, "User Action"="User Pressed Enable Platform", "main ref"=w2430) -> ("error out"=w2431:errorcluster)  [unwired: 6 in, 1 out]
        n1456 = call "HEAVE WRITE FGV.vi"("Enum - Menu"=Heave_Write_enum."WRITE", "error in (no error)"=w2431, "main ref"=w2430) -> ("error out"=w2447:errorcluster)  [unwired: 8 in]
        n1457 = call "SET LOAD PARAMETERS.vi"("error in (no error)"=w2431, "main ref"=w2430) -> ()  [unwired: 9 in, 1 out]
        n1458 = call "TRACTION HOME.vi"("error in (no error)"=w2431, "Data Cluster"=w2430) -> ("error out"=→"error out":errorcluster)  [unwired: 9 in]
        n1459 = Unbundle By Name(w2430) -> ("Heave AND Surge.Read Heave Temp"=w2451:refnum<vi>)
        n1460 = property on="Property Node" class="Bool (strict)"(reference=w2451, error in=w2447, "Value"=TRUE) -> (reference out=w2449:refnum<vi>, error out=w2450:errorcluster)
        n1461 = Close Reference(reference=w2449, error in (no error)=w2450) -> (error out=w2446:errorcluster)
        "HEAVE ENABLE" <- TRUE ("HEAVE ENABLE")
      }
      frame "Heave Up main" {
        n1462 = Unbundle By Name(w2458) -> ("Platform Settings.Heave Up main"=w2468:refnum<vi>)
        n1463 = call "Heave Up Main.vi"("error in (no error)"=w2460, "main ref"=w2458) -> ("error out"=w2459:errorcluster)  [unwired: 9 in]
        n1464 = property on="Property Node" class="Bool (strict)"(reference=w2468, "Value"=FALSE) -> (reference out=w2466:refnum<vi>, error out=w2467:errorcluster)  [unwired: 1 in]
        n1465 = Close Reference(reference=w2466, error in (no error)=w2467) -> ()  [unwired: 1 out]
        n1466 = call "DATA ENCRYPT STRING FILE WRITE.vi"("error in (no error)"=w2459, "User Action"="User Pressed Heave UP", "main ref"=w2458) -> ("error out"=w2463:errorcluster)  [unwired: 6 in, 1 out]
        n1467 = call "HEAVE WRITE FGV.vi"("Enum - Menu"=Heave_Write_enum."WRITE", "error in (no error)"=w2463, "main ref"=w2458) -> ("error out"=w2462:errorcluster)  [unwired: 8 in]
      }
      frame "Heave Up MM" {
        n1468 = Unbundle By Name(w2469) -> ("Motion Module.Heave Up MM"=w2479:refnum<vi>)
        n1469 = call "Heave Up Motion Module.vi"("error in (no error)"=w2471, "main ref"=w2469) -> ("error out"=w2470:errorcluster)  [unwired: 9 in]
        n1470 = property on="Property Node" class="Bool (strict)"(reference=w2479, "Value"=FALSE) -> (reference out=w2477:refnum<vi>, error out=w2478:errorcluster)  [unwired: 1 in]
        n1471 = Close Reference(reference=w2477, error in (no error)=w2478) -> ()  [unwired: 1 out]
        n1472 = call "DATA ENCRYPT STRING FILE WRITE.vi"("error in (no error)"=w2470, "User Action"="User Pressed Heave UP in Motion Module", "main ref"=w2469) -> ("error out"=w2474:errorcluster)  [unwired: 6 in, 1 out]
        n1473 = call "HEAVE WRITE FGV.vi"("Enum - Menu"=Heave_Write_enum."WRITE", "error in (no error)"=w2474, "main ref"=w2469) -> ("error out"=w2473:errorcluster)  [unwired: 8 in]
      }
      frame "Heave Down Main" {
        n1474 = call "Heave Down Main.vi"("error in (no error)"=w2482, "main ref"=w2480) -> ("error out"=w2481:errorcluster)  [unwired: 9 in]
        n1475 = Unbundle By Name(w2480) -> ("Platform Settings.Heave Down Main"=w2490:refnum<vi>)
        n1476 = property on="Property Node" class="Bool (strict)"(reference=w2490, "Value"=FALSE) -> (reference out=w2488:refnum<vi>, error out=w2489:errorcluster)  [unwired: 1 in]
        n1477 = Close Reference(reference=w2488, error in (no error)=w2489) -> ()  [unwired: 1 out]
        n1478 = call "DATA ENCRYPT STRING FILE WRITE.vi"("error in (no error)"=w2481, "User Action"="User Pressed Heave DOWN", "main ref"=w2480) -> ("error out"=w2485:errorcluster)  [unwired: 6 in, 1 out]
        n1479 = call "HEAVE WRITE FGV.vi"("Enum - Menu"=Heave_Write_enum."WRITE", "error in (no error)"=w2485, "main ref"=w2480) -> ("error out"=w2484:errorcluster)  [unwired: 8 in]
      }
      frame "Heave Down MM" {
        n1480 = call "Heave Down Motion Module.vi"("error in (no error)"=w2493, "main ref"=w2491) -> ("error out"=w2492:errorcluster)  [unwired: 9 in]
        n1481 = Unbundle By Name(w2491) -> ("Motion Module.Heave Down MM"=w2501:refnum<vi>)
        n1482 = property on="Property Node" class="Bool (strict)"(reference=w2501, "Value"=FALSE) -> (reference out=w2499:refnum<vi>, error out=w2500:errorcluster)  [unwired: 1 in]
        n1483 = Close Reference(reference=w2499, error in (no error)=w2500) -> ()  [unwired: 1 out]
        n1484 = call "DATA ENCRYPT STRING FILE WRITE.vi"("error in (no error)"=w2492, "User Action"="User Pressed Heave DOWN in Motion Module", "main ref"=w2491) -> ("error out"=w2496:errorcluster)  [unwired: 6 in, 1 out]
        n1485 = call "HEAVE WRITE FGV.vi"("Enum - Menu"=Heave_Write_enum."WRITE", "error in (no error)"=w2496, "main ref"=w2491) -> ("error out"=w2495:errorcluster)  [unwired: 8 in]
      }
      frame "Surge Backward Main" {
        n1486 = Unbundle By Name(w2502) -> ("Platform Settings.Surge Backward Main"=w2512:refnum<vi>)
        n1487 = call "Surge Backward Main.vi"("error in (no error)"=w2504, "main ref"=w2502) -> ("error out"=w2503:errorcluster)  [unwired: 9 in]
        n1488 = property on="Property Node" class="Bool (strict)"(reference=w2512, "Value"=FALSE) -> (reference out=w2510:refnum<vi>, error out=w2511:errorcluster)  [unwired: 1 in]
        n1489 = Close Reference(reference=w2510, error in (no error)=w2511) -> ()  [unwired: 1 out]
        n1490 = call "DATA ENCRYPT STRING FILE WRITE.vi"("error in (no error)"=w2503, "User Action"="User Pressed Surge Backward", "main ref"=w2502) -> ("error out"=w2507:errorcluster)  [unwired: 6 in, 1 out]
        n1491 = call "HEAVE WRITE FGV.vi"("Enum - Menu"=Heave_Write_enum."WRITE", "error in (no error)"=w2507, "main ref"=w2502) -> ("error out"=w2506:errorcluster)  [unwired: 8 in]
      }
      frame "Surge Backward MM" {
        n1492 = Unbundle By Name(w2513) -> ("Motion Module.Surge Backward MM"=w2523:refnum<vi>)
        n1493 = call "Surge Backward MM.vi"("error in (no error)"=w2515, "main ref"=w2513) -> ("error out"=w2514:errorcluster)  [unwired: 9 in]
        n1494 = property on="Property Node" class="Bool (strict)"(reference=w2523, "Value"=FALSE) -> (reference out=w2521:refnum<vi>, error out=w2522:errorcluster)  [unwired: 1 in]
        n1495 = Close Reference(reference=w2521, error in (no error)=w2522) -> ()  [unwired: 1 out]
        n1496 = call "DATA ENCRYPT STRING FILE WRITE.vi"("error in (no error)"=w2514, "User Action"="User Pressed Surge Backward in Motion Module", "main ref"=w2513) -> ("error out"=w2518:errorcluster)  [unwired: 6 in, 1 out]
        n1497 = call "HEAVE WRITE FGV.vi"("Enum - Menu"=Heave_Write_enum."WRITE", "error in (no error)"=w2518, "main ref"=w2513) -> ("error out"=w2517:errorcluster)  [unwired: 8 in]
      }
      frame "Surge Forward Main" {
        n1498 = Unbundle By Name(w2524) -> ("Platform Settings.Surge Forward Main"=w2534:refnum<vi>)
        n1499 = call "Surge Forward Main.vi"("error in (no error)"=w2526, "main ref"=w2524) -> ("error out"=w2525:errorcluster)  [unwired: 9 in]
        n1500 = property on="Property Node" class="Bool (strict)"(reference=w2534, "Value"=FALSE) -> (reference out=w2532:refnum<vi>, error out=w2533:errorcluster)  [unwired: 1 in]
        n1501 = Close Reference(reference=w2532, error in (no error)=w2533) -> ()  [unwired: 1 out]
        n1502 = call "DATA ENCRYPT STRING FILE WRITE.vi"("error in (no error)"=w2525, "User Action"="User Pressed Surge Forward", "main ref"=w2524) -> ("error out"=w2529:errorcluster)  [unwired: 6 in, 1 out]
        n1503 = call "HEAVE WRITE FGV.vi"("Enum - Menu"=Heave_Write_enum."WRITE", "error in (no error)"=w2529, "main ref"=w2524) -> ("error out"=w2528:errorcluster)  [unwired: 8 in]
      }
      frame "Surge Forward MM" {
        n1504 = Unbundle By Name(w2535) -> ("Motion Module.Surge Forward MM"=w2545:refnum<vi>)
        n1505 = call "Surge Forward MM.vi"("error in (no error)"=w2537, "main ref"=w2535) -> ("error out"=w2536:errorcluster)  [unwired: 9 in]
        n1506 = property on="Property Node" class="Bool (strict)"(reference=w2545, "Value"=FALSE) -> (reference out=w2543:refnum<vi>, error out=w2544:errorcluster)  [unwired: 1 in]
        n1507 = Close Reference(reference=w2543, error in (no error)=w2544) -> ()  [unwired: 1 out]
        n1508 = call "DATA ENCRYPT STRING FILE WRITE.vi"("error in (no error)"=w2536, "User Action"="User Pressed Surge Forward in Motion Module", "main ref"=w2535) -> ("error out"=w2540:errorcluster)  [unwired: 6 in, 1 out]
        n1509 = call "HEAVE WRITE FGV.vi"("Enum - Menu"=Heave_Write_enum."WRITE", "error in (no error)"=w2540, "main ref"=w2535) -> ("error out"=w2539:errorcluster)  [unwired: 8 in]
      }
      frame "Sway Left Main" {
        n1510 = call "Sway Left Main.vi"("error in (no error)"=w2549, "main ref"=w2547) -> ("error out"=w2548:errorcluster)  [unwired: 9 in]
        n1511 = Unbundle By Name(w2547) -> ("Platform Settings.Sway Left Main"=w2556:refnum<vi>)
        n1512 = property on="Property Node" class="Bool (strict)"(reference=w2556, "Value"=FALSE) -> (reference out=w2554:refnum<vi>, error out=w2555:errorcluster)  [unwired: 1 in]
        n1513 = Close Reference(reference=w2554, error in (no error)=w2555) -> ()  [unwired: 1 out]
        n1514 = call "DATA ENCRYPT STRING FILE WRITE.vi"("error in (no error)"=w2548, "User Action"="User Pressed Sway Left ", "main ref"=w2547) -> ("error out"=w2551:errorcluster)  [unwired: 6 in, 1 out]
        n1515 = call "SWAY WRITE FGV.vi"("Enum - Menu"=Sway_Write_enum."WRITE", "error in (no error)"=w2551, "main ref"=w2547) -> ("error out"=w2550:errorcluster)  [unwired: 8 in]
      }
      frame "Sway Left MM" {
        n1516 = call "Sway Left MM.vi"("error in (no error)"=w2560, "main ref"=w2558) -> ("error out"=w2559:errorcluster)  [unwired: 9 in]
        n1517 = Unbundle By Name(w2558) -> ("Motion Module.Sway Left MM"=w2567:refnum<vi>)
        n1518 = property on="Property Node" class="Bool (strict)"(reference=w2567, "Value"=FALSE) -> (reference out=w2565:refnum<vi>, error out=w2566:errorcluster)  [unwired: 1 in]
        n1519 = Close Reference(reference=w2565, error in (no error)=w2566) -> ()  [unwired: 1 out]
        n1520 = call "DATA ENCRYPT STRING FILE WRITE.vi"("error in (no error)"=w2559, "User Action"="User Pressed Sway Left in MM", "main ref"=w2558) -> ("error out"=w2562:errorcluster)  [unwired: 6 in, 1 out]
        n1521 = call "SWAY WRITE FGV.vi"("Enum - Menu"=Sway_Write_enum."WRITE", "error in (no error)"=w2562, "main ref"=w2558) -> ("error out"=w2561:errorcluster)  [unwired: 8 in]
      }
      frame "Sway Right MM" {
        n1522 = call "Sway Right MM.vi"("error in (no error)"=w2571, "main ref"=w2569) -> ("error out"=w2570:errorcluster)  [unwired: 9 in]
        n1523 = Unbundle By Name(w2569) -> ("Motion Module.Sway Right MM"=w2578:refnum<vi>)
        n1524 = property on="Property Node" class="Bool (strict)"(reference=w2578, "Value"=FALSE) -> (reference out=w2576:refnum<vi>, error out=w2577:errorcluster)  [unwired: 1 in]
        n1525 = Close Reference(reference=w2576, error in (no error)=w2577) -> ()  [unwired: 1 out]
        n1526 = call "DATA ENCRYPT STRING FILE WRITE.vi"("error in (no error)"=w2570, "User Action"="User Pressed Sway Right in MM", "main ref"=w2569) -> ("error out"=w2573:errorcluster)  [unwired: 6 in, 1 out]
        n1527 = call "SWAY WRITE FGV.vi"("Enum - Menu"=Sway_Write_enum."WRITE", "error in (no error)"=w2573, "main ref"=w2569) -> ("error out"=w2572:errorcluster)  [unwired: 8 in]
      }
      frame "Sway Right Main" {
        n1528 = call "Sway Right Main.vi"("error in (no error)"=w2582, "main ref"=w2580) -> ("error out"=w2581:errorcluster)  [unwired: 9 in]
        n1529 = Unbundle By Name(w2580) -> ("Platform Settings.Sway Right Main"=w2589:refnum<vi>)
        n1530 = property on="Property Node" class="Bool (strict)"(reference=w2589, "Value"=FALSE) -> (reference out=w2587:refnum<vi>, error out=w2588:errorcluster)  [unwired: 1 in]
        n1531 = Close Reference(reference=w2587, error in (no error)=w2588) -> ()  [unwired: 1 out]
        n1532 = call "DATA ENCRYPT STRING FILE WRITE.vi"("error in (no error)"=w2581, "User Action"="User Pressed Sway Right", "main ref"=w2580) -> ("error out"=w2584:errorcluster)  [unwired: 6 in, 1 out]
        n1533 = call "SWAY WRITE FGV.vi"("Enum - Menu"=Sway_Write_enum."WRITE", "error in (no error)"=w2584, "main ref"=w2580) -> ("error out"=w2583:errorcluster)  [unwired: 8 in]
      }
      frame "Manual Write Heave & Surge" {
        n1534 = Unbundle By Name(w2590) -> ("Heave AND Surge.Manual Write"=w2599:refnum<vi>)
        n1535 = property on="Property Node" class="Bool (strict)"(reference=w2599, "Value"=FALSE) -> (reference out=w2597:refnum<vi>, error out=w2598:errorcluster)  [unwired: 1 in]
        n1536 = Close Reference(reference=w2597, error in (no error)=w2598) -> ()  [unwired: 1 out]
        n1537 = call "DATA ENCRYPT STRING FILE WRITE.vi"("error in (no error)"=w2591, "User Action"="User Pressed Manual Write Heave and Surge", "main ref"=w2590) -> ("error out"=w2594:errorcluster)  [unwired: 6 in, 1 out]
        n1538 = call "HEAVE WRITE FGV.vi"("Enum - Menu"=Heave_Write_enum."WRITE", "error in (no error)"=w2594, "main ref"=w2590) -> ("error out"=w2593:errorcluster)  [unwired: 8 in]
      }
      frame "Manual Write SWAY" {
        n1539 = Unbundle By Name(w2601) -> ("SWAY.Manual Write SWAY"=w2609:refnum<vi>)
        n1540 = property on="Property Node" class="Bool (strict)"(reference=w2609, "Value"=FALSE) -> (reference out=w2607:refnum<vi>, error out=w2608:errorcluster)  [unwired: 1 in]
        n1541 = Close Reference(reference=w2607, error in (no error)=w2608) -> ()  [unwired: 1 out]
        n1542 = call "DATA ENCRYPT STRING FILE WRITE.vi"("error in (no error)"=w2602, "User Action"="User Pressed Manual Write Sway", "main ref"=w2601) -> ("error out"=w2604:errorcluster)  [unwired: 6 in, 1 out]
        n1543 = call "SWAY WRITE FGV.vi"("Enum - Menu"=Sway_Write_enum."WRITE", "error in (no error)"=w2604, "main ref"=w2601) -> ("error out"=w2603:errorcluster)  [unwired: 8 in]
      }
      frame "Manual Write TRACTION" {
        n1544 = Unbundle By Name(w2611) -> ("Traction.Manual Write TRACTION"=w2619:refnum<vi>)
        n1545 = property on="Property Node" class="Bool (strict)"(reference=w2619, "Value"=FALSE) -> (reference out=w2617:refnum<vi>, error out=w2618:errorcluster)  [unwired: 1 in]
        n1546 = Close Reference(reference=w2617, error in (no error)=w2618) -> ()  [unwired: 1 out]
        n1547 = call "DATA ENCRYPT STRING FILE WRITE.vi"("error in (no error)"=w2612, "User Action"="User Pressed Manual Write Traction", "main ref"=w2611) -> ("error out"=w2614:errorcluster)  [unwired: 6 in, 1 out]
        n1548 = call "TRACTION WRITE FGV.vi"("Enum - Menu"=Traction_Write_enum."WRITE", "error in (no error)"=w2614, "main ref"=w2611) -> ("error out"=w2613:errorcluster)  [unwired: 8 in]
      }
      frame "Manual Write ACQUOSTIC" {
        n1549 = local write "Manual Write Acquostic"(FALSE ("Manual Write Acquostic")) -> ()
        n1550 = call "DATA ENCRYPT STRING FILE WRITE.vi"("error in (no error)"=w2623, "User Action"="User Pressed Manual Write Acquostics", "main ref"=w2622) -> ("error out"=w2625:errorcluster)  [unwired: 6 in, 1 out]
        n1551 = call "Acq Write Loop.vi"("Enum - Menu"=Write_Main_Enum."WRITE", "error in (no error)"=w2625, "main ref"=w2622) -> ("error out"=w2624:errorcluster)  [unwired: 8 in]
      }
      frame "Load En" {
        # "zNL 2"
        n1552 = Unbundle By Name(w2628) -> ("Main Screen.Load En"=w2633:refnum<vi>)
        n1553 = property on="Property Node" class="Bool (strict)"(reference=w2633) -> (reference out=w2631:refnum<vi>, error out=w2632:errorcluster, "Value"=w2627:bool)  [unwired: 1 in]
        n1554 = Close Reference(reference=w2631, error in (no error)=w2632) -> ()  [unwired: 1 out]
        n1555 = case shown="False" w2627 {
          tunnel: [w2645 w2655] -> w2629
          tunnel: w2630 -> [w2647 w2654]
          tunnel: w2628 -> [w2635 w2649]
          tunnel: w2628 -> [w2643 _]
          tunnel: w2628 -> [w2642 _]
          frame False {
            n1556 = call "DATA ENCRYPT STRING FILE WRITE.vi"("error in (no error)"=w2647, "User Action"="User Pressed UnLoad on Main Screen", "main ref"=w2635) -> ("error out"=w2636:errorcluster)  [unwired: 6 in, 1 out]
            n1557 = call "Stall Data Flow.vim"("value in"=w2636, "milliseconds to wait"=u32 2000) -> ("value out"=w2641:errorcluster)  [unwired: 1 out]
            n1558 = Unbundle By Name(w2635) -> ("Main Screen.zNL 2"=w2639:refnum<vi>)
            n1559 = property on="Property Node" class="Bool (strict)"(reference=w2639, "DisabledEnum"=T31."Enabled" ("Disabled")) -> (reference out=w2637:refnum<vi>, error out=w2638:errorcluster)  [unwired: 1 in]
            n1560 = call "PID UNLOAD.vi"("error in (no error)"=w2641, "main ref"=w2642) -> ("error out"=w2644:errorcluster)  [unwired: 9 in]
            n1561 = Close Reference(reference=w2637, error in (no error)=w2638) -> ()  [unwired: 1 out]
            n1562 = call "HEAVE WRITE FGV.vi"("Enum - Menu"=Heave_Write_enum."WRITE", "error in (no error)"=w2644, "main ref"=w2643) -> ("error out"=w2645:errorcluster)  [unwired: 8 in]
          }
          frame True {
            n1563 = call "DATA ENCRYPT STRING FILE WRITE.vi"("error in (no error)"=w2654, "User Action"="User Pressed Load on Main Screen", "main ref"=w2649) -> ("error out"=w2655:errorcluster)  [unwired: 6 in, 1 out]
            n1564 = Unbundle By Name(w2649) -> ("Main Screen.zNL 2"=w2653:refnum<vi>)
            n1565 = property on="Property Node" class="Bool (strict)"(reference=w2653, "DisabledEnum"=T31."Disabled and Grayed Out" ("Disabled")) -> (reference out=w2651:refnum<vi>, error out=w2652:errorcluster)  [unwired: 1 in]
            n1566 = Close Reference(reference=w2651, error in (no error)=w2652) -> ()  [unwired: 1 out]
          }
        }
      }
      frame "apply load" {
        n1567 = Unbundle By Name(w2658) -> ("Main Screen.Load En"=w2663:refnum<vi>)
        n1568 = property on="Property Node" class="Bool (strict)"(reference=w2663) -> (reference out=w2661:refnum<vi>, error out=w2662:errorcluster, "Value"=w2657:bool)  [unwired: 1 in]
        n1569 = Close Reference(reference=w2661, error in (no error)=w2662) -> ()  [unwired: 1 out]
        n1570 = case shown="False" w2657 {
          tunnel: [w2670 w2677] -> w2659
          tunnel: w2660 -> [w2673 w2676]
          tunnel: w2658 -> [w2672 w2675]
          tunnel: w2658 -> [w2667 _]
          tunnel: w2658 -> [w2666 _]
          frame False {
            n1571 = call "DATA ENCRYPT STRING FILE WRITE.vi"("error in (no error)"=w2673, "User Action"="User Pressed UnLoad on Service Screen", "main ref"=w2672) -> ("error out"=w2669:errorcluster)  [unwired: 6 in, 1 out]
            n1572 = call "Stall Data Flow.vim"("value in"=w2669, "milliseconds to wait"=u32 2000) -> ("value out"=w2665:errorcluster)  [unwired: 1 out]
            n1573 = call "PID UNLOAD.vi"("error in (no error)"=w2665, "main ref"=w2666) -> ("error out"=w2668:errorcluster)  [unwired: 9 in]
            n1574 = call "HEAVE WRITE FGV.vi"("Enum - Menu"=Heave_Write_enum."WRITE", "error in (no error)"=w2668, "main ref"=w2667) -> ("error out"=w2670:errorcluster)  [unwired: 8 in]
          }
          frame True {
            n1575 = call "DATA ENCRYPT STRING FILE WRITE.vi"("error in (no error)"=w2676, "User Action"="User Pressed Load on Service Screen", "main ref"=w2675) -> ("error out"=w2677:errorcluster)  [unwired: 6 in, 1 out]
          }
        }
      }
      frame "BACK" {
        w2684 = FALSE ("Value")
        n1576 = Unbundle By Name(w2679) -> ("Main Screen.BACK"=w2704:refnum<vi>)
        n1577 = property on="Property Node" class="Bool (strict)"(reference=w2704, "Value"=FALSE) -> (reference out=w2702:refnum<vi>, error out=w2703:errorcluster)  [unwired: 1 in]
        n1578 = Close Reference(reference=w2702, error in (no error)=w2703) -> ()  [unwired: 1 out]
        n1579 = call "DATA ENCRYPT STRING FILE WRITE.vi"("error in (no error)"=w2701, "User Action"="User Pressed Back on Main Screen", "main ref"=w2679) -> ("error out"=w2699:errorcluster)  [unwired: 6 in, 1 out]
        n1580 = Unbundle By Name(w2679) -> ("Main Home Screen.MainPage"=w2691:refnum<vi>)
        n1581 = Unbundle By Name(w2679) -> ("Main Screen.Start Test"=w2687:refnum<vi>)
        n1582 = Unbundle By Name(w2679) -> ("Main Screen.STOP"=w2686:refnum<vi>)
        n1583 = Unbundle By Name(w2679) -> ("Main Home Screen.GUI"=w2695:refnum<vi>)
        n1584 = property on="Property Node" class="TabCtl (strict)"(reference=w2691, "Value"=T15."HOME") -> (reference out=w2693:refnum<vi>, error out=w2692:errorcluster)  [unwired: 1 in]
        n1585 = property on="Property Node" class="TabCtl (strict)"(reference=w2695, "Value"=T14."Setup") -> (reference out=w2697:refnum<vi>, error out=w2696:errorcluster)  [unwired: 1 in]
        n1586 = property on="Property Node" class="Bool (strict)"(reference=w2687, "Visible"=TRUE ("Value"), "Value"=FALSE) -> (reference out=w2682:refnum<vi>, error out=w2688:errorcluster)  [unwired: 1 in]
        n1587 = property on="Property Node" class="Bool (strict)"(reference=w2686, "Value"=w2684, "Visible"=w2684) -> (reference out=w2681:refnum<vi>, error out=w2685:errorcluster)  [unwired: 1 in]
        n1588 = Close Reference(reference=w2697, error in (no error)=w2696) -> ()  [unwired: 1 out]
        n1589 = Close Reference(reference=w2693, error in (no error)=w2692) -> ()  [unwired: 1 out]
        n1590 = Close Reference(reference=w2682, error in (no error)=w2688) -> ()  [unwired: 1 out]
        n1591 = Close Reference(reference=w2681, error in (no error)=w2685) -> ()  [unwired: 1 out]
        n1592 = call "Reinitial Parameter After Test.vi"("error in (no error)"=w2699, "main ref"=w2679) -> ("error out"=w2680:errorcluster)  [unwired: 9 in]
      }
      frame "Start Test" {
        n1593 = Unbundle By Name(w2705) -> ("Environmental control.Acoustic Emission 3"=w2711:refnum<vi>)
        n1594 = property on="Property Node" class="Bool (strict)"(reference=w2711) -> (reference out=w2709:refnum<vi>, error out=w2710:errorcluster, "Value"=w2708:bool)  [unwired: 1 in]
        n1595 = Close Reference(reference=w2709, error in (no error)=w2710) -> ()  [unwired: 1 out]
        n1596 = case shown="True" w2708 {
          tunnel: w2707 -> [w2713 w2717]
          tunnel: [w2713 w2714] -> w2706
          tunnel: w2705 -> [_ w2715]
          frame False {
          }
          frame True {
            n1597 = call "Acq start.vi"("error in (no error)"=w2717, "Data Cluster"=w2715) -> ("error out"=w2716:errorcluster)  [unwired: 9 in]
            n1598 = call <vilib>:"Clear Errors.vi"("error in (no error)"=w2716) -> ("error out"=w2714:errorcluster)  [unwired: 5 in, 1 out]
          }
        }
        n1599 = call "Test Start Sequence.vi"("error in (no error)"=w2706, "Data Cluster"=w2705) -> ("error out"=w2712:errorcluster)  [unwired: 9 in]
      }
      frame "STOP" {
        n1600 = call "Test Stop.vi"("error in (no error)"=w2739, "Data Cluster"=w2718) -> ("error out"=w2719:errorcluster)  [unwired: 9 in]
        n1601 = Unbundle By Name(w2718) -> ("Main Screen.Load En"=w2738:refnum<vi>)
        n1602 = Unbundle By Name(w2718) -> ("Main Screen.CZ FF"=w2733:refnum<vi>)
        n1603 = Unbundle By Name(w2718) -> ("Main Screen.zFF"=w2730:refnum<vi>)
        n1604 = property on="Property Node" class="Bool (strict)"(reference=w2738, "DisabledEnum"=T31."Disabled and Grayed Out" ("Disabled")) -> (reference out=w2726:refnum<vi>, error out=w2737:errorcluster)  [unwired: 1 in]
        n1605 = property on="Property Node" class="Bool (strict)"(reference=w2733, "DisabledEnum"=T31."Disabled and Grayed Out" ("Disabled"), "Value"=FALSE ("Visible")) -> (reference out=w2732:refnum<vi>, error out=w2734:errorcluster)  [unwired: 1 in]
        n1606 = property on="Property Node" class="Bool (strict)"(reference=w2730, "DisabledEnum"=T31."Disabled and Grayed Out" ("Disabled"), "Value"=FALSE ("Visible")) -> (reference out=w2731:refnum<vi>, error out=w2729:errorcluster)  [unwired: 1 in]
        n1607 = Close Reference(reference=w2726, error in (no error)=w2737) -> ()  [unwired: 1 out]
        n1608 = Close Reference(reference=w2732, error in (no error)=w2734) -> ()  [unwired: 1 out]
        n1609 = Close Reference(reference=w2731, error in (no error)=w2729) -> ()  [unwired: 1 out]
        n1610 = Unbundle By Name(w2718) -> ("Environmental control.Acoustic Emission 3"=w2724:refnum<vi>)
        n1611 = property on="Property Node" class="Bool (strict)"(reference=w2724) -> (reference out=w2722:refnum<vi>, error out=w2723:errorcluster, "Value"=w2721:bool)  [unwired: 1 in]
        n1612 = Close Reference(reference=w2722, error in (no error)=w2723) -> ()  [unwired: 1 out]
        n1613 = case shown="False" w2721 {
          tunnel: w2719 -> [w2740 w2744]
          tunnel: [w2740 w2741] -> w2720
          tunnel: w2718 -> [_ w2742]
          frame False {
          }
          frame True {
            n1614 = call "Acq stop.vi"("error in (no error)"=w2744, "Data Cluster"=w2742) -> ("error out"=w2743:errorcluster)  [unwired: 9 in]
            n1615 = call <vilib>:"Clear Errors.vi"("error in (no error)"=w2743) -> ("error out"=w2741:errorcluster)  [unwired: 5 in, 1 out]
          }
        }
      }
      frame "PlaceModule" {
        n1616 = call "Place Module.vi"("error in (no error)"=w2747, "main ref"=w2745) -> ("error out"=w2746:errorcluster)  [unwired: 9 in]
      }
      frame "Stage Homing" {
        n1617 = call "HOMINING.vi"("error in (no error)"=w2750, "main ref"=w2748) -> ("error out"=w2749:errorcluster)  [unwired: 9 in]
      }
      frame "Clear 3" {
        n1618 = Unbundle By Name(w2752) -> ("Loading.Stribeck Table  For loading"=w2762:refnum<vi>)
        n1619 = Unbundle By Name(w2752) -> ("Loading.Clear 3"=w2753:refnum<vi>)
        n1620 = property on="Property Node" class="Bool (strict)"(reference=w2753, "Value"=FALSE) -> (reference out=w2755:refnum<vi>, error out=w2754:errorcluster)  [unwired: 1 in]
        n1621 = call "DATA ENCRYPT STRING FILE WRITE.vi"("error in (no error)"=w2758, "User Action"="User Pressed Clear  on Step Load Sequence", "main ref"=w2752) -> ("error out"=w2757:errorcluster)  [unwired: 6 in, 1 out]
        n1622 = property on="Property Node" class="Tbl (strict)"(reference=w2762, "Value"=string[][] []) -> (reference out=w2760:refnum<vi>, error out=w2761:errorcluster)  [unwired: 1 in]
        n1623 = Close Reference(reference=w2755, error in (no error)=w2754) -> ()  [unwired: 1 out]
        n1624 = Close Reference(reference=w2760, error in (no error)=w2761) -> ()  [unwired: 1 out]
      }
      frame "Set WTD" {
        n1625 = Unbundle By Name(w2763) -> ("Motion Module.Set WTD"=w2766:refnum<vi>)
        n1626 = property on="Property Node" class="Bool (strict)"(reference=w2766, "Value"=FALSE) -> (reference out=w2768:refnum<vi>, error out=w2767:errorcluster)  [unwired: 1 in]
        n1627 = call "DATA ENCRYPT STRING FILE WRITE.vi"("error in (no error)"=w2770, "User Action"="User Pressed  on Set Wear Track", "main ref"=w2763) -> ("error out"=w2769:errorcluster)  [unwired: 6 in, 1 out]
        n1628 = call "Sway wear trac set.vi"("error in (no error)"=w2769, "main ref"=w2763) -> ("error out"=w2764:errorcluster)  [unwired: 9 in]
        n1629 = Close Reference(reference=w2768, error in (no error)=w2767) -> ()  [unwired: 1 out]
      }
      frame "Import 2" {
        n1630 = call "File Dialog"("start path"=path "C:/LAB-IQ 150/User Defined Protocol", "error in"=w2779) -> ("selected path"=w2773:path, "cancelled"=w2776:bool, "error out"=w2778:errorcluster)  [unwired: 10 in, 1 out]
        n1631 = call <vilib>:"Clear Errors.vi"("error in (no error)"=w2778) -> ("error out"=w2775:errorcluster)  [unwired: 5 in, 1 out]
        n1632 = case shown="False" w2776 {
          tunnel: w2775 -> [w2789 w2790]
          tunnel: [w2781 w2790] -> w2774
          tunnel: w2773 -> [w2788 _]
          tunnel: w2772 -> [w2783 _]
          frame False {
            n1633 = call-poly <vilib>:"Read Delimited Spreadsheet.vi"("file path (dialog if empty)"=w2788, "error in (no error)"=w2789, "delimiter (\\t)"=":" ("delimiter (\\t)")) -> ("all rows"=w2780:string[][], "error out"=w2782:errorcluster)  [unwired: 7 in, 4 out]
            n1634 = Unbundle By Name(w2783) -> ("Motion Module.StepTable For Speed"=w2786:refnum<vi>)
            n1635 = property on="Property Node" class="Tbl (strict)"(reference=w2786, error in=w2782, "Value"=w2780) -> (reference out=w2784:refnum<vi>, error out=w2785:errorcluster)
            n1636 = Close Reference(reference=w2784, error in (no error)=w2785) -> (error out=w2781:errorcluster)
          }
          frame True {
          }
        }
      }
      frame "Import 3" {
        n1637 = call "File Dialog7"("start path"=path "C:/LAB-IQ 150/User Defined Protocol", "error in"=w2799) -> ("selected path"=w2793:path, "cancelled"=w2796:bool, "error out"=w2798:errorcluster)  [unwired: 10 in, 1 out]
        n1638 = call <vilib>:"Clear Errors.vi"("error in (no error)"=w2798) -> ("error out"=w2795:errorcluster)  [unwired: 5 in, 1 out]
        n1639 = local write "Import 3"(FALSE ("Import 3")) -> ()
        n1640 = case shown="False" w2796 {
          tunnel: w2795 -> [w2809 w2810]
          tunnel: [w2801 w2810] -> w2794
          tunnel: w2793 -> [w2808 _]
          tunnel: w2792 -> [w2803 _]
          frame False {
            n1641 = call-poly <vilib>:"Read Delimited Spreadsheet.vi"("file path (dialog if empty)"=w2808, "error in (no error)"=w2809, "delimiter (\\t)"=":" ("delimiter (\\t)")) -> ("all rows"=w2800:string[][], "error out"=w2802:errorcluster)  [unwired: 7 in, 4 out]
            n1642 = Unbundle By Name(w2803) -> ("Loading.Stribeck Table  For loading"=w2806:refnum<vi>)
            n1643 = property on="Property Node" class="Tbl (strict)"(reference=w2806, error in=w2802, "Value"=w2800) -> (reference out=w2804:refnum<vi>, error out=w2805:errorcluster)
            n1644 = Close Reference(reference=w2804, error in (no error)=w2805) -> (error out=w2801:errorcluster)
          }
          frame True {
          }
        }
      }
      frame "Save 2" {
        n1645 = Unbundle By Name(w2814) -> ("Motion Module.StepTable For Speed"=w2829:refnum<vi>)
        n1646 = property on="Property Node" class="Tbl (strict)"(reference=w2829) -> (reference out=w2827:refnum<vi>, error out=w2828:errorcluster, "Value"=w2825:string[][])  [unwired: 1 in]
        n1647 = call "File Dialog2"("start path"=path "C:/LAB-IQ 150/User Defined Protocol", "error in"=w2819) -> ("selected path"=w2822:path, "error out"=w2821:errorcluster)  [unwired: 10 in, 2 out]
        n1648 = call <vilib>:"Clear Errors.vi"("error in (no error)"=w2821) -> ("error out"=w2820:errorcluster)  [unwired: 5 in, 1 out]
        n1649 = Close Reference(reference=w2827, error in (no error)=w2828) -> ()  [unwired: 1 out]
        n1650 = call-poly <vilib>:"Write Delimited Spreadsheet.vi"("file path (dialog if empty)"=w2822, "2D data"=w2825, "append to file? (new file:F)"=TRUE, "error in (no error)"=w2820, "delimiter (\\t)"=":" ("delimiter (\\t)")) -> ("error out"=w2818:errorcluster)  [unwired: 9 in, 1 out]
        n1651 = call <vilib>:"Clear Errors.vi"("error in (no error)"=w2818) -> ("error out"=w2813:errorcluster)  [unwired: 5 in, 1 out]
        n1652 = Unbundle By Name(w2814) -> ("Motion Module.Save 2"=w2815:refnum<vi>)
        n1653 = property on="Property Node" class="Bool (strict)"(reference=w2815, error in=w2813, "Value"=FALSE) -> (reference out=w2817:refnum<vi>, error out=w2816:errorcluster)
        n1654 = Close Reference(reference=w2817, error in (no error)=w2816) -> (error out=w2812:errorcluster)
      }
      frame "Save 3" {
        n1655 = Unbundle By Name(w2832) -> ("Loading.Stribeck Table  For loading"=w2844:refnum<vi>)
        n1656 = property on="Property Node" class="Tbl (strict)"(reference=w2844) -> (reference out=w2842:refnum<vi>, error out=w2843:errorcluster, "Value"=w2840:string[][])  [unwired: 1 in]
        n1657 = call "File Dialog8"("start path"=path "C:/LAB-IQ 150/User Defined Protocol", "error in"=w2834) -> ("selected path"=w2837:path, "error out"=w2836:errorcluster)  [unwired: 10 in, 2 out]
        n1658 = call <vilib>:"Clear Errors.vi"("error in (no error)"=w2836) -> ("error out"=w2835:errorcluster)  [unwired: 5 in, 1 out]
        n1659 = Close Reference(reference=w2842, error in (no error)=w2843) -> ()  [unwired: 1 out]
        n1660 = call-poly <vilib>:"Write Delimited Spreadsheet.vi"("file path (dialog if empty)"=w2837, "2D data"=w2840, "append to file? (new file:F)"=TRUE, "error in (no error)"=w2835, "delimiter (\\t)"=":" ("delimiter (\\t)")) -> ("error out"=w2833:errorcluster)  [unwired: 9 in, 1 out]
        n1661 = call <vilib>:"Clear Errors.vi"("error in (no error)"=w2833) -> ("error out"=w2831:errorcluster)  [unwired: 5 in, 1 out]
        n1662 = local write "Save 3"(FALSE ("Value")) -> ()
      }
      frame "Calculate Rotary" {
        n1663 = call "STEP LOAD MM_SEC AND RPM CONVERSION.vi"("error in (no error)"=w2848, "Data Cluster"=w2846) -> ("error out"=w2847:errorcluster)  [unwired: 9 in]
        n1664 = local write "calculate rotary"(FALSE) -> ()
      }
      frame "Clear List" {
        n1665 = Unbundle By Name(w2850) -> ("Environmental control.Sensors Picked"=w2857:refnum<vi>)
        n1666 = Unbundle By Name(w2850) -> ("Environmental control.Clear List"=w2851:refnum<vi>)
        n1667 = property on="Property Node" class="Bool (strict)"(reference=w2851, "Value"=FALSE) -> (reference out=w2853:refnum<vi>, error out=w2852:errorcluster)  [unwired: 1 in]
        n1668 = property on="Property Node" class="Str"(reference=w2857, "Value"="") -> (reference out=w2855:refnum<vi>, error out=w2856:errorcluster)  [unwired: 1 in]
        n1669 = Close Reference(reference=w2853, error in (no error)=w2852) -> ()  [unwired: 1 out]
        n1670 = Close Reference(reference=w2855, error in (no error)=w2856) -> ()  [unwired: 1 out]
      }
      frame "ClrLog" {
        n1671 = Unbundle By Name(w2860) -> ("Main Screen.ClrLog"=w2861:refnum<vi>)
        n1672 = Unbundle By Name(w2860) -> ("Main Screen.Trip Log"=w2867:refnum<vi>)
        n1673 = property on="Property Node" class="Bool (strict)"(reference=w2861, "Value"=FALSE) -> (reference out=w2863:refnum<vi>, error out=w2862:errorcluster)  [unwired: 1 in]
        n1674 = property on="Property Node" class="Str"(reference=w2867, "Value"="") -> (reference out=w2865:refnum<vi>, error out=w2866:errorcluster)  [unwired: 1 in]
        n1675 = Close Reference(reference=w2863, error in (no error)=w2862) -> ()  [unwired: 1 out]
        n1676 = Close Reference(reference=w2865, error in (no error)=w2866) -> ()  [unwired: 1 out]
      }
      frame "Add to list" {
        n1677 = Unbundle By Name(w2869) -> ("Environmental control.Sensors Picked"=w2875:refnum<vi>)
        n1678 = property on="Property Node" class="Str"(reference=w2875, error in=w2870, "Value"="") -> (reference out=w2873:refnum<vi>, error out=w2874:errorcluster)
        n1679 = Close Reference(reference=w2873, error in (no error)=w2874) -> (error out=w2871:errorcluster)
        n1680 = call "Add  to List Loop.vi"("error in (no error)"=w2871, "Data Cluster"=w2869) -> ("error out"=w2877:errorcluster)  [unwired: 9 in]
        n1681 = Unbundle By Name(w2869) -> ("Environmental control.Add to list"=w2879:refnum<vi>)
        n1682 = property on="Property Node" class="Bool (strict)"(reference=w2879, error in=w2877, "Value"=FALSE) -> (reference out=w2881:refnum<vi>, error out=w2880:errorcluster)
        n1683 = Close Reference(reference=w2881, error in (no error)=w2880) -> (error out=w2876:errorcluster)
      }
      frame "Disable Axis Jog Soft Limits" {
        n1684 = call "DATA ENCRYPT STRING FILE WRITE.vi"("error in (no error)"=w2885, "User Action"="User Pressed Disable Axis Jog Soft Limits in Main Screen", "main ref"=w2883) -> ("error out"=w2884:errorcluster)  [unwired: 6 in, 1 out]
      }
      frame "Home Service" {
        n1685 = Unbundle By Name(w2887) -> ("Main Home Screen.MainPage"=w2893:refnum<vi>)
        n1686 = Unbundle By Name(w2887) -> ("Main Home Screen.GUI"=w2891:refnum<vi>)
        n1687 = local write "Home Service"(FALSE ("Home Service")) -> ()
        n1688 = property on="Property Node" class="TabCtl (strict)"(reference=w2893, "Value"=T15."HOME") -> (reference out=w2895:refnum<vi>, error out=w2894:errorcluster)  [unwired: 1 in]
        n1689 = property on="Property Node" class="TabCtl (strict)"(reference=w2891, "Value"=T14."Setup") -> (reference out=w2889:refnum<vi>, error out=w2890:errorcluster)  [unwired: 1 in]
        n1690 = Close Reference(reference=w2895, error in (no error)=w2894) -> ()  [unwired: 1 out]
        n1691 = Close Reference(reference=w2889, error in (no error)=w2890) -> ()  [unwired: 1 out]
        n1692 = call "DATA ENCRYPT STRING FILE WRITE.vi"("error in (no error)"=w2898, "User Action"="User Pressed Home Service from Service Screen", "main ref"=w2887) -> ("error out"=w2897:errorcluster)  [unwired: 6 in, 1 out]
      }
      frame "Analysis Home" {
        n1693 = Unbundle By Name(w2900) -> ("Main Screen.Main Screen Tab"=w2903:refnum<vi>)
        n1694 = Unbundle By Name(w2900) -> ("Main Home Screen.MainPage"=w2910:refnum<vi>)
        n1695 = Unbundle By Name(w2900) -> ("Main Home Screen.GUI"=w2908:refnum<vi>)
        n1696 = local write "Analysis Home new"(FALSE ("Analysis Home new")) -> ()
        n1697 = property on="Property Node" class="TabCtl (strict)"(reference=w2903, "Value"=T18."  Acquire  ") -> (reference out=w2901:refnum<vi>, error out=w2902:errorcluster)  [unwired: 1 in]
        n1698 = property on="Property Node" class="TabCtl (strict)"(reference=w2910, "Value"=T15."HOME") -> (reference out=w2912:refnum<vi>, error out=w2911:errorcluster)  [unwired: 1 in]
        n1699 = property on="Property Node" class="TabCtl (strict)"(reference=w2908, "Value"=T14."Setup") -> (reference out=w2906:refnum<vi>, error out=w2907:errorcluster)  [unwired: 1 in]
        n1700 = Close Reference(reference=w2901, error in (no error)=w2902) -> ()  [unwired: 1 out]
        n1701 = Close Reference(reference=w2912, error in (no error)=w2911) -> ()  [unwired: 1 out]
        n1702 = Close Reference(reference=w2906, error in (no error)=w2907) -> ()  [unwired: 1 out]
        n1703 = call "DATA ENCRYPT STRING FILE WRITE.vi"("error in (no error)"=w2915, "User Action"="User Pressed Home from AnalysisScreen", "main ref"=w2900) -> ("error out"=w2914:errorcluster)  [unwired: 6 in, 1 out]
      }
      frame "Post Analysis" {
        n1704 = Unbundle By Name(w2918) -> ("Main Screen.Main Screen Tab"=w2921:refnum<vi>)
        n1705 = Unbundle By Name(w2918) -> ("Main Home Screen.MainPage"=w2927:refnum<vi>)
        n1706 = Unbundle By Name(w2918) -> ("Main Home Screen.GUI"=w2925:refnum<vi>)
        n1707 = property on="Property Node" class="TabCtl (strict)"(reference=w2921, "Value"=T18."Compare Files Rot") -> (reference out=w2919:refnum<vi>, error out=w2920:errorcluster)  [unwired: 1 in]
        n1708 = property on="Property Node" class="TabCtl (strict)"(reference=w2927, "Value"=T15."HOME") -> (reference out=w2929:refnum<vi>, error out=w2928:errorcluster)  [unwired: 1 in]
        n1709 = property on="Property Node" class="TabCtl (strict)"(reference=w2925, "Value"=T14."Begin") -> (reference out=w2923:refnum<vi>, error out=w2924:errorcluster)  [unwired: 1 in]
        n1710 = local write "Post Analysis"(FALSE ("Post Analysis")) -> ()
        n1711 = Close Reference(reference=w2919, error in (no error)=w2920) -> ()  [unwired: 1 out]
        n1712 = Close Reference(reference=w2929, error in (no error)=w2928) -> ()  [unwired: 1 out]
        n1713 = Close Reference(reference=w2923, error in (no error)=w2924) -> ()  [unwired: 1 out]
        n1714 = call "DATA ENCRYPT STRING FILE WRITE.vi"("error in (no error)"=w2932, "User Action"="User Pressed Post Analysis ", "main ref"=w2918) -> ("error out"=w2931:errorcluster)  [unwired: 6 in, 1 out]
      }
      frame "Edit Gain Constants" {
        n1715 = Unbundle By Name(w2934) -> ("About Screen.Heave and Surge COM Port:"=w2964:refnum<vi>)
        n1716 = Unbundle By Name(w2934) -> ("About Screen.Edit Gain Constants"=w2944:refnum<vi>)
        n1717 = Unbundle By Name(w2934) -> ("About Screen.Sway COM Port:"=w2961:refnum<vi>)
        n1718 = Unbundle By Name(w2934) -> ("About Screen.Ramp Port:"=w2938:refnum<vi>)
        n1719 = Unbundle By Name(w2934) -> ("About Screen.Temp Modbus:"=w2958:refnum<vi>)
        n1720 = Unbundle By Name(w2934) -> ("About Screen.Humidity Port:"=w2957:refnum<vi>)
        n1721 = Unbundle By Name(w2934) -> ("About Screen.Password"=w2952:refnum<vi>)
        n1722 = Unbundle By Name(w2934) -> ("About Screen.ECR Port:"=w2937:refnum<vi>)
        n1723 = property on="Property Node" class="VISAName"(reference=w2938, "DisabledEnum"=T31."Enabled" ("Disabled")) -> (reference out=w2940:refnum<vi>, error out=w2939:errorcluster)  [unwired: 1 in]
        n1724 = property on="Property Node" class="Bool (strict)"(reference=w2944, "Value"=FALSE) -> (reference out=w2945:refnum<vi>, error out=w2943:errorcluster)  [unwired: 1 in]
        n1725 = property on="Property Node" class="VISAName"(reference=w2937, "DisabledEnum"=T31."Enabled" ("Disabled")) -> (reference out=w2933:refnum<vi>, error out=w2936:errorcluster)  [unwired: 1 in]
        n1726 = property on="Property Node" class="VISAName"(reference=w2964, "DisabledEnum"=T31."Enabled" ("Disabled")) -> (reference out=w2965:refnum<vi>, error out=w2963:errorcluster)  [unwired: 1 in]
        n1727 = property on="Property Node" class="VISAName"(reference=w2961, "DisabledEnum"=T31."Enabled" ("Disabled")) -> (reference out=w2962:refnum<vi>, error out=w2960:errorcluster)  [unwired: 1 in]
        n1728 = property on="Property Node" class="VISAName"(reference=w2958, "DisabledEnum"=T31."Enabled" ("Disabled")) -> (reference out=w2946:refnum<vi>, error out=w2959:errorcluster)  [unwired: 1 in]
        n1729 = property on="Property Node" class="VISAName"(reference=w2957, "DisabledEnum"=T31."Enabled" ("Disabled")) -> (reference out=w2955:refnum<vi>, error out=w2956:errorcluster)  [unwired: 1 in]
        n1730 = property on="Property Node" class="Str"(reference=w2952, "Visible"=FALSE) -> (reference out=w2954:refnum<vi>, error out=w2953:errorcluster)  [unwired: 1 in]
        n1731 = Close Reference(reference=w2940, error in (no error)=w2939) -> ()  [unwired: 1 out]
        n1732 = Close Reference(reference=w2954, error in (no error)=w2953) -> ()  [unwired: 1 out]
        n1733 = Close Reference(reference=w2933, error in (no error)=w2936) -> ()  [unwired: 1 out]
        n1734 = Close Reference(reference=w2945, error in (no error)=w2943) -> ()  [unwired: 1 out]
        n1735 = Close Reference(reference=w2965, error in (no error)=w2963) -> ()  [unwired: 1 out]
        n1736 = Close Reference(reference=w2962, error in (no error)=w2960) -> ()  [unwired: 1 out]
        n1737 = Close Reference(reference=w2946, error in (no error)=w2959) -> ()  [unwired: 1 out]
        n1738 = Close Reference(reference=w2955, error in (no error)=w2956) -> ()  [unwired: 1 out]
        n1739 = call "DATA ENCRYPT STRING FILE WRITE.vi"("error in (no error)"=w2968, "User Action"="User Pressed Home Service from Service Screen", "main ref"=w2934) -> ("error out"=w2967:errorcluster)  [unwired: 6 in, 1 out]
      }
      frame "Advanced Setting" {
        n1740 = Unbundle By Name(w2970) -> ("About Screen.Advanced Setting"=w2972:refnum<vi>)
        n1741 = property on="Property Node" class="Bool (strict)"(reference=w2972) -> (reference out=w2973:refnum<vi>, error out=w2971:errorcluster, "Value"=w2969:bool)  [unwired: 1 in]
        n1742 = Close Reference(reference=w2973, error in (no error)=w2971) -> ()  [unwired: 1 out]
        n1743 = case shown="True" w2969 {
          tunnel: w2970 -> [w2978 w3003]
          frame True {
            n1744 = Unbundle By Name(w2978) -> ("About Screen.Heave and Surge COM Port:"=w3000:refnum<vi>)
            n1745 = Unbundle By Name(w2978) -> ("About Screen.Edit Gain Constants"=w2980:refnum<vi>)
            n1746 = Unbundle By Name(w2978) -> ("About Screen.Sway COM Port:"=w2997:refnum<vi>)
            n1747 = Unbundle By Name(w2978) -> ("About Screen.Temp Modbus:"=w2994:refnum<vi>)
            n1748 = Unbundle By Name(w2978) -> ("About Screen.Humidity Port:"=w2993:refnum<vi>)
            n1749 = Unbundle By Name(w2978) -> ("About Screen.Password"=w2988:refnum<vi>)
            n1750 = property on="Property Node" class="Bool (strict)"(reference=w2980, "Value"=FALSE) -> (reference out=w2981:refnum<vi>, error out=w2979:errorcluster)  [unwired: 1 in]
            n1751 = property on="Property Node" class="VISAName"(reference=w3000, "DisabledEnum"=T31."Disabled and Grayed Out" ("Disabled")) -> (reference out=w3001:refnum<vi>, error out=w2999:errorcluster)  [unwired: 1 in]
            n1752 = property on="Property Node" class="VISAName"(reference=w2997, "DisabledEnum"=T31."Disabled and Grayed Out" ("Disabled")) -> (reference out=w2998:refnum<vi>, error out=w2996:errorcluster)  [unwired: 1 in]
            n1753 = property on="Property Node" class="VISAName"(reference=w2994, "DisabledEnum"=T31."Disabled and Grayed Out" ("Disabled")) -> (reference out=w2982:refnum<vi>, error out=w2995:errorcluster)  [unwired: 1 in]
            n1754 = property on="Property Node" class="VISAName"(reference=w2993, "DisabledEnum"=T31."Disabled and Grayed Out" ("Disabled")) -> (reference out=w2991:refnum<vi>, error out=w2992:errorcluster)  [unwired: 1 in]
            n1755 = property on="Property Node" class="Str"(reference=w2988, "Visible"=TRUE) -> (reference out=w2990:refnum<vi>, error out=w2989:errorcluster)  [unwired: 1 in]
            n1756 = Close Reference(reference=w2981, error in (no error)=w2979) -> ()  [unwired: 1 out]
            n1757 = Close Reference(reference=w3001, error in (no error)=w2999) -> ()  [unwired: 1 out]
            n1758 = Close Reference(reference=w2998, error in (no error)=w2996) -> ()  [unwired: 1 out]
            n1759 = Close Reference(reference=w2982, error in (no error)=w2995) -> ()  [unwired: 1 out]
            n1760 = Close Reference(reference=w2991, error in (no error)=w2992) -> ()  [unwired: 1 out]
            n1761 = Close Reference(reference=w2990, error in (no error)=w2989) -> ()  [unwired: 1 out]
          }
          frame False {
            n1762 = Unbundle By Name(w3003) -> ("About Screen.Heave and Surge COM Port:"=w3025:refnum<vi>)
            n1763 = Unbundle By Name(w3003) -> ("About Screen.Edit Gain Constants"=w3005:refnum<vi>)
            n1764 = Unbundle By Name(w3003) -> ("About Screen.Sway COM Port:"=w3022:refnum<vi>)
            n1765 = Unbundle By Name(w3003) -> ("About Screen.Temp Modbus:"=w3019:refnum<vi>)
            n1766 = Unbundle By Name(w3003) -> ("About Screen.Humidity Port:"=w3018:refnum<vi>)
            n1767 = Unbundle By Name(w3003) -> ("About Screen.Password"=w3013:refnum<vi>)
            n1768 = property on="Property Node" class="Bool (strict)"(reference=w3005, "Value"=FALSE) -> (reference out=w3006:refnum<vi>, error out=w3004:errorcluster)  [unwired: 1 in]
            n1769 = property on="Property Node" class="VISAName"(reference=w3025, "DisabledEnum"=T31."Disabled and Grayed Out" ("Disabled")) -> (reference out=w3026:refnum<vi>, error out=w3024:errorcluster)  [unwired: 1 in]
            n1770 = property on="Property Node" class="VISAName"(reference=w3022, "DisabledEnum"=T31."Disabled and Grayed Out" ("Disabled")) -> (reference out=w3023:refnum<vi>, error out=w3021:errorcluster)  [unwired: 1 in]
            n1771 = property on="Property Node" class="VISAName"(reference=w3019, "DisabledEnum"=T31."Disabled and Grayed Out" ("Disabled")) -> (reference out=w3007:refnum<vi>, error out=w3020:errorcluster)  [unwired: 1 in]
            n1772 = property on="Property Node" class="VISAName"(reference=w3018, "DisabledEnum"=T31."Disabled and Grayed Out" ("Disabled")) -> (reference out=w3016:refnum<vi>, error out=w3017:errorcluster)  [unwired: 1 in]
            n1773 = property on="Property Node" class="Str"(reference=w3013, "Visible"=FALSE) -> (reference out=w3015:refnum<vi>, error out=w3014:errorcluster)  [unwired: 1 in]
            n1774 = Close Reference(reference=w3006, error in (no error)=w3004) -> ()  [unwired: 1 out]
            n1775 = Close Reference(reference=w3026, error in (no error)=w3024) -> ()  [unwired: 1 out]
            n1776 = Close Reference(reference=w3023, error in (no error)=w3021) -> ()  [unwired: 1 out]
            n1777 = Close Reference(reference=w3007, error in (no error)=w3020) -> ()  [unwired: 1 out]
            n1778 = Close Reference(reference=w3016, error in (no error)=w3017) -> ()  [unwired: 1 out]
            n1779 = Close Reference(reference=w3015, error in (no error)=w3014) -> ()  [unwired: 1 out]
          }
        }
        n1780 = call "DATA ENCRYPT STRING FILE WRITE.vi"("error in (no error)"=w2976, "User Action"="User Pressed Advance Setting in Service Screen", "main ref"=w2970) -> ("error out"=w2975:errorcluster)  [unwired: 6 in, 1 out]
      }
      frame "Password" {
        n1781 = Unbundle By Name(w3027) -> ("About Screen.Password"=w3033:refnum<vi>)
        n1782 = property on="Property Node" class="Str"(reference=w3033) -> (reference out=w3034:refnum<vi>, error out=w3032:errorcluster, "Value"=w3031:string)  [unwired: 1 in]
        n1783 = call <vilib>:"Trim Whitespace.vi"("string"=w3031) -> ("trimmed string"=w3030:string)  [unwired: 1 in]
        n1784 = Close Reference(reference=w3034, error in (no error)=w3032) -> ()  [unwired: 1 out]
        n1785 = Equal?(x=w3030, y="UT150$") -> (x = y?=w3028:bool)
        n1786 = case shown="True" w3028 {
          tunnel: w3027 -> [_ w3037]
          frame False {
          }
          frame True {
            n1787 = Unbundle By Name(w3037) -> ("Main Screen.Main Screen Tab"=w3039:refnum<vi>)
            n1788 = Unbundle By Name(w3037) -> ("Main Home Screen.GUI"=w3043:refnum<vi>)
            n1789 = Unbundle By Name(w3037) -> ("About Screen.Password"=w3047:refnum<vi>)
            n1790 = property on="Property Node" class="TabCtl (strict)"(reference=w3043, "Value"=T14."Begin") -> (reference out=w3044:refnum<vi>, error out=w3042:errorcluster)  [unwired: 1 in]
            n1791 = property on="Property Node" class="TabCtl (strict)"(reference=w3039, "Value"=T18."Service") -> (reference out=w3038:refnum<vi>, error out=w3040:errorcluster)  [unwired: 1 in]
            n1792 = property on="Property Node" class="Str"(reference=w3047, "Value"="") -> (reference out=w3048:refnum<vi>, error out=w3046:errorcluster)  [unwired: 1 in]
            n1793 = Close Reference(reference=w3048, error in (no error)=w3046) -> ()  [unwired: 1 out]
            n1794 = Close Reference(reference=w3044, error in (no error)=w3042) -> ()  [unwired: 1 out]
            n1795 = Close Reference(reference=w3038, error in (no error)=w3040) -> ()  [unwired: 1 out]
          }
        }
      }
      frame "Service About" {
        n1796 = Unbundle By Name(w3050) -> ("Main Screen.Main Screen Tab"=w3053:refnum<vi>)
        n1797 = Unbundle By Name(w3050) -> ("Main Home Screen.GUI"=w3057:refnum<vi>)
        n1798 = local write "Service About"(FALSE ("Service About")) -> ()
        n1799 = property on="Property Node" class="TabCtl (strict)"(reference=w3057, "Value"=T14."Begin") -> (reference out=w3058:refnum<vi>, error out=w3056:errorcluster)  [unwired: 1 in]
        n1800 = property on="Property Node" class="TabCtl (strict)"(reference=w3053, "Value"=T18."About") -> (reference out=w3052:refnum<vi>, error out=w3054:errorcluster)  [unwired: 1 in]
        n1801 = Close Reference(reference=w3058, error in (no error)=w3056) -> ()  [unwired: 1 out]
        n1802 = Close Reference(reference=w3052, error in (no error)=w3054) -> ()  [unwired: 1 out]
      }
      frame "OPEN 1" {
        n1803 = Unbundle By Name(w3062) -> ("Analysis Screen.File 1 Discription"=w3071:refnum<vi>)
        n1804 = property on="Property Node" class="Str"(reference=w3071, error in=w3069, "Value"="") -> (reference out=w3072:refnum<vi>, error out=w3070:errorcluster)
        n1805 = Close Reference(reference=w3072, error in (no error)=w3070) -> (error out=w3068:errorcluster)
        n1806 = call <vilib>:"Application Directory.vi"() -> ("Application Directory"=w3076:path)
        n1807 = Unbundle By Name(w3062) -> ("Analysis Screen.OPEN 1"=w3064:refnum<vi>)
        n1808 = Build Path(base path=w3076, name or relative path="data") -> (appended path=w3074:path)
        n1809 = property on="Property Node" class="Bool (strict)"(reference=w3064, "Value"=FALSE) -> (reference out=w3065:refnum<vi>, error out=w3063:errorcluster)  [unwired: 1 in]
        n1810 = call "File Dialog3"("start path"=w3074, "error in"=w3068) -> ("selected path"=w3073:path, "cancelled"=w3060:bool, "error out"=w3077:errorcluster)  [unwired: 10 in, 1 out]
        n1811 = case shown="True" w3060 {
          tunnel: w3077 -> [w3091 _]
          tunnel: w3073 -> [w3087 _]
          tunnel: [w3079 _] -> w3066
          tunnel: w3062 -> [w3078 w3093]
          frame False {
            n1812 = Path To String(path=w3087) -> (string=w3086:string)
            n1813 = Unbundle By Name(w3078) -> ("Analysis Screen.File Name 1"=w3089:refnum<vi>)
            n1814 = call <vilib>:"Clear Errors.vi"("error in (no error)"=w3091) -> ("error out"=w3085:errorcluster)  [unwired: 5 in, 1 out]
            n1815 = property on="Property Node" class="Str"(reference=w3089, "Value"=w3086) -> (reference out=w3090:refnum<vi>, error out=w3088:errorcluster)  [unwired: 1 in]
            n1816 = call "INI FILE READ.vi"("error in (no error)"=w3085, "File Path"=w3086) -> ("error out"=w3081:errorcluster, "concatenated string"=w3080:string)  [unwired: 8 in]
            n1817 = Unbundle By Name(w3078) -> ("Analysis Screen.File 1 Discription"=w3083:refnum<vi>)
            n1818 = Close Reference(reference=w3090, error in (no error)=w3088) -> ()  [unwired: 1 out]
            n1819 = property on="Property Node" class="Str"(reference=w3083, error in=w3081, "Value"=w3080) -> (reference out=w3084:refnum<vi>, error out=w3082:errorcluster)
            n1820 = Close Reference(reference=w3084, error in (no error)=w3082) -> (error out=w3079:errorcluster)
          }
          frame True {
            n1821 = Unbundle By Name(w3093) -> ("Analysis Screen.File 1 Discription"=w3095:refnum<vi>)
            n1822 = Unbundle By Name(w3093) -> ("Analysis Screen.File Name 1"=w3099:refnum<vi>)
            n1823 = property on="Property Node" class="Str"(reference=w3095, "Value"="") -> (reference out=w3096:refnum<vi>, error out=w3094:errorcluster)  [unwired: 1 in]
            n1824 = property on="Property Node" class="Str"(reference=w3099, "Value"="") -> (reference out=w3100:refnum<vi>, error out=w3098:errorcluster)  [unwired: 1 in]
            n1825 = Close Reference(reference=w3096, error in (no error)=w3094) -> ()  [unwired: 1 out]
            n1826 = Close Reference(reference=w3100, error in (no error)=w3098) -> ()  [unwired: 1 out]
          }
        }
        n1827 = Close Reference(reference=w3065, error in (no error)=w3063) -> ()  [unwired: 1 out]
      }
      frame "OPEN 2" {
        n1828 = Unbundle By Name(w3103) -> ("Analysis Screen.File 2 Discription"=w3112:refnum<vi>)
        n1829 = property on="Property Node" class="Str"(reference=w3112, error in=w3110, "Value"="") -> (reference out=w3113:refnum<vi>, error out=w3111:errorcluster)
        n1830 = Close Reference(reference=w3113, error in (no error)=w3111) -> (error out=w3109:errorcluster)
        n1831 = call <vilib>:"Application Directory.vi"() -> ("Application Directory"=w3117:path)
        n1832 = Unbundle By Name(w3103) -> ("Analysis Screen.OPEN 2"=w3105:refnum<vi>)
        n1833 = Build Path(base path=w3117, name or relative path="data") -> (appended path=w3115:path)
        n1834 = property on="Property Node" class="Bool (strict)"(reference=w3105, "Value"=FALSE) -> (reference out=w3106:refnum<vi>, error out=w3104:errorcluster)  [unwired: 1 in]
        n1835 = call "File Dialog4"("start path"=w3115, "error in"=w3109) -> ("selected path"=w3114:path, "cancelled"=w3101:bool, "error out"=w3118:errorcluster)  [unwired: 10 in, 1 out]
        n1836 = case shown="True" w3101 {
          tunnel: w3118 -> [w3132 w3134]
          tunnel: w3114 -> [w3128 _]
          tunnel: [w3120 w3133] -> w3107
          tunnel: w3103 -> [w3119 w3136]
          frame False {
            n1837 = Path To String(path=w3128) -> (string=w3127:string)
            n1838 = Unbundle By Name(w3119) -> ("Analysis Screen.File Name 2"=w3130:refnum<vi>)
            n1839 = call <vilib>:"Clear Errors.vi"("error in (no error)"=w3132) -> ("error out"=w3126:errorcluster)  [unwired: 5 in, 1 out]
            n1840 = property on="Property Node" class="Str"(reference=w3130, "Value"=w3127) -> (reference out=w3131:refnum<vi>, error out=w3129:errorcluster)  [unwired: 1 in]
            n1841 = call "INI FILE READ.vi"("error in (no error)"=w3126, "File Path"=w3127) -> ("error out"=w3122:errorcluster, "concatenated string"=w3121:string)  [unwired: 8 in]
            n1842 = Unbundle By Name(w3119) -> ("Analysis Screen.File 2 Discription"=w3124:refnum<vi>)
            n1843 = Close Reference(reference=w3131, error in (no error)=w3129) -> ()  [unwired: 1 out]
            n1844 = property on="Property Node" class="Str"(reference=w3124, error in=w3122, "Value"=w3121) -> (reference out=w3125:refnum<vi>, error out=w3123:errorcluster)
            n1845 = Close Reference(reference=w3125, error in (no error)=w3123) -> (error out=w3120:errorcluster)
          }
          frame True {
            n1846 = Unbundle By Name(w3136) -> ("Analysis Screen.File Name 2"=w3142:refnum<vi>)
            n1847 = Unbundle By Name(w3136) -> ("Analysis Screen.File 2 Discription"=w3138:refnum<vi>)
            n1848 = property on="Property Node" class="Str"(reference=w3142, "Value"="") -> (reference out=w3143:refnum<vi>, error out=w3141:errorcluster)  [unwired: 1 in]
            n1849 = property on="Property Node" class="Str"(reference=w3138, "Value"="") -> (reference out=w3137:refnum<vi>, error out=w3139:errorcluster)  [unwired: 1 in]
            n1850 = call <vilib>:"Clear Errors.vi"("error in (no error)"=w3134) -> ("error out"=w3133:errorcluster)  [unwired: 5 in, 1 out]
            n1851 = Close Reference(reference=w3137, error in (no error)=w3139) -> ()  [unwired: 1 out]
            n1852 = Close Reference(reference=w3143, error in (no error)=w3141) -> ()  [unwired: 1 out]
          }
        }
        n1853 = Close Reference(reference=w3106, error in (no error)=w3104) -> ()  [unwired: 1 out]
      }
      frame "OPEN 3" {
        # "3416\n4017\n4554"
        n1854 = Unbundle By Name(w3146) -> ("Analysis Screen.File 3 Discription"=w3155:refnum<vi>)
        n1855 = property on="Property Node" class="Str"(reference=w3155, error in=w3153, "Value"="") -> (reference out=w3156:refnum<vi>, error out=w3154:errorcluster)
        n1856 = Close Reference(reference=w3156, error in (no error)=w3154) -> (error out=w3152:errorcluster)
        n1857 = call <vilib>:"Application Directory.vi"() -> ("Application Directory"=w3160:path)
        n1858 = Unbundle By Name(w3146) -> ("Analysis Screen.OPEN 3"=w3148:refnum<vi>)
        n1859 = Build Path(base path=w3160, name or relative path="data") -> (appended path=w3158:path)
        n1860 = property on="Property Node" class="Bool (strict)"(reference=w3148, "Value"=FALSE) -> (reference out=w3149:refnum<vi>, error out=w3147:errorcluster)  [unwired: 1 in]
        n1861 = call "File Dialog5"("start path"=w3158, "error in"=w3152) -> ("selected path"=w3157:path, "cancelled"=w3144:bool, "error out"=w3161:errorcluster)  [unwired: 10 in, 1 out]
        n1862 = case shown="True" w3144 {
          tunnel: w3161 -> [w3175 w3177]
          tunnel: w3157 -> [w3171 _]
          tunnel: [w3163 w3176] -> w3150
          tunnel: w3146 -> [w3162 w3179]
          frame False {
            n1863 = Path To String(path=w3171) -> (string=w3170:string)
            n1864 = Unbundle By Name(w3162) -> ("Analysis Screen.File Name 3"=w3173:refnum<vi>)
            n1865 = call <vilib>:"Clear Errors.vi"("error in (no error)"=w3175) -> ("error out"=w3169:errorcluster)  [unwired: 5 in, 1 out]
            n1866 = property on="Property Node" class="Str"(reference=w3173, "Value"=w3170) -> (reference out=w3174:refnum<vi>, error out=w3172:errorcluster)  [unwired: 1 in]
            n1867 = call "INI FILE READ.vi"("error in (no error)"=w3169, "File Path"=w3170) -> ("error out"=w3165:errorcluster, "concatenated string"=w3164:string)  [unwired: 8 in]
            n1868 = Unbundle By Name(w3162) -> ("Analysis Screen.File 3 Discription"=w3167:refnum<vi>)
            n1869 = Close Reference(reference=w3174, error in (no error)=w3172) -> ()  [unwired: 1 out]
            n1870 = property on="Property Node" class="Str"(reference=w3167, error in=w3165, "Value"=w3164) -> (reference out=w3168:refnum<vi>, error out=w3166:errorcluster)
            n1871 = Close Reference(reference=w3168, error in (no error)=w3166) -> (error out=w3163:errorcluster)
          }
          frame True {
            n1872 = Unbundle By Name(w3179) -> ("Analysis Screen.File Name 3"=w3185:refnum<vi>)
            n1873 = Unbundle By Name(w3179) -> ("Analysis Screen.File 3 Discription"=w3181:refnum<vi>)
            n1874 = property on="Property Node" class="Str"(reference=w3185, "Value"="") -> (reference out=w3186:refnum<vi>, error out=w3184:errorcluster)  [unwired: 1 in]
            n1875 = property on="Property Node" class="Str"(reference=w3181, "Value"="") -> (reference out=w3180:refnum<vi>, error out=w3182:errorcluster)  [unwired: 1 in]
            n1876 = Close Reference(reference=w3180, error in (no error)=w3182) -> ()  [unwired: 1 out]
            n1877 = Close Reference(reference=w3186, error in (no error)=w3184) -> ()  [unwired: 1 out]
            n1878 = call <vilib>:"Clear Errors.vi"("error in (no error)"=w3177) -> ("error out"=w3176:errorcluster)  [unwired: 5 in, 1 out]
          }
        }
        n1879 = Close Reference(reference=w3149, error in (no error)=w3147) -> ()  [unwired: 1 out]
      }
      frame "OPEN 4" {
        n1880 = Unbundle By Name(w3189) -> ("Analysis Screen.File 4 Discription"=w3198:refnum<vi>)
        n1881 = property on="Property Node" class="Str"(reference=w3198, error in=w3196, "Value"="") -> (reference out=w3199:refnum<vi>, error out=w3197:errorcluster)
        n1882 = Close Reference(reference=w3199, error in (no error)=w3197) -> (error out=w3195:errorcluster)
        n1883 = call <vilib>:"Application Directory.vi"() -> ("Application Directory"=w3203:path)
        n1884 = Unbundle By Name(w3189) -> ("Analysis Screen.OPEN 4"=w3191:refnum<vi>)
        n1885 = Build Path(base path=w3203, name or relative path="data") -> (appended path=w3201:path)
        n1886 = property on="Property Node" class="Bool (strict)"(reference=w3191, "Value"=FALSE) -> (reference out=w3192:refnum<vi>, error out=w3190:errorcluster)  [unwired: 1 in]
        n1887 = call "File Dialog6"("start path"=w3201, "error in"=w3195) -> ("selected path"=w3200:path, "cancelled"=w3187:bool, "error out"=w3204:errorcluster)  [unwired: 10 in, 1 out]
        n1888 = case shown="True" w3187 {
          tunnel: w3204 -> [w3218 w3220]
          tunnel: w3200 -> [w3214 _]
          tunnel: [w3206 w3219] -> w3193
          tunnel: w3189 -> [w3205 w3222]
          frame False {
            n1889 = Path To String(path=w3214) -> (string=w3213:string)
            n1890 = Unbundle By Name(w3205) -> ("Analysis Screen.File Name 4"=w3216:refnum<vi>)
            n1891 = call <vilib>:"Clear Errors.vi"("error in (no error)"=w3218) -> ("error out"=w3212:errorcluster)  [unwired: 5 in, 1 out]
            n1892 = property on="Property Node" class="Str"(reference=w3216, "Value"=w3213) -> (reference out=w3217:refnum<vi>, error out=w3215:errorcluster)  [unwired: 1 in]
            n1893 = call "INI FILE READ.vi"("error in (no error)"=w3212, "File Path"=w3213) -> ("error out"=w3208:errorcluster, "concatenated string"=w3207:string)  [unwired: 8 in]
            n1894 = Unbundle By Name(w3205) -> ("Analysis Screen.File 4 Discription"=w3210:refnum<vi>)
            n1895 = Close Reference(reference=w3217, error in (no error)=w3215) -> ()  [unwired: 1 out]
            n1896 = property on="Property Node" class="Str"(reference=w3210, error in=w3208, "Value"=w3207) -> (reference out=w3211:refnum<vi>, error out=w3209:errorcluster)
            n1897 = Close Reference(reference=w3211, error in (no error)=w3209) -> (error out=w3206:errorcluster)
          }
          frame True {
            n1898 = Unbundle By Name(w3222) -> ("Analysis Screen.File Name 4"=w3228:refnum<vi>)
            n1899 = Unbundle By Name(w3222) -> ("Analysis Screen.File 4 Discription"=w3224:refnum<vi>)
            n1900 = property on="Property Node" class="Str"(reference=w3228, "Value"="") -> (reference out=w3229:refnum<vi>, error out=w3227:errorcluster)  [unwired: 1 in]
            n1901 = property on="Property Node" class="Str"(reference=w3224, "Value"="") -> (reference out=w3223:refnum<vi>, error out=w3225:errorcluster)  [unwired: 1 in]
            n1902 = Close Reference(reference=w3223, error in (no error)=w3225) -> ()  [unwired: 1 out]
            n1903 = Close Reference(reference=w3229, error in (no error)=w3227) -> ()  [unwired: 1 out]
            n1904 = call <vilib>:"Clear Errors.vi"("error in (no error)"=w3220) -> ("error out"=w3219:errorcluster)  [unwired: 5 in, 1 out]
          }
        }
        n1905 = Close Reference(reference=w3192, error in (no error)=w3190) -> ()  [unwired: 1 out]
      }
      frame "Refresh 2" {
        n1906 = call "Data Log Refresh.vi"("error in (no error)"=w3232, "Data Cluster"=w3231) -> ("error out"=w3233:errorcluster)  [unwired: 9 in]
        n1907 = local write "Refresh 2"(FALSE ("Refresh 2")) -> ()
      }
      frame "Scratch Mode" {
        n1908 = Unbundle By Name(w3234) -> ("Motion Module.Scratch Mode"=w3237:refnum<vi>)
        n1909 = property on="Property Node" class="Ring (strict)"(reference=w3237) -> (reference out=w3238:refnum<vi>, error out=w3236:errorcluster, "Value"=w3235:u16)  [unwired: 1 in]
        n1910 = Close Reference(reference=w3238, error in (no error)=w3236) -> ()  [unwired: 1 out]
        n1911 = case shown="2" w3235 {
          tunnel: w3234 -> [w3241 w3245]
          frame 0, Default {
            n1912 = Unbundle By Name(w3241) -> ("Motion Module.No of Scratch"=w3243:refnum<vi>)
            n1913 = property on="Property Node" class="DigNum (strict)"(reference=w3243, "Visible"=FALSE) -> (reference out=w3244:refnum<vi>, error out=w3242:errorcluster)  [unwired: 1 in]
            n1914 = Close Reference(reference=w3244, error in (no error)=w3242) -> ()  [unwired: 1 out]
          }
          frame 2 {
            n1915 = Unbundle By Name(w3245) -> ("Motion Module.No of Scratch"=w3248:refnum<vi>)
            n1916 = property on="Property Node" class="DigNum (strict)"(reference=w3248, "Visible"=TRUE) -> (reference out=w3249:refnum<vi>, error out=w3247:errorcluster)  [unwired: 1 in]
            n1917 = Close Reference(reference=w3249, error in (no error)=w3247) -> ()  [unwired: 1 out]
          }
        }
      }
      frame "Export" {
        n1918 = call "Export file.vi"("error in (no error)"=w3258, "Data Cluster"=w3251) -> ("error out"=w3253:errorcluster)  [unwired: 9 in]
        n1919 = call "DATA ENCRYPT STRING FILE WRITE.vi"("error in (no error)"=w3253, "User Action"="User Pressed  Export ", "main ref"=w3251) -> ("error out"=w3252:errorcluster)  [unwired: 6 in, 1 out]
        n1920 = Unbundle By Name(w3251) -> ("Analysis Screen.Export"=w3256:refnum<vi>)
        n1921 = property on="Property Node" class="Bool (strict)"(reference=w3256, "Value"=FALSE) -> (reference out=w3257:refnum<vi>, error out=w3255:errorcluster)  [unwired: 1 in]
        n1922 = Close Reference(reference=w3257, error in (no error)=w3255) -> ()  [unwired: 1 out]
      }
      frame "Traction Receipe Update Details" {
        n1923 = call "Traction Receipe Main.vi"("error in (no error)"=w3264, "main ref"=w3261) -> ("error out"=w3263:errorcluster)  [unwired: 9 in]
        n1924 = local write "Traction Receipe Update Details"(FALSE ("Traction Step Update Details")) -> ()
        n1925 = call "DATA ENCRYPT STRING FILE WRITE.vi"("error in (no error)"=w3263, "User Action"="User Pressed  Traction Update Details ", "main ref"=w3261) -> ("error out"=w3262:errorcluster)  [unwired: 6 in, 1 out]
      }
      frame "Acoustic Emission 3" {
        n1926 = Unbundle By Name(w3266) -> ("Environmental control.Acoustic Emission 3"=w3269:refnum<vi>)
        n1927 = property on="Property Node" class="Bool (strict)"(reference=w3269) -> (reference out=w3267:refnum<vi>, error out=w3268:errorcluster, "Value"=w3265:bool)  [unwired: 1 in]
        n1928 = Close Reference(reference=w3267, error in (no error)=w3268) -> ()  [unwired: 1 out]
        n1929 = case shown="True" w3265 {
          tunnel: w3266 -> [w3273 w3278]
          frame True {
            n1930 = Unbundle By Name(w3273) -> ("Acquostic.Gains"=w3275:refnum<vi>)
            n1931 = property class="RadioBtnsControl (strict)"(reference=w3275, "Visible"=TRUE) -> (reference out=w3277:refnum<vi>, error out=w3276:errorcluster)  [unwired: 1 in]
            n1932 = Close Reference(reference=w3277, error in (no error)=w3276) -> ()  [unwired: 1 out]
          }
          frame False {
            n1933 = Unbundle By Name(w3278) -> ("Acquostic.Gains"=w3280:refnum<vi>)
            n1934 = property class="RadioBtnsControl (strict)"(reference=w3280, "Visible"=FALSE) -> (reference out=w3282:refnum<vi>, error out=w3281:errorcluster)  [unwired: 1 in]
            n1935 = Close Reference(reference=w3282, error in (no error)=w3281) -> ()  [unwired: 1 out]
          }
        }
        n1936 = call "DATA ENCRYPT STRING FILE WRITE.vi"("error in (no error)"=w3272, "User Action"="User Pressed  on  Acuostic in Environmental Screen", "main ref"=w3266) -> ("error out"=w3271:errorcluster)  [unwired: 6 in, 1 out]
      }
      frame "Report" {
        n1937 = call "REPORT GENERATION FOR PYTHON.vi"("error in (no error)"=w3288, "main ref"=w3285) -> ("error out"=w3287:errorcluster)  [unwired: 9 in]
        n1938 = local write "Report"(FALSE ("Report")) -> ()
        n1939 = call "DATA ENCRYPT STRING FILE WRITE.vi"("error in (no error)"=w3287, "User Action"="User Pressed Report ", "main ref"=w3285) -> ("error out"=w3286:errorcluster)  [unwired: 6 in, 1 out]
      }
      frame "Error" {
        # "#CodeRecommended - If you ever change the name of this \"Error\" message, you'll need to update the name in the Check Loop Error.vi as well."
        # "#CodeRecommended - Consider creating a system for logging errors in some way. These errors are for notification purposes only. Handling of specific errors should be performed in the message frames that generated the error."
        # "Error - Display an error dialog. This message is sent by the \"Error Handler\" VIs at the end of other loops in this application."
        n1940 = Variant To Data(error in=w3295, type=errorcluster {"status"=FALSE, "code"=0, "source"=""} ("error constant"), Variant=w3293) -> (data=w3291:errorcluster, error out=w3290:errorcluster)
        n1941 = call <vilib>:"Simple Error Handler.vi"("error in (no error)"=w3291) -> ()  [unwired: 4 in, 5 out]
        n1942 = Merge Errors(w3290) -> (w3289:errorcluster)
      }
      frame "Confirm Quit" {
        # "#CodeNeeded - If you want to provide an \"Are you sure\" dialog (or some other notification) before the application exits, place that code here. This message is typically sent from a Panel Close? event."
        # "Confirm Quit - Message that can confirm whether or not the user wants to exit the application."
        n1943 = call-poly "Enqueue Message.vi"("Priority Message? (F)"=TRUE, "error in (no error)"=w3302, "Message"="Exit", "Message Queue"=w3299) -> ("error out"=w3300:errorcluster)  [unwired: 6 in, 1 out]
        n1944 = Merge Errors(w3300) -> (w3301:errorcluster)
      }
      frame "Exit" {
        # "Stop the VI"
        # "Release the message queue reference"
        # "#CodeNeeded - Add any required cleanup code here. Note that if 'Exit' was called as a result of an error, an error dialog will be displayed. Add any custom error handling for an 'Exit' condition here as well."
        # "Exit - Exit the application."
        n1945 = call "Fire User Event - Stop.vi"("User Event - Stop"=w3305) -> ("error out"=w3304:errorcluster)  [unwired: 10 in]
        n1946 = Release Queue(queue=w3310, error in (no error)=w3303) -> (error out=w3307:errorcluster)  [unwired: 1 in, 2 out]
        n1947 = Merge Errors(w3304, w3307) -> (w3306:errorcluster)
      }
      frame Default {
        # "'Default' case only runs if there is a message that isn't defined in any of the other cases.  Output a programming error."
        n1948 = xnode ("Error Ring")("parameter 0"=w3311) -> ("error out"=w3312:errorcluster)
      }
    }
    n1949 = call "LAB-IQ Error Handler - Message Handling Loop.vi"("error in (no error)"=w1877, "Message Queue"=w1879) -> ("dup error in"=w1878:errorcluster)  [unwired: 8 in, 1 out]
  }
  n1950 = while "Timed Loop" {
    shift-right: [w3332] -> _
    shift-left: w5 -> [w3333]
    tunnel: [w3326] -> w38
    tunnel: w37 -> [w3324]
    tunnel: w2 -> [w3323]
    tunnel: w6 -> [w3322]
    stop <- w3331 stop-if-true
    # "Load  Handling Loop"
    n1951 = call "Dequeue Message.vi"("error in (no error)"=w3323, "Message Queue"=w3324) -> ("error out"=w3330:errorcluster, "Message Data"=w3328:variant, "Message"=w3329:string, "dup Message Queue"=w3327:refnum<queue>)  [unwired: 6 in]
    n1952 = case "Message Cases" shown="\"Load Main\"" w3329 {
      selector: w3329 -> [_ _ _ _ _ w3384]
      tunnel: w3327 -> [w3337 w3348 _ w3373 w3383 _]
      tunnel: w3330 -> [w3336 w3346 w3364 w3375 w3377 _]
      tunnel: [w3339 w3349 w3358 w3368 w3379 w3385] -> w3325
      tunnel: w3333 -> [w3335 w3341 w3363 w3365 w3382 w3386]
      tunnel: [w3335 w3341 w3363 w3365 w3382 w3386] -> w3332
      tunnel: [_ _ _ _ TRUE _] -> w3331
      tunnel: w3328 -> [_ _ w3362 _ _ _]
      tunnel: w3322 -> [_ _ _ _ w3376 _]
      frame "init" {
        # "Bundle control references and a sample string value."
        # "Initialize - All initialization work should take place in this message, since other loops can potentially enqueue messages that execute immediately after this one."
        n1953 = call "SET LOAD PARAMETERS.vi"("error in (no error)"=w3336, "main ref"=w3335) -> ("error out"=w3334:errorcluster)  [unwired: 9 in]
        n1954 = call-poly "Enqueue Message.vi"("error in (no error)"=w3334, "Message"="Load Main", "Message Queue"=w3337) -> ("error out"=w3339:errorcluster)  [unwired: 7 in, 1 out]
      }
      frame "Load Main" {
        n1955 = call "LOAD CELL READ.vi"("error in (no error)"=w3346, "main ref"=w3341) -> ("error out"=w3342:errorcluster)  [unwired: 9 in]
        n1956 = call <vilib>:"Clear Errors.vi"("error in (no error)"=w3342) -> ("error out"=w3340:errorcluster)  [unwired: 5 in, 1 out]
        n1957 = Unbundle By Name(w3341) -> ("Main Home Screen.EXIT"=w3347:refnum<vi>)
        n1958 = property on="Property Node" class="Bool (strict)"(reference=w3347) -> (reference out=w3344:refnum<vi>, error out=w3345:errorcluster, "Value"=w3343:bool)  [unwired: 1 in]
        n1959 = Close Reference(reference=w3344, error in (no error)=w3345) -> ()  [unwired: 1 out]
        n1960 = case shown="False" w3343 {
          tunnel: [w3352 w3356] -> w3349
          tunnel: w3348 -> [w3351 w3355]
          tunnel: w3340 -> [w3350 w3354]
          frame True {
            n1961 = call-poly "Enqueue Message.vi"("error in (no error)"=w3350, "Message"="Confirm Quit", "Message Queue"=w3351) -> ("error out"=w3352:errorcluster)  [unwired: 7 in, 1 out]
          }
          frame False {
            n1962 = call-poly "Enqueue Message.vi"("error in (no error)"=w3354, "Message"="Load Main", "Message Queue"=w3355) -> ("error out"=w3356:errorcluster)  [unwired: 7 in, 1 out]
          }
        }
      }
      frame "Error" {
        # "#CodeRecommended - If you ever change the name of this \"Error\" message, you'll need to update the name in the Check Loop Error.vi as well."
        # "#CodeRecommended - Consider creating a system for logging errors in some way. These errors are for notification purposes only. Handling of specific errors should be performed in the message frames that generated the error."
        # "Error - Display an error dialog. This message is sent by the \"Error Handler\" VIs at the end of other loops in this application."
        n1963 = Variant To Data(error in=w3364, type=errorcluster {"status"=FALSE, "code"=0, "source"=""} ("error constant"), Variant=w3362) -> (data=w3360:errorcluster, error out=w3359:errorcluster)
        n1964 = call <vilib>:"Simple Error Handler.vi"("error in (no error)"=w3360) -> ()  [unwired: 4 in, 5 out]
        n1965 = Merge Errors(w3359) -> (w3358:errorcluster)
      }
      frame "Confirm Quit" {
        # "#CodeNeeded - If you want to provide an \"Are you sure\" dialog (or some other notification) before the application exits, place that code here. This message is typically sent from a Panel Close? event."
        # "Confirm Quit - Message that can confirm whether or not the user wants to exit the application."
        n1966 = call-poly "Enqueue Message.vi"("Priority Message? (F)"=TRUE, "error in (no error)"=w3375, "Message"="Exit", "Message Queue"=w3373) -> ("error out"=w3374:errorcluster)  [unwired: 6 in, 1 out]
        n1967 = Merge Errors(w3374) -> (w3370:errorcluster)
        n1968 = call <vilib>:"Clear Errors.vi"("error in (no error)"=w3370) -> ("error out"=w3369:errorcluster)  [unwired: 5 in, 1 out]
        n1969 = call "NEW Load Cell FGV.vi"("Enum - Menu"=Load_cell_Enum."close", "error in (no error)"=w3369, "main ref"=w3365) -> ("error out"=w3367:errorcluster)  [unwired: 7 in, 1 out]
        n1970 = call <vilib>:"Clear Errors.vi"("error in (no error)"=w3367) -> ("error out"=w3368:errorcluster)  [unwired: 5 in, 1 out]
      }
      frame "Exit" {
        # "Stop the VI"
        # "Release the message queue reference"
        # "#CodeNeeded - Add any required cleanup code here. Note that if 'Exit' was called as a result of an error, an error dialog will be displayed. Add any custom error handling for an 'Exit' condition here as well."
        # "Exit - Exit the application."
        n1971 = call "Fire User Event - Stop.vi"("User Event - Stop"=w3376) -> ("error out"=w3378:errorcluster)  [unwired: 10 in]
        n1972 = Release Queue(queue=w3383, error in (no error)=w3377) -> (error out=w3380:errorcluster)  [unwired: 1 in, 2 out]
        n1973 = Merge Errors(w3378, w3380) -> (w3379:errorcluster)
      }
      frame Default {
        # "'Default' case only runs if there is a message that isn't defined in any of the other cases.  Output a programming error."
        n1974 = xnode ("Error Ring")("parameter 0"=w3384) -> ("error out"=w3385:errorcluster)
      }
    }
    n1975 = call "LAB-IQ Error Handler - Message Handling Loop.vi"("error in (no error)"=w3325, "Message Queue"=w3327) -> ("dup error in"=w3326:errorcluster)  [unwired: 8 in, 1 out]
    n1976 = Wait (ms)(milliseconds to wait=u32 20) -> ()  [unwired: 1 out]
  }
  n1977 = while "Timed Loop" {
    shift-right: [w3395] -> _
    shift-left: w5 -> [w3414]
    tunnel: [w3408] -> w35
    tunnel: w36 -> [w3406]
    tunnel: w2 -> [w3405]
    tunnel: w6 -> [w3404]
    stop <- w3413 stop-if-true
    # "Sway Motor  Handling Loop"
    n1978 = call "Dequeue Message.vi"("error in (no error)"=w3405, "Message Queue"=w3406) -> ("error out"=w3412:errorcluster, "Message Data"=w3410:variant, "Message"=w3411:string, "dup Message Queue"=w3409:refnum<queue>)  [unwired: 6 in]
    n1979 = case "Message Cases" shown="\"Sway Main\"" w3411 {
      selector: w3411 -> [_ _ _ _ _ w3498]
      tunnel: w3409 -> [w3426 w3455 _ w3485 w3497 _]
      tunnel: w3412 -> [w3428 w3438 w3482 w3489 w3491 _]
      tunnel: [w3429 w3456 w3476 w3487 w3493 w3499] -> w3407
      tunnel: w3414 -> [w3416 w3433 w3481 w3488 w3496 w3500]
      tunnel: [w3416 w3433 w3481 w3488 w3496 w3500] -> w3395
      tunnel: [_ _ _ _ TRUE _] -> w3413
      tunnel: w3410 -> [_ _ w3480 _ _ _]
      tunnel: w3404 -> [_ _ _ _ w3490 _]
      frame "init" {
        # "Initialize - All initialization work should take place in this message, since other loops can potentially enqueue messages that execute immediately after this one."
        n1980 = call "SWAY WRITE FGV.vi"("Enum - Menu"=Sway_Write_enum."INIT", "error in (no error)"=w3428, "main ref"=w3416) -> ("error out"=w3425:errorcluster)  [unwired: 8 in]
        n1981 = call <vilib>:"Clear Errors.vi"("error in (no error)"=w3425) -> ("error out"=w3419:errorcluster)  [unwired: 5 in, 1 out]
        n1982 = call "Stall Data Flow.vim"("value in"=w3419, "milliseconds to wait"=u32 1000) -> ("value out"=w3423:errorcluster)  [unwired: 1 out]
        n1983 = call "Sway Init.vi"("error in (no error)"=w3423, "main ref"=w3416) -> ("error out"=w3420:errorcluster)  [unwired: 9 in]
        n1984 = call <vilib>:"Clear Errors.vi"("error in (no error)"=w3420) -> ("error out"=w3418:errorcluster)  [unwired: 5 in, 1 out]
        n1985 = call "SWAY READ FGV.vi"("Enum - Menu"=Sway_Right_enum."INIT", "error in (no error)"=w3418, "main ref"=w3416) -> ("error out"=w3417:errorcluster)  [unwired: 7 in, 1 out]
        n1986 = call <vilib>:"Clear Errors.vi"("error in (no error)"=w3417) -> ("error out"=w3421:errorcluster)  [unwired: 5 in, 1 out]
        n1987 = call-poly "Enqueue Message.vi"("error in (no error)"=w3421, "Message"="Sway Main", "Message Queue"=w3426) -> ("error out"=w3429:errorcluster)  [unwired: 7 in, 1 out]
      }
      frame "Sway Main" {
        n1988 = Unbundle By Name(w3433) -> ("Heave AND Surge.Homed"=w3441:refnum<vi>)
        n1989 = Unbundle By Name(w3433) -> ("SWAY.Read SWAY Temp"=w3450:refnum<vi>)
        n1990 = local read "HEAVE ENABLE"() -> (w3445:bool)
        n1991 = property on="Property Node" class="DigNum (strict)"(reference=w3441) -> (reference out=w3443:refnum<vi>, error out=w3442:errorcluster, "Value"=w3432:u8)  [unwired: 1 in]
        n1992 = property on="Property Node" class="Bool (strict)"(reference=w3450) -> (reference out=w3448:refnum<vi>, error out=w3449:errorcluster, "Value"=w3447:bool)  [unwired: 1 in]
        n1993 = Equal?(x=w3445, y=TRUE) -> (x = y?=w3440:bool)
        n1994 = Close Reference(reference=w3443, error in (no error)=w3442) -> ()  [unwired: 1 out]
        n1995 = Equal?(x=w3432, y=u8 1 ("Value")) -> (x = y?=w3430:bool)
        n1996 = Close Reference(reference=w3448, error in (no error)=w3449) -> ()  [unwired: 1 out]
        n1997 = And(x=w3440, y=w3430) -> (x .and. y?=w3439:bool)
        n1998 = case shown="True" w3447 {
          tunnel: w3438 -> [w3463 w3467]
          tunnel: [w3463 w3466] -> w3435
          tunnel: w3433 -> [_ w3465]
          frame False {
          }
          frame True {
            n1999 = call "SWAY READ FGV.vi"("Enum - Menu"=Sway_Right_enum."READ", "error in (no error)"=w3467, "main ref"=w3465) -> ("error out"=w3466:errorcluster)  [unwired: 7 in, 1 out]
          }
        }
        n2000 = case shown="True" w3439 {
          tunnel: w3433 -> [_ w3462]
          tunnel: w3438 -> [w3457 w3461]
          tunnel: [w3457 w3458] -> w3436
          frame False {
          }
          frame True {
            n2001 = call "SWAY HOME.vi"("error in (no error)"=w3461, "Data Cluster"=w3462) -> ("error out"=w3459:errorcluster)  [unwired: 9 in]
            n2002 = local write "HEAVE ENABLE"(FALSE ("HEAVE ENABLE")) -> ()
            n2003 = call <vilib>:"Clear Errors.vi"("error in (no error)"=w3459) -> ("error out"=w3458:errorcluster)  [unwired: 5 in, 1 out]
          }
        }
        n2004 = call "Sway Reinitize.vi"("error in (no error)"=w3435, "Data Cluster"=w3433) -> ("error out"=w3434:errorcluster)  [unwired: 9 in]
        n2005 = Unbundle By Name(w3433) -> ("Main Home Screen.EXIT"=w3454:refnum<vi>)
        n2006 = property on="Property Node" class="Bool (strict)"(reference=w3454) -> (reference out=w3452:refnum<vi>, error out=w3453:errorcluster, "Value"=w3451:bool)  [unwired: 1 in]
        n2007 = call <vilib>:"Clear Errors.vi"("error in (no error)"=w3434) -> ("error out"=w3446:errorcluster)  [unwired: 5 in, 1 out]
        n2008 = Merge Errors(w3446, w3436) -> (w3437:errorcluster)
        n2009 = Close Reference(reference=w3452, error in (no error)=w3453) -> ()  [unwired: 1 out]
        n2010 = case shown="False" w3451 {
          tunnel: [w3470 w3474] -> w3456
          tunnel: w3455 -> [w3469 w3473]
          tunnel: w3437 -> [w3468 w3472]
          frame True {
            n2011 = call-poly "Enqueue Message.vi"("error in (no error)"=w3468, "Message"="Confirm Quit", "Message Queue"=w3469) -> ("error out"=w3470:errorcluster)  [unwired: 7 in, 1 out]
          }
          frame False {
            n2012 = call-poly "Enqueue Message.vi"("error in (no error)"=w3472, "Message"="Sway Main", "Message Queue"=w3473) -> ("error out"=w3474:errorcluster)  [unwired: 7 in, 1 out]
          }
        }
      }
      frame "Error" {
        # "#CodeRecommended - If you ever change the name of this \"Error\" message, you'll need to update the name in the Check Loop Error.vi as well."
        # "#CodeRecommended - Consider creating a system for logging errors in some way. These errors are for notification purposes only. Handling of specific errors should be performed in the message frames that generated the error."
        # "Error - Display an error dialog. This message is sent by the \"Error Handler\" VIs at the end of other loops in this application."
        n2013 = Variant To Data(error in=w3482, type=errorcluster {"status"=FALSE, "code"=0, "source"=""} ("error constant"), Variant=w3480) -> (data=w3478:errorcluster, error out=w3477:errorcluster)
        n2014 = call <vilib>:"Simple Error Handler.vi"("error in (no error)"=w3478) -> ()  [unwired: 4 in, 5 out]
        n2015 = Merge Errors(w3477) -> (w3476:errorcluster)
      }
      frame "Confirm Quit" {
        # "#CodeNeeded - If you want to provide an \"Are you sure\" dialog (or some other notification) before the application exits, place that code here. This message is typically sent from a Panel Close? event."
        # "Confirm Quit - Message that can confirm whether or not the user wants to exit the application."
        n2016 = call-poly "Enqueue Message.vi"("Priority Message? (F)"=TRUE, "error in (no error)"=w3489, "Message"="Exit", "Message Queue"=w3485) -> ("error out"=w3486:errorcluster)  [unwired: 6 in, 1 out]
        n2017 = Merge Errors(w3486) -> (w3487:errorcluster)
      }
      frame "Exit" {
        # "Stop the VI"
        # "Release the message queue reference"
        # "#CodeNeeded - Add any required cleanup code here. Note that if 'Exit' was called as a result of an error, an error dialog will be displayed. Add any custom error handling for an 'Exit' condition here as well."
        # "Exit - Exit the application."
        n2018 = call "Fire User Event - Stop.vi"("User Event - Stop"=w3490) -> ("error out"=w3492:errorcluster)  [unwired: 10 in]
        n2019 = Release Queue(queue=w3497, error in (no error)=w3491) -> (error out=w3494:errorcluster)  [unwired: 1 in, 2 out]
        n2020 = Merge Errors(w3492, w3494) -> (w3493:errorcluster)
      }
      frame Default {
        # "'Default' case only runs if there is a message that isn't defined in any of the other cases.  Output a programming error."
        n2021 = xnode ("Error Ring")("parameter 0"=w3498) -> ("error out"=w3499:errorcluster)
      }
    }
    n2022 = Unbundle By Name(w3395) -> ("Environmental control.Acoustic Emission 3"=w3403:refnum<vi>)
    n2023 = call "LAB-IQ Error Handler - Message Handling Loop.vi"("error in (no error)"=w3407, "Message Queue"=w3409) -> ("dup error in"=w3408:errorcluster)  [unwired: 8 in, 1 out]
    n2024 = property on="Property Node" class="Bool (strict)"(reference=w3403) -> (reference out=w3401:refnum<vi>, error out=w3402:errorcluster, "Value"=w3400:bool)  [unwired: 1 in]
    n2025 = Close Reference(reference=w3401, error in (no error)=w3402) -> ()  [unwired: 1 out]
    n2026 = Equal?(x=w3400, y=TRUE) -> (x = y?=w3398:bool)
    n2027 = Select(t=i64 20 ("Period"), s=w3398, f=i64 5) -> (s? t:f=w3394:i64)
    n2028 = Wait (ms)(milliseconds to wait=w3394) -> ()  [unwired: 1 out]
  }
  n2029 = while {
    shift-right: [w3509] -> _
    shift-left: w5 -> [w3520]
    tunnel: [w3514] -> w10
    tunnel: w29 -> [w3512]
    tunnel: w2 -> [w3511]
    tunnel: w6 -> [w3510]
    stop <- w3519 stop-if-true
    # "Program  Handling Loop"
    n2030 = call "Dequeue Message.vi"("error in (no error)"=w3511, "Message Queue"=w3512) -> ("error out"=w3518:errorcluster, "Message Data"=w3516:variant, "Message"=w3517:string, "dup Message Queue"=w3515:refnum<queue>)  [unwired: 6 in]
    n2031 = case "Message Cases" shown="\"Program Main\"" w3517 {
      selector: w3517 -> [_ _ _ _ _ w3565]
      tunnel: w3515 -> [w3521 w3533 _ w3552 w3564 _]
      tunnel: w3518 -> [w3524 w3527 w3549 w3556 w3558 _]
      tunnel: [w3525 w3534 w3543 w3554 w3560 w3566] -> w3513
      tunnel: w3520 -> [w3523 w3526 w3548 w3555 w3563 w3567]
      tunnel: [w3523 w3526 w3548 w3555 w3563 w3567] -> w3509
      tunnel: [_ _ _ _ TRUE _] -> w3519
      tunnel: w3516 -> [_ _ w3547 _ _ _]
      tunnel: w3510 -> [_ _ _ _ w3557 _]
      frame "init" {
        # "Initialize - All initialization work should take place in this message, since other loops can potentially enqueue messages that execute immediately after this one."
        n2032 = call-poly "Enqueue Message.vi"("error in (no error)"=w3524, "Message"="Program Main", "Message Queue"=w3521) -> ("error out"=w3525:errorcluster)  [unwired: 7 in, 1 out]
      }
      frame "Program Main" {
        n2033 = call "Main Program Loop Vi.vi"("error in (no error)"=w3527, "Data Cluster"=w3526) -> ("error out"=w3528:errorcluster)  [unwired: 9 in]
        n2034 = Unbundle By Name(w3526) -> ("Main Home Screen.EXIT"=w3532:refnum<vi>)
        n2035 = property on="Property Node" class="Bool (strict)"(reference=w3532) -> (reference out=w3530:refnum<vi>, error out=w3531:errorcluster, "Value"=w3529:bool)  [unwired: 1 in]
        n2036 = case shown="False" w3529 {
          tunnel: [w3537 w3541] -> w3534
          tunnel: w3533 -> [w3536 w3540]
          tunnel: w3528 -> [w3535 w3539]
          frame True {
            n2037 = call-poly "Enqueue Message.vi"("error in (no error)"=w3535, "Message"="Confirm Quit", "Message Queue"=w3536) -> ("error out"=w3537:errorcluster)  [unwired: 7 in, 1 out]
          }
          frame False {
            n2038 = call-poly "Enqueue Message.vi"("error in (no error)"=w3539, "Message"="Program Main", "Message Queue"=w3540) -> ("error out"=w3541:errorcluster)  [unwired: 7 in, 1 out]
          }
        }
        n2039 = Close Reference(reference=w3530, error in (no error)=w3531) -> ()  [unwired: 1 out]
      }
      frame "Error" {
        # "#CodeRecommended - If you ever change the name of this \"Error\" message, you'll need to update the name in the Check Loop Error.vi as well."
        # "#CodeRecommended - Consider creating a system for logging errors in some way. These errors are for notification purposes only. Handling of specific errors should be performed in the message frames that generated the error."
        # "Error - Display an error dialog. This message is sent by the \"Error Handler\" VIs at the end of other loops in this application."
        n2040 = Variant To Data(error in=w3549, type=errorcluster {"status"=FALSE, "code"=0, "source"=""} ("error constant"), Variant=w3547) -> (data=w3545:errorcluster, error out=w3544:errorcluster)
        n2041 = call <vilib>:"Simple Error Handler.vi"("error in (no error)"=w3545) -> ()  [unwired: 4 in, 5 out]
        n2042 = Merge Errors(w3544) -> (w3543:errorcluster)
      }
      frame "Confirm Quit" {
        # "#CodeNeeded - If you want to provide an \"Are you sure\" dialog (or some other notification) before the application exits, place that code here. This message is typically sent from a Panel Close? event."
        # "Confirm Quit - Message that can confirm whether or not the user wants to exit the application."
        n2043 = call-poly "Enqueue Message.vi"("Priority Message? (F)"=TRUE, "error in (no error)"=w3556, "Message"="Exit", "Message Queue"=w3552) -> ("error out"=w3553:errorcluster)  [unwired: 6 in, 1 out]
        n2044 = Merge Errors(w3553) -> (w3554:errorcluster)
      }
      frame "Exit" {
        # "Stop the VI"
        # "Release the message queue reference"
        # "#CodeNeeded - Add any required cleanup code here. Note that if 'Exit' was called as a result of an error, an error dialog will be displayed. Add any custom error handling for an 'Exit' condition here as well."
        # "Exit - Exit the application."
        n2045 = call "Fire User Event - Stop.vi"("User Event - Stop"=w3557) -> ("error out"=w3559:errorcluster)  [unwired: 10 in]
        n2046 = Release Queue(queue=w3564, error in (no error)=w3558) -> (error out=w3561:errorcluster)  [unwired: 1 in, 2 out]
        n2047 = Merge Errors(w3559, w3561) -> (w3560:errorcluster)
      }
      frame Default {
        # "'Default' case only runs if there is a message that isn't defined in any of the other cases.  Output a programming error."
        n2048 = xnode ("Error Ring")("parameter 0"=w3565) -> ("error out"=w3566:errorcluster)
      }
    }
    n2049 = call "LAB-IQ Error Handler - Message Handling Loop.vi"("error in (no error)"=w3513, "Message Queue"=w3515) -> ("dup error in"=w3514:errorcluster)  [unwired: 8 in, 1 out]
    n2050 = Wait Until Next ms Multiple(millisecond multiple=i64 100 ("Period")) -> ()  [unwired: 1 out]
  }
  n2051 = while "Timed Loop" {
    shift-right: [w3581] -> _
    shift-left: w5 -> [w3595]
    tunnel: [w3589] -> w9
    tunnel: w28 -> [w3587]
    tunnel: w2 -> [w3586]
    tunnel: w6 -> [w3585]
    stop <- w3594 stop-if-true
    # "Monitor  Handling Loop"
    n2052 = call "Dequeue Message.vi"("error in (no error)"=w3586, "Message Queue"=w3587) -> ("error out"=w3593:errorcluster, "Message Data"=w3591:variant, "Message"=w3592:string, "dup Message Queue"=w3590:refnum<queue>)  [unwired: 6 in]
    n2053 = case "Message Cases" shown="\"Monitor Main\"" w3592 {
      selector: w3592 -> [_ _ _ _ _ w3642]
      tunnel: w3590 -> [w3596 w3610 _ w3629 w3641 _]
      tunnel: w3593 -> [w3599 w3601 w3626 w3633 w3635 _]
      tunnel: [w3600 w3611 w3620 w3631 w3637 w3643] -> w3588
      tunnel: w3595 -> [w3598 w3602 w3625 w3632 w3640 w3644]
      tunnel: [w3598 w3602 w3625 w3632 w3640 w3644] -> w3581
      tunnel: [_ _ _ _ TRUE _] -> w3594
      tunnel: w3591 -> [_ _ w3624 _ _ _]
      tunnel: w3585 -> [_ _ _ _ w3634 _]
      frame "init" {
        # "Initialize - All initialization work should take place in this message, since other loops can potentially enqueue messages that execute immediately after this one."
        n2054 = call-poly "Enqueue Message.vi"("error in (no error)"=w3599, "Message"="Monitor Main", "Message Queue"=w3596) -> ("error out"=w3600:errorcluster)  [unwired: 7 in, 1 out]
      }
      frame "Monitor Main" {
        n2055 = call "Main Monitor Loop.vi"("error in (no error)"=w3601, "main ref"=w3602) -> ("error out"=w3605:errorcluster)  [unwired: 9 in]
        n2056 = call "LOAD SELECTION MAIN CODE.vi"("error in (no error)"=w3601, "main ref"=w3602) -> ("error out"=w3603:errorcluster)  [unwired: 9 in]
        n2057 = Merge Errors(w3605, w3603) -> (w3604:errorcluster)
        n2058 = Unbundle By Name(w3602) -> ("Main Home Screen.EXIT"=w3609:refnum<vi>)
        n2059 = property on="Property Node" class="Bool (strict)"(reference=w3609) -> (reference out=w3607:refnum<vi>, error out=w3608:errorcluster, "Value"=w3606:bool)  [unwired: 1 in]
        n2060 = case shown="False" w3606 {
          tunnel: [w3614 w3618] -> w3611
          tunnel: w3610 -> [w3613 w3617]
          tunnel: w3604 -> [w3612 w3616]
          frame True {
            n2061 = call-poly "Enqueue Message.vi"("error in (no error)"=w3612, "Message"="Confirm Quit", "Message Queue"=w3613) -> ("error out"=w3614:errorcluster)  [unwired: 7 in, 1 out]
          }
          frame False {
            n2062 = call-poly "Enqueue Message.vi"("error in (no error)"=w3616, "Message"="Monitor Main", "Message Queue"=w3617) -> ("error out"=w3618:errorcluster)  [unwired: 7 in, 1 out]
          }
        }
        n2063 = Close Reference(reference=w3607, error in (no error)=w3608) -> ()  [unwired: 1 out]
      }
      frame "Error" {
        # "#CodeRecommended - If you ever change the name of this \"Error\" message, you'll need to update the name in the Check Loop Error.vi as well."
        # "#CodeRecommended - Consider creating a system for logging errors in some way. These errors are for notification purposes only. Handling of specific errors should be performed in the message frames that generated the error."
        # "Error - Display an error dialog. This message is sent by the \"Error Handler\" VIs at the end of other loops in this application."
        n2064 = Variant To Data(error in=w3626, type=errorcluster {"status"=FALSE, "code"=0, "source"=""} ("error constant"), Variant=w3624) -> (data=w3622:errorcluster, error out=w3621:errorcluster)
        n2065 = call <vilib>:"Simple Error Handler.vi"("error in (no error)"=w3622) -> ()  [unwired: 4 in, 5 out]
        n2066 = Merge Errors(w3621) -> (w3620:errorcluster)
      }
      frame "Confirm Quit" {
        # "#CodeNeeded - If you want to provide an \"Are you sure\" dialog (or some other notification) before the application exits, place that code here. This message is typically sent from a Panel Close? event."
        # "Confirm Quit - Message that can confirm whether or not the user wants to exit the application."
        n2067 = call-poly "Enqueue Message.vi"("Priority Message? (F)"=TRUE, "error in (no error)"=w3633, "Message"="Exit", "Message Queue"=w3629) -> ("error out"=w3630:errorcluster)  [unwired: 6 in, 1 out]
        n2068 = Merge Errors(w3630) -> (w3631:errorcluster)
      }
      frame "Exit" {
        # "Stop the VI"
        # "Release the message queue reference"
        # "#CodeNeeded - Add any required cleanup code here. Note that if 'Exit' was called as a result of an error, an error dialog will be displayed. Add any custom error handling for an 'Exit' condition here as well."
        # "Exit - Exit the application."
        n2069 = call "Fire User Event - Stop.vi"("User Event - Stop"=w3634) -> ("error out"=w3636:errorcluster)  [unwired: 10 in]
        n2070 = Release Queue(queue=w3641, error in (no error)=w3635) -> (error out=w3638:errorcluster)  [unwired: 1 in, 2 out]
        n2071 = Merge Errors(w3636, w3638) -> (w3637:errorcluster)
      }
      frame Default {
        # "'Default' case only runs if there is a message that isn't defined in any of the other cases.  Output a programming error."
        n2072 = xnode ("Error Ring")("parameter 0"=w3642) -> ("error out"=w3643:errorcluster)
      }
    }
    n2073 = Unbundle By Name(w3581) -> ("Environmental control.Acoustic Emission 3"=w3584:refnum<vi>)
    n2074 = property on="Property Node" class="Bool (strict)"(reference=w3584) -> (reference out=w3582:refnum<vi>, error out=w3583:errorcluster, "Value"=w3580:bool)  [unwired: 1 in]
    n2075 = call "LAB-IQ Error Handler - Message Handling Loop.vi"("error in (no error)"=w3588, "Message Queue"=w3590) -> ("dup error in"=w3589:errorcluster)  [unwired: 8 in, 1 out]
    n2076 = Close Reference(reference=w3582, error in (no error)=w3583) -> ()  [unwired: 1 out]
    n2077 = Equal?(x=w3580, y=TRUE) -> (x = y?=w3578:bool)
    n2078 = Select(t=i64 10 ("Period"), s=w3578, f=i64 100) -> (s? t:f=w3575:i64)
    n2079 = Wait Until Next ms Multiple(millisecond multiple=w3575) -> ()  [unwired: 1 out]
  }
  n2080 = Unregister For Events(event registration refnum=w61, error in=w59) -> (error out=w62:errorcluster)
  n2081 = Merge Errors(w62, w65, w38, w35, w33, w19, w16, w12, w11, w10, w9, w8, w2, w1) -> (w63:errorcluster)
  n2082 = call "Destroy User Event - Stop.vi"("error in (no error)"=w63, "User Event - Stop"=w6) -> ("error out"=w60:errorcluster)  [unwired: 9 in]
  n2083 = disable-structure "Conditional Disable Structure" shown="RUN_TIME_ENGINE==True" {
    disable-tunnel: w60 -> [_ _]
    frame condition #0 (active) {
    }
    frame condition #1 {
      # "Call Quit LabVIEW if running as a built application."
      n2084 = Quit LabVIEW() -> ()  [unwired: 1 in]
    }
  }
